vi "main4Ch_USBCam.vi"() -> ()   [LabVIEW 2024]
doc: "Main VI for FLS imaging system."
uses:
  SubVI/DigitizerConfiguration/FLImDAQ.ctl
  <instrlib>/niScope/Controls/niScope trigger source.ctl
  SubVI/LabJack/LJ Pin Setting.ctl
  ConfigFiles/AimingBeamVideoConfig.ctl
  LaguerreDeconLib/DeconEngineClass/LaguerreDeconEngineClass.lvclass/LaguerreDeconEngineClass.ctl
  <vilib>/Utility/error.llb/DialogType.ctl
  LaguerreDeconLib/DeconEngineClass/LaguerreDeconEngineClass.lvclass
  <vilib>/event_ctls.llb/usereventprio.ctl
  <vilib>/Utility/miscctls.llb/LVMinMaxIncTypeDef.ctl
  SubVI/APD/APDClass.lvclass
  <vilib>/vision/driver/IMAQdx.llb/IMAQdx Acquisition Mode.ctl
  <vilib>/userDefined/High Color/IMAQdx.ctl
  <vilib>/vision/driver/IMAQdx.llb/IMAQdx Camera Control Mode.ctl
  <vilib>/vision/driver/IMAQdx.llb/IMAQdx Buffer Number Mode.ctl
  <vilib>/Analysis/baseanly.llb/Mean (DBL).vi
  SubVI/GlobalVariables.vi
  <vilib>/addons/control/pid/pid.llb/PID (DBL).vi
  <vilib>/Utility/file.llb/Write Delimited Spreadsheet (DBL).vi
  <instrlib>/niScope/Acquire/Fetch/niScope Multi Fetch Binary 16.vi
  <vilib>/Instr/_visa.llb/VISA Configure Serial Port (Instr).vi
  <userlib>/_OpenG.lib/file/file.llb/openg_file.lvlib
  <userlib>/_OpenG.lib/time/time.llb/openg_time.lvlib
  <vilib>/Analysis/NI_AALBase.lvlib
  <vilib>/Utility/miscctls.llb/LVPointTypeDef.ctl
  <vilib>/addons/control/pid/NI_PID_pid.lvlib
  <vilib>/vision/driver/NI_Vision_Acquisition_Software.lvlib
  <resource>/objmgr/imaqdx.rc
panel:
  out "Image 2":T1(plugin-control)
  in  "Live?":bool
  out "Record Backlog 2":i32
  in  "Auto gain ch4":bool=TRUE caption="Auto gain ch3"
  in  "V 4":dbl caption="Gain 3" min=0.0 max=4.67 step=0.1
  out "Gain4":dbl
  out "Lifetime 4":dbl caption="Lifetime 3"
  out "IntR4":dbl format="%#_2g"
  out "SNR4":dbl format="%#_3g"
  out "Channel 4":dbl[][](graph) caption="Channel 3"
  out "RunStartTime":u32
  out "Dig1 Temp":dbl
  out "Dig2 Temp":dbl
  out "Visualization PC video source":T2
  in  "V target(1.0)":dbl=1.0 caption="V target(1.5)" min=0.3 max=1.5 step=0.1 format="%#_4g"
  out "SNR3":dbl format="%#_3g"
  out "SNR2":dbl format="%#_3g"
  out "SNR1":dbl format="%#_3g"
  in  "Show BG removed?":bool=TRUE
  out "IntR3":dbl format="%#_2g"
  out "IntR2":dbl format="%#_2g"
  out "IntR1":dbl format="%#_2g"
  in  "Video Display":bool
  out "Gain3":dbl
  out "Gain2":dbl
  out "Gain1":dbl
  in  "Skip Data Save?":bool
  out "Aq Loop?":bool
  out "ML?":bool
  out "aquisition loop Error Out":errorcluster
  out "Laser f (Hz)":dbl
  out "Record Backlog":i32
  out "Fetch Record #":i32
  out "Sync Success?":bool
  out "Disclamer":picture
  out "Calibration #":i8
  out "BG #":i8
  in  "TCP Connect":bool
  out "Help":string
  in  "355nm Laser toggle":bool caption="355nm 460Hz"
  in  "Cali&iRF alignment":bool
  in  "Background":bool
  in  "Aiming beam toggle":bool caption="445nm 0Hz 25mA"
  out "Lifetime 3":dbl
  out "Lifetime 2":dbl
  in  "Auto gain ch3":bool=TRUE
  in  "Auto gain ch2":bool=TRUE
  in  "Auto gain ch1":bool=TRUE
  out "Run #":i8
  in  "StopButton":bool caption="Stop"
  out "Aquisition Status:":bool
  in  "StartButton":bool caption="Start"
  in  "V 3":dbl caption="Gain 3" min=0.0 max=4.68 step=0.1
  in  "V 2":dbl caption="Gain 2" min=0.0 max=4.62 step=0.1
  out "Lifetime 1":dbl
  in  "V 1":dbl caption="Gain 1" min=0.0 max=4.66 step=0.1 format="%#_4g"
  in  "Video Source":enum32{"Camera", "FrameGrabber"}(radio)
  out "Case #":string
  out "System Hardware Connection Status":T3
  out "Channel 3":dbl[][](graph)
  out "Channel 2":dbl[][](graph)
  out "Channel 1":dbl[][](graph)
  in  "Tab Control":T4(tab)
  out "display loop timing(ms)":u32
  out "Aquisition loop timing(ms)":u32 format="%.2f"
  out "DisplayLoop":i32
  out "PID loop":i32 caption="processing loop"
  out "PID loop timing(ms)":u32 caption="processing loop timing(ms)"
  out "laser EM lamp V":dbl format="%0.6f"
  out "Decon Loop timing (ms)":dbl
  out "Auisition Loop idx":i32
  out "LJ process (ms)":u32
  out "LJ time(ms)":u32[](array[numeric])
  out "output variable":i32
  out "Lifetime (ns)":dbl(graph)
  out "Waveform Chart":dbl(graph)
  in  "Truncation":u32=600
  out "iRF Graph":dbl[][](graph)
  in  "Show BG":bool
  out "iRF length":i32
  out "BG length":i32
  out "data length":i32
  out "SysConfigCluster":T5
  out "LJ Pinout":T6={"Ch1 Bias"="DAC0", "Ch2 Bias"="DAC1", "Ch3 Bias"="DAC2", "Ch4 Bias"="DAC0", "355 PWM"="FIO0", "AimingBeam PWM"="FIO2", "Laser Ready"="FIO3", "Interlock"="FIO1", "Laser Start/Stop"="FIO1", "Red LED"="FIO1", "Green LED"="DIO3", "Foot Pedal"="DIO15"}
  out "FLImDAQ":T7={"Digitizer 1"="", "Digitizer 2"="", "Channel"=enum."Channel 0", "trigger source"="VAL_EXTERNAL", "trigger level"=0.5, "trigger delay"=1.35e-07, "min sample rate"=12500000000.0, "min record length"=2500, "vertical range"=1.0, "vertical offset"=-0.25, "Waveform to Avg"=2000} caption="FLIm DAQ Configuration" {"trigger delay" format="%^#.4e"; "trigger level" min=0.0 max=3.5 step=0.5 format="%.2f"; "vertical offset" format="%.4f"; "vertical range" format="%.2f"; "min sample rate" format="%#.2p"}
  in  "Sys Reconfig":bool
  out "PID loop error out":errorcluster caption="processing Error Out"
  out "decon error out":errorcluster
  out "Laser Rep Rate":dbl
  out "V4 Size":i32 caption="V3 Size"
  in  "Data Class":enum16{"Data", "BG", "Cali"}(ring)
  out "V1 Size":i32
  out "V2 Size":i32
  out "V3 Size":i32
  out "data Size":i32[](array[numeric])
  out "State log":string
  in  "Ch4 PID gains":T9={"proportional gain (Kc)"=30.0, "integral time (Ti, min)"=0.0003, "derivative time (Td, min)"=1e-05}
  in  "Ch3 PID gains":T9={"proportional gain (Kc)"=30.0, "integral time (Ti, min)"=0.0003, "derivative time (Td, min)"=1e-05}
  in  "Ch2 PID gains":T9={"proportional gain (Kc)"=30.0, "integral time (Ti, min)"=0.0003, "derivative time (Td, min)"=1e-05}
  in  "Ch1 PID gains":T9={"proportional gain (Kc)"=30.0, "integral time (Ti, min)"=0.0003, "derivative time (Td, min)"=1e-05}
  out "PNG write time (ms)":dbl(graph)
  in  "VideoMode":u32=12
  out "Acquired Frames/s":dbl
  out "FLIm 1st point time":dbl format="%_19f"
  out "Cam error out":errorcluster
  in  "Quit":bool
  in  "Radio Buttons":T10(radio)=enum."Ch2" caption="DeCon Chan"
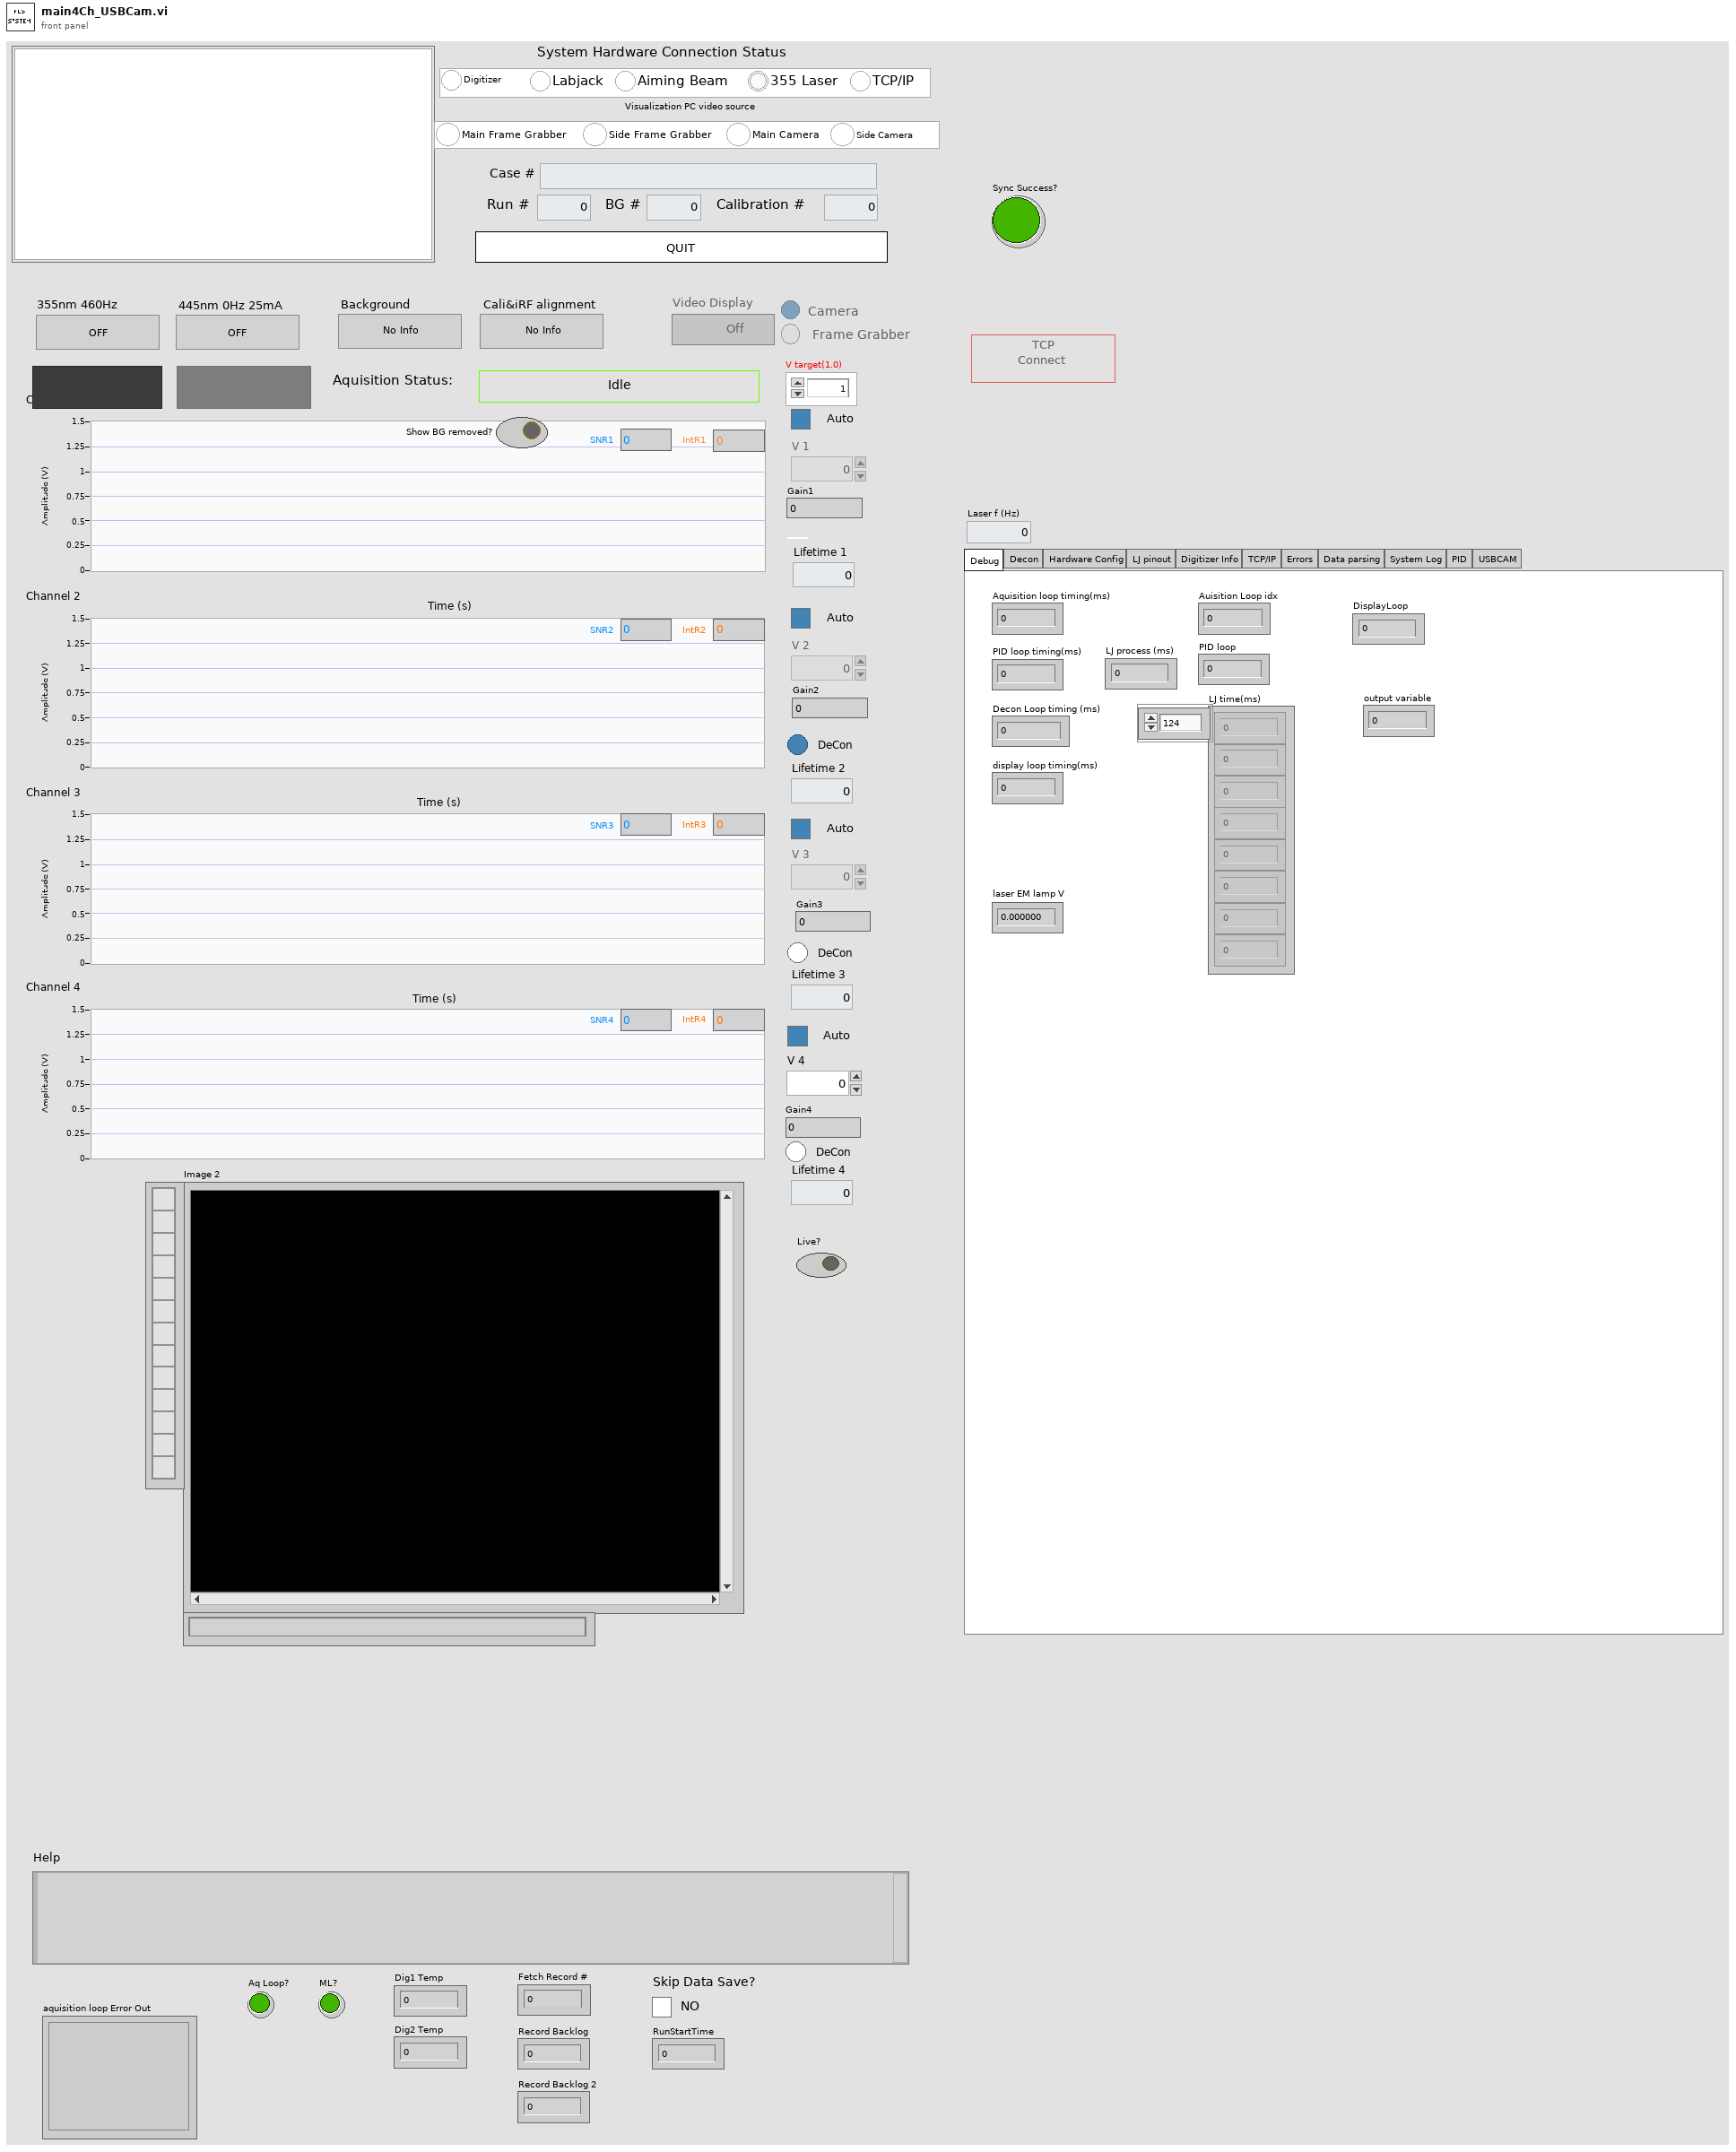
[diagram p1: front panel]
types:
  T1 = typedef "IMAQ Image.ctl" = refnum<image>
  T2 = cluster{"Main Frame Grabber":bool, "Side Frame Grabber":bool, "Main Camera":bool, "Side Camera":bool}
  T3 = cluster{"Digitizer":bool, "Labjack":bool, "Aiming Beam":bool, "355 Laser":bool, "TCP/IP":bool}
  T4 = enum32{"Debug", "Decon", "Hardware Config", "LJ pinout", "Digitizer Info", "TCP/IP", "Errors", "Data parsing", "System Log", "PID", "USBCAM"}
  T5 = cluster{"Ch1Enable?":bool, "Ch2Enable?":bool, "Ch3Enable?":bool, "Ch1AutoGain?":bool, "Ch2AutoGain?":bool, "Ch3AutoGain?":bool, "AimingBeamEnable?":bool}
  T6 = typedef "LJ Pin Setting.ctl" = cluster{"Ch1 Bias":string, "Ch2 Bias":string, "Ch3 Bias":string, "Ch4 Bias":string, "355 PWM":string, "AimingBeam PWM":string, "Laser Ready":string, "Interlock":string, "Laser Start/Stop":string, "Red LED":string, "Green LED":string, "Foot Pedal":string}
  T7 = typedef "FLImDAQ.ctl" = cluster{"Digitizer 1":refnum<k15>, "Digitizer 2":refnum<k15>, "Channel":enum16{"Channel 0", "Channel 1", "Channel 0&1"}, "trigger source":T8, "trigger level":dbl, "trigger delay":dbl, "min sample rate":dbl, "min record length":i32, "vertical range":dbl, "vertical offset":dbl, "Waveform to Avg":i16}
  T8 = typedef "niScope trigger source.ctl" = string
  T9 = cluster{"proportional gain (Kc)":dbl, "integral time (Ti, min)":dbl, "derivative time (Td, min)":dbl}
  T10 = enum32{"No Selection", "Ch1", "Ch2", "Ch3", "Ch4"}
  T11 = cluster{"remote start event":refnum<user-event>, "remote stop  event":refnum<user-event>}
  T12 = enum8{"Enabled", "Disabled", "Disabled and Grayed Out"}
  T13 = enum16{"open", "replace", "create", "open or create", "replace or create", "replace or create with confirmation"}
  T14 = cluster{"CH1":dbl[][], "CH2":dbl[][], "CH3":dbl[][], "CH4":dbl[][], "Gain cluster":cluster{"V1":dbl, "V2":dbl, "V3":dbl, "V4":dbl}}
  T15 = cluster{"idx":i32, "CH1&2":dbl[][], "CH3":dbl[][], "V cluster":cluster{"V1":dbl, "V2":dbl, "V3":dbl, "V4":dbl}}
  T16 = cluster{"Ch1 iRF":dbl[], "Ch2 iRF":dbl[], "Ch3 iRF":dbl[], "Ch4 iRF":dbl[]}
  T17 = enum16{"open", "open or create", "create or replace", "create", "open (read-only)"}
  T18 = enum32{"Invalid", "Standard", "Closed", "Hidden", "Minimized", "Maximized"}
  T19 = enum32{"invalid app kind", "Development System", "Run Time System", "Student Edition", "Embedded LabVIEW", "Evaluation", "Custom"}
  T20 = typedef "usereventprio.ctl" = enum32{"high priority", "normal priority"}
  T21 = enum32{"Bad", "Idle", "Run top level", "Running"}
  T22 = enum16{"Standard", "Buffered", "CRLF", "Immediate"}
  T23 = typedef "NI_Vision_Acquisition_Software.lvlib/IMAQdx Acquisition Mode.ctl" = enum32{"One Shot", "Continuous"}
  T24 = typedef "NI_Vision_Acquisition_Software.lvlib/IMAQdx Camera Control Mode.ctl" = enum32{"Controller", "Listener"}
  T25 = typedef "IMAQdx.ctl" = refnum<k21>
  T26 = typedef "AimingBeamVideoConfig.ctl" = cluster{"DeCon Channel":enum16{"1", "2", "3"}, "Scale Bar":bool, "Scale Low":dbl, "Scale High":dbl, "ANSI":dbl, "Radius":dbl, "3D?":bool, "Firefly?":bool, "Pentero?":bool}
  T27 = cluster{"Core":cluster{"Current VI Reference":refnum<vi>, "Close Panel on Exit?":bool}, "SysConfigCluster":cluster{"Ch1Enable?":bool, "Ch2Enable?":bool, "Ch3Enable?":bool, "Ch1AutoGain?":bool, "Ch2AutoGain?":bool, "Ch3AutoGain?":bool, "AimingBeamEnable?":bool}, "System Status":cluster{"Digitizer":bool, "Labjack":bool, "Aiming Beam":bool, "355 Laser":bool, "TCP/IP":bool}, "IDs":cluster{"RunID":i8, "BG ID":i8, "Cali ID":i8}, "CaseID":string, "DefaultPath":path, "Pathes":cluster{"DataPath":path, "BG Path":path, "iRFPath":path, "CaliPath":path}, "FLImDAQ":cluster{"resource name":refnum<k15>, "resource name 2":refnum<k15>, "Channel":enum16{"Channel 0", "Channel 1", "Channel 0&1"}, "trigger source":T8, "trigger level":dbl, "trigger delay":dbl, "min sample rate":dbl, "min record length":i32, "vertical range":dbl, "vertical offset":dbl, "Waveform to Avg":i32}, "SysRunning?":bool, "AB Cluster":cluster{"Aiming Beam COM Port":refnum<visa-resource-name>, "Min Current":dbl, "Max Current":dbl, "Default Current":dbl, "Freq":i32}, "LJ Pinout":T6, "355 PWM setting":cluster{"DIO_EF_CLOCK1_DIVISOR":i16, "DIO_EF_CLOCK1_ROLL_VALUE":i32, "DIO#_EF_INDEX":i16, "DIO#_EF_OPTIONS":i16, "DIO#_EF_CONFIG_A":i32}, "AB PWM setting":cluster{"DIO_EF_CLOCK1_DIVISOR":i16, "DIO_EF_CLOCK1_ROLL_VALUE":i32, "DIO#_EF_INDEX":i16, "DIO#_EF_OPTIONS":i16, "DIO#_EF_CONFIG_A":i32}, "Last Trigger":u32, "niTClk sessions":refnum<k20>[], "Laser start tic":u32, "TCP attempt count":i32, "Ch1Data":dbl[][], "Ch2Data":dbl[][], "Ch3Data":dbl[][], "Ch4Data":dbl[][], "V1":dbl[], "V2":dbl[], "V3":dbl[], "V4":dbl[], "SlowTimer":u32, "FastTimer":u32, "listener ID":refnum<k5>, "TempPath":path, "CaliPath":path, "LED vi reference":refnum<vi>, "Aquisition Timer":u32, "APDSerialNum":cluster{"Ch1APDSerial#":string, "Ch2APDSerial#":string, "Ch3APDSerial#":string, "Ch4APDSerial#":string}, "VideoConfig":T26, "LED vi ref open?":bool, "video source":cluster{"Main Frame Grabber":bool, "Side Frame Grabber":bool, "Main Camera":bool, "Side Camera":bool}, "bothVidSourceAvail":bool}
  T28 = typedef "LVCursorListTypeDef.ctl" = cluster{"Name":string, "Color":u32, "Style":u8, "Point Style":u8, "Name Visible":bool, "Allow Drag":bool, "Cursor Mode":u32, "Plot":i32, "Index":i32, "Position":cluster{"X":dbl, "Y":dbl}, "X Scale":u32, "Y Scale":u32, "Watch Plots":i32[], "Watch All Plots":bool, "Plot Area":i32, "Label Offset":cluster{"X":dbl, "Y":dbl}}[]
  T29 = cluster{"Name":string, "Color":u32, "Style":u8, "Point Style":u8, "Name Visible":bool, "Allow Drag":bool, "Cursor Mode":u32, "Plot":i32, "Index":i32, "Position":cluster{"X":dbl, "Y":dbl}, "X Scale":u32, "Y Scale":u32, "Watch Plots":i32[], "Watch All Plots":bool, "Plot Area":i32, "Label Offset":cluster{"X":dbl, "Y":dbl}}
  T30 = cluster{"Ch1APDSerial#":string, "Ch2APDSerial#":string, "Ch3APDSerial#":string, "Ch4APDSerial#":string}
  T31 = cluster{"DataPath":path, "BG Path":path, "iRFPath":path, "CaliPath":path}
  T32 = cluster{"DIO_EF_CLOCK1_DIVISOR":i16, "DIO_EF_CLOCK1_ROLL_VALUE":i32, "DIO#_EF_INDEX":i16, "DIO#_EF_OPTIONS":i16, "DIO#_EF_CONFIG_A":i32}
  T33 = cluster{"Aiming Beam COM Port":refnum<visa-resource-name>, "Min Current":dbl, "Max Current":dbl, "Default Current":dbl, "Freq":i32}
  T34 = cluster{"resource name":refnum<k15>, "resource name 2":refnum<k15>, "Channel":enum16{"Channel 0", "Channel 1", "Channel 0&1"}, "trigger source":T8, "trigger level":dbl, "trigger delay":dbl, "min sample rate":dbl, "min record length":i32, "vertical range":dbl, "vertical offset":dbl, "Waveform to Avg":i32}
  T35 = cluster{"Current VI Reference":refnum<vi>, "Close Panel on Exit?":bool}
  T36 = cluster{"Channel 1":dbl[], "Channel 2":dbl[], "Channel 3":dbl[], "Channel 4":dbl[]}
  T37 = cluster{"V 1":dbl[], "V 2":dbl[], "V 3":dbl[], "V 4":dbl[]}
  T38 = cluster{"Ch1 WF":dbl[], "Ch2 WF":dbl[], "Ch3 WF":dbl[], "Ch4 WF":dbl[], "V1":dbl, "V2":dbl, "V3":dbl, "V4":dbl}
  T39 = typedef "iRFData.ctl" = cluster{"dt":dbl, "NumOfWFs":i32, "WFLength":i32, "iRFCtrlV":dbl[], "iRFWFsAvg":dbl[][], "iRFRaw":dbl[][]}
  T40 = cluster{"mean":dbl, "mean":dbl, "mean":dbl, "mean":dbl}
  T41 = cluster{"V1":dbl, "V2":dbl, "V3":dbl, "V4":dbl}[]
  T42 = cluster{"DataPath":path, "CaseID":string, "RunID":i16, "Ch1Data":dbl[][], "Ch2Data":dbl[][], "Ch3Data":dbl[][], "Ch4Data":dbl[][], "V1":dbl[], "V2":dbl[], "V3":dbl[], "V4":dbl[], "LaserRepRate":u16, "WFAverage":i16, "RunStartTime":u64}
  T43 = typedef "DialogType.ctl" = u16
  T44 = typedef "LJ PWM Setting.ctl" = cluster{"DIO_EF_CLOCK1_DIVISOR":i16, "DIO_EF_CLOCK1_ROLL_VALUE":i32, "DIO#_EF_INDEX":i16, "DIO#_EF_OPTIONS":i16, "DIO#_EF_CONFIG_A":i32}
  T45 = typedef "AimingBeam.ctl" = cluster{"Aiming Beam COM Port":refnum<visa-resource-name>, "Min Current":dbl, "Max Current":dbl, "Default Current":dbl, "Frequency(Hz)":u32}
  T46 = cluster{"DC1":i32, "DC2":i32, "BG1":i32, "BG2":i32}
  T47 = typedef "LVMinMaxIncTypeDef.ctl" = cluster{"Minimum":dbl, "Maximum":dbl, "Increment":dbl}
  T48 = typedef "LVBoundsTypeDef.ctl" = cluster{"Width":u32, "Height":u32}
  T49 = typedef "imagedata.ctl" = cluster{"image type":i32, "image depth":i32, "image":u8[], "mask":u8[], "colors":u32[], "Rectangle":cluster{"left":i16, "top":i16, "right":i16, "bottom":i16}}
  T50 = cluster{"DC Idx1":i32, "DC Idx2":i32, "BG Idx1":i32, "BG Idx2":i32}
  T51 = typedef "LVPointTypeDef.ctl" = cluster{"Horizontal":i16, "Vertical":i16}
  T52 = cluster{"actualSamples":i32, "absoluteInitialX":dbl, "relativeInitialX":dbl, "xIncrement":dbl, "offset":dbl, "gain":dbl, "reserved1":dbl, "reserved2":dbl}[]
  T53 = cluster{"V1 out":dbl, "V2 out":dbl, "V3 out":dbl, "V3 out":dbl}
  T54 = cluster{i32, dbl[][], dbl[][], cluster{"V1 out":dbl, "V2 out":dbl, "V3 out":dbl, "V3 out":dbl}}
  T55 = cluster{dbl[][], dbl[][], dbl[][], dbl[][], "V cluster":cluster{"V1":dbl, "V2":dbl, "V3":dbl, "V4":dbl}}
  T56 = typedef "NI_Vision_Acquisition_Software.lvlib/IMAQdx Buffer Number Mode.ctl" = enum32{"Next", "Last", "Buffer Number", "Every", "Last New"}
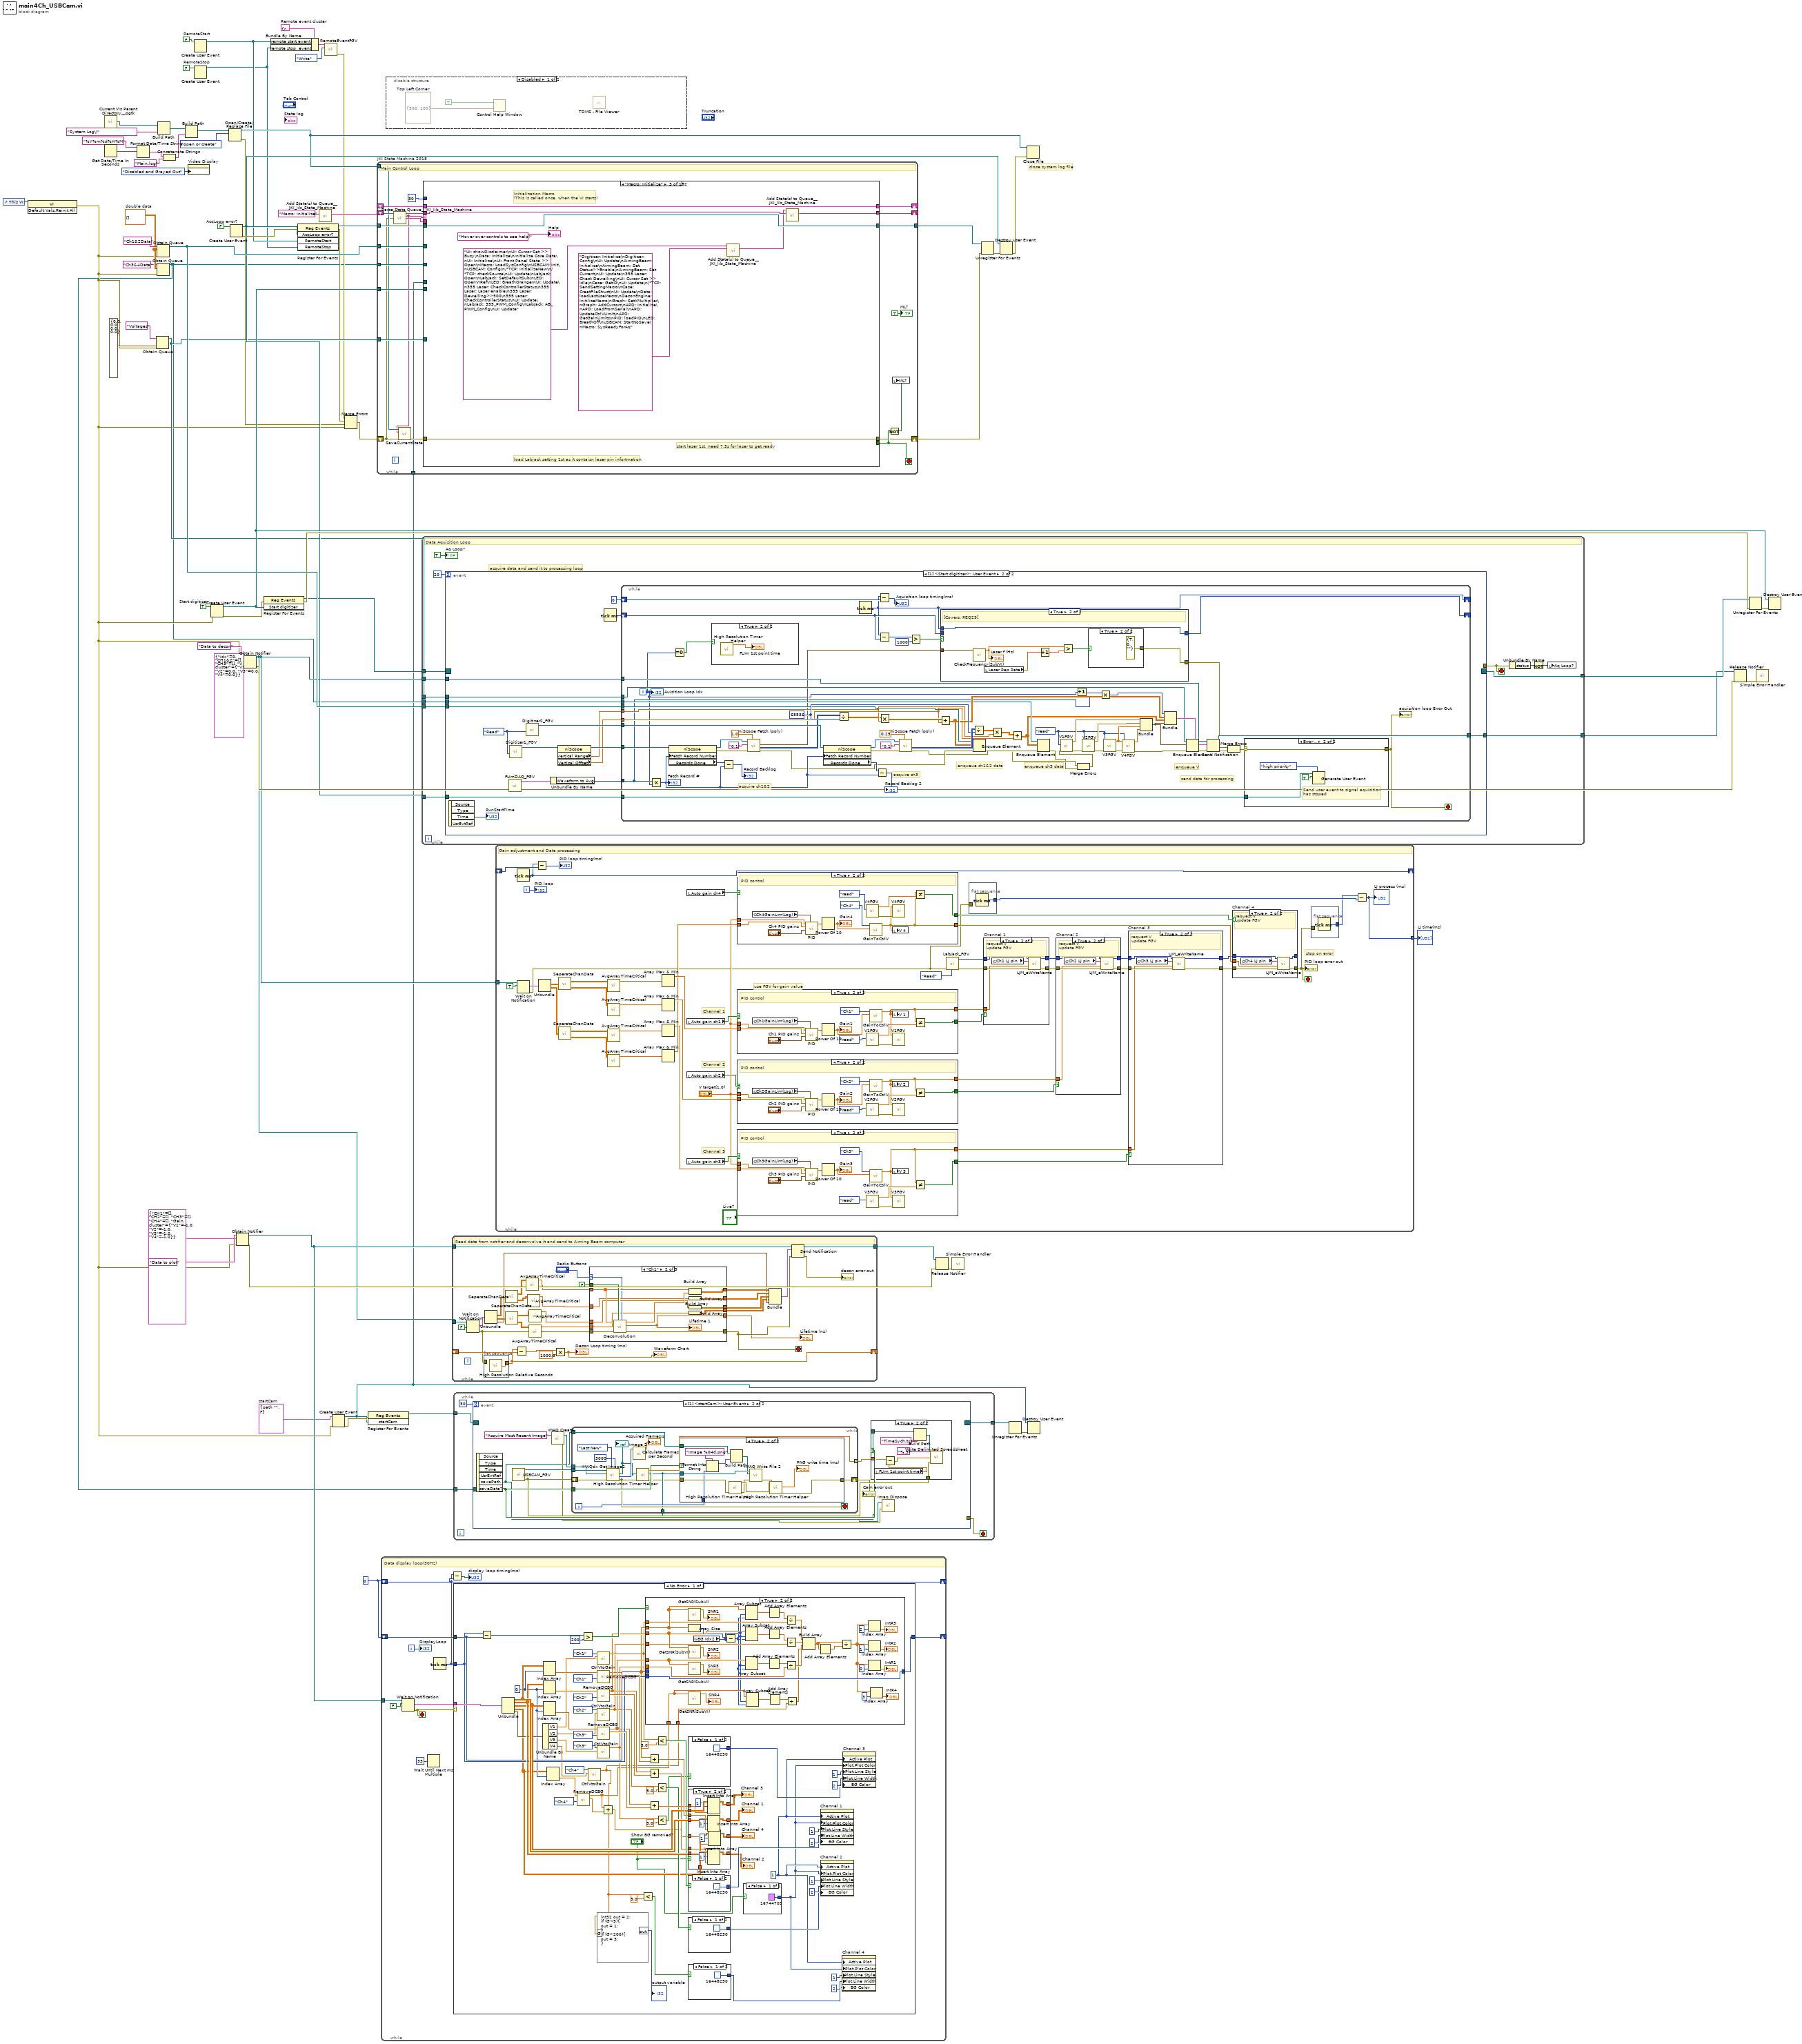
[diagram p0: block diagram]
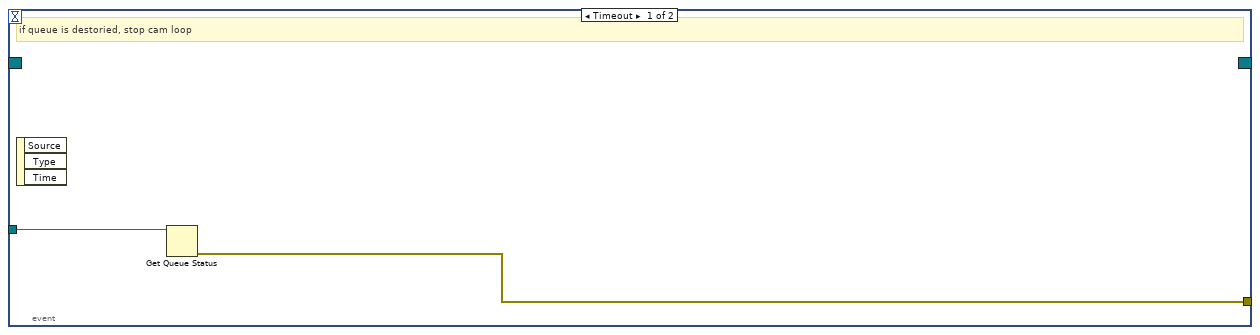
[diagram p2: hidden frame]
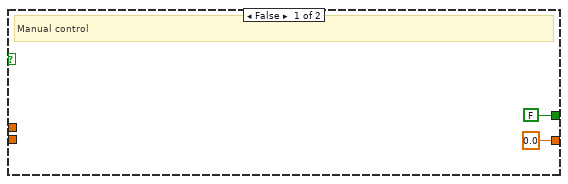
[diagram p9: hidden frame]
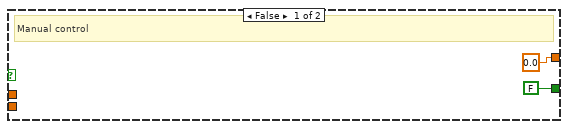
[diagram p10: hidden frame]
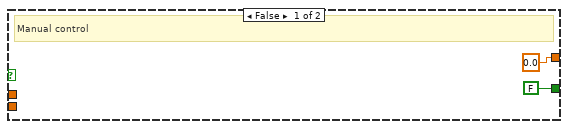
[diagram p11: hidden frame]
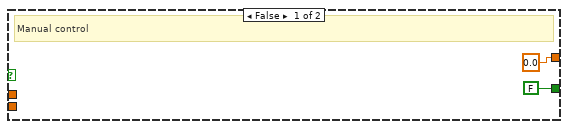
[diagram p12: hidden frame]
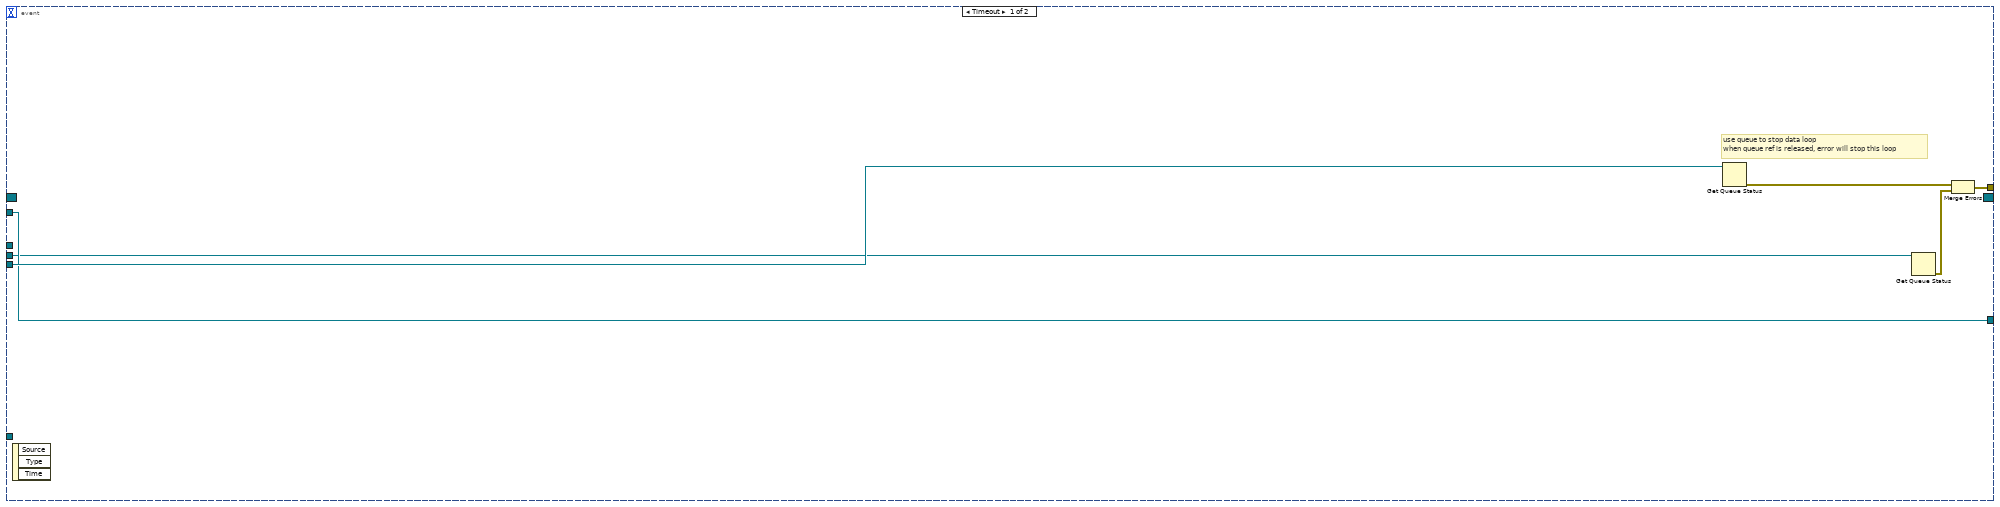
[diagram p13: hidden frame]
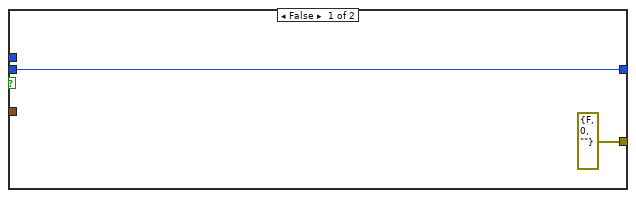
[diagram p15: hidden frame]
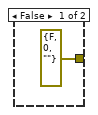
[diagram p16: hidden frame]
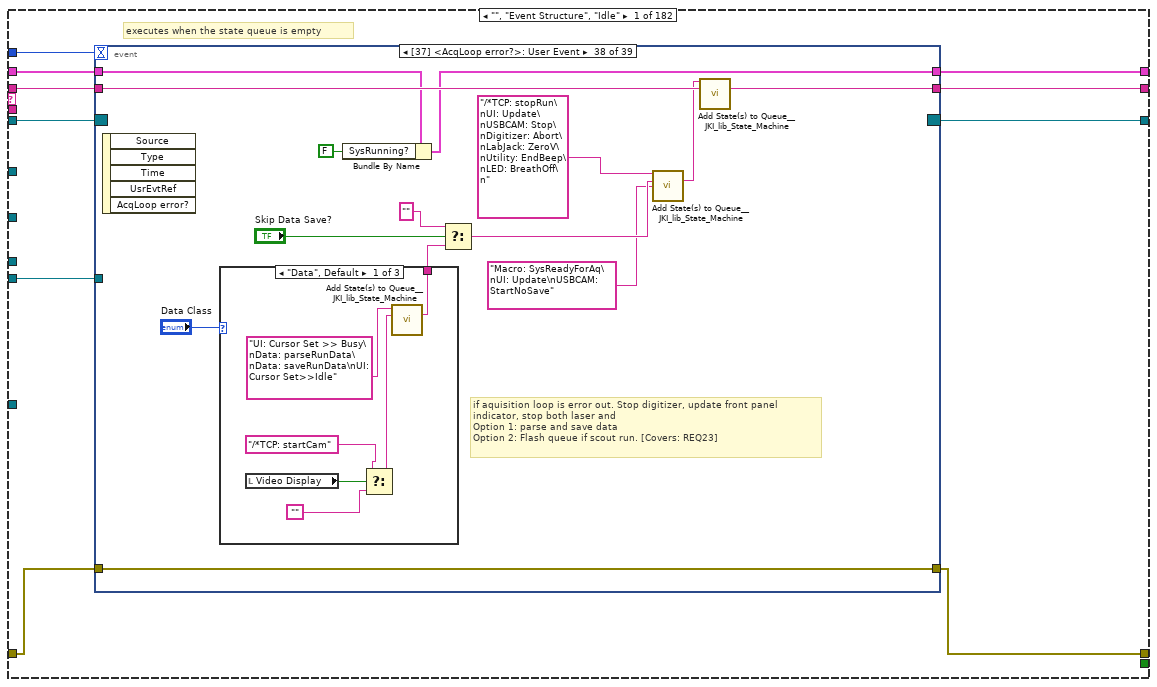
[diagram p18: hidden frame]
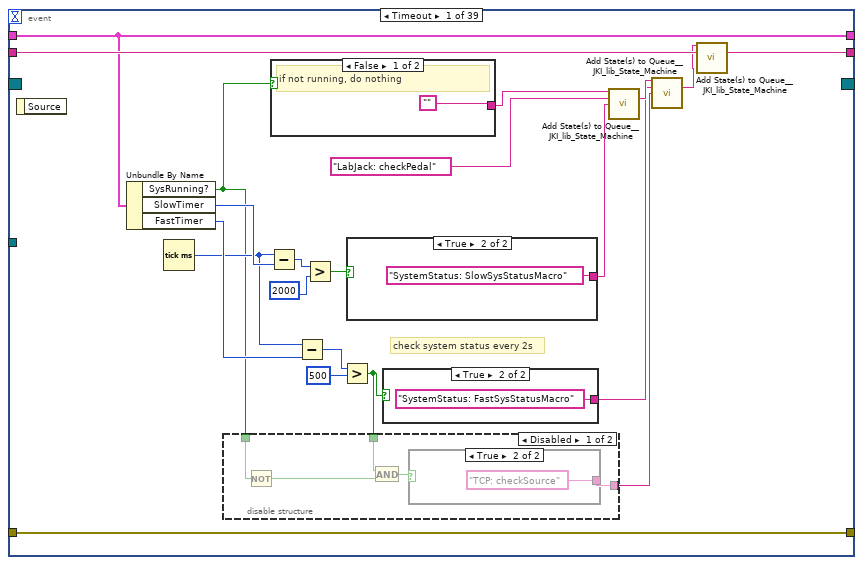
[diagram p19: hidden frame]
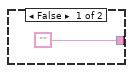
[diagram p20: hidden frame]
diagram:
  w8 = cluster{"savePath":path, "saveData?":bool} {"savePath"=path "", "saveData?"=FALSE}  # startCam
  w16 = T11 {"remote start event"=refnum, "remote stop  event"=refnum}  # Remote event cluster
  w19 = FALSE  # RemoteStop
  w20 = FALSE  # RemoteStart
  w23 = u32 0 ("millisecond timer value")
  w53 = FALSE  # AcqLoop error?
  w63 = TRUE  # Start digitizer
  w66 = dbl[][] []  # double data
  # "close system log file"
  n1 = control-ref of="This VI"() -> (w68:refnum<vi>)
  n2 = invoke on="Invoke Node" class="VI" method="Default Vals.Reinit All"(reference=w68) -> (error out=w7:errorcluster)  [unwired: 2 in, 2 out]
  n3 = call <userlib>:"Current VIs Parent Directory__ogtk.vi"() -> ("Parent Directory (+ Relative)"=w39:path)  [unwired: 5 in]
  n4 = Get Date/Time In Seconds() -> (seconds since 1Jan1904=w37:timestamp)
  n5 = Format Date/Time String(time format string (%c)="%Y%m%d%H%M", seconds (now)=w37) -> (date/time string=w34:string)  [unwired: 1 in]
  n6 = Obtain Queue(name (unnamed)="Voltages", element data type=cluster{"V1":dbl, "V2":dbl, "V3":dbl, "V4":dbl} {"V1"=0.0, "V2"=0.0, "V3"=0.0, "V4"=0.0}, error in (no error)=w7) -> (queue out=w40:refnum<queue>)  [unwired: 2 in, 2 out]
  n7 = Obtain Queue(name (unnamed)="Ch3&4Data", element data type=w66, error in (no error)=w7) -> (queue out=w4:refnum<queue>)  [unwired: 2 in, 2 out]
  n8 = Obtain Queue(name (unnamed)="Ch1&2Data", element data type=w66, error in (no error)=w7) -> (queue out=w64:refnum<queue>)  [unwired: 2 in, 2 out]
  n9 = Build Path(base path=w39, name or relative path="System Log\\") -> (appended path=w30:path)
  n10 = Concatenate Strings(w34, "Main.log" ("string")) -> (w32:string)
  n11 = Build Path(base path=w30, name or relative path=w32) -> (appended path=w35:path)
  n12 = property on="Video Display" class="Bool (strict)"("DisabledEnum"=T12."Disabled and Grayed Out" ("Disabled")) -> ()  [unwired: 2 in, 2 out]
  n13 = Create User Event(user event datatype=w20) -> (user event=w18:refnum<user-event>)  [unwired: 1 in, 1 out]
  n14 = Create User Event(user event datatype=w19) -> (user event=w17:refnum<user-event>)  [unwired: 1 in, 1 out]
  n15 = Create User Event(user event datatype=w63, error in=w7) -> (user event=w52:refnum<user-event>, error out=w44:errorcluster)
  n16 = Open/Create/Replace File(file path (use dialog)=w35, operation (0:open)=T13."open or create") -> (refnum out=w27:refnum<file>, error out=w28:errorcluster)  [unwired: 4 in, 1 out]
  n17 = Create User Event(user event datatype=w53) -> (user event=w43:refnum<user-event>, error out=w45:errorcluster)  [unwired: 1 in]
  n18 = Obtain Notifier(name (unnamed)="Data to plot", notification data type=T14 {"CH1"=[], "CH2"=[], "CH3"=[], "CH4"=[], "Gain cluster"={"V1"=-1.0, "V2"=-1.0, "V3"=-1.0, "V4"=-1.0}}, error in (no error)=w7) -> (notifier out=w21:refnum<notifier>, error out=w48:errorcluster)  [unwired: 1 in, 1 out]
  n19 = Obtain Notifier(name (unnamed)="Data to decon", notification data type=T15 {"idx"=0, "CH1&2"=[], "CH3"=[], "V cluster"={"V1"=0.0, "V2"=0.0, "V3"=0.0, "V4"=0.0}}, error in (no error)=w7) -> (notifier out=w25:refnum<notifier>, error out=w57:errorcluster)  [unwired: 1 in, 1 out]
  n20 = register-events(error in=w44, w52) -> (reference out=w54:refnum<event-registration>, error out=w60:errorcluster)  [unwired: 1 in]
  n21 = Bundle By Name(cluster=w16, "remote start event"=w18, "remote stop  event"=w17) -> (w14:T11)
  n22 = register-events(error in=w45, w43, w18, w17) -> (reference out=w47:refnum<event-registration>, error out=w13:errorcluster)  [unwired: 1 in]
  n23 = call <vilib>:"Add State(s) to Queue__JKI_lib_State_Machine.vi"("State(s) in (\"\")"="Macro: Initialize") -> ("States Out"=w70:string)  [unwired: 14 in]
  n24 = call "RemoteEventFGV.vi"("Operation (Read)"=enum16{"Read", "Write"}."Write", "Remote Event in"=w14) -> ("Error Out"=w10:errorcluster)  [unwired: 8 in, 1 out]
  n25 = Create User Event(user event datatype=w8, error in=w7) -> (user event=w1:refnum<user-event>, error out=w6:errorcluster)
  n26 = Merge Errors(w10, w13, w28, w7) -> (w29:errorcluster)
  n27 = register-events(error in=w6, w1) -> (reference out=w5:refnum<event-registration>)  [unwired: 1 in, 1 out]
  n28 = while "JKI State Machine 2018" {
    shift-right: [w88] -> _
    shift-left: _ -> [w87]
    shift-right: [w72] -> w12
    shift-left: w29 -> [w74]
    shift-right: [w89] -> _
    shift-left: w70 -> [w90]
    tunnel: w64 -> [w85]
    tunnel: w4 -> [w84]
    tunnel: w52 -> [w83]
    tunnel: w47 -> [w82]
    tunnel: [w81] -> w46
    tunnel: w40 -> [w77]
    tunnel: w27 -> [w76]
    tunnel: w1 -> [w71]
    stop <- w80 stop-if-true
    # "Main Control Loop"
    n29 = call <vilib>:"Parse State Queue__JKI_lib_State_Machine.vi"("State Queue"=w90, "Error In (no error)"=w74) -> ("Remaining States"=w92:string, "Current State"=w75:string, "Arguments"=w91:string)  [unwired: 11 in]
    n30 = call "SaveCurrentState.vi"("error in (no error)"=w74, "Current State"=w75, "Byte Stream File in"=w76) -> ("error out"=w73:errorcluster)  [unwired: 8 in]
    n31 = case shown="\"Macro: Initialize\"" w75 {
      selector: w75 -> [_ _ _ _ _ _ _ _ _ _ _ _ _ _ _ _ _ _ _ _ _ _ _ _ w1082 _ _ _ _ _ _ _ _ _ _ _ _ _ _ _ _ _ _ _ _ _ _ _ _ _ _ _ _ _ _ _ _ _ _ _ _ _ _ _ _ _ _ _ _ _ _ _ _ _ _ _ _ _ _ _ _ _ _ _ _ _ _ _ _ _ _ _ _ _ _ _ _ _ _ _ _ _ _ _ _ _ _ _ _ _ _ _ _ _ _ _ _ _ _ _ _ _ _ _ _ _ _ _ _ _ _ _ _ _ _ _ _ _ _ _ _ _ _ _ _ _ _ _ _ _ _ _ _ _ _ _ _ _ _ _ _ _ _ _ _ _ _ _ _ _ _ _ _ _ _ _ _ _ _ _ _ _]
      tunnel: w92 -> [w102 w518 w527 w533 w539 w561 w574 w616 w622 w649 w668 w739 w754 w785 w812 w844 w858 w887 w901 w986 w1023 w1062 w1075 w1080 w1086 w1114 w1122 w1145 w1150 w1163 w1182 w1210 w1238 w1276 w1281 w1287 w1311 w1335 w1359 w1383 w1388 w1405 w1452 w1474 w1490 w1505 w1525 w1530 w1542 w1571 w1597 w1609 w1647 w1660 w1666 w1677 w1689 w1720 w1733 w1747 w1762 w1781 w1816 w1821 w1835 w1845 w1861 w1873 w1885 w1913 w1928 w1933 w1945 w1957 w1962 w1970 w1978 w1987 w1996 w2001 w2009 w2018 w2036 w2053 w2073 w2084 w2106 w2121 w2138 w2143 w2151 w2159 w2164 w2172 w2179 w2187 w2194 w2204 w2232 w2240 w2247 w2255 w2260 w2268 w2275 w2281 w2290 w2306 w2311 w2318 w2330 w2400 w2412 w2421 w2438 w2447 w2470 w2487 w2498 w2511 w2536 w2559 w2565 w2581 w2603 w2611 w2617 w2622 w2629 w2639 w2651 w2660 w2665 w2677 w2682 w2692 w2698 w2704 w2709 w2714 w2719 w2729 w2753 w2774 w2779 w2790 w2815 w2842 w2865 w2870 w2885 w2936 w2982 w3027 w3038 w3056 w3076 w3090 w3103 w3111 w3128 w3150 w3174 w3193 w3211 w3229 w3247 w3261 w3275 w3294 w3308 w3323 w3338 w3347 w3352 w3373 w3387 w3395 w3407 w3418 w3429 w3434]
      tunnel: w91 -> [_ _ _ _ _ _ _ _ _ _ _ _ _ _ _ _ _ _ _ _ _ _ _ _ _ _ _ _ _ _ _ _ _ _ _ _ _ _ _ _ _ _ _ _ _ _ _ _ _ _ _ _ _ _ _ _ w1687 _ _ _ _ _ _ _ _ _ _ _ _ _ _ _ _ _ _ _ _ _ _ _ _ _ _ _ _ _ _ _ _ _ _ _ _ _ _ _ _ w2195 _ _ _ _ _ _ _ _ _ _ _ w2313 w2324 _ _ _ _ w2444 _ _ _ _ _ w2555 _ _ _ _ _ _ w2624 _ _ _ _ _ _ w2688 _ _ _ _ _ _ _ _ _ _ _ _ _ _ _ _ _ _ _ _ _ _ _ _ _ _ _ _ _ _ _ _ _ _ _ _ _ _ _ _ _ _ _ _ _ _]
      tunnel: w87 -> [w100 w515 w523 w530 w536 w558 w571 _ w618 w645 w664 w736 w745 w782 w804 w835 w855 w884 w898 w947 w1015 w1050 w1070 w1077 w1084 w1107 w1119 w1143 w1147 w1151 w1172 w1202 w1230 w1272 w1278 w1284 w1292 w1316 w1341 w1365 w1385 w1398 w1442 w1471 w1475 w1502 w1522 w1527 w1531 w1560 w1587 w1602 w1630 w1658 w1663 w1670 w1685 w1703 w1728 w1739 w1757 w1774 w1799 w1818 w1831 w1839 w1858 w1870 w1882 w1901 w1917 w1930 w1943 w1955 w1959 w1964 w1971 w1983 w1992 w1998 w2005 w2015 w2023 w2040 w2068 w2074 w2103 w2114 w2136 w2140 w2144 w2152 w2161 w2170 w2176 w2184 w2191 w2201 w2229 w2237 w2244 w2252 w2257 w2262 w2273 w2278 w2284 w2303 w2308 w2316 w2326 w2397 w2402 w2415 w2436 w2445 w2460 w2484 w2495 w2505 w2529 w2556 w2562 w2574 w2599 w2608 w2614 w2619 w2626 w2633 w2647 w2657 w2662 w2674 w2679 w2685 w2695 w2701 w2706 w2711 w2716 w2726 w2751 w2772 w2776 w2788 w2813 w2840 w2863 w2867 w2878 w2930 w2978 w3024 w3034 w3051 w3071 w3085 w3099 w3105 w3123 w3145 w3169 w3188 w3206 w3224 w3242 w3256 w3270 w3289 w3303 w3318 w3335 w3345 w3349 w3365 w3379 w3393 w3405 w3412 w3426 w3431]
      tunnel: [w93 w516 w525 w531 w537 w559 w572 w614 w620 w641 w660 w713 w741 w783 w792 w824 w848 w875 w899 w923 w1012 w1049 w1071 w1078 w1088 w1111 errorcluster {"status"=FALSE, "code"=0, "source"=""} ("error out") w1142 w1148 w1161 w1180 w1194 w1217 w1274 w1279 w1285 w1293 w1317 w1342 w1366 w1386 w1389 w1434 w1465 w1479 w1503 w1513 w1528 w1534 w1558 w1586 w1601 w1617 w1652 w1664 w1675 w1679 w1694 w1723 w1735 w1753 w1773 w1790 w1819 w1823 w1841 w1856 w1868 w1880 w1903 w1918 w1931 w1935 w1952 w1960 w1968 w1976 w1980 w1989 w1999 w2002 w2011 w2026 w2048 w2067 w2078 w2096 w2118 w2134 w2141 w2149 w2157 w2162 w2169 w2177 w2185 w2192 w2202 w2230 w2238 w2245 w2253 w2258 w2266 w2272 w2279 w2287 w2304 w2309 w2314 w2327 w2398 w2406 w2418 w2428 w2441 w2461 w2485 w2494 w2507 w2531 w2557 w2563 w2571 w2593 w2609 w2615 w2620 w2627 w2637 w2649 w2658 w2663 w2675 w2680 w2690 w2696 w2702 w2707 w2712 w2717 w2727 w2741 w2765 w2777 w2781 w2800 w2832 w2857 w2868 w2872 w2931 w2979 w3025 w3033 w3053 w3073 w3087 w3101 w3107 w3125 w3147 w3171 w3190 w3208 w3226 w3244 w3258 w3272 w3291 w3305 w3319 w3336 w3343 w3350 w3367 w3381 w3389 w3396 w3409 w3425 w3432] -> w72
      tunnel: w73 -> [w99 w516 w525 w531 w537 w559 w572 w614 w620 w642 w658 w713 w740 w783 w793 w831 w848 w865 w899 w923 w1013 w1052 w1072 w1078 w1087 w1111 w1115 w1142 w1148 w1161 w1180 w1193 w1229 w1274 w1279 w1285 w1297 w1321 w1346 w1370 w1386 w1396 w1437 w1464 w1478 w1503 w1515 w1528 w1533 w1559 w1577 w1607 w1628 w1651 w1664 w1672 w1682 w1693 w1722 w1738 w1752 w1772 w1789 w1819 w1829 w1842 w1855 w1867 w1879 w1902 w1919 w1931 w1934 w1947 w1960 w1968 w1976 w1979 w1988 w1999 w2003 w2012 w2031 w2047 w2066 w2077 w2102 w2117 w2133 w2141 w2149 w2157 w2162 w2169 w2177 w2185 w2192 w2202 w2230 w2238 w2245 w2253 w2258 w2266 w2272 w2279 w2287 w2304 w2309 w2315 w2328 w2398 w2407 w2417 w2424 w2440 w2462 w2485 w2494 w2502 w2534 w2557 w2563 w2576 w2592 w2609 w2615 w2620 w2627 w2637 w2649 w2658 w2663 w2675 w2680 w2690 w2696 w2702 w2707 w2712 w2717 w2727 w2740 w2764 w2777 w2780 w2799 w2822 w2848 w2868 _ w2932 w2979 w3025 w3032 w3052 w3072 w3086 w3101 w3106 w3124 w3146 w3170 w3189 w3207 w3225 w3243 w3257 w3271 w3290 w3304 w3317 w3336 w3342 w3350 w3366 w3380 w3388 w3403 w3413 w3424 w3432]
      tunnel: [w101 w517 w526 w532 w538 w560 w573 w615 w621 w648 w667 w738 w753 w784 w811 w843 w857 w886 w900 w985 w1022 w1061 w1074 w1079 w1085 w1113 w1121 w1144 w1149 w1162 w1181 w1209 w1237 w1275 w1280 w1286 w1310 w1334 w1358 w1382 w1387 w1404 w1451 w1473 w1489 w1504 w1524 w1529 w1541 w1570 w1596 w1608 w1646 w1659 w1665 w1676 w1688 w1719 w1732 w1746 w1761 w1780 w1815 w1820 w1834 w1844 w1860 w1872 w1884 w1912 w1927 w1932 w1944 w1956 w1961 w1969 w1977 w1986 w1995 w2000 w2008 w2017 w2035 w2052 w2072 w2083 w2105 w2120 w2137 w2142 w2150 w2158 w2163 w2171 w2178 w2186 w2193 w2203 w2231 w2239 w2246 w2254 w2259 w2267 w2274 w2280 w2289 w2305 w2310 w2317 w2329 w2399 w2411 w2420 w2437 w2446 w2469 w2486 w2497 w2510 w2535 w2558 w2564 w2580 w2602 w2610 w2616 w2621 w2628 w2638 w2650 w2659 w2664 w2676 w2681 w2691 w2697 w2703 w2708 w2713 w2718 w2728 w2752 w2773 w2778 w2789 w2814 w2841 w2864 w2869 w2884 w2935 w2981 w3026 w3037 w3055 w3075 w3089 w3102 w3110 w3127 w3149 w3173 w3192 w3210 w3228 w3246 w3260 w3274 w3293 w3307 w3322 w3337 w3346 w3351 w3372 w3386 w3394 w3406 w3417 w3428 w3433] -> w89
      tunnel: [_ _ _ _ _ _ _ _ _ _ _ _ _ _ _ _ _ _ _ _ _ _ _ _ _ _ _ TRUE _ _ _ _ _ _ _ _ _ _ _ _ _ _ _ _ _ _ _ _ _ _ _ _ _ _ _ _ _ _ _ _ _ _ _ _ _ _ _ _ _ _ _ _ _ _ _ _ _ _ _ _ _ _ _ _ _ _ _ _ _ _ _ _ _ _ _ _ _ _ _ _ _ _ _ _ _ _ _ _ _ _ _ _ _ _ _ _ _ _ _ _ _ _ _ _ _ _ _ _ _ _ _ _ _ _ _ _ _ _ _ _ _ _ _ _ _ _ _ _ _ _ _ _ _ _ _ _ _ _ _ _ _ _ _ _ _ _ _ _ _ _ _ _ _ _ _ _ _ _ _ _ _ _] -> w80
      tunnel: [w98 w515 w523 w530 w536 w558 w571 w589 w618 w645 w664 w736 w745 w782 w804 w835 w855 w884 w898 w947 w1016 w1051 w1070 w1077 w1084 w1112 w1119 w1143 w1147 w1152 w1173 w1203 w1231 w1273 w1278 w1284 w1292 w1316 w1341 w1365 w1385 w1398 w1443 w1471 w1476 w1502 w1523 w1527 w1532 w1560 w1587 w1606 w1630 w1658 w1663 w1673 w1685 w1703 w1728 w1739 w1757 w1774 w1799 w1818 w1832 w1839 w1858 w1870 w1882 w1901 w1917 w1930 w1943 w1955 w1959 w1965 w1972 w1984 w1993 w1998 w2006 w2016 w2024 w2046 w2055 w2079 w2104 w2115 w2136 w2140 w2145 w2153 w2161 w2170 w2176 w2184 w2191 w2201 w2229 w2237 w2244 w2252 w2257 w2262 w2273 w2278 w2284 w2303 w2308 w2316 w2326 w2397 w2403 w2416 w2436 w2445 w2460 w2484 w2495 w2506 w2530 w2556 w2562 w2575 w2599 w2608 w2614 w2619 w2626 w2634 w2647 w2657 w2662 w2674 w2679 w2685 w2695 w2701 w2706 w2711 w2716 w2726 w2751 w2772 w2776 w2788 w2813 w2840 w2863 w2867 w2883 w2929 w2978 w3024 w3034 w3051 w3071 w3085 w3099 w3105 w3123 w3145 w3169 w3188 w3206 w3224 w3242 w3256 w3270 w3289 w3303 w3320 w3335 w3345 w3349 w3365 w3379 w3393 w3405 w3412 w3426 w3431] -> w88
      tunnel: 30 ("Timeout") -> [w97 _ _ _ _ _ _ _ _ _ _ _ _ _ _ _ _ _ _ _ _ _ _ _ _ _ _ _ _ _ _ _ _ _ _ _ _ _ _ _ _ _ _ _ _ _ _ _ _ _ _ _ _ _ _ _ _ _ _ _ _ _ _ _ _ _ _ _ _ _ _ _ _ _ _ _ _ _ _ _ _ _ _ _ _ _ _ _ _ _ _ _ _ _ _ _ _ _ _ _ _ _ _ _ _ _ _ _ _ _ _ _ _ _ _ _ _ _ _ _ _ _ _ _ _ _ _ _ _ _ _ _ _ _ _ _ _ _ _ _ _ _ _ _ _ _ _ _ _ _ _ _ _ _ _ _ _ _ _ _ _ _ _ _ _ _ _ _ _ _ _ _ _ _ _ _ _ _ _ _ _ _]
      tunnel: w85 -> [_ _ _ _ _ _ _ _ _ _ _ _ _ _ _ _ _ _ _ _ w1020 _ _ _ _ _ _ _ _ _ _ _ _ _ _ _ _ _ _ _ _ _ _ _ _ _ _ _ _ _ _ _ _ _ _ _ _ _ _ _ _ _ _ _ _ _ _ _ _ _ _ _ w1940 w1951 _ _ _ _ _ _ _ _ _ _ _ _ _ _ _ _ _ _ _ _ _ _ _ _ _ _ _ _ _ _ _ _ _ _ _ _ _ _ _ _ _ _ _ _ _ _ _ _ _ _ _ _ _ _ _ _ _ _ _ _ _ _ _ _ _ _ _ _ _ _ _ _ _ _ _ _ _ _ _ _ _ _ _ _ _ _ _ _ _ _ _ _ _ _ _ _ _ _ _ _ _ _ _ _ _ _ _ _]
      tunnel: w84 -> [_ _ _ _ _ _ _ _ _ _ _ _ _ _ _ _ _ _ _ _ w1019 _ _ _ _ _ _ _ _ _ _ _ _ _ _ _ _ _ _ _ _ _ _ _ _ _ _ _ _ _ _ _ _ _ _ _ _ _ _ _ _ _ _ _ _ _ _ _ _ _ _ _ w1941 w1950 _ _ _ _ _ _ _ _ _ _ _ _ _ _ _ _ _ _ _ _ _ _ _ _ _ _ _ _ _ _ _ _ _ _ _ _ _ _ _ _ _ _ _ _ _ _ _ _ _ _ _ _ _ _ _ _ _ _ _ _ _ _ _ _ _ _ _ _ _ _ _ _ _ _ _ _ _ _ _ _ _ _ _ _ _ _ _ _ _ _ _ _ _ _ _ _ _ _ _ _ _ _ _ _ _ _ _ _]
      tunnel: w83 -> [w96 _ _ _ _ _ _ _ _ _ _ _ _ _ _ _ _ _ _ _ _ _ _ _ _ _ _ _ _ _ _ _ _ _ _ _ _ _ _ _ _ _ _ w1467 _ _ _ _ _ _ _ _ _ _ _ _ _ _ _ _ _ _ _ _ _ _ _ _ _ _ _ _ _ _ _ _ _ _ _ _ _ _ _ _ _ _ _ _ _ _ _ _ _ _ _ _ _ _ _ _ _ _ _ _ _ _ _ _ _ _ _ _ _ _ _ _ _ _ _ _ _ _ _ _ _ _ _ _ _ _ _ _ _ _ _ _ _ _ _ _ _ _ _ _ _ _ _ _ _ _ _ _ _ _ _ _ _ _ _ _ _ _ _ _ _ _ _ _ _ _ _ _ _ _ _ _ _ _ _ _ _ _]
      tunnel: w82 -> [w95 w514 w524 w529 w535 w550 w570 w599 w619 w647 w666 w737 w752 w781 w810 w842 w856 w885 w897 w984 w1021 w1060 w1069 w1076 w1081 w1099 w1118 w1141 w1146 w1160 w1179 w1208 w1228 w1271 w1277 w1283 w1291 w1315 w1340 w1364 w1384 w1393 w1417 w1472 w1488 w1501 w1510 w1526 w1540 w1569 w1595 w1600 w1645 w1650 w1662 w1669 w1678 w1690 w1721 w1737 w1751 w1771 w1786 w1817 w1833 w1843 w1859 w1871 w1883 w1911 w1914 w1929 w1942 w1949 w1958 w1967 w1975 w1982 w1991 w1997 w2007 w2010 w2022 w2041 w2056 w2075 w2101 w2119 w2135 w2139 w2147 w2155 w2160 w2168 w2175 w2183 w2190 w2200 w2228 w2236 w2243 w2248 w2256 w2265 w2271 w2277 w2286 w2298 w2307 w2312 w2323 w2396 w2401 w2413 w2423 w2439 w2468 w2483 w2496 w2508 w2532 w2552 w2560 w2573 w2601 w2606 w2612 w2618 w2625 w2636 w2648 w2656 w2661 w2673 w2678 w2689 w2694 w2700 w2705 w2710 w2715 w2725 w2750 w2771 w2775 w2787 w2812 w2839 w2862 w2866 w2882 w2934 w2980 w3021 w3036 w3054 w3074 w3088 w3100 w3109 w3126 w3148 w3172 w3191 w3209 w3227 w3245 w3259 w3273 w3292 w3306 w3321 w3334 w3344 w3348 w3371 w3385 w3392 w3404 w3416 w3427 w3430]
      tunnel: [w94 w514 w524 w529 w535 w550 w570 w599 w619 w647 w666 w737 w752 w781 w810 w842 w856 w885 w897 w984 w1021 w1060 w1069 w1076 w1081 w1099 w1118 w1141 w1146 w1160 w1179 w1208 w1228 w1271 w1277 w1283 w1291 w1315 w1340 w1364 w1384 w1393 w1417 w1472 w1488 w1501 w1510 w1526 w1540 w1569 w1595 w1600 w1645 w1650 w1662 w1669 w1678 w1690 w1721 w1737 w1751 w1771 w1786 w1817 w1833 w1843 w1859 w1871 w1883 w1911 w1914 w1929 w1942 w1949 w1958 w1967 w1975 w1982 w1991 w1997 w2007 w2010 w2022 w2041 w2056 w2075 w2101 w2119 w2135 w2139 w2147 w2155 w2160 w2168 w2175 w2183 w2190 w2200 w2228 w2236 w2243 w2248 w2256 w2265 w2271 w2277 w2286 w2298 w2307 w2312 w2323 w2396 w2401 w2413 w2423 w2439 w2468 w2483 w2496 w2508 w2532 w2552 w2560 w2573 w2601 w2606 w2612 w2618 w2625 w2636 w2648 w2656 w2661 w2673 w2678 w2689 w2694 w2700 w2705 w2710 w2715 w2725 w2750 w2771 w2775 w2787 w2812 w2839 w2862 w2866 w2882 w2934 w2980 w3021 w3036 w3054 w3074 w3088 w3100 w3109 w3126 w3148 w3172 w3191 w3209 w3227 w3245 w3259 w3273 w3292 w3306 w3321 w3334 w3344 w3348 w3371 w3385 w3392 w3404 w3416 w3427 w3430] -> w81
      tunnel: w77 -> [_ _ _ _ _ _ _ _ _ _ _ _ _ _ _ _ _ _ _ _ w1014 _ _ _ _ _ _ _ _ _ _ _ _ _ _ _ _ _ _ _ _ _ _ _ _ _ _ _ _ _ _ _ _ _ _ _ _ _ _ _ _ _ _ _ _ _ _ _ _ _ _ _ w1939 w1948 _ _ _ _ _ _ _ _ _ _ _ _ _ _ _ _ _ _ _ _ _ _ _ _ _ _ _ _ _ _ _ _ _ _ _ _ _ _ _ _ _ _ _ _ _ _ _ _ _ _ _ _ _ _ _ _ _ _ _ _ _ _ _ _ _ _ _ _ _ _ _ _ _ _ _ _ _ _ _ _ _ _ _ _ _ _ _ _ _ _ _ _ _ _ _ _ _ _ _ _ _ _ _ _ _ _ _ _]
      tunnel: w71 -> [_ _ _ _ _ _ _ _ _ _ _ _ _ _ _ _ _ _ _ _ _ _ _ _ _ _ _ _ _ _ _ _ _ _ _ _ _ _ _ _ _ _ _ _ _ _ _ _ _ _ _ _ _ _ _ _ _ _ _ _ _ _ _ _ _ _ _ _ _ _ _ _ _ _ _ _ _ _ _ _ _ _ _ _ _ _ _ _ _ _ _ _ _ _ _ _ _ _ _ _ _ _ _ _ _ _ _ _ _ _ _ _ _ _ _ _ _ _ _ _ _ _ _ _ _ _ _ _ _ _ _ _ _ _ _ _ _ _ _ _ _ _ _ _ _ _ _ _ _ _ _ _ _ _ _ _ _ _ _ _ _ _ _ _ _ _ _ _ _ _ _ _ _ _ _ w3368 w3382 _ _ _ _ _]
      frame "", "Event Structure", "Idle" {
        # "executes when the state queue is empty"
        n32 = event shown="[37] <AcqLoop error?>: User Event" {
          selector: w95 -> [_ _ _ _ _ _ _ _ _ _ _ _ _ _ _ _ _ _ _ _ _ _ _ _ _ _ _ _ _ _ _ _ _ _ _ _ _ _ _]
          dyn-events: [_ _ _ _ _ _ _ _ _ _ _ _ _ _ _ _ _ _ _ _ _ _ _ _ _ _ _ _ _ _ _ _ _ _ _ _ _ _ _] -> w94
          timeout: w97 -> [_ _ _ _ _ _ _ _ _ _ _ _ _ _ _ _ _ _ _ _ _ _ _ _ _ _ _ _ _ _ _ _ _ _ _ _ _ _ _]
          tunnel: w102 -> [w122 w140 w149 w157 w161 w165 w173 w179 w187 w195 w205 w212 w241 w261 w281 w301 w305 w312 w335 w349 w363 w377 w382 w385 w391 w398 w405 w411 w417 w423 w430 w443 w454 w466 w473 w477 w481 w497 w513]
          tunnel: [w123 w139 w149 w156 w161 w164 w173 w179 w187 w195 w205 w211 w241 w261 w281 w301 w305 w311 w335 w349 w363 w377 w381 w384 w391 w399 w406 w410 w416 w423 w431 w444 w454 w467 w473 w477 w480 w498 w512] -> w101
          tunnel: w100 -> [w106 w142 w147 w151 w159 w166 w172 w180 w188 w196 w203 w207 w239 w259 w279 w299 w303 w307 w334 w348 w362 w376 w378 w386 w389 w394 w401 w413 w418 w421 w425 w438 w452 w462 w471 w475 w482 w495 w510]
          tunnel: [w121 w143 w148 w152 w160 w167 w171 w178 w186 w194 w204 w213 w240 w260 w280 w300 w304 w313 w332 w336 w359 w374 w380 w387 w390 w395 w402 w414 w419 w422 w429 w442 w453 w463 w472 w476 w483 w499 w511] -> w93
          tunnel: w99 -> [w121 w143 w148 w152 w160 w167 w171 w178 w186 w194 w204 w213 w240 w260 w280 w300 w304 w313 w329 w338 w350 w366 w380 w387 w390 w395 w402 w414 w419 w422 w429 w442 w453 w465 w472 w476 w483 w499 w511]
          tunnel: [w106 w142 w147 w151 w159 w166 w172 w180 w188 w196 w203 w208 w239 w259 w279 w299 w303 w308 w334 w348 w362 w376 w378 w386 w389 w396 w403 w413 w418 w421 w426 w439 w452 w468 w471 w475 w482 w496 w510] -> w98
          tunnel: w96 -> [_ _ _ _ _ _ _ _ _ _ _ _ _ _ _ _ _ _ _ _ _ _ _ _ _ _ _ _ _ _ _ _ _ _ _ _ _ _ _]
          event Timeout {
            # "check system status every 2s"
            n33 = event-data() -> ()  [unwired: 1 in, 1 out]
            n34 = Unbundle By Name(w106) -> ("SysRunning?"=w104:bool, "SlowTimer"=w120:u32, "FastTimer"=w114:u32)
            n35 = Tick Count (ms)() -> (millisecond timer value=w107:u32)
            n36 = Subtract(x=w107, y=w120) -> (x-y=w117:u32)
            n37 = case shown="False" w104 {
              tunnel: ["" "Utility: AquiTimerCheck" ("State(s) in Front (\"\")")] -> w112
              frame False {
                # "if not running, do nothing"
              }
              frame True {
                # "if aquisition is running, check timer"
              }
            }
            n38 = Subtract(x=w107, y=w114) -> (x-y=w115:u32)
            n39 = Greater?(x=w117, y=u32 2000) -> (0:w118:bool)
            n40 = Greater?(x=w115, y=u32 500) -> (0:w105:bool)
            n41 = disable-structure shown="Disabled" {
              disable-tunnel: w105 -> [w128 _]
              disable-tunnel: w104 -> [w127 _]
              disable-tunnel: [w124 "" ("State(s) at Back (\"\")")] -> w103
              frame Disabled {
                n42 = Not(x=w127) -> (.not. x?=w126:bool)
                n43 = And(x=w128, y=w126) -> (x .and. y?=w125:bool)
                n44 = case shown="True" w125 {
                  tunnel: ["" ("Empty String Constant") "TCP: checkSource" ("State(s) in Front (\"\")")] -> w124
                  frame False {
                  }
                  frame True {
                  }
                }
              }
              frame Enabled {
              }
            }
            n45 = case shown="True" w118 {
              tunnel: ["" ("Empty String Constant") "SystemStatus: SlowSysStatusMacro" ("State(s) in Front (\"\")")] -> w110
              frame False {
              }
              frame True {
              }
            }
            n46 = case shown="True" w105 {
              tunnel: ["" ("Empty String Constant") "SystemStatus: FastSysStatusMacro" ("State(s) in Front (\"\")")] -> w108
              frame False {
              }
              frame True {
              }
            }
            n47 = call <vilib>:"Add State(s) to Queue__JKI_lib_State_Machine.vi"("State(s) in Front (\"\")"=w112, "State(s) in (\"\")"="LabJack: checkPedal" ("State(s) in Front (\"\")"), "State(s) at Back (\"\")"=w110) -> ("States Out"=w109:string)  [unwired: 12 in]
            n48 = call <vilib>:"Add State(s) to Queue__JKI_lib_State_Machine.vi"("State(s) in Front (\"\")"=w109, "State(s) in (\"\")"=w108, "State(s) at Back (\"\")"=w103) -> ("States Out"=w113:string)  [unwired: 12 in]
            n49 = call <vilib>:"Add State(s) to Queue__JKI_lib_State_Machine.vi"("State(s) in Front (\"\")"=w113, "State(s) in (\"\")"=w122) -> ("States Out"=w123:string)  [unwired: 13 in]
          }
          event "Live?": Value Change {
            n50 = event-data() -> ("NewVal"=w141:bool)  [unwired: 1 in, 5 out]
            n51 = case shown="True" w141 {
              tunnel: ["USBCAM: Stop" "USBCAM: StartNoSave"] -> w138
              frame False {
              }
              frame True {
              }
            }
            n52 = call <vilib>:"Add State(s) to Queue__JKI_lib_State_Machine.vi"("State(s) in Front (\"\")"=w138, "State(s) in (\"\")"=w140) -> ("States Out"=w139:string)  [unwired: 13 in]
          }
          event "355nm Laser toggle": Mouse Enter {
            n53 = event-data() -> ()  [unwired: 1 in, 4 out]
            n54 = local write "Help"("Toggle 355nm laser." ("Help")) -> ()
          }
          event "355nm Laser toggle": Value Change {
            # "[Covers: REQ34]"
            n55 = event-data() -> ()  [unwired: 1 in, 6 out]
            n56 = Select(t="LabJack: 355_PWM_Start\nLabJack: AB_Start", s="355nm Laser toggle", f="LabJack: 355_PWM_Stop\nLabJack: AB_Stop") -> (s? t:f=w154:string)
            n57 = call <vilib>:"Add State(s) to Queue__JKI_lib_State_Machine.vi"("State(s) in Front (\"\")"=w154, "State(s) in (\"\")"=w157) -> ("States Out"=w156:string)  [unwired: 13 in]
          }
          event "Aiming beam toggle": Mouse Enter {
            n58 = event-data() -> ()  [unwired: 1 in, 4 out]
            n59 = local write "Help"("Toggle aiming beam laser." ("Help")) -> ()
          }
          event "Aiming beam toggle": Value Change {
            # "[Covers: REQ33]"
            n60 = event-data() -> ()  [unwired: 1 in, 6 out]
            n61 = case shown="True" "Aiming beam toggle" {
              tunnel: ["LabJack: AB_Stop" ("State(s) in Front (\"\")") "LabJack: AB_Start" ("State(s) in Front (\"\")")] -> w163
              frame False {
              }
              frame True {
              }
            }
            n62 = call <vilib>:"Add State(s) to Queue__JKI_lib_State_Machine.vi"("State(s) in Front (\"\")"=w163, "State(s) in (\"\")"=w165) -> ("States Out"=w164:string)  [unwired: 13 in]
          }
          event "Auto gain ch1": Value Change {
            n63 = event-data() -> ("NewVal"=w170:bool)  [unwired: 1 in, 5 out]
            n64 = case shown="True" w170 {
              frame False {
                n65 = local read "V 1"() -> (w174:dbl)
                n66 = call "V1FGV.vi"("action (write)"=enum16{"write", "read"}."write" ("action"), "V1 in"=w174) -> ()  [unwired: 8 in, 2 out]
                n67 = property on="V 1" class="DigNum (strict)"("DisabledEnum"=T12."Enabled" ("Disabled")) -> ()  [unwired: 2 in, 2 out]
              }
              frame True {
                n68 = property on="V 1" class="DigNum (strict)"("DisabledEnum"=T12."Disabled and Grayed Out" ("Disabled")) -> ()  [unwired: 2 in, 2 out]
              }
            }
          }
          event "Auto gain ch2": Value Change {
            n69 = event-data() -> ("NewVal"=w181:bool)  [unwired: 1 in, 5 out]
            n70 = case shown="False" w181 {
              frame False {
                n71 = local read "V 2"() -> (w182:dbl)
                n72 = property on="V 2" class="DigNum (strict)"("DisabledEnum"=T12."Enabled" ("Disabled")) -> ()  [unwired: 2 in, 2 out]
                n73 = call "V2FGV.vi"("action(write)"=enum16{"write", "read"}."write" ("action"), "V2 in"=w182) -> ()  [unwired: 8 in, 2 out]
              }
              frame True {
                n74 = property on="V 2" class="DigNum (strict)"("DisabledEnum"=T12."Disabled and Grayed Out" ("Disabled")) -> ()  [unwired: 2 in, 2 out]
              }
            }
          }
          event "Auto gain ch3": Value Change {
            n75 = event-data() -> ("NewVal"=w189:bool)  [unwired: 1 in, 5 out]
            n76 = case shown="False" w189 {
              frame False {
                n77 = local read "V 3"() -> (w190:dbl)
                n78 = property on="V 3" class="DigNum (strict)"("DisabledEnum"=T12."Enabled" ("Disabled")) -> ()  [unwired: 2 in, 2 out]
                n79 = call "V3FGV.vi"("action(write)"=enum16{"write", "read"}."write" ("action"), "V3 in"=w190) -> ()  [unwired: 8 in, 2 out]
              }
              frame True {
                n80 = property on="V 3" class="DigNum (strict)"("DisabledEnum"=T12."Disabled and Grayed Out" ("Disabled")) -> ()  [unwired: 2 in, 2 out]
              }
            }
          }
          event "Auto gain ch4": Value Change {
            n81 = event-data() -> ("NewVal"=w197:bool)  [unwired: 1 in, 5 out]
            n82 = case shown="False" w197 {
              frame False {
                n83 = local read "V 4"() -> (w198:dbl)
                n84 = property on="V 4" class="DigNum (strict)"("DisabledEnum"=T12."Enabled" ("Disabled")) -> ()  [unwired: 2 in, 2 out]
                n85 = call "V4FGV.vi"("action(write)"=enum16{"write", "read"}."write" ("action"), "V3 in"=w198) -> ()  [unwired: 8 in, 2 out]
              }
              frame True {
                n86 = property on="V 4" class="DigNum (strict)"("DisabledEnum"=T12."Disabled and Grayed Out" ("Disabled")) -> ()  [unwired: 2 in, 2 out]
              }
            }
          }
          event "Background": Mouse Enter {
            n87 = event-data() -> ()  [unwired: 1 in, 4 out]
            n88 = local write "Help"("Click to record a background." ("Help")) -> ()
          }
          event "Background": Value Change {
            n89 = event-data() -> ("NewVal"=w209:bool)  [unwired: 1 in, 5 out]
            n90 = case shown="True" w209 {
              tunnel: ["Utility: SetAllChanManualGain\nQueue: Flash\nUtility: Dewelling >> 2500\nLabJack: 355_PWM_Stop\nLabJack: AB_Stop" "Utility: SetDataClass >> Bg\nUI: Update\nLabJack: 355_PWM_Start\nLabJack: AB_Start\nUtility: SaveDeconChan\nUtility: Dewelling >> 50\nLabJack: SetV\nDigitizer: Start\nUtility: AquiTimerReset\nLED: BreathGreen\nUI: duringBGAcquire"] -> w210
              tunnel: [FALSE TRUE] -> w206
              frame False {
                n91 = local read "Skip Data Save?"() -> (w214:bool)
                n92 = case shown="False" w214 {
                  frame False {
                    n93 = property on="Background" class="Bool (strict)"("BoolText.Text"="Done!" ("Boolean Text.Text")) -> ()  [unwired: 2 in, 2 out]
                  }
                  frame True {
                  }
                }
              }
              frame True {
                # "[Covers: REQ6]"
                n94 = property on="Background" class="Bool (strict)"("BoolText.Text"="Running" ("Boolean Text.Text"), "Colors [4]"=cluster{u32, u32}[] [{6618880, 6618880}, {16711680, 16711680}]) -> ()  [unwired: 2 in, 2 out]
              }
            }
            n95 = Bundle By Name(cluster=w207, "SysRunning?"=w206) -> (w208:T27)
            n96 = call <vilib>:"Add State(s) to Queue__JKI_lib_State_Machine.vi"("State(s) in Front (\"\")"=w210, "State(s) in (\"\")"=w212) -> ("States Out"=w211:string)  [unwired: 13 in]
          }
          event "Channel 1": Cursor Move {
            n97 = event-data() -> ("CursIdx"=w225:i32, "CursLoc"=w237:cluster{"X":dbl, "Y":dbl})  [unwired: 1 in, 7 out]
            n98 = property on="Channel 3" class="WFGraph (strict)"() -> ("CrsrList"=w232:T28)  [unwired: 2 in, 2 out]
            n99 = property on="Channel 4" class="WFGraph (strict)"() -> ("CrsrList"=w224:T28)  [unwired: 2 in, 2 out]
            n100 = property on="Channel 2" class="WFGraph (strict)"() -> ("CrsrList"=w235:T28)  [unwired: 2 in, 2 out]
            n101 = Index Array(array=w232, index=w225) -> (element=w236:T29)
            n102 = Index Array(array=w224, index=w225) -> (element=w227:T29)
            n103 = Unbundle By Name(w237) -> ("X"=w226:dbl)
            n104 = Index Array(array=w235, index=w225) -> (element=w238:T29)
            n105 = Bundle By Name(cluster=w236, "Position.X"=w226) -> (w231:T29)
            n106 = Bundle By Name(cluster=w227, "Position.X"=w226) -> (w223:T29)
            n107 = Bundle By Name(cluster=w238, "Position.X"=w226) -> (w234:T29)
            n108 = control-ref of="Channel 1"() -> (w228:refnum<vi>)
            n109 = Replace Array Subset(array=w232, new element=w231, index=w225) -> (w230:T28)
            n110 = Replace Array Subset(array=w224, new element=w223, index=w225) -> (w222:T28)
            n111 = Replace Array Subset(array=w235, new element=w234, index=w225) -> (w233:T28)
            n112 = property on="Channel 3" class="WFGraph (strict)"("CrsrList"=w230) -> (error out=w229:errorcluster)  [unwired: 2 in, 1 out]
            n113 = property on="Channel 4" class="WFGraph (strict)"("CrsrList"=w222) -> ()  [unwired: 2 in, 2 out]
            n114 = property on="Channel 2" class="WFGraph (strict)"("CrsrList"=w233) -> ()  [unwired: 2 in, 2 out]
            n115 = call "UpdateCurserIdx(SubVI).vi"("error in (no error)"=w229, "WaveformGraph in"=w228) -> ()  [unwired: 9 in, 1 out]
          }
          event "Channel 2": Cursor Move {
            n116 = event-data() -> ("CursIdx"=w244:i32, "CursLoc"=w258:cluster{"X":dbl, "Y":dbl})  [unwired: 1 in, 7 out]
            n117 = Unbundle By Name(w258) -> ("X"=w246:dbl)
            n118 = property on="Channel 1" class="WFGraph (strict)"() -> ("CrsrList"=w252:T28)  [unwired: 2 in, 2 out]
            n119 = property on="Channel 3" class="WFGraph (strict)"() -> ("CrsrList"=w254:T28)  [unwired: 2 in, 2 out]
            n120 = property on="Channel 4" class="WFGraph (strict)"() -> ("CrsrList"=w245:T28)  [unwired: 2 in, 2 out]
            n121 = Index Array(array=w252, index=w244) -> (element=w257:T29)
            n122 = Index Array(array=w254, index=w244) -> (element=w256:T29)
            n123 = Index Array(array=w245, index=w244) -> (element=w247:T29)
            n124 = Bundle By Name(cluster=w247, "Position.X"=w246) -> (w243:T29)
            n125 = Bundle By Name(cluster=w257, "Position.X"=w246) -> (w255:T29)
            n126 = Bundle By Name(cluster=w256, "Position.X"=w246) -> (w253:T29)
            n127 = Replace Array Subset(array=w252, new element=w255, index=w244) -> (w251:T28)
            n128 = Replace Array Subset(array=w254, new element=w253, index=w244) -> (w250:T28)
            n129 = Replace Array Subset(array=w245, new element=w243, index=w244) -> (w242:T28)
            n130 = control-ref of="Channel 1"() -> (w249:refnum<vi>)
            n131 = property on="Channel 1" class="WFGraph (strict)"("CrsrList"=w251) -> ()  [unwired: 2 in, 2 out]
            n132 = property on="Channel 3" class="WFGraph (strict)"("CrsrList"=w250) -> (error out=w248:errorcluster)  [unwired: 2 in, 1 out]
            n133 = property on="Channel 4" class="WFGraph (strict)"("CrsrList"=w242) -> ()  [unwired: 2 in, 2 out]
            n134 = call "UpdateCurserIdx(SubVI).vi"("error in (no error)"=w248, "WaveformGraph in"=w249) -> ()  [unwired: 9 in, 1 out]
          }
          event "Channel 3": Cursor Move {
            n135 = event-data() -> ("CursIdx"=w264:i32, "CursLoc"=w278:cluster{"X":dbl, "Y":dbl})  [unwired: 1 in, 7 out]
            n136 = Unbundle By Name(w278) -> ("X"=w266:dbl)
            n137 = property on="Channel 4" class="WFGraph (strict)"() -> ("CrsrList"=w265:T28)  [unwired: 2 in, 2 out]
            n138 = property on="Channel 1" class="WFGraph (strict)"() -> ("CrsrList"=w275:T28)  [unwired: 2 in, 2 out]
            n139 = property on="Channel 2" class="WFGraph (strict)"() -> ("CrsrList"=w273:T28)  [unwired: 2 in, 2 out]
            n140 = Index Array(array=w265, index=w264) -> (element=w267:T29)
            n141 = Index Array(array=w275, index=w264) -> (element=w277:T29)
            n142 = Index Array(array=w273, index=w264) -> (element=w276:T29)
            n143 = Bundle By Name(cluster=w267, "Position.X"=w266) -> (w263:T29)
            n144 = Bundle By Name(cluster=w277, "Position.X"=w266) -> (w274:T29)
            n145 = Bundle By Name(cluster=w276, "Position.X"=w266) -> (w272:T29)
            n146 = Replace Array Subset(array=w265, new element=w263, index=w264) -> (w262:T28)
            n147 = Replace Array Subset(array=w275, new element=w274, index=w264) -> (w271:T28)
            n148 = Replace Array Subset(array=w273, new element=w272, index=w264) -> (w270:T28)
            n149 = control-ref of="Channel 1"() -> (w268:refnum<vi>)
            n150 = property on="Channel 4" class="WFGraph (strict)"("CrsrList"=w262) -> ()  [unwired: 2 in, 2 out]
            n151 = property on="Channel 1" class="WFGraph (strict)"("CrsrList"=w271) -> ()  [unwired: 2 in, 2 out]
            n152 = property on="Channel 2" class="WFGraph (strict)"("CrsrList"=w270) -> (error out=w269:errorcluster)  [unwired: 2 in, 1 out]
            n153 = call "UpdateCurserIdx(SubVI).vi"("error in (no error)"=w269, "WaveformGraph in"=w268) -> ()  [unwired: 9 in, 1 out]
          }
          event "Channel 4": Cursor Move {
            n154 = event-data() -> ("CursIdx"=w286:i32, "CursLoc"=w298:cluster{"X":dbl, "Y":dbl})  [unwired: 1 in, 7 out]
            n155 = Unbundle By Name(w298) -> ("X"=w284:dbl)
            n156 = property on="Channel 1" class="WFGraph (strict)"() -> ("CrsrList"=w296:T28)  [unwired: 2 in, 2 out]
            n157 = property on="Channel 2" class="WFGraph (strict)"() -> ("CrsrList"=w292:T28)  [unwired: 2 in, 2 out]
            n158 = property on="Channel 3" class="WFGraph (strict)"() -> ("CrsrList"=w287:T28)  [unwired: 2 in, 2 out]
            n159 = Index Array(array=w296, index=w286) -> (element=w297:T29)
            n160 = Index Array(array=w292, index=w286) -> (element=w293:T29)
            n161 = Index Array(array=w287, index=w286) -> (element=w289:T29)
            n162 = Bundle By Name(cluster=w297, "Position.X"=w284) -> (w295:T29)
            n163 = Bundle By Name(cluster=w293, "Position.X"=w284) -> (w291:T29)
            n164 = Bundle By Name(cluster=w289, "Position.X"=w284) -> (w288:T29)
            n165 = Replace Array Subset(array=w296, new element=w295, index=w286) -> (w294:T28)
            n166 = Replace Array Subset(array=w292, new element=w291, index=w286) -> (w290:T28)
            n167 = Replace Array Subset(array=w287, new element=w288, index=w286) -> (w285:T28)
            n168 = control-ref of="Channel 1"() -> (w282:refnum<vi>)
            n169 = call "UpdateCurserIdx(SubVI).vi"() -> ()  [unwired: 11 in, 1 out]
            n170 = call "UpdateCurserIdx(SubVI).vi"() -> ()  [unwired: 11 in, 1 out]
            n171 = property on="Channel 1" class="WFGraph (strict)"("CrsrList"=w294) -> ()  [unwired: 2 in, 2 out]
            n172 = property on="Channel 2" class="WFGraph (strict)"("CrsrList"=w290) -> ()  [unwired: 2 in, 2 out]
            n173 = property on="Channel 3" class="WFGraph (strict)"("CrsrList"=w285) -> (error out=w283:errorcluster)  [unwired: 2 in, 1 out]
            n174 = call "UpdateCurserIdx(SubVI).vi"("error in (no error)"=w283, "WaveformGraph in"=w282) -> ()  [unwired: 9 in, 1 out]
          }
          event "Cali&iRF alignment": Mouse Enter {
            n175 = event-data() -> ()  [unwired: 1 in, 4 out]
            n176 = local write "Help"("Click to run system intensity calibration and irf alignment" ("Help")) -> ()
          }
          event "Cali&iRF alignment": Value Change {
            n177 = event-data() -> ("NewVal"=w309:bool)  [unwired: 1 in, 5 out]
            n178 = case shown="False" w309 {
              tunnel: ["Utility: SetAllChanManualGain\nQueue: Flash\nUtility: Dewelling >> 2500\nLabJack: 355_PWM_Stop\nLabJack: AB_Stop" "Utility: SetDataClass >> Cali\nUI: Update\nUtility: SaveDeconChan\nLabJack: 355_PWM_Start\nLabJack: AB_Start\nLabJack: SetV\nDigitizer: Start\nUtility: AquiTimerReset\nLED: BreathGreen\nUI: duringIRFAlign"] -> w310
              tunnel: [FALSE TRUE] -> w306
              frame False {
                n179 = local read "Skip Data Save?"() -> (w314:bool)
                n180 = case shown="False" w314 {
                  frame False {
                    n181 = property on="Cali&iRF alignment" class="Bool (strict)"("BoolText.Text"="Done!" ("Boolean Text.Text")) -> ()  [unwired: 2 in, 2 out]
                  }
                  frame True {
                  }
                }
              }
              frame True {
                n182 = property on="Cali&iRF alignment" class="Bool (strict)"("BoolText.Text"="Running" ("Boolean Text.Text"), "Colors [4]"=cluster{u32, u32}[] [{6618880, 6618880}, {16711680, 16711680}]) -> ()  [unwired: 2 in, 2 out]
              }
            }
            n183 = Bundle By Name(cluster=w307, "SysRunning?"=w306) -> (w308:T27)
            n184 = call <vilib>:"Add State(s) to Queue__JKI_lib_State_Machine.vi"("State(s) in Front (\"\")"=w310, "State(s) in (\"\")"=w312) -> ("States Out"=w311:string)  [unwired: 13 in]
          }
          event "V 1": Value Change {
            n185 = event-data() -> ()  [unwired: 1 in, 6 out]
            n186 = call "LabJack_FGV.vi"("Operation(Read)"=enum16{"Write", "Read"}."Read" ("Operation"), "error in (no error)"=w329) -> ("error out"=w326:errorcluster, "Read data"=w327:i32)  [unwired: 8 in]
            n187 = global read "GlobalVariables.vi" "Ch1 LJ pin"() -> (w325:string)
            n188 = call "LJM_eWriteName.vi"("Handle In"=w327, "Name"=w325, "Value"="V 1", "error in"=w326) -> ("error out"=w323:errorcluster)  [unwired: 10 in, 1 out]
            n189 = call "V1FGV.vi"("Error In"=w323, "action (write)"=enum16{"write", "read"}."write" ("action"), "V1 in"="V 1") -> ("Error Out"=w322:errorcluster)  [unwired: 7 in, 1 out]
            n190 = call "CtrlVtoGain.vi"("error in (no error)"=w322, "CtrlV(V)"="V 1", "Channel"=enum16{"Ch1", "Ch2", "Ch3"}."Ch1" ("Enum")) -> ("error out"=w332:errorcluster, "Gain"=w331:dbl)  [unwired: 7 in]
            n191 = local write "Gain1"(w331) -> ()
          }
          event "V 2": Value Change {
            n192 = event-data() -> ()  [unwired: 1 in, 6 out]
            n193 = call "LabJack_FGV.vi"("Operation(Read)"=enum16{"Write", "Read"}."Read" ("Operation"), "error in (no error)"=w338) -> ("error out"=w343:errorcluster, "Read data"=w344:i32)  [unwired: 8 in]
            n194 = global read "GlobalVariables.vi" "Ch2 LJ pin"() -> (w342:string)
            n195 = call "LJM_eWriteName.vi"("Handle In"=w344, "Name"=w342, "Value"="V 2", "error in"=w343) -> ("error out"=w341:errorcluster)  [unwired: 10 in, 1 out]
            n196 = call "V2FGV.vi"("Error In"=w341, "action(write)"=enum16{"write", "read"}."write" ("action"), "V2 in"="V 2") -> ("Error Out"=w340:errorcluster)  [unwired: 7 in, 1 out]
            n197 = call "CtrlVtoGain.vi"("error in (no error)"=w340, "CtrlV(V)"="V 2", "Channel"=enum16{"Ch1", "Ch2", "Ch3"}."Ch2" ("Enum")) -> ("error out"=w336:errorcluster, "Gain"=w337:dbl)  [unwired: 7 in]
            n198 = local write "Gain2"(w337) -> ()
          }
          event "V 3": Value Change {
            n199 = event-data() -> ()  [unwired: 1 in, 6 out]
            n200 = call "LabJack_FGV.vi"("Operation(Read)"=enum16{"Write", "Read"}."Read" ("Operation"), "error in (no error)"=w350) -> ("error out"=w355:errorcluster, "Read data"=w356:i32)  [unwired: 8 in]
            n201 = global read "GlobalVariables.vi" "Ch3 LJ pin"() -> (w354:string)
            n202 = call "LJM_eWriteName.vi"("Handle In"=w356, "Name"=w354, "Value"="V 3", "error in"=w355) -> ("error out"=w352:errorcluster)  [unwired: 10 in, 1 out]
            n203 = call "V3FGV.vi"("Error In"=w352, "action(write)"=enum16{"write", "read"}."write" ("action"), "V3 in"="V 3") -> ("Error Out"=w351:errorcluster)  [unwired: 7 in, 1 out]
            n204 = call "CtrlVtoGain.vi"("error in (no error)"=w351, "CtrlV(V)"="V 3", "Channel"=enum16{"Ch1", "Ch2", "Ch3"}."Ch3" ("Enum")) -> ("error out"=w359:errorcluster, "Gain"=w358:dbl)  [unwired: 7 in]
            n205 = local write "Gain3"(w358) -> ()
          }
          event "V 4": Value Change {
            n206 = event-data() -> ()  [unwired: 1 in, 6 out]
            n207 = call "LabJack_FGV.vi"("Operation(Read)"=enum16{"Write", "Read"}."Read" ("Operation"), "error in (no error)"=w366) -> ("error out"=w370:errorcluster, "Read data"=w371:i32)  [unwired: 8 in]
            n208 = global read "GlobalVariables.vi" "Ch4 LJ pin"() -> (w369:string)
            n209 = call "LJM_eWriteName.vi"("Handle In"=w371, "Name"=w369, "Value"="V 4", "error in"=w370) -> ("error out"=w368:errorcluster)  [unwired: 10 in, 1 out]
            n210 = call "V4FGV.vi"("Error In"=w368, "action(write)"=enum16{"write", "read"}."write" ("action"), "V3 in"="V 4") -> ("Error Out"=w367:errorcluster)  [unwired: 7 in, 1 out]
            n211 = call "CtrlVtoGain.vi"("error in (no error)"=w367, "CtrlV(V)"="V 4", "Channel"=enum16{"Ch1", "Ch2", "Ch3", "Ch4"}."Ch4") -> ("error out"=w374:errorcluster, "Gain"=w373:dbl)  [unwired: 7 in]
            n212 = local write "Gain4"(w373) -> ()
          }
          event "Quit": Value Change {
            # "Exit Button Value Change (pressed) Event\n(when pressed.  quite)"
            n213 = event-data() -> ()  [unwired: 1 in, 1 out]
            n214 = call <vilib>:"Add State(s) to Queue__JKI_lib_State_Machine.vi"("State(s) in Front (\"\")"="LED: Off\nMacro: Exit", "State(s) in (\"\")"=w382) -> ("States Out"=w381:string)  [unwired: 13 in]
          }
          event "Show BG": Value Change {
            n215 = event-data() -> ()  [unwired: 1 in, 6 out]
            n216 = call <vilib>:"Add State(s) to Queue__JKI_lib_State_Machine.vi"("State(s) in Front (\"\")"="Data: showBG" ("State(s) in Front (\"\")"), "State(s) in (\"\")"=w385) -> ("States Out"=w384:string)  [unwired: 13 in]
          }
          event "StartButton": Mouse Enter {
            n217 = event-data() -> ()  [unwired: 1 in, 4 out]
            n218 = local write "Help"("Press to start aquisition." ("Help")) -> ()
          }
          event "StartButton": Value Change {
            # "[Covers: REQ32]"
            # "start PWM before acquisition"
            # "Initialize both digitizer aquisition and\n send user event to trigger aquisition loop"
            n219 = event-data() -> ()  [unwired: 1 in, 6 out]
            n220 = local write "StartButton"(FALSE ("StartButton")) -> ()
            n221 = Bundle By Name(cluster=w394, "SysRunning?"=TRUE) -> (w396:T27)
            n222 = call <vilib>:"Add State(s) to Queue__JKI_lib_State_Machine.vi"("State(s) in Front (\"\")"="/*TCP: stopCam\nUSBCAM: Stop\nUtility: SetDataClass >> Data\nQueue: Flash\nUI: Update\nUSBCAM: StartAndSave\nUtility: StartBeep\nLabJack: 355_PWM_Start\nLabJack: AB_Start\nLabJack: SetV\nDigitizer: Start\nUtility: AquiTimerReset\nUI: DuringAquisition\nLED: BreathGreen\n/*TCP: sendRunNum\n/*TCP: sendVideoSource\n/*TCP: sendChannel\n/*TCP: startRun", "State(s) in (\"\")"=w398) -> ("States Out"=w399:string)  [unwired: 13 in]
          }
          event User Event {
            # "[Covers: REQ32]"
            # "start PWM before acquisition"
            # "Initialize both digitizer aquisition and\n send user event to trigger aquisition loop"
            n223 = event-data() -> ()  [unwired: 1 in, 5 out]
            n224 = Bundle By Name(cluster=w401, "SysRunning?"=TRUE) -> (w403:T27)
            n225 = call <vilib>:"Add State(s) to Queue__JKI_lib_State_Machine.vi"("State(s) in Front (\"\")"="/*TCP: stopCam\nUtility: SetDataClass >> Data\nQueue: Flash\nUI: Update\nUtility: StartBeep\nLabJack: 355_PWM_Start\nLabJack: AB_Start\nLabJack: SetV\nDigitizer: Start\nUtility: AquiTimerReset\nUI: DuringAquisition\nLED: BreathGreen\n/*TCP: sendRunNum\n/*TCP: sendVideoSource\n/*TCP: sendChannel\n/*TCP: startRun", "State(s) in (\"\")"=w405) -> ("States Out"=w406:string)  [unwired: 13 in]
          }
          event "Video Display": Value Change {
            n226 = event-data() -> ("NewVal"=w412:bool)  [unwired: 1 in, 5 out]
            n227 = Select(t="/*TCP: startCam", s=w412, f="/*TCP: stopCam") -> (s? t:f=w409:string)
            n228 = call <vilib>:"Add State(s) to Queue__JKI_lib_State_Machine.vi"("State(s) in (\"\")"=w411, "State(s) at Back (\"\")"=w409) -> ("States Out"=w410:string)  [unwired: 13 in]
          }
          event "Video Source": Value Change {
            n229 = event-data() -> ()  [unwired: 1 in, 6 out]
            n230 = call <vilib>:"Add State(s) to Queue__JKI_lib_State_Machine.vi"("State(s) in Front (\"\")"="TCP: sendVideoSource" ("State(s) in Front (\"\")"), "State(s) in (\"\")"=w417) -> ("States Out"=w416:string)  [unwired: 13 in]
          }
          event "StopButton": Mouse Enter {
            n231 = event-data() -> ()  [unwired: 1 in, 4 out]
            n232 = local write "Help"("Press to stop data aquisition." ("Help")) -> ()
          }
          event "StopButton": Value Change {
            # "if system is running, send stop command, if not do nothing."
            # "stop aquisition\nupdate UI"
            n233 = event-data() -> ()  [unwired: 1 in, 6 out]
            n234 = Unbundle By Name(w425) -> ("SysRunning?"=w427:bool)
            n235 = case shown="True" w427 {
              tunnel: ["" ("Empty String Constant") "LabJack: AB_Stop\nLabJack: 355_PWM_Stop\n/*Digitizer: Abort"] -> w428
              tunnel: w425 -> [w432 w436]
              tunnel: [w432 w435] -> w426
              frame False {
              }
              frame True {
                n236 = Bundle By Name(cluster=w436, "SysRunning?"=FALSE) -> (w435:T27)
              }
            }
            n237 = call <vilib>:"Add State(s) to Queue__JKI_lib_State_Machine.vi"("State(s) in Front (\"\")"=w428, "State(s) in (\"\")"=w430) -> ("States Out"=w431:string)  [unwired: 13 in]
            n238 = local write "StopButton"(FALSE ("StopButton")) -> ()
          }
          event User Event {
            # "if system is running, send stop command, if not do nothing."
            # "stop aquisition\nupdate UI"
            n239 = event-data() -> ()  [unwired: 1 in, 5 out]
            n240 = Unbundle By Name(w438) -> ("SysRunning?"=w440:bool)
            n241 = case shown="True" w440 {
              tunnel: ["" ("Empty String Constant") "LabJack: AB_Stop\nLabJack: 355_PWM_Stop\n/*Digitizer: Abort"] -> w441
              tunnel: w438 -> [w445 w449]
              tunnel: [w445 w448] -> w439
              frame False {
              }
              frame True {
                n242 = Bundle By Name(cluster=w449, "SysRunning?"=FALSE) -> (w448:T27)
              }
            }
            n243 = call <vilib>:"Add State(s) to Queue__JKI_lib_State_Machine.vi"("State(s) in Front (\"\")"=w441, "State(s) in (\"\")"=w443) -> ("States Out"=w444:string)  [unwired: 13 in]
          }
          event "Sys Reconfig": Mouse Enter {
            n244 = event-data() -> ()  [unwired: 1 in, 4 out]
            n245 = local write "Help"("Click to reconfig digitizer settings." ("Help")) -> ()
          }
          event "Sys Reconfig": Value Change {
            # "everytime the user change data aquisition setting, need to reinitilize decon engine and realign iRF.\ncheck whether data length has changed, if changed, reinitialize Decon engine\nreset BG ready, need a new BG"
            # "update DAQ FGV"
            n246 = event-data() -> ()  [unwired: 1 in, 6 out]
            n247 = call "SystemConfigEditorV6.vi"("error in"=w465) -> ("error out"=w464:errorcluster, "FLImDAQ out"=w459:T7)  [unwired: 1 in]
            n248 = Unbundle By Name(w462) -> ("FLImDAQ.min record length"=w461:i32)
            n249 = Unbundle By Name(w459) -> ("min record length"=w460:i32)
            n250 = call "FLImDAQ_FGV.vi"("error in (no error)"=w464, "Operation (Read)"=enum16{"Write", "Read"}."Write" ("Operation"), "Write data"=w459) -> ("error out"=w463:errorcluster, "Read data"=w458:T7)  [unwired: 7 in]
            n251 = Equal?(x=w461, y=w460) -> (x = y?=w457:bool)
            n252 = case shown="False" w457 {
              tunnel: ["UI: Cursor Set >> Busy\nDigitizer: Config\nDeconEngine: InitializeCh1\nDeconEngine: InitializeCh2\nDeconEngine: InitializeCh3\nUI: CaliAndiRFNotReady\n/*UI iRF not ready\nUI: Update\nUI: Cursor Set >> Idle" "UI: Cursor Set >> Busy\nDigitizer: Config\nUI: Update\nUI: Cursor Set >> Idle"] -> w456
              frame False {
              }
              frame True {
              }
            }
            n253 = Bundle By Name(cluster=w462, "FLImDAQ"=w458) -> (w468:T27)
            n254 = call <vilib>:"Add State(s) to Queue__JKI_lib_State_Machine.vi"("State(s) in Front (\"\")"=w456, "State(s) in (\"\")"=w466) -> ("States Out"=w467:string)  [unwired: 13 in]
          }
          event "System Hardware Connection Status", "StartButton", "StopButton", "355nm Laser toggle", "Aiming beam toggle", "Cali&iRF alignment", "Background", "Sys Reconfig": Mouse Leave {
            n255 = event-data() -> ()  [unwired: 1 in, 4 out]
            n256 = invoke on="Help" class="Str" method="Reinit To Default"() -> ()  [unwired: 3 in, 3 out]
          }
          event "System Hardware Connection Status.Digitizer": Mouse Enter {
            n257 = event-data() -> ()  [unwired: 1 in, 4 out]
            n258 = local write "Help"("Status of hardware connections. TCP/IP is optional." ("Help")) -> ()
          }
          event "TCP Connect": Value Change {
            n259 = event-data() -> ("NewVal"=w478:bool)  [unwired: 1 in, 5 out]
            n260 = case shown="False" w478 {
              tunnel: ["/*TCP: Close\nUI: Update" ("State(s) in Front (\"\")") "/*TCP: SendSettingMacro\nUI: Update" ("State(s) in Front (\"\")")] -> w479
              frame False {
              }
              frame True {
              }
            }
            n261 = call <vilib>:"Add State(s) to Queue__JKI_lib_State_Machine.vi"("State(s) in Front (\"\")"=w479, "State(s) in (\"\")"=w481) -> ("States Out"=w480:string)  [unwired: 13 in]
          }
          event User Event {
            # "if aquisition loop is error out. Stop digitizer, update front panel indicator, stop both laser and \nOption 1: parse and save data\nOption 2: Flash queue if scout run. [Covers: REQ23]"
            n262 = event-data() -> ()  [unwired: 1 in, 5 out]
            n263 = case shown="\"Data\", Default" "Data Class" {
              tunnel: [w503 "UI: Cursor Set >> Busy\nUtility: SetAllChanAutoGain\nUtility: RestoreDeConChan\nData: parseRunData\nData: irfAlignment\nUI: Cursor Set >> Idle" "UI: Cursor Set >> Busy\nUtility: SetAllChanAutoGain\nUtility: RestoreDeConChan\nData: parseRunData\nData: saveBGtoFGV\nData: saveBGtoFile\nUI: Cursor Set >> Idle\nData: showBG\nRun: BGIncrement"] -> w493
              frame "Data", Default {
                n264 = local read "Video Display"() -> (w505:bool)
                n265 = Select(t="/*TCP: startCam", s=w505, f="") -> (s? t:f=w501:string)
                n266 = call <vilib>:"Add State(s) to Queue__JKI_lib_State_Machine.vi"("State(s) in Front (\"\")"="UI: Cursor Set >> Busy\nData: parseRunData\nData: saveRunData\nUI: Cursor Set>>Idle" ("State(s) in Front (\"\")"), "State(s) in (\"\")"=w501) -> ("States Out"=w503:string)  [unwired: 13 in]
              }
              frame "Cali" {
              }
              frame "BG" {
              }
            }
            n267 = Bundle By Name(cluster=w495, "SysRunning?"=FALSE) -> (w496:T27)
            n268 = Select(t="" ("State(s) in Front (\"\")"), s="Skip Data Save?", f=w493) -> (s? t:f=w490:string)
            n269 = call <vilib>:"Add State(s) to Queue__JKI_lib_State_Machine.vi"("State(s) in Front (\"\")"="/*TCP: stopRun\nUI: Update\nUSBCAM: Stop\nDigitizer: Abort\nLabJack: ZeroV\nUtility: EndBeep\nLED: BreathOff\n" ("State(s) in Front (\"\")"), "State(s) in (\"\")"=w490, "State(s) at Back (\"\")"="Macro: SysReadyForAq\nUI: Update\nUSBCAM: StartNoSave" ("State(s) in Front (\"\")")) -> ("States Out"=w488:string)  [unwired: 12 in]
            n270 = call <vilib>:"Add State(s) to Queue__JKI_lib_State_Machine.vi"("State(s) in Front (\"\")"=w488, "State(s) in (\"\")"=w497) -> ("States Out"=w498:string)  [unwired: 13 in]
          }
          event Panel Close? {
            # "Discard the event because we'll close the front panel ourselves in Macro: Exit"
            # "Close Panel button (pressed) Event\n(this executes Macro: Exit to terminate the VI)"
            n271 = event-data() -> ()  [unwired: 1 in, 1 out]
            n272 = call <vilib>:"Add State(s) to Queue__JKI_lib_State_Machine.vi"("State(s) in Front (\"\")"="Macro: Exit", "State(s) in (\"\")"=w513) -> ("States Out"=w512:string)  [unwired: 13 in]
            n273 = event-data ("Event Filter Node")("Discard?"=TRUE) -> ()  [unwired: 1 in, 1 out]
          }
        }
      }
      frame "---------- Macro ----------" {
        # "Do not put any code in this frame.\n(It is a separator no-op. You can make a copy of this frame to create a new Macro frame)"
        n274 = call <vilib>:"Add State(s) to Queue__JKI_lib_State_Machine.vi"("State(s) in (\"\")"=w518) -> ("States Out"=w517:string)  [unwired: 14 in]
      }
      frame "Macro: Initialize" {
        # "load Labjack setting 1st as it contaisn laser pin infortmation"
        # "start laser 1st, need 7.5s for laser to get ready"
        # "Initialization Macro\n(This is called once, when the VI starts)"
        n275 = call <vilib>:"Add State(s) to Queue__JKI_lib_State_Machine.vi"("State(s) in Front (\"\")"="UI: showDisclaimer\nUI: Cursor Set >> Busy\nData: Initialize\nInitialize Core Data\nUI: Initialize\nUI: Front Panel State >> Open\nMacro: LoadSysConfig\nUSBCAM: Init\nUSBCAM: Config\n/*TCP: InitializeNew\n/*TCP: checkSource\nUI: Update\nLabJack: Open\nLabJack: SetDefaultSub\nLED: OpenVIRef\nLED: BreathOrange\nUI: Update\n355 Laser: CheckControllerStatus\n355 Laser: Laser enable\n355 Laser: Dewelling>>500\n355 Laser: CheckControllerStatus\nUI: Update\nLabJack: 355_PWM_Config\nLabJack: AB_PWM_Config\nUI: Update", "State(s) in (\"\")"="Digitizer: Initialize\nDigitizer: Config\nUI: Update\nAimingBeam: Initialize\nAimingBeam: Set Status>>Enable\nAimingBeam: Set Current\nUI: Update\n355 Laser: Check Dewelling\nUI: Cursor Set >> Idle\nCase: GetID\nUI: Update\n/*TCP: SendSettingMacro\nCase: CreatFileStruct\nUI: Update\nData: loadLastUseMacro\nDeconEngine: InitilizeMacro\nGraph: SetXMultiplier\nGraph: AddCursors\nAPD: Initialize\nAPD: LoadFromSerial\nAPD: UpdateCtrlVLimit\nAPD: GetGainLimits\nPID: loadPID\nLED: BreathOff\nUSBCAM: StartNoSave\nMacro: SysReadyForAq") -> ("States Out"=w519:string)  [unwired: 13 in]
        n276 = call <vilib>:"Add State(s) to Queue__JKI_lib_State_Machine.vi"("State(s) in Front (\"\")"=w519, "State(s) in (\"\")"=w527) -> ("States Out"=w526:string)  [unwired: 13 in]
        "Help" <- "Hover over controls to see help!" ("Help")
      }
      frame "Macro: LoadSysConfig" {
        # "System configuration Macro. [Covers: REQ15]\n(Load configurations for different component of the system)"
        n277 = call <vilib>:"Add State(s) to Queue__JKI_lib_State_Machine.vi"("State(s) in Front (\"\")"="SysConfig: Load Sys Config\nSysConfig: Load Digitizer Setting\nSysConfig: Load AB setting\nSysConfig: Load LJ Pinout\nSysConfig: Load 355 PWM\nSysConfig: LoadAPDSerialNumber\nSysConfig: LoadABVideoSetting\nSysConfig: LoadCursorLocation", "State(s) in (\"\")"=w533) -> ("States Out"=w532:string)  [unwired: 13 in]
      }
      frame "Macro: SysReadyForAq" {
        # "Macro for system ready\n(It is a separator no-op. You can make a copy of this frame to create a new Macro frame)"
        n278 = call <vilib>:"Add State(s) to Queue__JKI_lib_State_Machine.vi"("State(s) in Front (\"\")"="UI: ReadyForAquisition\nLED: Green" ("State(s) in Front (\"\")"), "State(s) in (\"\")"=w539) -> ("States Out"=w538:string)  [unwired: 13 in]
      }
      frame "Macro: Exit" {
        # "close LJ last"
        # "check whether hardware is initilized, if so close, if not do nothing"
        # "Exit Macro, close all hardware\n(This is called once, when the VI exits)"
        n279 = Unbundle By Name(w558) -> ("System Status.Digitizer"=w554:bool, "System Status.Aiming Beam"=w553:bool, "System Status.355 Laser"=w552:bool, "System Status.Labjack"=w543:bool, "Core.Close Panel on Exit?"=w547:bool)
        n280 = case shown="True" w554 {
          tunnel: ["" ("Empty String Constant") "Digitizer: Close"] -> w549
          frame False {
          }
          frame True {
          }
        }
        n281 = case shown="True" w543 {
          tunnel: ["" ("Empty String Constant") "LabJack: SetDefaultAndClose"] -> w540
          frame False {
          }
          frame True {
          }
        }
        n282 = case shown="True" w553 {
          tunnel: ["" ("Empty String Constant") w565] -> w542
          frame False {
          }
          frame True {
            w565 = "AimingBeam: Set Status >> Disable\nAimingBeam: Close"  # AimingBeam: Set Status >> Disable AimingBeam: Close
          }
        }
        n283 = case shown="True" w552 {
          tunnel: ["" ("Empty String Constant") "355 Laser: Close\n355 Laser: CheckControllerStatus"] -> w541
          frame False {
          }
          frame True {
          }
        }
        n284 = Select(t="UI: Front Panel State >> Close", s=w547, f="" ("Empty String Constant")) -> (s? t:f=w544:string)
        n285 = call <vilib>:"Add State(s) to Queue__JKI_lib_State_Machine.vi"("State(s) in Front (\"\")"="USBCAM: Close", "State(s) in (\"\")"=w549, "State(s) at Back (\"\")"=w542) -> ("States Out"=w551:string)  [unwired: 12 in]
        n286 = call <vilib>:"Add State(s) to Queue__JKI_lib_State_Machine.vi"("State(s) in Front (\"\")"=w551, "State(s) in (\"\")"=w541, "State(s) at Back (\"\")"=w540) -> ("States Out"=w546:string)  [unwired: 12 in]
        n287 = call <vilib>:"Add State(s) to Queue__JKI_lib_State_Machine.vi"("State(s) in Front (\"\")"=w546, "State(s) in (\"\")"="UI: Update\nUI: Reset\nGraph: SaveCursorLoc\nLED: CloseVIRef\nQueue: Destory\nData: Cleanup\nExit", "State(s) at Back (\"\")"=w544) -> ("States Out"=w555:string)  [unwired: 12 in]
        n288 = call <vilib>:"Add State(s) to Queue__JKI_lib_State_Machine.vi"("State(s) in Front (\"\")"=w555, "State(s) in (\"\")"=w561) -> ("States Out"=w560:string)  [unwired: 13 in]
      }
      frame "---------- Data ----------" {
        # "Do not put any code in this frame.\n(It is a separator no-op. You can make a copy of this frame to create a new Data frame)"
        n289 = call <vilib>:"Add State(s) to Queue__JKI_lib_State_Machine.vi"("State(s) in (\"\")"=w574) -> ("States Out"=w573:string)  [unwired: 14 in]
      }
      frame "Data: Initialize" {
        w575 = path ""  # CaliPath
        w576 = dbl[] []  # V4
        w577 = dbl[][] []  # Ch4Data
        w578 = FALSE  # bothVidSourceAvail
        w579 = T2 {"Main Frame Grabber"=FALSE, "Side Frame Grabber"=FALSE, "Main Camera"=FALSE, "Side Camera"=FALSE}  # video source
        w580 = FALSE  # LED vi ref open?
        w582 = T26 {"DeCon Channel"=enum."1", "Scale Bar"=FALSE, "Scale Low"=3.0, "Scale High"=8.0, "ANSI"=20.0, "Radius"=1.0, "3D?"=FALSE, "Firefly?"=FALSE, "Pentero?"=FALSE}  # VideoConfig
        w583 = T30 {"Ch1APDSerial#"="", "Ch2APDSerial#"="", "Ch3APDSerial#"="", "Ch4APDSerial#"=""}  # APDSerialNum
        w584 = u32 0  # Aquisition Timer
        w585 = cluster{"RunID":i8, "BG ID":i8, "Cali ID":i8} {"RunID"=1, "BG ID"=1, "Cali ID"=1}  # IDs
        w586 = refnum<vi> refnum  # LED vi reference
        w587 = path ""  # TempPath
        w588 = T31 {"DataPath"=path "", "BG Path"=path "", "iRFPath"=path "", "CaliPath"=path ""}  # Pathes
        w590 = dbl[] []  # V3
        w591 = dbl[] []  # V2
        w592 = dbl[] []  # V1
        w594 = u32 0  # FastTimer
        w595 = u32 0  # SlowTimer
        w596 = dbl[][] []  # Ch3Data
        w597 = dbl[][] []  # Ch2Data
        w581 = dbl[][] []  # Ch1Data
        w600 = T3 {"Digitizer"=FALSE, "Labjack"=FALSE, "Aiming Beam"=FALSE, "355 Laser"=FALSE, "TCP/IP"=FALSE}  # System Status
        w601 = T32 {"DIO_EF_CLOCK1_DIVISOR"=16, "DIO_EF_CLOCK1_ROLL_VALUE"=25000, "DIO#_EF_INDEX"=0, "DIO#_EF_OPTIONS"=1, "DIO#_EF_CONFIG_A"=6250}  # AB PWM setting
        w602 = T6 {"Ch1 Bias"="TDA11", "Ch2 Bias"="DAC10", "Ch3 Bias"="DAC0", "Ch4 Bias"="DAC0", "355 PWM"="FIO0", "AimingBeam PWM"="FIO2", "Laser Ready"="FIO3", "Interlock"="FIO1", "Laser Start/Stop"="FIO1", "Red LED"="FIO1", "Green LED"="FIO1", "Foot Pedal"="DIO15"}  # LJ Pinout
        w603 = 0  # TCP attempt count
        w604 = u32 0  # Laser start tic
        w605 = refnum<k20>[] []  # niTClk sessions
        w606 = u32 0  # Last Trigger
        w607 = T32 {"DIO_EF_CLOCK1_DIVISOR"=16, "DIO_EF_CLOCK1_ROLL_VALUE"=25000, "DIO#_EF_INDEX"=0, "DIO#_EF_OPTIONS"=1, "DIO#_EF_CONFIG_A"=6250}  # 355 PWM setting
        w608 = T33 {"Aiming Beam COM Port"="COM3", "Min Current"=0.0, "Max Current"=63.0, "Default Current"=20.0, "Freq"=0}  # AB Cluster
        w609 = T34 {"resource name"="", "resource name 2"="", "Channel"=enum."Channel 0", "trigger source"="VAL_EXTERNAL", "trigger level"=0.5, "trigger delay"=1.35e-07, "min sample rate"=12500000000.0, "min record length"=2500, "vertical range"=1.0, "vertical offset"=-0.25, "Waveform to Avg"=2000}  # FLImDAQ
        w610 = FALSE  # SysRunning?
        w598 = path ""  # DefaultPath
        w611 = ""  # CaseID
        w612 = T5 {"Ch1Enable?"=FALSE, "Ch2Enable?"=FALSE, "Ch3Enable?"=FALSE, "Ch1AutoGain?"=FALSE, "Ch2AutoGain?"=FALSE, "Ch3AutoGain?"=FALSE, "AimingBeamEnable?"=FALSE}  # SysConfigCluster
        w613 = T35 {"Current VI Reference"=refnum, "Close Panel on Exit?"=FALSE}  # Core
        # "Initialize the shift-register data, here.\n(data names are defined by what you wire into the bundle function)"
        n290 = Bundle("Core"=w613, "SysConfigCluster"=w612, "System Status"=w600, "IDs"=w585, "CaseID"=w611, "DefaultPath"=w598, "Pathes"=w588, "FLImDAQ"=w609, "SysRunning?"=w610, "AB Cluster"=w608, "LJ Pinout"=w602, "355 PWM setting"=w607, "AB PWM setting"=w601, "Last Trigger"=w606, "niTClk sessions"=w605, "Laser start tic"=w604, "TCP attempt count"=w603, "Ch1Data"=w581, "Ch2Data"=w597, "Ch3Data"=w596, "Ch4Data"=w577, "V1"=w592, "V2"=w591, "V3"=w590, "V4"=w576, "SlowTimer"=w595, "FastTimer"=w594, "listener ID"=refnum<k5> refnum, "TempPath"=w587, "CaliPath"=w575, "LED vi reference"=w586, "Aquisition Timer"=w584, "APDSerialNum"=w583, "VideoConfig"=w582, "LED vi ref open?"=w580, "video source"=w579, "bothVidSourceAvail"=w578) -> (w589:T27)  [unwired: 1 in]
        n291 = call <vilib>:"Add State(s) to Queue__JKI_lib_State_Machine.vi"("State(s) in (\"\")"=w616) -> ("States Out"=w615:string)  [unwired: 14 in]
      }
      frame "Data: loadLastUseMacro" {
        # "Load last use BG and Cali and iRF.\n(It is a separator no-op. You can make a copy of this frame to create a new Data frame)"
        n292 = call <vilib>:"Add State(s) to Queue__JKI_lib_State_Machine.vi"("State(s) in Front (\"\")"="Data: loadLastUseBG\nData: loadSystemCali\nData: loadLastUseiRF\n/*Data: LoadiRFFromAPDFile\nUI: CaliAndiRFLoaded\nData: ShowiRF" ("State(s) in Front (\"\")"), "State(s) in (\"\")"=w622) -> ("States Out"=w621:string)  [unwired: 13 in]
      }
      frame "Data: loadLastUseBG" {
        w626 = enum16{"write", "read"}."write" ("action")
        # "Load last use BG.\n()"
        n293 = Unbundle By Name(w645) -> ("TempPath"=w644:path)
        n294 = call "FLImDAQ_FGV.vi"() -> ("Read data"=w640:T7)  [unwired: 10 in, 1 out]
        n295 = Build Path(base path=w644, name or relative path="Background.tdms") -> (appended path=w643:path)
        n296 = call "ReadBGorCali (SubVI).vi"("DataType"=enum16{"BG", "Cali"}."BG", "error in (no error)"=w642, "file path in"=w643) -> ("error out"=w641:errorcluster, "AvgDataCluster"=w636:T36)  [unwired: 6 in, 1 out]
        n297 = Unbundle By Name(w636) -> ("Channel 1"=w623:dbl[], "Channel 2"=w635:dbl[], "Channel 3"=w628:dbl[], "Channel 4"=w625:dbl[])
        n298 = Unbundle By Name(w640) -> ("min record length"=w632:i32)
        n299 = Array Size(array=w623) -> (size(s)=w634:i32)
        "BG length" <- w634
        n300 = Equal?(x=w634, y=w632) -> (x = y?=w633:bool)
        n301 = Select(t="UI: BGLoaded" ("State(s) in Front (\"\")"), s=w633, f="UI: BGSizeError" ("State(s) in Front (\"\")")) -> (s? t:f=w637:string)
        n302 = case shown="True" w633 {
          tunnel: w623 -> [_ w656]
          tunnel: w635 -> [_ w655]
          tunnel: w628 -> [_ w654]
          tunnel: w632 -> [w651 _]
          tunnel: [w650 w656] -> w631
          tunnel: [w650 w655] -> w630
          tunnel: [w650 w654] -> w629
          tunnel: w625 -> [_ w653]
          tunnel: [w650 w653] -> w624
          frame False {
            # "If error set BG all 0, update UI"
            n303 = for {
              N: w651 -> [_]
              tunnel: [0.0] -> w650 mode=indexing
            }
          }
          frame True {
            # "If no error, check size match"
          }
        }
        n304 = call "BG4FGV.vi"("action"=w626, "BG4 in"=w624) -> ()  [unwired: 8 in, 2 out]
        n305 = call "BG3FGV.vi"("action"=w626, "BG3 in"=w629) -> ()  [unwired: 8 in, 2 out]
        n306 = call "BG1FGV.vi"("action"=w626, "BG1 in"=w631) -> ()  [unwired: 8 in, 2 out]
        n307 = call "BG2FGV.vi"("action"=w626, "BG2 in"=w630) -> ()  [unwired: 8 in, 2 out]
        n308 = call <vilib>:"Add State(s) to Queue__JKI_lib_State_Machine.vi"("State(s) in Front (\"\")"=w637, "State(s) in (\"\")"=w649) -> ("States Out"=w648:string)  [unwired: 13 in]
      }
      frame "Data: loadSystemCali" {
        # "Load last use calibration.\n()"
        n309 = Unbundle By Name(w664) -> ("CaliPath"=w663:path)
        n310 = Build Path(base path=w663, name or relative path="Calibration.tdms") -> (appended path=w659:path)
        n311 = call "ReadBGorCali (SubVI).vi"("DataType"=enum16{"BG", "Cali"}."Cali", "error in (no error)"=w658, "file path in"=w659) -> ("error out"=w660:errorcluster, "CtrlVCluster"=w662:T37, "AvgDataCluster"=w661:T36)  [unwired: 6 in]
        n312 = case shown="No Error" w660 {
          tunnel: w662 -> [w683 _]
          tunnel: w661 -> [w682 _]
          frame No Error {
            w673 = T38 {"Ch1 WF"=[], "Ch2 WF"=[], "Ch3 WF"=[], "Ch4 WF"=[], "V1"=0.0, "V2"=0.0, "V3"=0.0, "V4"=0.0}  # SysCaliData
            n313 = Unbundle By Name(w682) -> ("Channel 1"=w681:dbl[], "Channel 2"=w680:dbl[], "Channel 3"=w679:dbl[], "Channel 4"=w672:dbl[])
            n314 = Unbundle By Name(w683) -> ("V 1"=w678:dbl[], "V 2"=w677:dbl[], "V 3"=w671:dbl[], "V 4"=w669:dbl[])
            n315 = Index Array(array=w678) -> (element=w676:dbl)  [unwired: 1 in]
            n316 = Index Array(array=w677) -> (element=w675:dbl)  [unwired: 1 in]
            n317 = Index Array(array=w671) -> (element=w674:dbl)  [unwired: 1 in]
            n318 = Index Array(array=w669) -> (element=w670:dbl)  [unwired: 1 in]
            n319 = Bundle By Name(cluster=w673, "Ch1 WF"=w681, "Ch2 WF"=w680, "Ch3 WF"=w679, "Ch4 WF"=w672, "V1"=w676, "V2"=w675, "V3"=w674, "V4"=w670) -> (w684:T38)
            n320 = global write "GlobalVariables.vi" "SysCaliData"(w684) -> ()
          }
          frame Error {
          }
        }
        n321 = call <vilib>:"Add State(s) to Queue__JKI_lib_State_Machine.vi"("State(s) in (\"\")"=w668) -> ("States Out"=w667:string)  [unwired: 14 in]
      }
      frame "Data: LoadiRFFromAPDFile" {
        w714 = T16 {"Ch1 iRF"=[], "Ch2 iRF"=[], "Ch3 iRF"=[], "Ch4 iRF"=[]}  # LastUseiRF
        # "only load the last 5th  iRF for the moment"
        # "Load APD detector data\n(It is a separator no-op. You can make a copy of this frame to create a new Data frame)"
        n322 = Unbundle By Name(w736) -> ("APDSerialNum.Ch1APDSerial#"=w735:string, "APDSerialNum.Ch2APDSerial#"=w716:string, "APDSerialNum.Ch3APDSerial#"=w715:string, "APDSerialNum.Ch4APDSerial#"=w712:string)
        n323 = call "CreatFromSerialNumNoRaw.vi"("error in (no error)"=w713, "APD Serial #"=w735) -> ("error out"=w733:errorcluster, "APDClass out"=w734:refnum<class "APDClass.lvclass">)  [unwired: 8 in]
        n324 = call "CreatFromSerialNumNoRaw.vi"("error in (no error)"=w713, "APD Serial #"=w716) -> ("error out"=w724:errorcluster, "APDClass out"=w725:refnum<class "APDClass.lvclass">)  [unwired: 8 in]
        n325 = call "CreatFromSerialNumNoRaw.vi"("error in (no error)"=w713, "APD Serial #"=w715) -> ("error out"=w718:errorcluster, "APDClass out"=w719:refnum<class "APDClass.lvclass">)  [unwired: 8 in]
        n326 = call "CreatFromSerialNumNoRaw.vi"("error in (no error)"=w713, "APD Serial #"=w712) -> ("error out"=w710:errorcluster, "APDClass out"=w711:refnum<class "APDClass.lvclass">)  [unwired: 8 in]
        n327 = call-dynamic "Read iRFData.vi"("error in (no error)"=w733, "APDClass in"=w734) -> ("iRFData"=w732:T39)  [unwired: 7 in, 2 out]
        n328 = call-dynamic "Read iRFData.vi"("error in (no error)"=w724, "APDClass in"=w725) -> ("iRFData"=w728:T39)  [unwired: 7 in, 2 out]
        n329 = call-dynamic "Read iRFData.vi"("error in (no error)"=w718, "APDClass in"=w719) -> ("iRFData"=w722:T39)  [unwired: 7 in, 2 out]
        n330 = call-dynamic "Read iRFData.vi"("error in (no error)"=w710, "APDClass in"=w711) -> ("iRFData"=w709:T39)  [unwired: 7 in, 2 out]
        n331 = Unbundle By Name(w732) -> ("iRFWFsAvg"=w731:dbl[][])
        n332 = Unbundle By Name(w728) -> ("iRFWFsAvg"=w727:dbl[][])
        n333 = Unbundle By Name(w722) -> ("iRFWFsAvg"=w721:dbl[][])
        n334 = Unbundle By Name(w709) -> ("iRFWFsAvg"=w706:dbl[][])
        n335 = Array Size(array=w731) -> (size(s)=w730:i32[])
        n336 = Array Size(array=w727) -> (size(s)=w723:i32[])
        n337 = Array Size(array=w721) -> (size(s)=w717:i32[])
        n338 = Array Size(array=w706) -> (size(s)=w707:i32[])
        n339 = Index Array(array=w730, index=0) -> (element=w705:i32)
        n340 = Index Array(array=w723, index=0) -> (element=w701:i32)
        n341 = Index Array(array=w717, index=0) -> (element=w698:i32)
        n342 = Index Array(array=w707, index=0) -> (element=w695:i32)
        n343 = Subtract(x=w705, y=5) -> (x-y=w703:i32)
        n344 = Subtract(x=w701, y=5) -> (x-y=w700:i32)
        n345 = Subtract(x=w698, y=5) -> (x-y=w697:i32)
        n346 = Subtract(x=w695, y=5) -> (x-y=w694:i32)
        n347 = Index Array(array=w731, index (row)=w703) -> (element=w693:dbl[])  [unwired: 1 in]
        n348 = Index Array(array=w727, index (row)=w700) -> (element=w692:dbl[])  [unwired: 1 in]
        n349 = Index Array(array=w721, index (row)=w697) -> (element=w691:dbl[])  [unwired: 1 in]
        n350 = Index Array(array=w706, index (row)=w694) -> (element=w690:dbl[])  [unwired: 1 in]
        n351 = call "DownSampleAndShiftiRF (SubVI).vi"("ArrayIn"=w693) -> ("ArrayOut"=w689:dbl[])  [unwired: 10 in]
        n352 = call "DownSampleAndShiftiRF (SubVI).vi"("ArrayIn"=w692) -> ("ArrayOut"=w685:dbl[])  [unwired: 10 in]
        n353 = call "DownSampleAndShiftiRF (SubVI).vi"("ArrayIn"=w691) -> ("ArrayOut"=w686:dbl[])  [unwired: 10 in]
        n354 = call "DownSampleAndShiftiRF (SubVI).vi"("ArrayIn"=w690) -> ("ArrayOut"=w688:dbl[])  [unwired: 10 in]
        n355 = call <vilib>:"Add State(s) to Queue__JKI_lib_State_Machine.vi"("State(s) in (\"\")"=w739) -> ("States Out"=w738:string)  [unwired: 14 in]
        n356 = Bundle(cluster=w714, "Ch1 iRF"=w689, "Ch2 iRF"=w685, "Ch3 iRF"=w686, "Ch4 iRF"=w688) -> (w687:T16)
        n357 = global write "GlobalVariables.vi" "LastUseiRF"(w687) -> ()
      }
      frame "Data: loadLastUseiRF" {
        # "Load last use iRF.\n()"
        n358 = Unbundle By Name(w745) -> ("TempPath"=w744:path)
        n359 = Build Path(base path=w744, name or relative path="iRF.tdms") -> (appended path=w750:path)
        n360 = TDMS Open(8:w740, 11:w750) -> (0:w748:errorcluster, 3:w749:refnum<k34>)  [unwired: 5 in]
        n361 = TDMS Read(0:w749, 11:w748, 12:dbl[][] []) -> (4:w743:refnum<k34>, 10:w746:dbl[][], 15:w742:errorcluster)  [unwired: 5 in, 3 out]
        n362 = TDMS Close(8:w742, 11:w743) -> (0:w741:errorcluster)  [unwired: 1 out]
        n363 = case shown="No Error" w742 {
          tunnel: w746 -> [w756 _]
          frame No Error {
            w760 = T16 {"Ch1 iRF"=[], "Ch2 iRF"=[], "Ch3 iRF"=[], "Ch4 iRF"=[]}  # LastUseiRF
            n364 = Index Array(array=w756, index (row)=0) -> (element=w769:dbl[])  [unwired: 1 in]
            n365 = Index Array(array=w756, index (row)=1) -> (element=w766:dbl[])  [unwired: 1 in]
            n366 = Index Array(array=w756, index (row)=2) -> (element=w763:dbl[])  [unwired: 1 in]
            n367 = Index Array(array=w756, index (row)=3) -> (element=w758:dbl[])  [unwired: 1 in]
            n368 = Add Array Elements(numeric array=w769) -> (sum=w768:dbl)
            n369 = Add Array Elements(numeric array=w766) -> (sum=w765:dbl)
            n370 = Add Array Elements(numeric array=w763) -> (sum=w762:dbl)
            n371 = Add Array Elements(numeric array=w758) -> (sum=w757:dbl)
            n372 = Divide(x=w769, y=w768) -> (x/y=w767:dbl[])
            n373 = Divide(x=w766, y=w765) -> (x/y=w764:dbl[])
            n374 = Divide(x=w763, y=w762) -> (x/y=w761:dbl[])
            n375 = Divide(x=w758, y=w757) -> (x/y=w755:dbl[])
            n376 = Bundle(cluster=w760, "Ch1 iRF"=w767, "Ch2 iRF"=w764, "Ch3 iRF"=w761, "Ch4 iRF"=w755) -> (w771:T16)
            n377 = Array Size(array=w769) -> (size(s)=→"iRF length":i32)
            n378 = global write "GlobalVariables.vi" "LastUseiRF"(w771) -> ()
          }
          frame Error {
          }
        }
        n379 = call <vilib>:"Add State(s) to Queue__JKI_lib_State_Machine.vi"("State(s) in (\"\")"=w754) -> ("States Out"=w753:string)  [unwired: 14 in]
      }
      frame "Data: ShowiRF" {
        # "Show loaded iRF.\n(It is a separator no-op. You can make a copy of this frame to create a new Data frame)"
        n380 = global read "GlobalVariables.vi" "LastUseiRF"() -> (w780:T16)
        n381 = Unbundle By Name(w780) -> ("Ch1 iRF"=w779:dbl[], "Ch2 iRF"=w778:dbl[], "Ch3 iRF"=w777:dbl[], "Ch4 iRF"=w776:dbl[])
        n382 = Build Array(w779, w778, w777, w776) -> (→"iRF Graph":dbl[][])
        n383 = call <vilib>:"Add State(s) to Queue__JKI_lib_State_Machine.vi"("State(s) in (\"\")"=w785) -> ("States Out"=w784:string)  [unwired: 14 in]
      }
      frame "Data: saveCalibration" {
        # "Average data and save calibration file. [Covers: REQ11]\n(It is a separator no-op. You can make a copy of this frame to create a new Data frame)"
        n384 = Unbundle By Name(w804) -> ("Ch1Data"=w803:dbl[][], "V1"=w802:dbl[], "Ch2Data"=w801:dbl[][], "V2"=w800:dbl[], "Ch3Data"=w799:dbl[][], "V3"=w798:dbl[], "Ch4Data"=w789:dbl[][], "V4"=w788:dbl[], "Pathes.CaliPath"=w807:path, "IDs.Cali ID"=w806:i8)
        n385 = Increment(x=w806) -> (x+1=w790:i8)
        n386 = Bundle("Ch1Data"=w803, "V1"=w802) -> (w797:cluster{"Ch1Data":dbl[][], "V1":dbl[]})  [unwired: 1 in]
        n387 = Bundle("Ch4Data"=w789, "V4"=w788) -> (w787:cluster{"Ch4Data":dbl[][], "V4":dbl[]})  [unwired: 1 in]
        n388 = Bundle("Ch2Data"=w801, "V2"=w800) -> (w796:cluster{"Ch2Data":dbl[][], "V2":dbl[]})  [unwired: 1 in]
        n389 = Bundle("Ch3Data"=w799, "V3"=w798) -> (w795:cluster{"Ch3Data":dbl[][], "V3":dbl[]})  [unwired: 1 in]
        n390 = Format Value(string ("")="Calibration" ("default name"), format string="%02d", value (0)=w790) -> (output string=w809:string)
        n391 = Build Path(base path=w807, name or relative path=w809) -> (appended path=w794:path)
        n392 = call "SaveBGorCali(SubVI).vi"("Channel1"=w797, "BG path"=w794, "DataType"=enum16{"BG", "Cali"}."Cali", "Channel 2"=w796, "Channel 3"=w795, "Channel 4"=w787, "error in (no error)"=w793, "SytemID"="UCDVetMed") -> ("error out"=w792:errorcluster)  [unwired: 7 in]
        n393 = call <vilib>:"Add State(s) to Queue__JKI_lib_State_Machine.vi"("State(s) in (\"\")"=w812) -> ("States Out"=w811:string)  [unwired: 14 in]
      }
      frame "Data: saveiRF" {
        w818 = enum16{"write", "read"}."read" ("action")
        # "Get iRF from decon stracture and save it on disk.\n(It is a separator no-op. You can make a copy of this frame to create a new Data frame)"
        n394 = Unbundle By Name(w835) -> ("TempPath"=w834:path)
        n395 = call "Ch1DeconEngineFGV.vi"("action(read)"=w818) -> ("Error Out"=w840:errorcluster, "Ch1DeconEngine out"=w841:refnum<class "LaguerreDeconEngineClass.lvclass">)  [unwired: 9 in]
        n396 = call "Ch2DeconEngineFGV.vi"("action(read)"=w818) -> ("Error Out"=w838:errorcluster, "Ch2DeconEngine out"=w839:refnum<class "LaguerreDeconEngineClass.lvclass">)  [unwired: 9 in]
        n397 = call "Ch3DeconEngineFGV.vi"("action(read)"=w818) -> ("Error Out"=w836:errorcluster, "Ch3DeconEngine out"=w837:refnum<class "LaguerreDeconEngineClass.lvclass">)  [unwired: 9 in]
        n398 = call "Ch4DeconEngineFGV.vi"("action(read)"=w818) -> ("Error Out"=w817:errorcluster, "Ch3DeconEngine out"=w816:refnum<class "LaguerreDeconEngineClass.lvclass">)  [unwired: 9 in]
        n399 = Build Path(base path=w834, name or relative path="iRF" ("default name")) -> (appended path=w832:path)
        n400 = call "getIRF.vi"("error in (no error)"=w817, "LaguerreDeconEngineClass in"=w816) -> ("iRF"=w815:dbl[])  [unwired: 7 in, 2 out]
        n401 = call "getIRF.vi"("error in (no error)"=w840, "LaguerreDeconEngineClass in"=w841) -> ("iRF"=w823:dbl[])  [unwired: 7 in, 2 out]
        n402 = call "getIRF.vi"("error in (no error)"=w838, "LaguerreDeconEngineClass in"=w839) -> ("iRF"=w822:dbl[])  [unwired: 7 in, 2 out]
        n403 = call "getIRF.vi"("error in (no error)"=w836, "LaguerreDeconEngineClass in"=w837) -> ("iRF"=w821:dbl[])  [unwired: 7 in, 2 out]
        n404 = TDMS Open(8:w831, 10:T17."create or replace" ("operation (0:open)"), 11:w832) -> (0:w828:errorcluster, 3:w829:refnum<k34>)  [unwired: 4 in]
        n405 = Bundle(cluster=T16 {"Ch1 iRF"=[], "Ch2 iRF"=[], "Ch3 iRF"=[], "Ch4 iRF"=[]} ("LastUseiRF"), "Ch1 iRF"=w823, "Ch2 iRF"=w822, "Ch3 iRF"=w821, "Ch4 iRF"=w815) -> (w819:T16)
        n406 = Build Array(w823, w822, w821, w815) -> (w827:dbl[][])
        n407 = global write "GlobalVariables.vi" "LastUseiRF"(w819) -> ()
        n408 = TDMS Write(0:w829, 5:"iRF" ("group name in (Untitled)"), 7:string[] ["Ch1", "Ch2", "Ch3", "Ch4"] ("channel name(s) in (Untitled)"), 9:w827, 11:w828) -> (4:w826:refnum<k34>, 15:w825:errorcluster)  [unwired: 1 in, 2 out]
        n409 = TDMS Close(8:w825, 11:w826) -> (0:w824:errorcluster)  [unwired: 1 out]
        n410 = call <vilib>:"Add State(s) to Queue__JKI_lib_State_Machine.vi"("State(s) in (\"\")"=w844) -> ("States Out"=w843:string)  [unwired: 14 in]
      }
      frame "Data: saveBGtoFGV" {
        w845 = enum16{"write", "read"}."write" ("action")
        # "Save BG and pass it to FGV.\n(save BG to disk and set it to FGV)"
        n411 = Unbundle By Name(w855) -> ("Ch1Data"=w854:dbl[][], "Ch2Data"=w853:dbl[][], "Ch3Data"=w852:dbl[][], "Ch4Data"=w847:dbl[][])
        n412 = call "AvgArrayTimeCritical.vi"("2D array"=w854) -> ("1D Avg"=w851:dbl[])  [unwired: 10 in]
        n413 = call "AvgArrayTimeCritical.vi"("2D array"=w853) -> ("1D Avg"=w850:dbl[])  [unwired: 10 in]
        n414 = call "AvgArrayTimeCritical.vi"("2D array"=w852) -> ("1D Avg"=w849:dbl[])  [unwired: 10 in]
        n415 = call "AvgArrayTimeCritical.vi"("2D array"=w847) -> ("1D Avg"=w846:dbl[])  [unwired: 10 in]
        n416 = call "BG1FGV.vi"("action"=w845, "BG1 in"=w851) -> ()  [unwired: 8 in, 2 out]
        n417 = call "BG2FGV.vi"("action"=w845, "BG2 in"=w850) -> ()  [unwired: 8 in, 2 out]
        n418 = call "BG3FGV.vi"("action"=w845, "BG3 in"=w849) -> ()  [unwired: 8 in, 2 out]
        n419 = call "BG4FGV.vi"("action"=w845, "BG4 in"=w846) -> ()  [unwired: 8 in, 2 out]
        n420 = call <vilib>:"Add State(s) to Queue__JKI_lib_State_Machine.vi"("State(s) in (\"\")"=w858) -> ("States Out"=w857:string)  [unwired: 14 in]
      }
      frame "Data: saveBGtoFile" {
        w880 = "Background" ("name or relative path")
        # "Save BG to file.\n(save BG to disk both data folder and temp folder)"
        n421 = Unbundle By Name(w884) -> ("Pathes.BG Path"=w877:path, "IDs.BG ID"=w876:i8, "Ch1Data"=w874:dbl[][], "V1"=w873:dbl[], "Ch2Data"=w872:dbl[][], "V2"=w871:dbl[], "Ch3Data"=w870:dbl[][], "V3"=w869:dbl[], "Ch4Data"=w861:dbl[][], "V4"=w860:dbl[], "TempPath"=w882:path)
        n422 = Increment(x=w876) -> (x+1=w881:i8)
        n423 = Format Value(string ("")=w880, format string="%02d", value (0)=w881) -> (output string=w879:string)
        n424 = Build Path(base path=w882, name or relative path=w880) -> (appended path=w863:path)
        n425 = call "File Dialog2"("start path"=w877, "prompt"="Please select BG name, DO NOT CANCEL!", "default name"=w879) -> ("selected path"=w864:path)  [unwired: 9 in, 3 out]
        n426 = Bundle("Ch1Data"=w874, "V1"=w873) -> (w868:cluster{"Ch1Data":dbl[][], "V1":dbl[]})  [unwired: 1 in]
        n427 = Bundle("Ch4Data"=w861, "V4"=w860) -> (w859:cluster{"Ch4Data":dbl[][], "V4":dbl[]})  [unwired: 1 in]
        n428 = Bundle("Ch2Data"=w872, "V2"=w871) -> (w867:cluster{"Ch2Data":dbl[][], "V2":dbl[]})  [unwired: 1 in]
        n429 = Bundle("Ch3Data"=w870, "V3"=w869) -> (w866:cluster{"Ch3Data":dbl[][], "V3":dbl[]})  [unwired: 1 in]
        n430 = Build Array(w864, w863) -> (w862:path[])
        n431 = for {
          tunnel: w868 -> [w895]
          tunnel: w867 -> [w894]
          tunnel: w866 -> [w893]
          shift-right: [w896] -> w875
          shift-left: w865 -> [w892]
          tunnel: w862 -> [w891] mode=indexing
          tunnel: w859 -> [w889]
          n432 = call "SaveBGorCali(SubVI).vi"("Channel1"=w895, "BG path"=w891, "DataType"=enum16{"BG", "Cali"}."BG", "Channel 2"=w894, "Channel 3"=w893, "Channel 4"=w889, "error in (no error)"=w892, "SytemID"="UCDVetMed") -> ("error out"=w896:errorcluster)  [unwired: 7 in]
        }
        n433 = call <vilib>:"Add State(s) to Queue__JKI_lib_State_Machine.vi"("State(s) in (\"\")"=w887) -> ("States Out"=w886:string)  [unwired: 14 in]
      }
      frame "Data: showBG" {
        # "Show BG in seperate window.\n()"
        n434 = call "showBG.vi"() -> ()  [unwired: 12 in]
        n435 = call <vilib>:"Add State(s) to Queue__JKI_lib_State_Machine.vi"("State(s) in (\"\")"=w901) -> ("States Out"=w900:string)  [unwired: 14 in]
      }
      frame "Data: irfAlignment" {
        w902 = enum16{"write", "read"}."write" ("action")
        # "do iRF alignment in this state\n(It is a separator no-op. You can make a copy of this frame to create a new Data frame)"
        n436 = Unbundle By Name(w947) -> ("Ch1Data"=w983:dbl[][], "Ch2Data"=w982:dbl[][], "Ch3Data"=w981:dbl[][], "Ch4Data"=w924:dbl[][])
        n437 = call "Ch1DeconEngineFGV.vi"("Error In"=w923) -> ("Error Out"=w979:errorcluster, "Ch1DeconEngine out"=w980:refnum<class "LaguerreDeconEngineClass.lvclass">)  [unwired: 9 in]
        n438 = call "Ch2DeconEngineFGV.vi"("Error In"=w923) -> ("Error Out"=w977:errorcluster, "Ch2DeconEngine out"=w978:refnum<class "LaguerreDeconEngineClass.lvclass">)  [unwired: 9 in]
        n439 = call "Ch3DeconEngineFGV.vi"("Error In"=w923) -> ("Error Out"=w975:errorcluster, "Ch3DeconEngine out"=w976:refnum<class "LaguerreDeconEngineClass.lvclass">)  [unwired: 9 in]
        n440 = call "Ch4DeconEngineFGV.vi"("Error In"=w923) -> ("Error Out"=w914:errorcluster, "Ch3DeconEngine out"=w913:refnum<class "LaguerreDeconEngineClass.lvclass">)  [unwired: 9 in]
        n441 = call "AvgArray.vi"("2D array in"=w982) -> ("1D Avg out"=w929:dbl[])  [unwired: 10 in]
        n442 = call "AvgArray.vi"("2D array in"=w981) -> ("1D Avg out"=w928:dbl[])  [unwired: 10 in]
        n443 = call "AvgArray.vi"("2D array in"=w924) -> ("1D Avg out"=w903:dbl[])  [unwired: 10 in]
        n444 = call "AvgArray.vi"("2D array in"=w983) -> ("1D Avg out"=w930:dbl[])  [unwired: 10 in]
        n445 = call "RemoveDCBG.vi"("WF in"=w930) -> ("DC"=w937:dbl, "WF out"=w927:dbl[])  [unwired: 8 in, 1 out]
        n446 = call "RemoveDCBG.vi"("WF in"=w929) -> ("DC"=w934:dbl, "WF out"=w940:dbl[])  [unwired: 8 in, 1 out]
        n447 = call "RemoveDCBG.vi"("WF in"=w928) -> ("DC"=w932:dbl, "WF out"=w939:dbl[])  [unwired: 8 in, 1 out]
        n448 = call "RemoveDCBG.vi"("WF in"=w903) -> ("DC"=w907:dbl, "WF out"=w905:dbl[])  [unwired: 8 in, 1 out]
        n449 = call "computeIRFAlignment.vi"("error in (no error)"=w979, "fIRF temp"=w927, "LaguerreDeconEngineClass in"=w980) -> ("error out"=w971:errorcluster, "LaguerreDeconEngineClass out"=w972:refnum<class "LaguerreDeconEngineClass.lvclass">)  [unwired: 6 in, 1 out]
        n450 = call "computeIRFAlignment.vi"("error in (no error)"=w977, "fIRF temp"=w940, "LaguerreDeconEngineClass in"=w978) -> ("error out"=w969:errorcluster, "LaguerreDeconEngineClass out"=w970:refnum<class "LaguerreDeconEngineClass.lvclass">)  [unwired: 6 in, 1 out]
        n451 = call "computeIRFAlignment.vi"("error in (no error)"=w975, "fIRF temp"=w939, "LaguerreDeconEngineClass in"=w976) -> ("error out"=w973:errorcluster, "LaguerreDeconEngineClass out"=w974:refnum<class "LaguerreDeconEngineClass.lvclass">)  [unwired: 6 in, 1 out]
        n452 = call "computeIRFAlignment.vi"("error in (no error)"=w914, "fIRF temp"=w905, "LaguerreDeconEngineClass in"=w913) -> ("error out"=w921:errorcluster, "LaguerreDeconEngineClass out"=w922:refnum<class "LaguerreDeconEngineClass.lvclass">)  [unwired: 6 in, 1 out]
        n453 = call "Ch1DeconEngineFGV.vi"("Error In"=w971, "action(read)"=w902, "Ch1DeconEngine in"=w972) -> ("Error Out"=w967:errorcluster, "Ch1DeconEngine out"=w968:refnum<class "LaguerreDeconEngineClass.lvclass">)  [unwired: 7 in]
        n454 = call "Ch2DeconEngineFGV.vi"("Error In"=w969, "action(read)"=w902, "Ch2DeconEngine in"=w970) -> ("Error Out"=w957:errorcluster, "Ch2DeconEngine out"=w958:refnum<class "LaguerreDeconEngineClass.lvclass">)  [unwired: 7 in]
        n455 = call "Ch3DeconEngineFGV.vi"("Error In"=w973, "action(read)"=w902, "Ch3DeconEngine in"=w974) -> ("Error Out"=w951:errorcluster, "Ch3DeconEngine out"=w952:refnum<class "LaguerreDeconEngineClass.lvclass">)  [unwired: 7 in]
        n456 = call "Ch4DeconEngineFGV.vi"("Error In"=w921, "action(read)"=w902, "Ch3DeconEngine in"=w922) -> ("Error Out"=w915:errorcluster, "Ch3DeconEngine out"=w916:refnum<class "LaguerreDeconEngineClass.lvclass">)  [unwired: 7 in]
        n457 = call "setfIRF.vi"("error in (no error)"=w951, "fIRF"=w939, "LaguerreDeconEngineClass in"=w952) -> ("error out"=w955:errorcluster, "LaguerreDeconEngineClass out"=w956:refnum<class "LaguerreDeconEngineClass.lvclass">)  [unwired: 7 in]
        n458 = call "setfIRF.vi"("error in (no error)"=w915, "fIRF"=w905, "LaguerreDeconEngineClass in"=w916) -> ("error out"=w919:errorcluster, "LaguerreDeconEngineClass out"=w920:refnum<class "LaguerreDeconEngineClass.lvclass">)  [unwired: 7 in]
        n459 = call "setfIRF.vi"("error in (no error)"=w957, "fIRF"=w940, "LaguerreDeconEngineClass in"=w958) -> ("error out"=w961:errorcluster, "LaguerreDeconEngineClass out"=w962:refnum<class "LaguerreDeconEngineClass.lvclass">)  [unwired: 7 in]
        n460 = call "setfIRF.vi"("error in (no error)"=w967, "fIRF"=w927, "LaguerreDeconEngineClass in"=w968) -> ("error out"=w965:errorcluster, "LaguerreDeconEngineClass out"=w966:refnum<class "LaguerreDeconEngineClass.lvclass">)  [unwired: 7 in]
        n461 = Unbundle By Name(w947) -> ("V1"=w926:dbl[], "V2"=w946:dbl[], "V3"=w945:dbl[], "V4"=w912:dbl[])
        n462 = call "computeLCs.vi"("error in (no error)"=w965, "LaguerreDeconClass in"=w966) -> ("error out"=w963:errorcluster, "LaguerreDeconClass out"=w964:refnum<class "LaguerreDeconEngineClass.lvclass">)  [unwired: 8 in]
        n463 = call "computeLCs.vi"("error in (no error)"=w961, "LaguerreDeconClass in"=w962) -> ("error out"=w959:errorcluster, "LaguerreDeconClass out"=w960:refnum<class "LaguerreDeconEngineClass.lvclass">)  [unwired: 8 in]
        n464 = call "computeLCs.vi"("error in (no error)"=w955, "LaguerreDeconClass in"=w956) -> ("error out"=w953:errorcluster, "LaguerreDeconClass out"=w954:refnum<class "LaguerreDeconEngineClass.lvclass">)  [unwired: 8 in]
        n465 = call "computeLCs.vi"("error in (no error)"=w919, "LaguerreDeconClass in"=w920) -> ("error out"=w917:errorcluster, "LaguerreDeconClass out"=w918:refnum<class "LaguerreDeconEngineClass.lvclass">)  [unwired: 8 in]
        n466 = call-poly <vilib>:"Mean.vi"("X"=w926) -> ("mean"=w925:dbl)  [unwired: 1 out]
        n467 = call-poly <vilib>:"Mean.vi"("X"=w912) -> ("mean"=w911:dbl)  [unwired: 1 out]
        n468 = call-poly <vilib>:"Mean.vi"("X"=w946) -> ("mean"=w944:dbl)  [unwired: 1 out]
        n469 = call "getFitting.vi"("error in (no error)"=w963, "LaguerreDeconEngineClass in"=w964) -> ("Fitting"=w936:dbl[])  [unwired: 7 in, 2 out]
        n470 = call "getFitting.vi"("error in (no error)"=w959, "LaguerreDeconEngineClass in"=w960) -> ("Fitting"=w933:dbl[])  [unwired: 7 in, 2 out]
        n471 = call "getFitting.vi"("error in (no error)"=w953, "LaguerreDeconEngineClass in"=w954) -> ("Fitting"=w909:dbl[])  [unwired: 7 in, 2 out]
        n472 = call "getFitting.vi"("error in (no error)"=w917, "LaguerreDeconEngineClass in"=w918) -> ("Fitting"=w908:dbl[])  [unwired: 7 in, 2 out]
        n473 = Add(x=w937, y=w936) -> (x+y=w938:dbl[])
        n474 = Add(x=w934, y=w933) -> (x+y=w935:dbl[])
        n475 = call-poly <vilib>:"Mean.vi"("X"=w945) -> ("mean"=w943:dbl)  [unwired: 1 out]
        n476 = Add(x=w932, y=w909) -> (x+y=w931:dbl[])
        n477 = Build Array(w930, w938) -> (w950:dbl[][])
        n478 = Build Array(w929, w935) -> (w949:dbl[][])
        n479 = Build Array(w928, w931) -> (w948:dbl[][])
        n480 = Add(x=w907, y=w908) -> (x+y=w906:dbl[])
        n481 = Bundle("mean"=w925, "mean"=w944, "mean"=w943, "mean"=w911) -> (w910:T40)  [unwired: 1 in]
        n482 = Build Array(w903, w906) -> (w904:dbl[][])
        n483 = call "Calib_and_iRFAlign_confirm.vi"("Current V"=w910, "Ch4 Data"=w904, "Ch3 Data"=w948, "Ch2 Data"=w949, "Ch1 Data"=w950) -> ("Save?"=w942:bool)  [unwired: 6 in]
        n484 = case shown="True" w942 {
          tunnel: ["" ("Empty String Constant") "Data: saveCalibration\nData: saveiRF\nRun: CaliIncrement"] -> w941
          frame False {
          }
          frame True {
            # "[Covers: REQ2]"
          }
        }
        n485 = call <vilib>:"Add State(s) to Queue__JKI_lib_State_Machine.vi"("State(s) in Front (\"\")"=w941, "State(s) in (\"\")"=w986) -> ("States Out"=w985:string)  [unwired: 13 in]
      }
      frame "Data: parseRunData" {
        # "All APD bias"
        # "flash queue"
        # "Ch3&4"
        # "Ch1&2"
        # "Flash data from queue and save it in structure\n()"
        n486 = Flush Queue(queue=w1014, error in (no error)=w1013) -> (remaining elements=w1008:T41, error out=w1009:errorcluster)  [unwired: 1 out]
        n487 = Flush Queue(queue=w1019, error in (no error)=w1013) -> (remaining elements=w1017:cluster{"double data":dbl[][]}[], error out=w1010:errorcluster)  [unwired: 1 out]
        n488 = Flush Queue(queue=w1020, error in (no error)=w1013) -> (remaining elements=w1018:cluster{"double data":dbl[][]}[], error out=w1011:errorcluster)  [unwired: 1 out]
        n489 = for {
          tunnel: w1018 -> [w1036] mode=indexing
          tunnel: [w1034] -> w1003 mode=concatenating
          tunnel: [w1033] -> w1004 mode=concatenating
          n490 = Unbundle By Name(w1036) -> ("double data"=w1035:dbl[][])
          n491 = call "SeperateChanData.vi"("Input (Ch1&2)"=w1035) -> ("Ch1"=w1034:dbl[][], "Ch2"=w1033:dbl[][])
        }
        n492 = for {
          tunnel: w1017 -> [w1032] mode=indexing
          tunnel: [w1031] -> w993 mode=concatenating
          tunnel: [w1029] -> w994 mode=concatenating
          n493 = Unbundle By Name(w1032) -> ("double data"=w1030:dbl[][])
          n494 = call "SeperateChanData.vi"("Input (Ch1&2)"=w1030) -> ("Ch1"=w1031:dbl[][], "Ch2"=w1029:dbl[][])
        }
        n495 = call "FLImDAQ_FGV.vi"() -> ("Read data"=w1001:T7)  [unwired: 10 in, 1 out]
        n496 = Unbundle By Name(w1001) -> ("Waveform to Avg"=w991:i16)
        n497 = for {
          tunnel: w1008 -> [w1028] mode=indexing
          tunnel: [w1027] -> w1000 mode=indexing
          tunnel: [w1026] -> w998 mode=indexing
          tunnel: [w1025] -> w996 mode=indexing
          tunnel: [w1024] -> w992 mode=indexing
          n498 = Unbundle By Name(w1028) -> ("V1"=w1027:dbl, "V2"=w1026:dbl, "V3"=w1025:dbl, "V4"=w1024:dbl)
        }
        n499 = call "DuplicateV(SubVI).vi"("Averaging"=w991, "V in"=w1000) -> ("V out"=w999:dbl[])  [unwired: 9 in]
        n500 = Array Size(array=w993) -> (size(s)=→"data Size":i32[])
        n501 = call "DuplicateV(SubVI).vi"("Averaging"=w991, "V in"=w998) -> ("V out"=w997:dbl[])  [unwired: 9 in]
        n502 = call "DuplicateV(SubVI).vi"("Averaging"=w991, "V in"=w996) -> ("V out"=w995:dbl[])  [unwired: 9 in]
        n503 = call "DuplicateV(SubVI).vi"("Averaging"=w991, "V in"=w992) -> ("V out"=w989:dbl[])  [unwired: 9 in]
        n504 = Bundle By Name(cluster=w1015, "Ch1Data"=w1003, "Ch2Data"=w1004, "Ch3Data"=w993, "Ch4Data"=w994, "V1"=w999, "V2"=w997, "V3"=w995, "V4"=w989) -> (w1016:T27)
        n505 = Merge Errors(w1011, w1010, w1009) -> (w1012:errorcluster)
        n506 = Array Size(array=w999) -> (size(s)=→"V1 Size":i32)
        n507 = Array Size(array=w997) -> (size(s)=→"V2 Size":i32)
        n508 = Array Size(array=w995) -> (size(s)=→"V3 Size":i32)
        n509 = Array Size(array=w989) -> (size(s)=→"V4 Size":i32)
        n510 = call <vilib>:"Add State(s) to Queue__JKI_lib_State_Machine.vi"("State(s) in (\"\")"=w1023) -> ("States Out"=w1022:string)  [unwired: 14 in]
      }
      frame "Data: saveRunData" {
        w1039 = T42 {"DataPath"=path "", "CaseID"="", "RunID"=0, "Ch1Data"=[], "Ch2Data"=[], "Ch3Data"=[], "Ch4Data"=[], "V1"=[], "V2"=[], "V3"=[], "V4"=[], "LaserRepRate"=0, "WFAverage"=0, "RunStartTime"=0}  # Data cluster
        # "Save FLIm data to disk.\n(Save to LV tdms file format)"
        n511 = Unbundle By Name(w1050) -> ("Pathes.DataPath"=w1046:path, "CaseID"=w1058:string, "IDs.RunID"=w1048:i8, "Ch1Data"=w1057:dbl[][], "Ch2Data"=w1056:dbl[][], "Ch3Data"=w1045:dbl[][], "Ch4Data"=w1038:dbl[][], "V1"=w1040:dbl[], "V2"=w1055:dbl[], "V3"=w1054:dbl[], "V4"=w1037:dbl[])
        n512 = call "FLImDAQ_FGV.vi"() -> ("Read data"=w1043:T7)  [unwired: 10 in, 1 out]
        n513 = Unbundle By Name(w1043) -> ("Waveform to Avg"=w1042:i16)
        n514 = local read "RunStartTime"() -> (w1041:u32)
        n515 = local read "Laser Rep Rate"() -> (w1044:dbl)
        n516 = Increment(x=w1048) -> (x+1=w1047:i8)
        n517 = Bundle By Name(cluster=w1039, "DataPath"=w1046, "CaseID"=w1058, "RunID"=w1047, "Ch1Data"=w1057, "Ch2Data"=w1056, "Ch3Data"=w1045, "Ch4Data"=w1038, "V1"=w1040, "V2"=w1055, "V3"=w1054, "V4"=w1037, "LaserRepRate"=w1044, "WFAverage"=w1042, "RunStartTime"=w1041) -> (w1053:T42)
        n518 = call "SaveRunData(SubVI).vi"("Data cluster"=w1053, "error in (no error)"=w1052) -> ("error out"=w1049:errorcluster)  [unwired: 13 in]
        n519 = flat-sequence {
          tunnel: w1050 -> [w1066]
          tunnel: [w1065] -> w1051
          tunnel: w1049 -> [_]
          frame #0 {
            w1063 = dbl[][] [] ("Ch1Data")
            w1064 = dbl[] [] ("V1")
            # "reset local data"
            n520 = Bundle By Name(cluster=w1066, "Ch1Data"=w1063, "Ch2Data"=w1063, "Ch3Data"=w1063, "Ch4Data"=w1063, "V1"=w1064, "V2"=w1064, "V3"=w1064, "V4"=w1064) -> (w1065:T27)
          }
        }
        n521 = case shown="No Error" w1049 {
          tunnel: ["Run: Increment" "" ("Empty String Constant")] -> w1059
          frame No Error {
          }
          frame Error {
          }
        }
        n522 = call <vilib>:"Add State(s) to Queue__JKI_lib_State_Machine.vi"("State(s) in Front (\"\")"=w1059, "State(s) in (\"\")"=w1062) -> ("States Out"=w1061:string)  [unwired: 13 in]
      }
      frame "Data: Cleanup" {
        # "Cleanup any data and references, here.\n(this is called automatically, by the Macro: Exit)"
        n523 = Unbundle By Name(w1070) -> ("Core.Current VI Reference"=w1073:refnum<vi>)
        n524 = Close Reference(reference=w1073, error in (no error)=w1072) -> (error out=w1071:errorcluster)
        n525 = call <vilib>:"Add State(s) to Queue__JKI_lib_State_Machine.vi"("State(s) in (\"\")"=w1075) -> ("States Out"=w1074:string)  [unwired: 14 in]
      }
      frame "---------- Core ----------" {
        # "Do not put any code in this frame.\n(it is a separator no-op)"
        n526 = call <vilib>:"Add State(s) to Queue__JKI_lib_State_Machine.vi"("State(s) in (\"\")"=w1080) -> ("States Out"=w1079:string)  [unwired: 14 in]
      }
      frame Default {
        w1091 = 42 items=["No error", "Argument error", "Memory is full", "Out of zone", "End of file", "File already open", "Generic file I/O error", "File not found", "File permission error", "Disk is full", "Duplicate path", "Too many files open", "System feature not enabled", "Resource file not found", "Cannot add resource", "Resource not found", "Image not found", "Image memory error", "Pen does not exist", "Config type invalid", "Config token not found", "Config parse error", "Config memory error", "Bad external code format", "Bad external code offset", "External code not present", "Null window", "Destroy window error", "Null menu", "Print aborted", "Bad print record", "Print driver error", "Windows error during printing", "Memory error during printing", "Print dialog error", "Generic print error", "Invalid device refnum", "Device not found", "Device parameter error", "Device unit error", "Cannot open device", "Device call aborted", "Generic error", "Cancelled by user", "Object ID too low", "Object ID too high", "Object not in heap", "Unknown heap", "Unknown object (invalid DefProc)", "Unknown object (DefProc not in table)", "Message out of range", "Invalid (null) method", "Unknown message", "Manager call not supported", "Bad address", "Network operation in progress", "Network operation timed out", "Connection is busy", "Network attribute not supported", "Network error", "Address in use", "System out of memory", "Connection aborted", "Connection refused", "Not connected", "Already connected", "Connection closed", "Initialization error (interapplication manager)", "Bad occurrence", "Wait on unbound occurrence handler", "Occurrence queue overflow", "Datalog type conflict", "Unused", "Unrecognized type (interapplication manager)", "Memory corrupt", "Failed to make temporary DLL", "Old CIN version", "Drag socket not found", "Failed to load drop-object", "Failed to register OLE object", "Failed to release OLE object", "Format specifier type mismatch", "Unknown format specifier", "Too few format specifiers", "Too many format specifiers", "Scan failed", "Newer CIN version", "Error converting to variant", "Runtime menu error", "Password tampered", "Variant attribute not found", "Incompatible variant data type", "Event data is not available", "Event Store is not present", "Occurrence is not found", "Event Queue is not created", "Event info is not available", "Refnum passed is NULL", "Error retrieving Class GUID", "Error retrieving CoClass GUID", "Error retrieving TypeLib GUID.", "Bad built application magic bytes.", "Specific driver is different from the specific driver associated with the Logical Name.", "There is no session opened to the class driver.", "Max Error", "MAX - Error with config objects", "MAX - Error loading configuration", "MAX - Group not supported"]
        # "Current State"
        # "Do not delete, rename, or modify this frame.\n(this is used to capture unhandled states and typos)"
        # "Handle mistyped state name (developer tool)"
        n527 = Format Into String(format string="Software Exception: Unhandled State \"%s\"." ("message"), error in=w1087, w1082) -> (resulting string=w1090:string, error out=w1089:errorcluster)  [unwired: 1 in]
        n528 = call <vilib>:"Error Cluster From Error Code.vi"("show call chain? (False)"=TRUE, "error in (no error)"=w1089, "error message (\"\")"=w1090, "error code (0)"=w1091) -> ("error out"=w1088:errorcluster)  [unwired: 5 in]
        n529 = call <vilib>:"Add State(s) to Queue__JKI_lib_State_Machine.vi"("State(s) in (\"\")"=w1086) -> ("States Out"=w1085:string)  [unwired: 14 in]
      }
      frame "Initialize Core Data" {
        # "Build default path based on the location of project"
        # "Do not delete, rename, or modify this frame.\n(this is used to determine panel behavior on exit)"
        # "originally closed?"
        # "exe?"
        # "If panel starts closed or is an EXE, then close it when we exit"
        n530 = call <vilib>:"Application Directory.vi"() -> ("Application Directory"=w1094:path)
        n531 = property on="Property Node" class="App"() -> ("App.Kind"=w1110:T19)  [unwired: 2 in, 2 out]
        n532 = property on="Property Node" class="VI"() -> ("FP.State"=w1104:T18)  [unwired: 2 in, 2 out]
        n533 = control-ref of="Current VI Reference"() -> (w1105:refnum<vi>)
        n534 = Equal?(x=w1104, y=T18."Closed" ("Front Panel Window:State")) -> (x = y?=w1102:bool)
        n535 = Strip Path(path=w1094) -> (stripped path=w1093:path)  [unwired: 1 out]
        n536 = Equal?(x=w1110, y=T19."Run Time System" ("Application:Kind")) -> (x = y?=w1108:bool)
        n537 = Build Path(base path=w1093, name or relative path="Data") -> (appended path=w1100:path)
        n538 = Build Path(base path=w1094, name or relative path="SystemTemp") -> (appended path=w1097:path)
        n539 = Build Path(base path=w1094, name or relative path="SystemCalibrationFile") -> (appended path=w1095:path)
        n540 = Or(x=w1102, y=w1108) -> (x .or. y?=w1106:bool)
        n541 = Bundle By Name(cluster=w1107, "Core.Current VI Reference"=w1105, "Core.Close Panel on Exit?"=w1106, "DefaultPath"=w1100, "TempPath"=w1097, "CaliPath"=w1095) -> (w1112:T27)
        n542 = call <vilib>:"Add State(s) to Queue__JKI_lib_State_Machine.vi"("State(s) in (\"\")"=w1114) -> ("States Out"=w1113:string)  [unwired: 14 in]
      }
      frame "Error Handler" {
        # "Unhandled Error -- Display it"
        # "Handle any errors here.\nYou can also output any states to clean-up after errors occur"
        # "Clear error"
        n543 = Unbundle By Name(w1115) -> ("code"=w1117:i32)
        n544 = case shown="Default" w1117 {
          tunnel: ["Macro: Exit" w1127 w1133] -> w1116
          tunnel: w1115 -> [w1123 _ _]
          frame Default {
            w1125 = T43 1 items=["no dialog", "OK message", "continue or stop message", "OK message + warnings", "continue/stop + warnings"] ("type of dialog (OK msg:1)")
            n545 = call <vilib>:"General Error Handler.vi"("type of dialog (OK msg:1)"=w1125, "error in (no error)"=w1123) -> ()  [unwired: 9 in, 5 out]
          }
          frame 5002 {
            n546 = Two Button Dialog(message="Laser interlock open! Please close interlock and try again! ", 1:"Safely Shutdown" ("F button name (\"Cancel\")"), 2:"OK" ("T button name (\"OK\")")) -> (T button?=w1128:bool)
            n547 = case shown="True" w1128 {
              tunnel: ["Macro: Exit" "355 Laser: CheckControllerStatus"] -> w1127
              frame False {
              }
              frame True {
              }
            }
          }
          frame 5001 {
            n548 = Two Button Dialog(message="Unable to connect to imaging computer, do you want to run data aquisiton alone? ", 1:"No" ("F button name (\"Cancel\")"), 2:"Yes" ("T button name (\"OK\")")) -> (T button?=w1134:bool)
            n549 = case shown="False" w1134 {
              tunnel: ["Macro: Exit" "" ("Empty String Constant")] -> w1133
              frame False {
              }
              frame True {
              }
            }
          }
        }
        n550 = call <vilib>:"Add State(s) to Queue__JKI_lib_State_Machine.vi"("State(s) in Front (\"\")"=w1116, "State(s) in (\"\")"=w1122) -> ("States Out"=w1121:string)  [unwired: 13 in]
      }
      frame "Exit" {
        # "Do not put any code in this frame.\n(No errors that occur here will be handled.)"
        n551 = call <vilib>:"Add State(s) to Queue__JKI_lib_State_Machine.vi"("State(s) in (\"\")"=w1145) -> ("States Out"=w1144:string)  [unwired: 14 in]
      }
      frame "---------- Case ----------" {
        # "Template Separator\n(You can make a copy of, or modify, this frame)"
        n552 = call <vilib>:"Add State(s) to Queue__JKI_lib_State_Machine.vi"("State(s) in (\"\")"=w1150) -> ("States Out"=w1149:string)  [unwired: 14 in]
      }
      frame "Case: getCaliID" {
        # "Get Calibration file #\n(You can make a copy of, or modify, this frame)"
        n553 = Unbundle By Name(w1151) -> ("Pathes.CaliPath"=w1154:path)
        n554 = call <vilib>:"Recursive File List.vi"("pattern"="*.tdms", "Treat LLBs as Folders?"=FALSE, "Folder Path"=w1154) -> ("All Files in Dir"=w1159:path[])  [unwired: 4 in, 4 out]
        n555 = for {
          tunnel: w1159 -> [w1169] mode=indexing
          tunnel: [w1168] -> w1158 mode=indexing
          tunnel: "Calibration" -> [w1165]
          n556 = Strip Path(path=w1169) -> (name=w1166:string)  [unwired: 1 out]
          n557 = Search and Replace String(input string=w1166, search string=w1165) -> (result string=w1164:string)  [unwired: 6 in, 3 out]
          n558 = Scan From String(format string="%d" ("string"), input string=w1164) -> (output 1=w1168:i32)  [unwired: 3 in, 3 out]
        }
        n559 = Array Max & Min(array=w1158) -> (max value=w1157:i32)  [unwired: 3 out]
        n560 = Bundle By Name(cluster=w1151, "IDs.Cali ID"=w1157) -> (w1152:T27)
        n561 = call <vilib>:"Add State(s) to Queue__JKI_lib_State_Machine.vi"("State(s) in (\"\")"=w1163) -> ("States Out"=w1162:string)  [unwired: 14 in]
      }
      frame "Case: getBGID" {
        # "Get background #\n(You can make a copy of, or modify, this frame)"
        n562 = Unbundle By Name(w1172) -> ("Pathes.BG Path"=w1177:path)
        n563 = call <vilib>:"Recursive File List.vi"("pattern"="*.tdms", "Treat LLBs as Folders?"=FALSE, "Folder Path"=w1177) -> ("All Files in Dir"=w1175:path[])  [unwired: 4 in, 4 out]
        n564 = for {
          tunnel: w1175 -> [w1192] mode=indexing
          tunnel: "Background" ("name or relative path") -> [w1190]
          shift-right: [w1183] -> w1170
          shift-left: 0 -> [w1187]
          n565 = Strip Path(path=w1192) -> (name=w1191:string)  [unwired: 1 out]
          n566 = Search and Replace String(input string=w1191, search string=w1190) -> (number of replacements=w1189:i32)  [unwired: 6 in, 3 out]
          n567 = Greater Than 0?(x=w1189) -> (x > 0?=w1188:bool)
          n568 = Select(t=1, s=w1188, f=0) -> (s? t:f=w1186:i32)
          n569 = Add(x=w1186, y=w1187) -> (x+y=w1183:i32)
        }
        n570 = Bundle By Name(cluster=w1172, "IDs.BG ID"=w1170) -> (w1173:T27)
        n571 = call <vilib>:"Add State(s) to Queue__JKI_lib_State_Machine.vi"("State(s) in (\"\")"=w1182) -> ("States Out"=w1181:string)  [unwired: 14 in]
      }
      frame "Case: getRunID" {
        # "Check folder for run ID\n(You can make a copy of, or modify, this frame)"
        n572 = Unbundle By Name(w1202) -> ("Pathes.DataPath"=w1201:path, "CaseID"=w1197:string)
        n573 = Build Array("Background" ("name or relative path"), "Calibration", "3DScanData" ("element")) -> (w1207:string[])
        n574 = call <vilib>:"Recursive File List.vi"("Folders to Exclude"=w1207, "pattern"="*.tdms", "Treat LLBs as Folders?"=FALSE, "Folder Path"=w1201) -> ("All Files in Dir"=w1198:path[])  [unwired: 3 in, 4 out]
        n575 = for {
          tunnel: w1198 -> [w1216] mode=indexing
          tunnel: [w1215] -> w1204 mode=indexing
          tunnel: w1197 -> [w1212]
          n576 = Strip Path(path=w1216) -> (name=w1213:string)  [unwired: 1 out]
          n577 = Search and Replace String(input string=w1213, search string=w1212) -> (result string=w1211:string)  [unwired: 6 in, 3 out]
          n578 = Scan From String(format string="_%d" ("string"), input string=w1211) -> (output 1=w1215:i32)  [unwired: 3 in, 3 out]
        }
        n579 = Array Max & Min(array=w1204) -> (max value=w1195:i32)  [unwired: 3 out]
        n580 = Bundle By Name(cluster=w1202, "IDs.RunID"=w1195) -> (w1203:T27)
        n581 = call "RunIDFGV.vi"("Error In"=w1193, "RunID in"=w1195) -> ("Error Out"=w1194:errorcluster)  [unwired: 8 in, 1 out]
        n582 = call <vilib>:"Add State(s) to Queue__JKI_lib_State_Machine.vi"("State(s) in (\"\")"=w1210) -> ("States Out"=w1209:string)  [unwired: 14 in]
      }
      frame "Case: CreatFileStruct" {
        # "Creat case file structure"
        n583 = Unbundle By Name(w1230) -> ("DefaultPath"=w1236:path, "CaseID"=w1223:string)
        n584 = Build Path(base path=w1236, name or relative path=w1223) -> (appended path=w1235:path)
        n585 = call <vilib>:"Check if File or Folder Exists.vi"("error in (no error)"=w1229, "path"=w1235) -> ("error out"=w1232:errorcluster, "file or folder exists?"=w1234:bool, "dup path"=w1233:path)  [unwired: 7 in]
        n586 = case shown="False" w1234 {
          tunnel: w1233 -> [w1253 w1261]
          tunnel: w1232 -> [w1251 w1256]
          tunnel: [w1245 w1261] -> w1221
          tunnel: [w1249 w1263] -> w1220
          tunnel: [u32 0 u32 0] -> w1219
          tunnel: [w1247 w1266] -> w1227
          tunnel: "Background" ("name or relative path") -> [w1246 w1258]
          tunnel: "Calibration" -> [w1244 w1257]
          tunnel: [w1240 w1259] -> w1224
          tunnel: w1223 -> [_ _]
          tunnel: ["" ("Empty String Constant") "Case: getRunID\nCase: getBGID\nCase: getCaliID\nUI: Update"] -> w1222
          frame False {
            # "Folder not exist. Creat folders."
            n587 = Create Folder(path (use dialog)=w1253, error in=w1251) -> (created path=w1245:path, error out=w1242:errorcluster)  [unwired: 1 in, 1 out]
            n588 = Build Path(base path=w1245, name or relative path=w1244) -> (appended path=w1243:path)
            n589 = Build Path(base path=w1245, name or relative path=w1246) -> (appended path=w1252:path)
            n590 = Create Folder(path (use dialog)=w1252, error in=w1242) -> (created path=w1247:path, error out=w1248:errorcluster)  [unwired: 1 in, 1 out]
            n591 = Create Folder(path (use dialog)=w1243, error in=w1242) -> (created path=w1240:path, error out=w1241:errorcluster)  [unwired: 1 in, 1 out]
            n592 = Merge Errors(w1248, w1241) -> (w1249:errorcluster)
          }
          frame True {
            # "Folder exsit, check file #"
            n593 = Build Path(base path=w1261, name or relative path=w1257) -> (appended path=w1262:path)
            n594 = Build Path(base path=w1261, name or relative path=w1258) -> (appended path=w1267:path)
            n595 = call <vilib>:"Check if File or Folder Exists.vi"("path"=w1262) -> ("file or folder exists?"=w1260:bool, "dup path"=w1259:path)  [unwired: 8 in, 1 out]
            n596 = call <vilib>:"Check if File or Folder Exists.vi"("path"=w1267) -> ("file or folder exists?"=w1265:bool, "dup path"=w1266:path)  [unwired: 8 in, 1 out]
            n597 = And(x=w1265, y=w1260) -> (x .and. y?=w1264:bool)
            n598 = case shown="False" w1264 {
              tunnel: w1256 -> [_ w1269]
              tunnel: [errorcluster {"status"=TRUE, "code"=5003, "source"="File structure error."} ("error out") w1269] -> w1263
              frame False {
              }
              frame True {
              }
            }
          }
        }
        n599 = Bundle By Name(cluster=w1230, "Pathes.DataPath"=w1221, "Pathes.BG Path"=w1227, "Pathes.CaliPath"=w1224, "IDs.RunID"=w1219, "IDs.BG ID"=w1219, "IDs.Cali ID"=w1219) -> (w1231:T27)
        n600 = call "DataRootPathFGV.vi"("Error In"=w1220, "PathIn"=w1221) -> ("Error Out"=w1218:errorcluster)  [unwired: 8 in, 1 out]
        n601 = call "RunIDFGV.vi"("Error In"=w1218, "RunID in"=w1219) -> ("Error Out"=w1217:errorcluster)  [unwired: 8 in, 1 out]
        n602 = call <vilib>:"Add State(s) to Queue__JKI_lib_State_Machine.vi"("State(s) in Front (\"\")"=w1222, "State(s) in (\"\")"=w1238) -> ("States Out"=w1237:string)  [unwired: 13 in]
      }
      frame "Case: GetID" {
        # "Template Separator\n(You can make a copy of, or modify, this frame)"
        n603 = call "set_subjectID.vi"() -> ("subject_id"=w1270:string)  [unwired: 10 in]
        n604 = Bundle By Name(cluster=w1272, "CaseID"=w1270) -> (w1273:T27)
        n605 = call <vilib>:"Add State(s) to Queue__JKI_lib_State_Machine.vi"("State(s) in (\"\")"=w1276) -> ("States Out"=w1275:string)  [unwired: 14 in]
      }
      frame "---------- DeconEngine ----------" {
        # "start data aquisition and then set irfAligh to ture and decon channel to 1,2 and 3."
        # "Template Separator\n(You can make a copy of, or modify, this frame)"
        n606 = call <vilib>:"Add State(s) to Queue__JKI_lib_State_Machine.vi"("State(s) in (\"\")"=w1281) -> ("States Out"=w1280:string)  [unwired: 14 in]
      }
      frame "DeconEngine: InitilizeMacro" {
        # "start data aquisition and then set irfAligh to ture and decon channel to 1,2 and 3."
        # "Initilize Decon Engine for all channel\n(You can make a copy of, or modify, this frame)"
        n607 = call <vilib>:"Add State(s) to Queue__JKI_lib_State_Machine.vi"("State(s) in Front (\"\")"="DeconEngine: InitializeCh1\nDeconEngine: InitializeCh2\nDeconEngine: InitializeCh3\nDeconEngine: InitializeCh4" ("State(s) in Front (\"\")"), "State(s) in (\"\")"=w1287) -> ("States Out"=w1286:string)  [unwired: 13 in]
      }
      frame "DeconEngine: InitializeCh1" {
        w1309 = refnum<class "LaguerreDeconEngineClass.lvclass"> refnum  # Ch1DeconObj
        # "Initilize Laguerre Deconvolution engine Object\n(You can make a copy of, or modify, this frame)"
        n608 = global read "GlobalVariables.vi" "LastUseiRF"() -> (w1290:T16)
        n609 = local read "Truncation"() -> (w1288:u32)
        n610 = call "setLaguerreOrder.vi"("error in (no error)"=w1297, "LaguerreOrder"=u32 12, "LaguerreDeconClass in"=w1309) -> ("error out"=w1306:errorcluster, "LaguerreDeconClass out"=w1307:refnum<class "LaguerreDeconEngineClass.lvclass">)  [unwired: 7 in]
        n611 = Unbundle By Name(w1290) -> ("Ch1 iRF"=w1289:dbl[])
        n612 = call "setDataLength.vi"("error in (no error)"=w1306, "dataLength"=w1288, "LaguerreDeconClass in"=w1307) -> ("error out"=w1305:errorcluster, "LaguerreDeconClass out"=w1304:refnum<class "LaguerreDeconEngineClass.lvclass">)  [unwired: 7 in]
        n613 = call "setIRF.vi"("error in (no error)"=w1305, "iRF"=w1289, "LaguerreDeconClass in"=w1304) -> ("error out"=w1302:errorcluster, "LaguerreDeconClass out"=w1303:refnum<class "LaguerreDeconEngineClass.lvclass">)  [unwired: 7 in]
        n614 = call "computeAlpha.vi"("error in (no error)"=w1302, "LaguerreDeconClass in"=w1303) -> ("error out"=w1300:errorcluster, "LaguerreDeconClass out"=w1301:refnum<class "LaguerreDeconEngineClass.lvclass">)  [unwired: 8 in]
        n615 = call "dataInitilize.vi"("error in (no error)"=w1300, "LaguerreDeconClass in"=w1301) -> ("error out"=w1298:errorcluster, "LaguerreDeconClass out"=w1299:refnum<class "LaguerreDeconEngineClass.lvclass">)  [unwired: 8 in]
        n616 = call "computeDeconMatrix.vi"("error in (no error)"=w1298, "LaguerreDeconClass in"=w1299) -> ("error out"=w1294:errorcluster, "LaguerreDeconClass out"=w1296:refnum<class "LaguerreDeconEngineClass.lvclass">)  [unwired: 8 in]
        n617 = call "Ch1DeconEngineFGV.vi"("Error In"=w1294, "action(read)"=enum16{"write", "read"}."write" ("action"), "Ch1DeconEngine in"=w1296) -> ("Error Out"=w1293:errorcluster)  [unwired: 7 in, 1 out]
        n618 = call <vilib>:"Add State(s) to Queue__JKI_lib_State_Machine.vi"("State(s) in (\"\")"=w1311) -> ("States Out"=w1310:string)  [unwired: 14 in]
      }
      frame "DeconEngine: InitializeCh2" {
        w1333 = refnum<class "LaguerreDeconEngineClass.lvclass"> refnum  # Ch2DeconObj
        # "Initilize Laguerre Deconvolution engine Object\n(You can make a copy of, or modify, this frame)"
        n619 = global read "GlobalVariables.vi" "LastUseiRF"() -> (w1314:T16)
        n620 = call "setLaguerreOrder.vi"("error in (no error)"=w1321, "LaguerreOrder"=u32 12, "LaguerreDeconClass in"=w1333) -> ("error out"=w1330:errorcluster, "LaguerreDeconClass out"=w1331:refnum<class "LaguerreDeconEngineClass.lvclass">)  [unwired: 7 in]
        n621 = local read "Truncation"() -> (w1312:u32)
        n622 = Unbundle By Name(w1314) -> ("Ch2 iRF"=w1313:dbl[])
        n623 = call "setDataLength.vi"("error in (no error)"=w1330, "dataLength"=w1312, "LaguerreDeconClass in"=w1331) -> ("error out"=w1329:errorcluster, "LaguerreDeconClass out"=w1328:refnum<class "LaguerreDeconEngineClass.lvclass">)  [unwired: 7 in]
        n624 = call "setIRF.vi"("error in (no error)"=w1329, "iRF"=w1313, "LaguerreDeconClass in"=w1328) -> ("error out"=w1326:errorcluster, "LaguerreDeconClass out"=w1327:refnum<class "LaguerreDeconEngineClass.lvclass">)  [unwired: 7 in]
        n625 = call "computeAlpha.vi"("error in (no error)"=w1326, "LaguerreDeconClass in"=w1327) -> ("error out"=w1324:errorcluster, "LaguerreDeconClass out"=w1325:refnum<class "LaguerreDeconEngineClass.lvclass">)  [unwired: 8 in]
        n626 = call "dataInitilize.vi"("error in (no error)"=w1324, "LaguerreDeconClass in"=w1325) -> ("error out"=w1322:errorcluster, "LaguerreDeconClass out"=w1323:refnum<class "LaguerreDeconEngineClass.lvclass">)  [unwired: 8 in]
        n627 = call "computeDeconMatrix.vi"("error in (no error)"=w1322, "LaguerreDeconClass in"=w1323) -> ("error out"=w1318:errorcluster, "LaguerreDeconClass out"=w1320:refnum<class "LaguerreDeconEngineClass.lvclass">)  [unwired: 8 in]
        n628 = call "Ch2DeconEngineFGV.vi"("Error In"=w1318, "action(read)"=enum16{"write", "read"}."write" ("action"), "Ch2DeconEngine in"=w1320) -> ("Error Out"=w1317:errorcluster)  [unwired: 7 in, 1 out]
        n629 = call <vilib>:"Add State(s) to Queue__JKI_lib_State_Machine.vi"("State(s) in (\"\")"=w1335) -> ("States Out"=w1334:string)  [unwired: 14 in]
      }
      frame "DeconEngine: InitializeCh3" {
        w1337 = refnum<class "LaguerreDeconEngineClass.lvclass"> refnum  # Ch3DeconObj
        # "Initilize Laguerre Deconvolution engine Object\n(You can make a copy of, or modify, this frame)"
        n630 = global read "GlobalVariables.vi" "LastUseiRF"() -> (w1339:T16)
        n631 = local read "Truncation"() -> (w1336:u32)
        n632 = call "setLaguerreOrder.vi"("error in (no error)"=w1346, "LaguerreOrder"=u32 12, "LaguerreDeconClass in"=w1337) -> ("error out"=w1355:errorcluster, "LaguerreDeconClass out"=w1356:refnum<class "LaguerreDeconEngineClass.lvclass">)  [unwired: 7 in]
        n633 = Unbundle By Name(w1339) -> ("Ch3 iRF"=w1338:dbl[])
        n634 = call "setDataLength.vi"("error in (no error)"=w1355, "dataLength"=w1336, "LaguerreDeconClass in"=w1356) -> ("error out"=w1354:errorcluster, "LaguerreDeconClass out"=w1353:refnum<class "LaguerreDeconEngineClass.lvclass">)  [unwired: 7 in]
        n635 = call "setIRF.vi"("error in (no error)"=w1354, "iRF"=w1338, "LaguerreDeconClass in"=w1353) -> ("error out"=w1351:errorcluster, "LaguerreDeconClass out"=w1352:refnum<class "LaguerreDeconEngineClass.lvclass">)  [unwired: 7 in]
        n636 = call "computeAlpha.vi"("error in (no error)"=w1351, "LaguerreDeconClass in"=w1352) -> ("error out"=w1349:errorcluster, "LaguerreDeconClass out"=w1350:refnum<class "LaguerreDeconEngineClass.lvclass">)  [unwired: 8 in]
        n637 = call "dataInitilize.vi"("error in (no error)"=w1349, "LaguerreDeconClass in"=w1350) -> ("error out"=w1347:errorcluster, "LaguerreDeconClass out"=w1348:refnum<class "LaguerreDeconEngineClass.lvclass">)  [unwired: 8 in]
        n638 = call "computeDeconMatrix.vi"("error in (no error)"=w1347, "LaguerreDeconClass in"=w1348) -> ("error out"=w1343:errorcluster, "LaguerreDeconClass out"=w1345:refnum<class "LaguerreDeconEngineClass.lvclass">)  [unwired: 8 in]
        n639 = call "Ch3DeconEngineFGV.vi"("Error In"=w1343, "action(read)"=enum16{"write", "read"}."write" ("action"), "Ch3DeconEngine in"=w1345) -> ("Error Out"=w1342:errorcluster)  [unwired: 7 in, 1 out]
        n640 = call <vilib>:"Add State(s) to Queue__JKI_lib_State_Machine.vi"("State(s) in (\"\")"=w1359) -> ("States Out"=w1358:string)  [unwired: 14 in]
      }
      frame "DeconEngine: InitializeCh4" {
        w1361 = refnum<class "LaguerreDeconEngineClass.lvclass"> refnum  # Ch3DeconObj
        # "Initilize Laguerre Deconvolution engine Object\n(You can make a copy of, or modify, this frame)"
        n641 = global read "GlobalVariables.vi" "LastUseiRF"() -> (w1363:T16)
        n642 = local read "Truncation"() -> (w1360:u32)
        n643 = call "setLaguerreOrder.vi"("error in (no error)"=w1370, "LaguerreOrder"=u32 12, "LaguerreDeconClass in"=w1361) -> ("error out"=w1379:errorcluster, "LaguerreDeconClass out"=w1380:refnum<class "LaguerreDeconEngineClass.lvclass">)  [unwired: 7 in]
        n644 = Unbundle By Name(w1363) -> ("Ch4 iRF"=w1362:dbl[])
        n645 = call "setDataLength.vi"("error in (no error)"=w1379, "dataLength"=w1360, "LaguerreDeconClass in"=w1380) -> ("error out"=w1378:errorcluster, "LaguerreDeconClass out"=w1377:refnum<class "LaguerreDeconEngineClass.lvclass">)  [unwired: 7 in]
        n646 = call "setIRF.vi"("error in (no error)"=w1378, "iRF"=w1362, "LaguerreDeconClass in"=w1377) -> ("error out"=w1375:errorcluster, "LaguerreDeconClass out"=w1376:refnum<class "LaguerreDeconEngineClass.lvclass">)  [unwired: 7 in]
        n647 = call "computeAlpha.vi"("error in (no error)"=w1375, "LaguerreDeconClass in"=w1376) -> ("error out"=w1373:errorcluster, "LaguerreDeconClass out"=w1374:refnum<class "LaguerreDeconEngineClass.lvclass">)  [unwired: 8 in]
        n648 = call "dataInitilize.vi"("error in (no error)"=w1373, "LaguerreDeconClass in"=w1374) -> ("error out"=w1371:errorcluster, "LaguerreDeconClass out"=w1372:refnum<class "LaguerreDeconEngineClass.lvclass">)  [unwired: 8 in]
        n649 = call "computeDeconMatrix.vi"("error in (no error)"=w1371, "LaguerreDeconClass in"=w1372) -> ("error out"=w1367:errorcluster, "LaguerreDeconClass out"=w1369:refnum<class "LaguerreDeconEngineClass.lvclass">)  [unwired: 8 in]
        n650 = call "Ch4DeconEngineFGV.vi"("Error In"=w1367, "action(read)"=enum16{"write", "read"}."write" ("action"), "Ch3DeconEngine in"=w1369) -> ("Error Out"=w1366:errorcluster)  [unwired: 7 in, 1 out]
        n651 = call <vilib>:"Add State(s) to Queue__JKI_lib_State_Machine.vi"("State(s) in (\"\")"=w1383) -> ("States Out"=w1382:string)  [unwired: 14 in]
      }
      frame "---------- Digitizer ----------" {
        # "Template Separator\n(You can make a copy of, or modify, this frame)"
        n652 = call <vilib>:"Add State(s) to Queue__JKI_lib_State_Machine.vi"("State(s) in (\"\")"=w1388) -> ("States Out"=w1387:string)  [unwired: 14 in]
      }
      frame "Digitizer: Initialize" {
        # "reset digitizer to everytime the system runs"
        # "reset digitizer to everytime the system runs"
        # "Initialize digitizer.\nInitialize both digitizer and update status."
        n653 = call "FLImDAQ_FGV.vi"("error in (no error)"=w1396) -> ("error out"=w1390:errorcluster, "Read data"=w1395:T7)  [unwired: 9 in]
        n654 = Unbundle By Name(w1398) -> ("SysConfigCluster.Ch1Enable?"=w1403:bool, "SysConfigCluster.Ch2Enable?"=w1402:bool, "SysConfigCluster.Ch3Enable?"=w1400:bool)
        n655 = Unbundle By Name(w1395) -> ("Digitizer 1"=w1391:refnum<k15>, "Digitizer 2"=w1394:refnum<k15>)
        n656 = property on="Digitizer" class="Bool (strict)"("Blinking"=TRUE) -> ()  [unwired: 2 in, 2 out]
        n657 = Or(x=w1403, y=w1402) -> (x .or. y?=w1401:bool)
        n658 = case shown="True" w1401 {
          tunnel: w1390 -> [w1411 w1414]
          tunnel: [w1411 w1413] -> w1392
          tunnel: w1391 -> [_ w1415]
          frame False {
          }
          frame True {
            n659 = call <instrlib>:"niScope Initialize.vi"("resource name"=w1415, "reset device"=TRUE, "error in"=w1414) -> ("error out"=w1413:errorcluster)  [unwired: 11 in, 1 out]
          }
        }
        n660 = case shown="True" w1400 {
          tunnel: w1390 -> [w1406 w1408]
          tunnel: [w1406 w1410] -> w1397
          tunnel: w1394 -> [_ w1409]
          frame False {
          }
          frame True {
            n661 = call <instrlib>:"niScope Initialize.vi"("resource name"=w1409, "reset device"=TRUE, "error in"=w1408) -> ("error out"=w1410:errorcluster)  [unwired: 11 in, 1 out]
          }
        }
        n662 = Merge Errors(w1392, w1397) -> (w1389:errorcluster)
        n663 = call <vilib>:"Add State(s) to Queue__JKI_lib_State_Machine.vi"("State(s) in (\"\")"=w1405) -> ("States Out"=w1404:string)  [unwired: 14 in]
      }
      frame "Digitizer: Config" {
        # "Synchronize is taking time ~3s."
        # "Config  digitizer\nCall subVi to config digitizer"
        n664 = call "FLImDAQ_FGV.vi"() -> ("Read data"=w1433:T7)  [unwired: 10 in, 1 out]
        n665 = Unbundle By Name(w1442) -> ("SysConfigCluster.Ch1Enable?"=w1450:bool, "SysConfigCluster.Ch2Enable?"=w1449:bool, "SysConfigCluster.Ch3Enable?"=w1447:bool, "FLImDAQ"=w1444:T34)
        n666 = Unbundle By Name(w1433) -> ("Digitizer 1"=w1436:refnum<k15>, "Digitizer 2"=w1435:refnum<k15>)
        n667 = property on="Digitizer" class="Bool (strict)"(error in=w1437, "Blinking"=TRUE) -> (error out=w1438:errorcluster)  [unwired: 1 in, 1 out]
        n668 = Or(x=w1450, y=w1449) -> (x .or. y?=w1448:bool)
        n669 = case shown="True" w1448 {
          tunnel: w1444 -> [_ w1463]
          tunnel: w1438 -> [w1459 w1462]
          tunnel: [w1459 w1461] -> w1445
          tunnel: w1436 -> [_ w1460]
          frame False {
          }
          frame True {
            n670 = call "DigitizerConfig.vi"("error in (no error)"=w1462, "FLImDAQ"=w1463, "IVI Refnum in"=w1460) -> ("error out"=w1461:errorcluster)  [unwired: 7 in, 1 out]
          }
        }
        n671 = case shown="True" w1447 {
          tunnel: w1444 -> [_ w1458]
          tunnel: w1445 -> [w1453 w1457]
          tunnel: [w1453 w1456] -> w1421
          tunnel: w1435 -> [_ w1454]
          frame False {
          }
          frame True {
            n672 = call "DigitizerConfig.vi"("Config Trigger? (T)"=FALSE ("Config Trigge(T)r:"), "error in (no error)"=w1457, "FLImDAQ"=w1458, "IVI Refnum in"=w1454) -> ("error out"=w1456:errorcluster)  [unwired: 6 in, 1 out]
          }
        }
        n673 = call "Digitizer1_FGV.vi"("error in (no error)"=w1421) -> ("error out"=w1431:errorcluster, "Read data"=w1432:refnum<k15>)  [unwired: 9 in]
        n674 = call <instrlib>:"niScope Get Session Reference.vi"("instrument handle"=w1432, "error in"=w1431) -> ("session reference"=w1425:refnum<k20>, "error out"=w1423:errorcluster)  [unwired: 11 in, 1 out]
        n675 = call "Digitizer2_FGV.vi"("error in (no error)"=w1423) -> ("error out"=w1429:errorcluster, "Read data"=w1430:refnum<k15>)  [unwired: 9 in]
        n676 = call <instrlib>:"niScope Get Session Reference.vi"("instrument handle"=w1430, "error in"=w1429) -> ("session reference"=w1424:refnum<k20>, "error out"=w1422:errorcluster)  [unwired: 11 in, 1 out]
        n677 = Build Array(w1425, w1424) -> (w1428:refnum<k20>[])
        n678 = call <instrlib>:"niTClk Configure For Homogeneous Triggers.vi"("error in (no error)"=w1422, "sessions"=w1428) -> ("error out"=w1427:errorcluster, "sessions out"=w1426:refnum<k20>[])  [unwired: 8 in]
        n679 = call <instrlib>:"niTClk Synchronize.vi"("error in (no error)"=w1427, "sessions"=w1426) -> ("error out"=w1420:errorcluster, "sessions out"=w1418:refnum<k20>[])  [unwired: 8 in]
        n680 = call <userlib>:"Wait (ms)__ogtk.vi"("error in (no error)"=w1420, "milliseconds to wait"=u32 1500) -> ("error out"=w1416:errorcluster)  [unwired: 8 in, 1 out]
        n681 = Unbundle By Name(w1416) -> ("status"=w1441:bool)
        n682 = Not(x=w1441) -> (.not. x?=w1440:bool)
        n683 = Bundle By Name(cluster=w1442, "System Status.Digitizer"=w1440, "niTClk sessions"=w1418) -> (w1443:T27)
        n684 = property on="Digitizer" class="Bool (strict)"(error in=w1416, "Blinking"=FALSE) -> (error out=w1434:errorcluster)  [unwired: 1 in, 1 out]
        n685 = call <vilib>:"Add State(s) to Queue__JKI_lib_State_Machine.vi"("State(s) in (\"\")"=w1452) -> ("States Out"=w1451:string)  [unwired: 14 in]
      }
      frame "Digitizer: Start" {
        # "send trigger to start acquisition loop"
        # "initilize aquisition"
        # "Start Digitizer\n(TClk start)"
        n686 = Unbundle By Name(w1471) -> ("niTClk sessions"=w1470:refnum<k20>[])
        n687 = call <instrlib>:"niTClk Initiate.vi"("error in (no error)"=w1464, "sessions"=w1470) -> ("error out"=w1466:errorcluster)  [unwired: 8 in, 1 out]
        n688 = Generate User Event(priority (normal)=usereventprio."high priority", user event=w1467, event data cluster=TRUE ("event data"), error in=w1466) -> (error out=w1465:errorcluster)  [unwired: 1 out]
        n689 = call <vilib>:"Add State(s) to Queue__JKI_lib_State_Machine.vi"("State(s) in (\"\")"=w1474) -> ("States Out"=w1473:string)  [unwired: 14 in]
      }
      frame "Digitizer: Abort" {
        # "Template Separator\n(You can make a copy of, or modify, this frame)"
        n690 = call "Digitizer1_FGV.vi"("error in (no error)"=w1478, "Operation (Read)"=enum16{"Write", "Read"}."Read" ("Operation")) -> ("error out"=w1485:errorcluster, "Read data"=w1482:refnum<k15>)  [unwired: 8 in]
        n691 = call "Digitizer2_FGV.vi"("error in (no error)"=w1478, "Operation (Read)"=enum16{"Write", "Read"}."Read" ("Operation")) -> ("error out"=w1481:errorcluster, "Read data"=w1483:refnum<k15>)  [unwired: 8 in]
        n692 = Bundle By Name(cluster=w1475, "SysRunning?"=FALSE ("System Status")) -> (w1476:T27)
        n693 = call <instrlib>:"niScope Abort.vi"("instrument handle"=w1482, "error in"=w1485) -> ("error out"=w1487:errorcluster)  [unwired: 12 in, 1 out]
        n694 = call <instrlib>:"niScope Abort.vi"("instrument handle"=w1483, "error in"=w1481) -> ("error out"=w1486:errorcluster)  [unwired: 12 in, 1 out]
        n695 = Merge Errors(w1487, w1486) -> (w1479:errorcluster)
        n696 = call <vilib>:"Add State(s) to Queue__JKI_lib_State_Machine.vi"("State(s) in (\"\")"=w1490) -> ("States Out"=w1489:string)  [unwired: 14 in]
      }
      frame "Digitizer: checkTemp" {
        w1493 = 65.0 ("y")
        w1498 = enum16{"Write", "Read"}."Read" ("Operation")
        # "Template Separator\n(You can make a copy of, or modify, this frame)"
        n697 = call "Digitizer1_FGV.vi"("Operation (Read)"=w1498) -> ("error out"=w1499:errorcluster, "Read data"=w1500:refnum<k15>)  [unwired: 9 in]
        n698 = call "Digitizer2_FGV.vi"("Operation (Read)"=w1498) -> ("error out"=w1496:errorcluster, "Read data"=w1497:refnum<k15>)  [unwired: 9 in]
        n699 = property on="Property Node" class="niScope"(reference=w1497, error in=w1496) -> ("Device Temperature"=w1494:dbl)  [unwired: 2 out]
        "Dig2 Temp" <- w1494
        n700 = property on="Property Node" class="niScope"(reference=w1500, error in=w1499) -> ("Device Temperature"=w1495:dbl)  [unwired: 2 out]
        "Dig1 Temp" <- w1495
        n701 = Greater?(x=w1495, y=w1493) -> (0:w1492:bool)
        n702 = Greater?(x=w1494, y=w1493) -> (0:w1491:bool)
        n703 = case shown="True" w1492 {
          frame False {
          }
          frame True {
            n704 = One Button Dialog(message="Digitizer 1 over heating!", button name ("OK")="OK") -> ()  [unwired: 1 out]
          }
        }
        n705 = case shown="True" w1491 {
          frame False {
          }
          frame True {
            n706 = One Button Dialog(message="Digitizer 2 over heating!", button name ("OK")="OK") -> ()  [unwired: 1 out]
          }
        }
        n707 = call <vilib>:"Add State(s) to Queue__JKI_lib_State_Machine.vi"("State(s) in (\"\")"=w1505) -> ("States Out"=w1504:string)  [unwired: 14 in]
      }
      frame "Digitizer: Close" {
        # "Close Digitizer"
        n708 = call "Digitizer1_FGV.vi"("error in (no error)"=w1515, "Operation (Read)"=enum16{"Write", "Read"}."Read" ("Operation")) -> ("error out"=w1517:errorcluster, "Read data"=w1521:refnum<k15>)  [unwired: 8 in]
        n709 = call "Digitizer2_FGV.vi"("error in (no error)"=w1515, "Operation (Read)"=enum16{"Write", "Read"}."Read" ("Operation")) -> ("error out"=w1516:errorcluster, "Read data"=w1519:refnum<k15>)  [unwired: 8 in]
        n710 = call <instrlib>:"niScope Close.vi"("instrument handle"=w1521, "error in"=w1517) -> ("error out"=w1514:errorcluster)  [unwired: 13 in]
        n711 = call <instrlib>:"niScope Close.vi"("instrument handle"=w1519, "error in"=w1516) -> ("error out"=w1513:errorcluster)  [unwired: 13 in]
        n712 = Merge Errors(w1514, w1513) -> (w1512:errorcluster)
        n713 = Unbundle By Name(w1512) -> ("status"=w1511:bool)
        n714 = Bundle By Name(cluster=w1522, "System Status.Digitizer"=w1511) -> (w1523:T27)
        n715 = call <vilib>:"Add State(s) to Queue__JKI_lib_State_Machine.vi"("State(s) in (\"\")"=w1525) -> ("States Out"=w1524:string)  [unwired: 14 in]
      }
      frame "---------- LabJack ----------" {
        # "Template Separator\n(You can make a copy of, or modify, this frame)"
        n716 = call <vilib>:"Add State(s) to Queue__JKI_lib_State_Machine.vi"("State(s) in (\"\")"=w1530) -> ("States Out"=w1529:string)  [unwired: 14 in]
      }
      frame "LabJack: checkPedal" {
        # "Template Separator\n(You can make a copy of, or modify, this frame)"
        n717 = Unbundle By Name(w1531) -> ("LJ Pinout.Foot Pedal"=w1535:string)
        n718 = call "LabJack_FGV.vi"("Operation(Read)"=enum16{"Write", "Read"}."Read" ("Operation"), "error in (no error)"=w1533) -> ("error out"=w1537:errorcluster, "Read data"=w1538:i32)  [unwired: 8 in]
        n719 = call "LJM_eReadName.vi"("Handle In"=w1538, "Name"=w1535, "error in"=w1537) -> ("Value"=w1536:dbl, "error out"=w1534:errorcluster)  [unwired: 10 in, 1 out]
        n720 = case shown="1" w1536 {
          tunnel: w1531 -> [w1543 w1546]
          tunnel: [w1543 w1544] -> w1532
          frame 0, Default {
          }
          frame 1 {
            # "If Pedal pressed"
            n721 = Tick Count (ms)() -> (millisecond timer value=w1550:u32)
            n722 = Unbundle By Name(w1546) -> ("Last Trigger"=w1545:u32)
            n723 = Subtract(x=w1550, y=w1545) -> (x-y=w1549:u32)
            n724 = Greater Or Equal?(x=w1549, y=u32 2000) -> (x >= y?=w1547:bool)
            n725 = case shown="True" w1547 {
              tunnel: w1546 -> [w1551 w1552]
              tunnel: w1545 -> [_ _]
              tunnel: [w1551 w1553] -> w1544
              frame False {
              }
              frame True {
                n726 = Tick Count (ms)() -> (millisecond timer value=w1554:u32)
                n727 = Unbundle By Name(w1552) -> ("SysRunning?"=w1555:bool)
                n728 = case shown="False" w1555 {
                  frame False {
                    n729 = property on="StartButton" class="Bool (strict)"("Val(Sgnl)"=TRUE ("Value (Signaling)")) -> ()  [unwired: 2 in, 2 out]
                  }
                  frame True {
                    n730 = property on="StopButton" class="Bool (strict)"("Val(Sgnl)"=TRUE ("Value (Signaling)")) -> ()  [unwired: 2 in, 2 out]
                  }
                }
                n731 = Bundle By Name(cluster=w1552, "Last Trigger"=w1554) -> (w1553:T27)
              }
            }
          }
        }
        n732 = call <vilib>:"Add State(s) to Queue__JKI_lib_State_Machine.vi"("State(s) in (\"\")"=w1542) -> ("States Out"=w1541:string)  [unwired: 14 in]
      }
      frame "LabJack: ZeroV" {
        # "Just Zero V\nDO not update FGV and front panel\nWIll resume from last V"
        # "set bias to 0"
        # "Zero APD bias\n(You can make a copy of, or modify, this frame)"
        n733 = Unbundle By Name(w1560) -> ("LJ Pinout.Ch1 Bias"=w1565:string, "LJ Pinout.Ch2 Bias"=w1564:string, "LJ Pinout.Ch3 Bias"=w1563:string)
        n734 = Build Array(w1565, w1564, w1563) -> (w1562:string[])
        n735 = call "LabJack_FGV.vi"("Operation(Read)"=enum16{"Write", "Read"}."Read" ("Operation"), "error in (no error)"=w1559) -> ("error out"=w1566:errorcluster, "Read data"=w1567:i32)  [unwired: 8 in]
        n736 = call "LJM_eWriteNames.vi"("Handle In"=w1567, "aNames"=w1562, "aValuesIn"=dbl[] [0.0, 0.0, 0.0], "error in"=w1566) -> ("error out"=w1558:errorcluster)  [unwired: 9 in, 2 out]
        n737 = call <vilib>:"Add State(s) to Queue__JKI_lib_State_Machine.vi"("State(s) in (\"\")"=w1571) -> ("States Out"=w1570:string)  [unwired: 14 in]
      }
      frame "LabJack: SetV" {
        w1578 = enum16{"write", "read"}."read" ("action (write)")
        # "set bias to user specifid"
        # "Set APD bias\n(You can make a copy of, or modify, this frame)"
        n738 = Unbundle By Name(w1587) -> ("LJ Pinout.Ch1 Bias"=w1591:string, "LJ Pinout.Ch2 Bias"=w1590:string, "LJ Pinout.Ch3 Bias"=w1589:string, "LJ Pinout.Ch4 Bias"=w1581:string)
        n739 = call "V2FGV.vi"("Error In"=w1577, "action(write)"=w1578) -> ("Error Out"=w1575:errorcluster, "V2 out"=w1583:dbl)  [unwired: 8 in]
        n740 = call "V4FGV.vi"("Error In"=w1577, "action(write)"=w1578) -> ("Error Out"=w1573:errorcluster, "V3 out"=w1579:dbl)  [unwired: 8 in]
        n741 = call "V1FGV.vi"("Error In"=w1577, "action (write)"=w1578) -> ("Error Out"=w1576:errorcluster, "V1 out"=w1580:dbl)  [unwired: 8 in]
        n742 = call "V3FGV.vi"("Error In"=w1577, "action(write)"=w1578) -> ("Error Out"=w1574:errorcluster, "V3 out"=w1582:dbl)  [unwired: 8 in]
        n743 = local write "V 3"(w1582) -> ()
        n744 = local write "V 2"(w1583) -> ()
        n745 = local write "V 4"(w1579) -> ()
        n746 = local write "V 1"(w1580) -> ()
        n747 = Build Array(w1591, w1590, w1589, w1581) -> (w1588:string[])
        n748 = call "LabJack_FGV.vi"("Operation(Read)"=enum16{"Write", "Read"}."Read" ("Operation"), "error in (no error)"=w1577) -> ("error out"=w1592:errorcluster, "Read data"=w1593:i32)  [unwired: 8 in]
        n749 = Build Array(w1580, w1583, w1582, w1579) -> (w1584:dbl[])
        n750 = call "LJM_eWriteNames.vi"("Handle In"=w1593, "aNames"=w1588, "aValuesIn"=w1584, "error in"=w1592) -> ("error out"=w1585:errorcluster)  [unwired: 9 in, 2 out]
        n751 = Merge Errors(w1576, w1575, w1574, w1573) -> (w1572:errorcluster)
        n752 = call <vilib>:"Add State(s) to Queue__JKI_lib_State_Machine.vi"("State(s) in (\"\")"=w1597) -> ("States Out"=w1596:string)  [unwired: 14 in]
        n753 = Merge Errors(w1572, w1585) -> (w1586:errorcluster)
      }
      frame "LabJack: Open" {
        # "Initialize LabJack T7\nEstablish connection and initialize pins"
        n754 = call "LJ_Open.vi"("error in"=w1607, "DeviceType"="LJM_dtT7") -> ("error out"=w1604:errorcluster, "Success?"=w1605:bool, "Handle Out"=w1599:i32)  [unwired: 7 in]
        n755 = call "LabJack_FGV.vi"("Operation(Read)"=enum16{"Write", "Read"}."Write" ("Operation"), "error in (no error)"=w1604, "Write data"=w1599) -> ("error out"=w1601:errorcluster)  [unwired: 7 in, 1 out]
        n756 = Bundle By Name(cluster=w1602, "System Status.Labjack"=w1605) -> (w1606:T27)
        n757 = call <vilib>:"Add State(s) to Queue__JKI_lib_State_Machine.vi"("State(s) in (\"\")"=w1609) -> ("States Out"=w1608:string)  [unwired: 14 in]
      }
      frame "LabJack: SetDefaultSub" {
        w1619 = enum16{"write", "read"}."write" ("action")
        w1620 = 0.0 ("V1 in")
        w1633 = "_EF_ENABLE" ("string")
        # "1. Disable PWM\n2. Set all V to 0\n3. Set 355 relay to open\n4. Set LED to off"
        # "read once to set DIO to input"
        # "set all initila V to 0. Set footpedal to input. Set PWM to low. Set laser relay to open. Set LEDs to yellow."
        # "Set Labjack to correct input and output state and initial values"
        n758 = disable-structure shown="Disabled" {
          frame Disabled {
            (unwired) dbl[] [0.0, 0.0, 0.0, 0.0, 0.0, 0.0, 0.0, 0.0, 0.0] ("aValuesIn")
          }
          frame Enabled {
          }
        }
        n759 = Unbundle By Name(w1630) -> ("LJ Pinout.355 PWM"=w1635:string, "LJ Pinout.AimingBeam PWM"=w1634:string, "LJ Pinout.Ch1 Bias"=w1640:string, "LJ Pinout.Ch2 Bias"=w1610:string, "LJ Pinout.Ch3 Bias"=w1644:string, "LJ Pinout.Ch4 Bias"=w1624:string, "LJ Pinout.Laser Start/Stop"=w1643:string, "LJ Pinout.Red LED"=w1642:string, "LJ Pinout.Green LED"=w1641:string)
        n760 = call "V1FGV.vi"("Error In"=w1628, "action (write)"=w1619, "V1 in"=w1620) -> ("Error Out"=w1623:errorcluster, "V1 out"=w1627:dbl)  [unwired: 7 in]
        n761 = local write "V 1"(w1627) -> ()
        n762 = call "V2FGV.vi"("Error In"=w1623, "action(write)"=w1619, "V2 in"=w1620) -> ("Error Out"=w1622:errorcluster, "V2 out"=w1626:dbl)  [unwired: 7 in]
        n763 = call "LabJack_FGV.vi"("Operation(Read)"=enum16{"Write", "Read"}."Read" ("Operation"), "error in (no error)"=w1628) -> ("error out"=w1616:errorcluster, "Read data"=w1638:i32)  [unwired: 8 in]
        n764 = Concatenate Strings(w1635, w1633) -> (w1632:string)
        n765 = Concatenate Strings(w1634, w1633) -> (w1631:string)
        n766 = local write "V 2"(w1626) -> ()
        n767 = call "V3FGV.vi"("Error In"=w1622, "action(write)"=w1619, "V3 in"=w1620) -> ("Error Out"=w1621:errorcluster, "V3 out"=w1625:dbl)  [unwired: 7 in]
        n768 = Build Array(w1632, w1631, w1640, w1610, w1644, w1624, w1643, w1642, w1641) -> (w1614:string[])
        n769 = local write "V 3"(w1625) -> ()
        n770 = call "V4FGV.vi"("Error In"=w1621, "action(write)"=w1619, "V3 in"=w1620) -> ("Error Out"=w1617:errorcluster, "V3 out"=w1618:dbl)  [unwired: 7 in]
        n771 = Array Size(array=w1614) -> (size(s)=w1613:i32)
        n772 = local write "V 4"(w1618) -> ()
        n773 = Initialize Array(0.0 ("element"), w1613) -> (w1611:dbl[])
        n774 = Unbundle By Name(w1630) -> ("LJ Pinout.Foot Pedal"=w1629:string)
        n775 = call "LJM_eWriteNames.vi"("Handle In"=w1638, "aNames"=w1614, "aValuesIn"=w1611, "error in"=w1616) -> ("Handle Out"=w1637:i32, "error out"=w1636:errorcluster)  [unwired: 9 in, 1 out]
        n776 = call "LJM_eReadName.vi"("Handle In"=w1637, "Name"=w1629, "error in"=w1636) -> ("error out"=w1615:errorcluster)  [unwired: 10 in, 2 out]
        n777 = case shown="Error .." w1615 {
          frame No Error {
            # "no error"
          }
          frame Error {
            # "handle error"
            n778 = One Button Dialog(message="Labjack error! The pin assignment is likely wrong. Please check pin setting of Labjack. Program will terminate.", button name ("OK")="OK") -> ()  [unwired: 1 out]
          }
        }
        n779 = call <vilib>:"Add State(s) to Queue__JKI_lib_State_Machine.vi"("State(s) in (\"\")"=w1647) -> ("States Out"=w1646:string)  [unwired: 14 in]
      }
      frame "LabJack: FootPedalConfig" {
        # "Setup footPedal\n(You can make a copy of, or modify, this frame)"
        n780 = call "LabJack_FGV.vi"("Operation(Read)"=enum16{"Write", "Read"}."Read" ("Operation"), "error in (no error)"=w1651) -> ("error out"=w1655:errorcluster, "Read data"=w1656:i32)  [unwired: 8 in]
        n781 = call "LJM_eWriteName.vi"("Handle In"=w1656, "Name"="DIO15", "Value"=1.0, "error in"=w1655) -> ("error out"=w1652:errorcluster)  [unwired: 10 in, 1 out]
        n782 = call <vilib>:"Add State(s) to Queue__JKI_lib_State_Machine.vi"("State(s) in (\"\")"=w1660) -> ("States Out"=w1659:string)  [unwired: 14 in]
      }
      frame "LabJack: SetDefaultAndClose" {
        # "Template Separator\n(You can make a copy of, or modify, this frame)"
        n783 = call <vilib>:"Add State(s) to Queue__JKI_lib_State_Machine.vi"("State(s) in Front (\"\")"="LabJack: SetDefaultSub\nLabJack: Close" ("State(s) in Front (\"\")"), "State(s) in (\"\")"=w1666) -> ("States Out"=w1665:string)  [unwired: 13 in]
      }
      frame "LabJack: Close" {
        # "Close LabJack Refnum"
        n784 = call "LabJack_FGV.vi"("Operation(Read)"=enum16{"Write", "Read"}."Read" ("Operation"), "error in (no error)"=w1672) -> ("error out"=w1667:errorcluster, "Read data"=w1668:i32)  [unwired: 8 in]
        n785 = Bundle By Name(cluster=w1670, "System Status.Labjack"=FALSE ("System Status.Gain Control")) -> (w1673:T27)
        n786 = call "LJM_Close.vi"("error in"=w1667, "Handle"=w1668) -> ("error out"=w1675:errorcluster)  [unwired: 9 in]
        n787 = call <vilib>:"Add State(s) to Queue__JKI_lib_State_Machine.vi"("State(s) in (\"\")"=w1677) -> ("States Out"=w1676:string)  [unwired: 14 in]
      }
      frame "LabJack: Interlock enable/disable" {
        w1686 = i8 0  # int8
        # "[Covers: REQ8]"
        # "Interlock enable/disable\n(Usage: \"LabJack: Interlock enable/disable >> 1|0\")"
        n788 = Fract/Exp String To Number(string=w1687, default (0 dbl)=w1686) -> (number=w1683:i8)  [unwired: 2 in, 1 out]
        n789 = Unbundle By Name(w1685) -> ("LJ Pinout.Interlock"=w1684:string)
        n790 = call "LabJack_FGV.vi"("Operation(Read)"=enum16{"Write", "Read"}."Read" ("Operation")) -> ("Read data"=w1681:i32)  [unwired: 9 in, 1 out]
        n791 = call "LJM_eWriteName.vi"("Handle In"=w1681, "Name"=w1684, "Value"=w1683, "error in"=w1682) -> ("error out"=w1679:errorcluster)  [unwired: 10 in, 1 out]
        n792 = call <vilib>:"Add State(s) to Queue__JKI_lib_State_Machine.vi"("State(s) in (\"\")"=w1689) -> ("States Out"=w1688:string)  [unwired: 14 in]
      }
      frame "LabJack: 355_PWM_Config" {
        w1691 = 0.0 ("element")
        w1711 = "DIO_EF_CLOCK1_ENABLE"
        # "Config PWM frequency"
        n793 = Unbundle By Name(w1703) -> ("LJ Pinout.355 PWM"=w1710:string)
        n794 = Unbundle By Name(w1703) -> ("355 PWM setting.DIO_EF_CLOCK1_DIVISOR"=w1702:i16, "355 PWM setting.DIO_EF_CLOCK1_ROLL_VALUE"=w1701:i32, "355 PWM setting.DIO#_EF_INDEX"=w1698:i16, "355 PWM setting.DIO#_EF_OPTIONS"=w1697:i16, "355 PWM setting.DIO#_EF_CONFIG_A"=w1696:i32)
        n795 = Concatenate Strings(w1710, "_EF_ENABLE" ("string")) -> (w1706:string)
        n796 = Concatenate Strings(w1710, "_EF_INDEX") -> (w1709:string)
        n797 = Concatenate Strings(w1710, "_EF_OPTIONS") -> (w1708:string)
        n798 = Concatenate Strings(w1710, "_EF_CONFIG_A") -> (w1707:string)
        n799 = call "LabJack_FGV.vi"("Operation(Read)"=enum16{"Write", "Read"}."Read" ("Operation")) -> ("Read data"=w1704:i32)  [unwired: 9 in, 1 out]
        n800 = Build Array(w1691, w1691, w1702, w1701, 1.0 ("element"), 0.0 ("element"), w1698, w1697, w1696) -> (w1695:dbl[])
        n801 = Build Array("DIO_EF_CLOCK0_ENABLE", w1711, "DIO_EF_CLOCK1_DIVISOR", "DIO_EF_CLOCK1_ROLL_VALUE", w1711, w1706, w1709, w1708, w1707) -> (w1705:string[])
        n802 = call "LJM_eWriteNames.vi"("Handle In"=w1704, "aNames"=w1705, "aValuesIn"=w1695, "error in"=w1693) -> ("error out"=w1694:errorcluster)  [unwired: 9 in, 2 out]
        n803 = call <vilib>:"Add State(s) to Queue__JKI_lib_State_Machine.vi"("State(s) in (\"\")"=w1720) -> ("States Out"=w1719:string)  [unwired: 14 in]
      }
      frame "LabJack: 355_PWM_Start" {
        # "Template Separator\n(You can make a copy of, or modify, this frame)"
        n804 = Unbundle By Name(w1728) -> ("LJ Pinout.355 PWM"=w1727:string)
        n805 = call "LabJack_FGV.vi"("Operation(Read)"=enum16{"Write", "Read"}."Read" ("Operation"), "error in (no error)"=w1722) -> ("error out"=w1729:errorcluster, "Read data"=w1730:i32)  [unwired: 8 in]
        n806 = Concatenate Strings(w1727, "_EF_ENABLE" ("string")) -> (w1725:string)
        n807 = call "LJM_eWriteName.vi"("Handle In"=w1730, "Name"=w1725, "Value"=1.0, "error in"=w1729) -> ("error out"=w1723:errorcluster)  [unwired: 10 in, 1 out]
        n808 = call <vilib>:"Add State(s) to Queue__JKI_lib_State_Machine.vi"("State(s) in (\"\")"=w1733) -> ("States Out"=w1732:string)  [unwired: 14 in]
      }
      frame "LabJack: 355_PWM_Stop" {
        # "Template Separator\n(You can make a copy of, or modify, this frame)"
        n809 = Unbundle By Name(w1739) -> ("LJ Pinout.355 PWM"=w1743:string)
        n810 = call "LabJack_FGV.vi"("Operation(Read)"=enum16{"Write", "Read"}."Read" ("Operation"), "error in (no error)"=w1738) -> ("error out"=w1744:errorcluster, "Read data"=w1736:i32)  [unwired: 8 in]
        n811 = Concatenate Strings(w1743, "_EF_ENABLE" ("string")) -> (w1741:string)
        n812 = call "LJM_eWriteName.vi"("Handle In"=w1736, "Name"=w1741, "Value"=0.0, "error in"=w1744) -> ("error out"=w1735:errorcluster)  [unwired: 10 in, 1 out]
        n813 = local write "355nm Laser toggle"(FALSE ("355nm Laser toggle")) -> ()
        n814 = call <vilib>:"Add State(s) to Queue__JKI_lib_State_Machine.vi"("State(s) in (\"\")"=w1747) -> ("States Out"=w1746:string)  [unwired: 14 in]
      }
      frame "LabJack: AB_Start" {
        # "Aiming Beam Start\n(Based on aimging beam frequency, set LabJack pin)"
        n815 = Unbundle By Name(w1757) -> ("AB Cluster.Freq"=w1749:i32, "LJ Pinout.AimingBeam PWM"=w1756:string)
        n816 = Greater Than 0?(x=w1749) -> (x > 0?=w1748:bool)
        n817 = case shown="False" w1748 {
          tunnel: w1756 -> [w1763 w1766]
          tunnel: [w1763 w1764] -> w1755
          frame False {
            # "if 0 freq, set PWM pin"
          }
          frame True {
            # "if non zero freq, set PWM enable"
            n818 = Concatenate Strings(w1766, "_EF_ENABLE" ("string")) -> (w1764:string)
          }
        }
        n819 = call "LabJack_FGV.vi"("Operation(Read)"=enum16{"Write", "Read"}."Read" ("Operation"), "error in (no error)"=w1752) -> ("error out"=w1758:errorcluster, "Read data"=w1759:i32)  [unwired: 8 in]
        n820 = call "LJM_eWriteName.vi"("Handle In"=w1759, "Name"=w1755, "Value"=1.0, "error in"=w1758) -> ("error out"=w1753:errorcluster)  [unwired: 10 in, 1 out]
        n821 = local write "Aiming beam toggle"(TRUE ("Aiming beam toggle")) -> ()
        n822 = call <vilib>:"Add State(s) to Queue__JKI_lib_State_Machine.vi"("State(s) in (\"\")"=w1762) -> ("States Out"=w1761:string)  [unwired: 14 in]
      }
      frame "LabJack: AB_Stop" {
        # "Aiming Beam Stop\n(Based on aiming beam frequency, set LabJack pin low)"
        n823 = Unbundle By Name(w1774) -> ("AB Cluster.Freq"=w1769:i32, "LJ Pinout.AimingBeam PWM"=w1776:string)
        n824 = Greater Than 0?(x=w1769) -> (x > 0?=w1768:bool)
        n825 = case shown="False" w1768 {
          tunnel: w1776 -> [w1782 w1785]
          tunnel: [w1782 w1783] -> w1767
          frame False {
          }
          frame True {
            n826 = Concatenate Strings(w1785, "_EF_ENABLE" ("string")) -> (w1783:string)
          }
        }
        n827 = call "LabJack_FGV.vi"("Operation(Read)"=enum16{"Write", "Read"}."Read" ("Operation"), "error in (no error)"=w1772) -> ("error out"=w1777:errorcluster, "Read data"=w1778:i32)  [unwired: 8 in]
        n828 = call "LJM_eWriteName.vi"("Handle In"=w1778, "Name"=w1767, "Value"=0.0, "error in"=w1777) -> ("error out"=w1773:errorcluster)  [unwired: 10 in, 1 out]
        n829 = local write "Aiming beam toggle"(FALSE ("Aiming beam toggle")) -> ()
        n830 = call <vilib>:"Add State(s) to Queue__JKI_lib_State_Machine.vi"("State(s) in (\"\")"=w1781) -> ("States Out"=w1780:string)  [unwired: 14 in]
      }
      frame "LabJack: AB_PWM_Config" {
        w1787 = 0.0 ("element")
        w1807 = "DIO_EF_CLOCK2_ENABLE"
        # "Config PWM frequency"
        n831 = Unbundle By Name(w1799) -> ("LJ Pinout.AimingBeam PWM"=w1806:string)
        n832 = Unbundle By Name(w1799) -> ("AB PWM setting.DIO_EF_CLOCK1_DIVISOR"=w1798:i16, "AB PWM setting.DIO_EF_CLOCK1_ROLL_VALUE"=w1797:i32, "AB PWM setting.DIO#_EF_INDEX"=w1794:i16, "AB PWM setting.DIO#_EF_OPTIONS"=w1793:i16, "AB PWM setting.DIO#_EF_CONFIG_A"=w1792:i32)
        n833 = Concatenate Strings(w1806, "_EF_ENABLE" ("string")) -> (w1802:string)
        n834 = Concatenate Strings(w1806, "_EF_INDEX") -> (w1805:string)
        n835 = Concatenate Strings(w1806, "_EF_OPTIONS") -> (w1804:string)
        n836 = Concatenate Strings(w1806, "_EF_CONFIG_A") -> (w1803:string)
        n837 = call "LabJack_FGV.vi"("Operation(Read)"=enum16{"Write", "Read"}."Read" ("Operation")) -> ("Read data"=w1800:i32)  [unwired: 9 in, 1 out]
        n838 = Build Array(w1787, w1787, w1798, w1797, 1.0 ("element"), 0.0 ("element"), w1794, w1793, w1792) -> (w1791:dbl[])
        n839 = Build Array("DIO_EF_CLOCK0_ENABLE", w1807, "DIO_EF_CLOCK2_DIVISOR", "DIO_EF_CLOCK2_ROLL_VALUE", w1807, w1802, w1805, w1804, w1803) -> (w1801:string[])
        n840 = call "LJM_eWriteNames.vi"("Handle In"=w1800, "aNames"=w1801, "aValuesIn"=w1791, "error in"=w1789) -> ("error out"=w1790:errorcluster)  [unwired: 9 in, 2 out]
        n841 = call <vilib>:"Add State(s) to Queue__JKI_lib_State_Machine.vi"("State(s) in (\"\")"=w1816) -> ("States Out"=w1815:string)  [unwired: 14 in]
      }
      frame "---------- LED ----------" {
        # "Template Separator\n(You can make a copy of, or modify, this frame)"
        n842 = call <vilib>:"Add State(s) to Queue__JKI_lib_State_Machine.vi"("State(s) in (\"\")"=w1821) -> ("States Out"=w1820:string)  [unwired: 14 in]
      }
      frame "LED: OpenVIRef" {
        # "Template Separator\n(You can make a copy of, or modify, this frame)"
        n843 = call <vilib>:"Application Directory.vi"() -> ("Application Directory"=w1828:path)
        n844 = Build Path(base path=w1828, name or relative path="SubVI") -> (appended path=w1826:path)
        n845 = Build Path(base path=w1826, name or relative path="LEDBreath.vi") -> (appended path=w1824:path)
        n846 = Open VI Reference(vi path=w1824, error in (no error)=w1829) -> (vi reference=w1830:refnum<vi>, error out=w1823:errorcluster)  [unwired: 4 in]
        n847 = case shown="Error .." w1823 {
          tunnel: [TRUE FALSE] -> w1822
          frame No Error {
          }
          frame Error {
          }
        }
        n848 = Bundle By Name(cluster=w1831, "LED vi reference"=w1830, "LED vi ref open?"=w1822) -> (w1832:T27)
        n849 = call <vilib>:"Add State(s) to Queue__JKI_lib_State_Machine.vi"("State(s) in (\"\")"=w1835) -> ("States Out"=w1834:string)  [unwired: 14 in]
      }
      frame "LED: CloseVIRef" {
        # "Template Separator\n(You can make a copy of, or modify, this frame)"
        n850 = Unbundle By Name(w1839) -> ("LED vi reference"=w1840:refnum<vi>, "LED vi ref open?"=w1838:bool)
        n851 = case shown="True" w1838 {
          tunnel: w1842 -> [w1846 w1849]
          tunnel: [w1846 w1848] -> w1841
          tunnel: w1840 -> [_ w1847]
          frame False {
          }
          frame True {
            n852 = Close Reference(reference=w1847, error in (no error)=w1849) -> (error out=w1848:errorcluster)
          }
        }
        n853 = call <vilib>:"Add State(s) to Queue__JKI_lib_State_Machine.vi"("State(s) in (\"\")"=w1845) -> ("States Out"=w1844:string)  [unwired: 14 in]
      }
      frame "LED: BreathGreen" {
        w1850 = FALSE ("Wait Until Done")
        # "Breath system LED\n(LED: Breath >> True/False)"
        n854 = Unbundle By Name(w1858) -> ("LED vi reference"=w1857:refnum<vi>)
        n855 = invoke class="VI" method="Ctrl Val.Set"(reference=w1857, error in=w1855, "Control Name"="Color", "Value"=0) -> (reference out=w1854:refnum<vi>, error out=w1853:errorcluster)  [unwired: 1 in, 3 out]
        n856 = invoke on="Invoke Node" class="VI" method="Run VI"(reference=w1854, error in=w1853, "Wait until done"=w1850, "Auto Dispose Ref"=w1850) -> (error out=w1856:errorcluster)  [unwired: 1 in, 4 out]
        n857 = call <vilib>:"Add State(s) to Queue__JKI_lib_State_Machine.vi"("State(s) in (\"\")"=w1861) -> ("States Out"=w1860:string)  [unwired: 14 in]
      }
      frame "LED: BreathOrange" {
        w1862 = FALSE ("Wait Until Done")
        # "Breath system LED\n(LED: Breath >> True/False)"
        n858 = Unbundle By Name(w1870) -> ("LED vi reference"=w1869:refnum<vi>)
        n859 = invoke class="VI" method="Ctrl Val.Set"(reference=w1869, error in=w1867, "Control Name"="Color", "Value"=1) -> (reference out=w1866:refnum<vi>, error out=w1865:errorcluster)  [unwired: 1 in, 3 out]
        n860 = invoke on="Invoke Node" class="VI" method="Run VI"(reference=w1866, error in=w1865, "Wait until done"=w1862, "Auto Dispose Ref"=w1862) -> (error out=w1868:errorcluster)  [unwired: 1 in, 4 out]
        n861 = call <vilib>:"Add State(s) to Queue__JKI_lib_State_Machine.vi"("State(s) in (\"\")"=w1873) -> ("States Out"=w1872:string)  [unwired: 14 in]
      }
      frame "LED: BreathOff" {
        # "System LED Breath Off\n(Breath off, check VI status to make sure it is off)"
        n862 = Unbundle By Name(w1882) -> ("LED vi reference"=w1881:refnum<vi>)
        n863 = invoke on="Invoke Node" class="VI" method="Ctrl Val.Set"(reference=w1881, error in=w1879, "Control Name"="Stop", "Value"=TRUE) -> (reference out=w1874:refnum<vi>, error out=w1875:errorcluster)  [unwired: 1 in, 3 out]
        n864 = case shown="No Error" w1875 {
          selector: w1875 -> [w1887 _]
          tunnel: [w1886 errorcluster {"status"=FALSE, "code"=0, "source"=""} ("error IO")] -> w1880
          tunnel: ["" ("State(s) in Front (\"\")") "LED: BreathOff" ("State(s) in Front (\"\")")] -> w1878
          tunnel: w1874 -> [w1888 _]
          frame No Error {
            # "No error, wait for VI to stop"
            n865 = while {
              tunnel: w1888 -> [w1896]
              shift-right: [w1890] -> w1886
              shift-left: w1887 -> [w1895]
              stop <- w1892 stop-if-true
              # "continue check whether vi is running"
              n866 = property class="VI"(reference=w1896, error in=w1895) -> (error out=w1890:errorcluster, "Exec.State"=w1894:T21)  [unwired: 1 out]
              n867 = Wait (ms)(milliseconds to wait=u32 50) -> ()  [unwired: 1 out]
              n868 = Equal?(x=w1894, y=T21."Idle") -> (x = y?=w1892:bool)
            }
          }
          frame Error {
            # "try again when error"
          }
        }
        n869 = call <vilib>:"Add State(s) to Queue__JKI_lib_State_Machine.vi"("State(s) in Front (\"\")"=w1878, "State(s) in (\"\")"=w1885) -> ("States Out"=w1884:string)  [unwired: 13 in]
      }
      frame "LED: Off" {
        # "set LED to red"
        # "Template Separator\n(You can make a copy of, or modify, this frame)"
        n870 = Unbundle By Name(w1901) -> ("LJ Pinout.Red LED"=w1900:string, "LJ Pinout.Green LED"=w1899:string)
        n871 = call "LabJack_FGV.vi"("Operation(Read)"=enum16{"Write", "Read"}."Read" ("Operation"), "error in (no error)"=w1902) -> ("error out"=w1909:errorcluster, "Read data"=w1908:i32)  [unwired: 8 in]
        n872 = call "LJM_eWriteName.vi"("Handle In"=w1908, "Name"=w1900, "Value"=0.0, "error in"=w1909) -> ("Handle Out"=w1906:i32, "error out"=w1905:errorcluster)  [unwired: 10 in]
        n873 = call "LJM_eWriteName.vi"("Handle In"=w1906, "Name"=w1899, "Value"=0.0, "error in"=w1905) -> ("error out"=w1903:errorcluster)  [unwired: 10 in, 1 out]
        n874 = call <vilib>:"Add State(s) to Queue__JKI_lib_State_Machine.vi"("State(s) in (\"\")"=w1913) -> ("States Out"=w1912:string)  [unwired: 14 in]
      }
      frame "LED: Green" {
        # "set LED to green"
        # "Template Separator\n(You can make a copy of, or modify, this frame)"
        n875 = Unbundle By Name(w1917) -> ("LJ Pinout.Red LED"=w1915:string, "LJ Pinout.Green LED"=w1916:string)
        n876 = call "LabJack_FGV.vi"("Operation(Read)"=enum16{"Write", "Read"}."Read" ("Operation"), "error in (no error)"=w1919) -> ("error out"=w1925:errorcluster, "Read data"=w1924:i32)  [unwired: 8 in]
        n877 = call "LJM_eWriteName.vi"("Handle In"=w1924, "Name"=w1915, "Value"=0.0, "error in"=w1925) -> ("Handle Out"=w1922:i32, "error out"=w1921:errorcluster)  [unwired: 10 in]
        n878 = call "LJM_eWriteName.vi"("Handle In"=w1922, "Name"=w1916, "Value"=9.0, "error in"=w1921) -> ("error out"=w1918:errorcluster)  [unwired: 10 in, 1 out]
        n879 = call <vilib>:"Add State(s) to Queue__JKI_lib_State_Machine.vi"("State(s) in (\"\")"=w1928) -> ("States Out"=w1927:string)  [unwired: 14 in]
      }
      frame "---------- Queue ----------" {
        # "Template Separator\n(You can make a copy of, or modify, this frame)"
        n880 = call <vilib>:"Add State(s) to Queue__JKI_lib_State_Machine.vi"("State(s) in (\"\")"=w1933) -> ("States Out"=w1932:string)  [unwired: 14 in]
      }
      frame "Queue: Flash" {
        # "Clear queue contnet\n(clear queue content by flash it)"
        n881 = Flush Queue(queue=w1940, error in (no error)=w1934) -> (error out=w1938:errorcluster)  [unwired: 2 out]
        n882 = Flush Queue(queue=w1941, error in (no error)=w1934) -> (error out=w1937:errorcluster)  [unwired: 2 out]
        n883 = Flush Queue(queue=w1939, error in (no error)=w1934) -> (error out=w1936:errorcluster)  [unwired: 2 out]
        n884 = Merge Errors(w1938, w1937, w1936) -> (w1935:errorcluster)
        n885 = call <vilib>:"Add State(s) to Queue__JKI_lib_State_Machine.vi"("State(s) in (\"\")"=w1945) -> ("States Out"=w1944:string)  [unwired: 14 in]
      }
      frame "Queue: Destory" {
        # "Destory Data Queue\nDistory data queue ref so the aquisition loop stop"
        n886 = Release Queue(queue=w1951, error in (no error)=w1947) -> (error out=w1954:errorcluster)  [unwired: 1 in, 2 out]
        n887 = Release Queue(queue=w1950, error in (no error)=w1947) -> (error out=w1953:errorcluster)  [unwired: 1 in, 2 out]
        n888 = Release Queue(queue=w1948, error in (no error)=w1947) -> (error out=w1946:errorcluster)  [unwired: 1 in, 2 out]
        n889 = Merge Errors(w1954, w1953, w1946) -> (w1952:errorcluster)
        n890 = call <vilib>:"Simple Error Handler.vi"("error in (no error)"=w1952) -> ()  [unwired: 4 in, 5 out]
        n891 = call <vilib>:"Add State(s) to Queue__JKI_lib_State_Machine.vi"("State(s) in (\"\")"=w1957) -> ("States Out"=w1956:string)  [unwired: 14 in]
      }
      frame "---------- Run ----------" {
        # "Template Separator\n(You can make a copy of, or modify, this frame)"
        n892 = call <vilib>:"Add State(s) to Queue__JKI_lib_State_Machine.vi"("State(s) in (\"\")"=w1962) -> ("States Out"=w1961:string)  [unwired: 14 in]
      }
      frame "Run: CaliIncrement" {
        # "Increment Calibration #\n(You can make a copy of, or modify, this frame)"
        n893 = Unbundle By Name(w1964) -> ("IDs.Cali ID"=w1966:i8)
        n894 = Increment(x=w1966) -> (x+1=w1963:i8)
        n895 = Bundle By Name(cluster=w1964, "IDs.Cali ID"=w1963) -> (w1965:T27)
        n896 = call <vilib>:"Add State(s) to Queue__JKI_lib_State_Machine.vi"("State(s) in (\"\")"=w1970) -> ("States Out"=w1969:string)  [unwired: 14 in]
      }
      frame "Run: BGIncrement" {
        # "Increment BG #\n(You can make a copy of, or modify, this frame)"
        n897 = Unbundle By Name(w1971) -> ("IDs.BG ID"=w1974:i8)
        n898 = Increment(x=w1974) -> (x+1=w1973:i8)
        n899 = Bundle By Name(cluster=w1971, "IDs.BG ID"=w1973) -> (w1972:T27)
        n900 = call <vilib>:"Add State(s) to Queue__JKI_lib_State_Machine.vi"("State(s) in (\"\")"=w1978) -> ("States Out"=w1977:string)  [unwired: 14 in]
      }
      frame "Run: Increment" {
        # "Increase Run# by 1"
        n901 = Unbundle By Name(w1983) -> ("IDs.RunID"=w1985:i8)
        n902 = Increment(x=w1985) -> (x+1=w1981:i8)
        n903 = Bundle By Name(cluster=w1983, "IDs.RunID"=w1981) -> (w1984:T27)
        n904 = call "RunIDFGV.vi"("Error In"=w1979, "RunID in"=w1981) -> ("Error Out"=w1980:errorcluster)  [unwired: 8 in, 1 out]
        n905 = call <vilib>:"Add State(s) to Queue__JKI_lib_State_Machine.vi"("State(s) in (\"\")"=w1987) -> ("States Out"=w1986:string)  [unwired: 14 in]
      }
      frame "Run: Decrement" {
        # "Increase Run# by 1"
        n906 = Unbundle By Name(w1992) -> ("IDs.RunID"=w1994:i8)
        n907 = Decrement(x=w1994) -> (x-1=w1990:i8)
        n908 = Bundle By Name(cluster=w1992, "IDs.RunID"=w1990) -> (w1993:T27)
        n909 = call "RunIDFGV.vi"("Error In"=w1988, "RunID in"=w1990) -> ("Error Out"=w1989:errorcluster)  [unwired: 8 in, 1 out]
        n910 = call <vilib>:"Add State(s) to Queue__JKI_lib_State_Machine.vi"("State(s) in (\"\")"=w1996) -> ("States Out"=w1995:string)  [unwired: 14 in]
      }
      frame "---------- SysConfig ----------" {
        # "Template Separator\n(You can make a copy of, or modify, this frame)"
        n911 = call <vilib>:"Add State(s) to Queue__JKI_lib_State_Machine.vi"("State(s) in (\"\")"=w2001) -> ("States Out"=w2000:string)  [unwired: 14 in]
      }
      frame "SysConfig: LoadAPDSerialNumber" {
        # "Template Separator\n(You can make a copy of, or modify, this frame)"
        n912 = call "readAPDSerial.vi"("Error In"=w2003) -> ("Error Out"=w2002:errorcluster, "output cluster"=w2004:T30)  [unwired: 9 in]
        n913 = Bundle By Name(cluster=w2005, "APDSerialNum"=w2004) -> (w2006:T27)
        n914 = call <vilib>:"Add State(s) to Queue__JKI_lib_State_Machine.vi"("State(s) in (\"\")"=w2009) -> ("States Out"=w2008:string)  [unwired: 14 in]
      }
      frame "SysConfig: Load Sys Config" {
        # "[Covers: REQ5]"
        # "Load System config"
        # "Load system configuration\n(Load both hardware and DAQ config)"
        n915 = call "LoadSysConfig.vi"("Error In"=w2012, "Enum"=enum16{"LastUse", "Default"}."LastUse") -> ("Error Out"=w2011:errorcluster, "SysConfigCluster"=w2014:T5)  [unwired: 8 in]
        "SysConfigCluster" <- w2014
        n916 = Bundle By Name(cluster=w2015, "SysConfigCluster"=w2014) -> (w2016:T27)
        n917 = call <vilib>:"Add State(s) to Queue__JKI_lib_State_Machine.vi"("State(s) in (\"\")"=w2018) -> ("States Out"=w2017:string)  [unwired: 14 in]
      }
      frame "SysConfig: Load Digitizer Setting" {
        w2019 = enum16{"Write", "Read"}."Write" ("Operation")
        # "Load DAQ config\nSave to FGV"
        # "Template Separator\n(You can make a copy of, or modify, this frame)"
        n918 = call <userlib>:"Current VIs Parent Directory__ogtk.vi"() -> ("Parent Directory (+ Relative)"=w2033:path)  [unwired: 5 in]
        n919 = Build Path(base path=w2033, name or relative path="SubVI\\DigitizerConfiguration\\V6_Scope_last_use.config") -> (appended path=w2034:path)
        n920 = call "ReadDigitizerConfig(SubVI).vi"("error in (no error)"=w2031, "appended path"=w2034) -> ("error out"=w2027:errorcluster, "FLImDAQ"=w2025:T7)  [unwired: 8 in]
        n921 = call "FLImDAQ_FGV.vi"("error in (no error)"=w2027, "Operation (Read)"=w2019, "Write data"=w2025) -> ("error out"=w2029:errorcluster)  [unwired: 7 in, 1 out]
        n922 = Unbundle By Name(w2025) -> ("min record length"=→"data length":i32, "Digitizer 1"=w2021:refnum<k15>, "Digitizer 2"=w2028:refnum<k15>)
        n923 = Bundle By Name(cluster=w2023, "FLImDAQ"=w2025) -> (w2024:T27)
        n924 = call "Digitizer1_FGV.vi"("error in (no error)"=w2029, "Operation (Read)"=w2019, "Write data"=w2021) -> ("error out"=w2030:errorcluster)  [unwired: 7 in, 1 out]
        n925 = call "Digitizer2_FGV.vi"("error in (no error)"=w2030, "Operation (Read)"=w2019, "Write data"=w2028) -> ("error out"=w2026:errorcluster)  [unwired: 7 in, 1 out]
        n926 = call <vilib>:"Add State(s) to Queue__JKI_lib_State_Machine.vi"("State(s) in (\"\")"=w2036) -> ("States Out"=w2035:string)  [unwired: 14 in]
      }
      frame "SysConfig: Load LJ Pinout" {
        # "Template Separator\n(You can make a copy of, or modify, this frame)"
        n927 = call <userlib>:"Current VIs Parent Directory__ogtk.vi"() -> ("Parent Directory (+ Relative)"=w2051:path)  [unwired: 5 in]
        n928 = Build Path(base path=w2051, name or relative path="SubVI\\LabJack\\LJ_pin_setting.config") -> (appended path=w2049:path)
        n929 = call "ReadLabjackConfig(SubVI).vi"("error in (no error)"=w2047, "appended path"=w2049) -> ("error out"=w2048:errorcluster, "Utility"=w2045:T6)  [unwired: 8 in]
        n930 = Unbundle By Name(w2045) -> ("Ch1 Bias"=w2044:string, "Ch2 Bias"=w2043:string, "Ch3 Bias"=w2042:string, "Ch4 Bias"=w2037:string, "Red LED"=w2039:string, "Green LED"=w2038:string)
        n931 = global write "GlobalVariables.vi" "LED Green pin"(w2038) -> ()
        n932 = global write "GlobalVariables.vi" "Ch1 LJ pin"(w2044) -> ()
        n933 = global write "GlobalVariables.vi" "Ch2 LJ pin"(w2043) -> ()
        n934 = global write "GlobalVariables.vi" "Ch3 LJ pin"(w2042) -> ()
        n935 = global write "GlobalVariables.vi" "Ch4 LJ pin"(w2037) -> ()
        n936 = global write "GlobalVariables.vi" "LED Red pin"(w2039) -> ()
        n937 = Bundle By Name(cluster=w2040, "LJ Pinout"=w2045) -> (w2046:T27)
        n938 = call <vilib>:"Add State(s) to Queue__JKI_lib_State_Machine.vi"("State(s) in (\"\")"=w2053) -> ("States Out"=w2052:string)  [unwired: 14 in]
      }
      frame "SysConfig: Load 355 PWM" {
        # "Template Separator\n(You can make a copy of, or modify, this frame)"
        n939 = call <userlib>:"Current VIs Parent Directory__ogtk.vi"() -> ("Parent Directory (+ Relative)"=w2071:path)  [unwired: 5 in]
        n940 = Build Path(base path=w2071, name or relative path="SubVI\\LabJack\\PWM_setting_355.config") -> (appended path=w2069:path)
        n941 = call "ReadPWMConfig(SubVI).vi"("error in (no error)"=w2066, "appended path"=w2069) -> ("error out"=w2067:errorcluster, "PWM Setting"=w2065:T44)  [unwired: 8 in]
        n942 = Unbundle By Name(w2065) -> ("DIO_EF_CLOCK1_DIVISOR"=w2062:i16, "DIO_EF_CLOCK1_ROLL_VALUE"=w2061:i32)
        n943 = Multiply(x=w2062, y=w2061) -> (x*y=w2063:i32)
        n944 = Bundle By Name(cluster=w2068, "355 PWM setting"=w2065) -> (w2055:T27)
        n945 = Divide(x=80000000.0, y=w2063) -> (x/y=w2060:dbl)
        "Laser Rep Rate" <- w2060
        n946 = Number To Decimal String(number=w2060) -> (decimal integer string=w2059:string)  [unwired: 1 in]
        n947 = Concatenate Strings("355nm " ("string"), w2059, "Hz" ("string")) -> (w2057:string)
        n948 = property on="355nm Laser toggle" class="Bool (strict)"("Caption.Text"=w2057) -> ()  [unwired: 2 in, 2 out]
        n949 = call <vilib>:"Add State(s) to Queue__JKI_lib_State_Machine.vi"("State(s) in (\"\")"=w2073) -> ("States Out"=w2072:string)  [unwired: 14 in]
      }
      frame "SysConfig: Load AB PWM" {
        # "Template Separator\n(You can make a copy of, or modify, this frame)"
        n950 = call <userlib>:"Current VIs Parent Directory__ogtk.vi"() -> ("Parent Directory (+ Relative)"=w2082:path)  [unwired: 5 in]
        n951 = Build Path(base path=w2082, name or relative path="SubVI\\LabJack\\PWM_setting_AB.config") -> (appended path=w2080:path)
        n952 = call "ReadPWMConfig(SubVI).vi"("error in (no error)"=w2077, "appended path"=w2080) -> ("error out"=w2078:errorcluster, "PWM Setting"=w2076:T44)  [unwired: 8 in]
        n953 = Bundle By Name(cluster=w2074, "AB PWM setting"=w2076) -> (w2079:T27)
        n954 = call <vilib>:"Add State(s) to Queue__JKI_lib_State_Machine.vi"("State(s) in (\"\")"=w2084) -> ("States Out"=w2083:string)  [unwired: 14 in]
      }
      frame "SysConfig: Load AB setting" {
        # "load aming beam setting\n(check frequency, if 0 do nothing, if not zero, config PWM)"
        n955 = call "readAimingBeamSetting.vi"("error in (no error)"=w2102) -> ("error out"=w2097:errorcluster, "Aiming Beam Setting"=w2089:T45)  [unwired: 9 in]
        n956 = Unbundle By Name(w2089) -> ("Default Current"=w2088:dbl)
        n957 = Unbundle By Name(w2089) -> ("Frequency(Hz)"=w2085:u32)
        n958 = Equal To 0?(x=w2085) -> (x = 0?=w2095:bool)
        n959 = Select(t="", s=w2095, f="SysConfig: Load AB PWM" ("State(s) in Front (\"\")")) -> (s? t:f=w2098:string)
        n960 = Number To Decimal String(number=w2085) -> (decimal integer string=w2094:string)  [unwired: 1 in]
        n961 = Number To Decimal String(number=w2088, width (-)=i16 2) -> (decimal integer string=w2087:string)
        n962 = Concatenate Strings("445nm " ("string"), w2094, "Hz " ("string"), w2087, "mA" ("string")) -> (w2093:string)
        n963 = property on="Aiming beam toggle" class="Bool (strict)"("Caption.Text"=w2093) -> ()  [unwired: 2 in, 2 out]
        n964 = case shown="False" w2095 {
          tunnel: w2097 -> [w2110 w2113]
          tunnel: [w2109 w2113] -> w2096
          tunnel: w2085 -> [w2108 _]
          frame False {
            n965 = call "LJ_calculate_PWM_parameters.vi"("Duty Cycle (%)"=u32 10, "Error In"=w2110, "Show Confirmation"=FALSE, "Laser Rep Rate (Hz)"=w2108, "Laser"=enum16{"355nm", "AimingBeam"}."AimingBeam") -> ("Error Out"=w2109:errorcluster)  [unwired: 5 in, 1 out]
          }
          frame True {
          }
        }
        n966 = Bundle By Name(cluster=w2103, "AB Cluster"=w2089) -> (w2104:T27)
        n967 = call <vilib>:"Add State(s) to Queue__JKI_lib_State_Machine.vi"("State(s) in Front (\"\")"=w2098, "State(s) in (\"\")"=w2106) -> ("States Out"=w2105:string)  [unwired: 13 in]
      }
      frame "SysConfig: LoadABVideoSetting" {
        # "Load AB video setting form ini file\n()"
        n968 = call "readVideoConfig.vi"("error in (no error)"=w2117) -> ("error out"=w2118:errorcluster, "Aiming Beam Config"=w2116:T26)  [unwired: 8 in, 1 out]
        n969 = Bundle By Name(cluster=w2114, "VideoConfig"=w2116) -> (w2115:T27)
        n970 = call <vilib>:"Add State(s) to Queue__JKI_lib_State_Machine.vi"("State(s) in (\"\")"=w2121) -> ("States Out"=w2120:string)  [unwired: 14 in]
      }
      frame "SysConfig: LoadCursorLocation" {
        # "Load cursor location from ini file\n(load cursor from system setting ini file)"
        n971 = call "readCursorConfigMain.vi"("error in (no error)"=w2133) -> ("error out"=w2134:errorcluster, "Cursor Locations"=w2132:T46)  [unwired: 9 in]
        n972 = Unbundle By Name(w2132) -> ("DC1"=w2131:i32, "DC2"=w2130:i32, "BG1"=w2125:i32, "BG2"=w2124:i32)
        n973 = Build Array(w2131, w2130) -> (w2129:i32[])
        n974 = Build Array(w2125, w2124) -> (w2126:i32[])
        n975 = Array Max & Min(array=w2129) -> (max value=w2128:i32, min value=w2127:i32)  [unwired: 2 out]
        n976 = Array Max & Min(array=w2126) -> (max value=w2123:i32, min value=w2122:i32)  [unwired: 2 out]
        n977 = global write "GlobalVariables.vi" "DC Idx2"(w2128) -> ()
        n978 = global write "GlobalVariables.vi" "DC Idx1"(w2127) -> ()
        n979 = global write "GlobalVariables.vi" "BG Idx2"(w2123) -> ()
        n980 = global write "GlobalVariables.vi" "BG Idx1"(w2122) -> ()
        n981 = call <vilib>:"Add State(s) to Queue__JKI_lib_State_Machine.vi"("State(s) in (\"\")"=w2138) -> ("States Out"=w2137:string)  [unwired: 14 in]
      }
      frame "---------- SystemStatus ----------" {
        # "Template Separator\n(You can make a copy of, or modify, this frame)"
        n982 = call <vilib>:"Add State(s) to Queue__JKI_lib_State_Machine.vi"("State(s) in (\"\")"=w2143) -> ("States Out"=w2142:string)  [unwired: 14 in]
      }
      frame "SystemStatus: SlowSysStatusMacro" {
        # "store system check time"
        # "Template Separator\n(You can make a copy of, or modify, this frame)"
        n983 = Tick Count (ms)() -> (millisecond timer value=w2146:u32)
        n984 = Bundle By Name(cluster=w2144, "SlowTimer"=w2146) -> (w2145:T27)
        n985 = call <vilib>:"Add State(s) to Queue__JKI_lib_State_Machine.vi"("State(s) in Front (\"\")"="Digitizer: checkTemp\n/*TCP: CheckConnection" ("State(s) in Front (\"\")"), "State(s) in (\"\")"=w2151) -> ("States Out"=w2150:string)  [unwired: 13 in]
      }
      frame "SystemStatus: FastSysStatusMacro" {
        # "store system check time"
        # "Template Separator\n(You can make a copy of, or modify, this frame)"
        n986 = Tick Count (ms)() -> (millisecond timer value=w2154:u32)
        n987 = Bundle By Name(cluster=w2152, "FastTimer"=w2154) -> (w2153:T27)
        n988 = call <vilib>:"Add State(s) to Queue__JKI_lib_State_Machine.vi"("State(s) in Front (\"\")"="355 Laser: CheckPWMStatus\nAimingBeam: GetPWMStatus\n/*355 Laser: CheckControllerStatus" ("State(s) in Front (\"\")"), "State(s) in (\"\")"=w2159) -> ("States Out"=w2158:string)  [unwired: 13 in]
      }
      frame "---------- UI ----------" {
        # "Do not put any code in this frame.\n(It is a separator no-op. You can make a copy of this frame to create a new UI frame)"
        n989 = call <vilib>:"Add State(s) to Queue__JKI_lib_State_Machine.vi"("State(s) in (\"\")"=w2164) -> ("States Out"=w2163:string)  [unwired: 14 in]
      }
      frame "UI: Initialize" {
        w2166 = T47 {"Minimum"=0.0, "Maximum"=4.6, "Increment"=0.1} ("Data Entry Limits")
        w2165 = T12."Disabled and Grayed Out" ("Disabled")
        # "Disable all button on startup"
        # "Initialize the User Interface, here.\n(this is called automatically, by the Macro: Init)"
        n990 = property on="V 1" class="DigNum (strict)"("DisabledEnum"=w2165) -> ()  [unwired: 2 in, 2 out]
        n991 = property on="V 2" class="DigNum (strict)"("DisabledEnum"=w2165) -> ()  [unwired: 2 in, 2 out]
        n992 = property on="StopButton" class="Bool (strict)"("DisabledEnum"=w2165) -> ()  [unwired: 2 in, 2 out]
        n993 = property on="Sys Reconfig" class="Bool"("DisabledEnum"=w2165) -> ()  [unwired: 2 in, 2 out]
        n994 = property on="StartButton" class="Bool (strict)"("DisabledEnum"=w2165) -> ()  [unwired: 2 in, 2 out]
        n995 = property on="355nm Laser toggle" class="Bool (strict)"("DisabledEnum"=w2165) -> ()  [unwired: 2 in, 2 out]
        n996 = property on="Aiming beam toggle" class="Bool (strict)"("DisabledEnum"=w2165) -> ()  [unwired: 2 in, 2 out]
        n997 = property on="Background" class="Bool (strict)"("DisabledEnum"=w2165) -> ()  [unwired: 2 in, 2 out]
        n998 = property on="Cali&iRF alignment" class="Bool (strict)"("DisabledEnum"=w2165) -> ()  [unwired: 2 in, 2 out]
        n999 = property on="V 3" class="DigNum (strict)"("DisabledEnum"=w2165) -> ()  [unwired: 2 in, 2 out]
        n1000 = property on="Video Source" class="RadioBtnsControl (strict)"("DisabledEnum"=w2165) -> ()  [unwired: 2 in, 2 out]
        n1001 = property on="V 1" class="DigNum (strict)"("Data Range"=w2166) -> ()  [unwired: 2 in, 2 out]
        n1002 = property on="V 2" class="DigNum (strict)"("Data Range"=w2166) -> ()  [unwired: 2 in, 2 out]
        n1003 = property on="V 3" class="DigNum (strict)"("Data Range"=w2166) -> ()  [unwired: 2 in, 2 out]
        n1004 = call <vilib>:"Add State(s) to Queue__JKI_lib_State_Machine.vi"("State(s) in Front (\"\")"="UI: CaliAndiRFNotReady" ("State(s) in Front (\"\")"), "State(s) in (\"\")"=w2172) -> ("States Out"=w2171:string)  [unwired: 13 in]
      }
      frame "UI: BGLoaded" {
        # "[Covers: REQ24]"
        # "Do not put any code in this frame.\n(It is a separator no-op. You can make a copy of this frame to create a new UI frame)"
        n1005 = property on="Background" class="Bool (strict)"("BoolText.Text"="Loaded!" ("Boolean Text.Text"), "Colors [4]"=cluster{u32, u32}[] [{15764023, 15764023}, {16711680, 16711680}]) -> ()  [unwired: 2 in, 2 out]
        n1006 = call <vilib>:"Add State(s) to Queue__JKI_lib_State_Machine.vi"("State(s) in (\"\")"=w2179) -> ("States Out"=w2178:string)  [unwired: 14 in]
      }
      frame "UI: BGSizeError" {
        # "[Covers: REQ24]"
        # "Do not put any code in this frame.\n(It is a separator no-op. You can make a copy of this frame to create a new UI frame)"
        n1007 = property on="Background" class="Bool (strict)"("BoolText.Text"="Loaded!" ("Boolean Text.Text"), "Colors [4]"=cluster{u32, u32}[] [{7171459, 7171459}, {16711680, 16711680}]) -> ()  [unwired: 2 in, 2 out]
        n1008 = One Button Dialog(message="Background waveform length and current digitizer setting mismatch! Please take a new background before any aquisition!") -> ()  [unwired: 1 in, 1 out]
        n1009 = call <vilib>:"Add State(s) to Queue__JKI_lib_State_Machine.vi"("State(s) in (\"\")"=w2187) -> ("States Out"=w2186:string)  [unwired: 14 in]
      }
      frame "UI: CaliAndiRFLoaded" {
        # "[Covers: REQ24]"
        # "Do not put any code in this frame.\n(It is a separator no-op. You can make a copy of this frame to create a new UI frame)"
        n1010 = property on="Cali&iRF alignment" class="Bool (strict)"("BoolText.Text"="Loaded!" ("Boolean Text.Text"), "Colors [4]"=cluster{u32, u32}[] [{15764023, 15764023}, {16711680, 16711680}]) -> ()  [unwired: 2 in, 2 out]
        n1011 = call <vilib>:"Add State(s) to Queue__JKI_lib_State_Machine.vi"("State(s) in (\"\")"=w2194) -> ("States Out"=w2193:string)  [unwired: 14 in]
      }
      frame "UI: WFAutoScale" {
        # "Set graph auto scale.\n(UI: WFAutoScale >> T/F)"
        n1012 = Equal?(x=w2195, y="F") -> (x = y?=w2196:bool)
        n1013 = Equal?(x=w2195, y="T") -> (x = y?=w2198:bool)
        n1014 = case shown="True" w2198 {
          frame False {
          }
          frame True {
            w2214 = u8 2 ("Y Scale.Scale Fit")
            n1015 = property on="Channel 1" class="WFGraph (strict)"("YScale.ScaleFit"=w2214) -> ()  [unwired: 2 in, 2 out]
            n1016 = property on="Channel 2" class="WFGraph (strict)"("YScale.ScaleFit"=w2214) -> ()  [unwired: 2 in, 2 out]
            n1017 = property on="Channel 3" class="WFGraph (strict)"("YScale.ScaleFit"=w2214) -> ()  [unwired: 2 in, 2 out]
          }
        }
        n1018 = case shown="True" w2196 {
          frame False {
          }
          frame True {
            w2211 = 0.0 ("Y Scale.Range:Maximum")
            w2212 = 2.0 ("Y Scale.Range:Maximum")
            w2213 = u8 0 ("Y Scale.Scale Fit")
            n1019 = property on="Channel 1" class="WFGraph (strict)"("YScale.ScaleFit"=w2213) -> (error out=w2210:errorcluster)  [unwired: 2 in, 1 out]
            n1020 = property on="Channel 2" class="WFGraph (strict)"("YScale.ScaleFit"=w2213) -> (error out=w2209:errorcluster)  [unwired: 2 in, 1 out]
            n1021 = property on="Channel 3" class="WFGraph (strict)"("YScale.ScaleFit"=w2213) -> (error out=w2208:errorcluster)  [unwired: 2 in, 1 out]
            n1022 = property on="Channel 1" class="WFGraph (strict)"(error in=w2210, "YScale.Maximum"=w2212) -> (error out=w2207:errorcluster)  [unwired: 1 in, 1 out]
            n1023 = property on="Channel 2" class="WFGraph (strict)"(error in=w2209, "YScale.Maximum"=w2212) -> (error out=w2206:errorcluster)  [unwired: 1 in, 1 out]
            n1024 = property on="Channel 3" class="WFGraph (strict)"(error in=w2208, "YScale.Maximum"=w2212) -> (error out=w2205:errorcluster)  [unwired: 1 in, 1 out]
            n1025 = property on="Channel 1" class="WFGraph (strict)"(error in=w2207, "YScale.Minimum"=w2211) -> ()  [unwired: 1 in, 2 out]
            n1026 = property on="Channel 2" class="WFGraph (strict)"(error in=w2206, "YScale.Minimum"=w2211) -> ()  [unwired: 1 in, 2 out]
            n1027 = property on="Channel 3" class="WFGraph (strict)"(error in=w2205, "YScale.Minimum"=w2211) -> ()  [unwired: 1 in, 2 out]
          }
        }
        n1028 = call <vilib>:"Add State(s) to Queue__JKI_lib_State_Machine.vi"("State(s) in (\"\")"=w2204) -> ("States Out"=w2203:string)  [unwired: 14 in]
      }
      frame "UI: showDisclaimer" {
        # "Show disclamer window.\n(It is a separator no-op. You can make a copy of this frame to create a new UI frame)"
        n1029 = call <vilib>:"Application Directory.vi"() -> ("Application Directory"=w2227:path)
        n1030 = Build Path(base path=w2227, name or relative path="Disclamer.png") -> (appended path=w2225:path)
        n1031 = property on="Disclamer" class="Pict"() -> ("Draw Area Size"=w2223:T48)  [unwired: 2 in, 2 out]
        n1032 = disable-structure "Diagram Disable Structure" shown="Disabled" {
          frame Disabled {
            n1033 = flat-sequence {
              frame #0 {
                n1034 = call "disclaimer.vi"() -> ()  [unwired: 12 in]
              }
              frame #1 {
                n1035 = Wait (ms)(milliseconds to wait=u32 250) -> ()  [unwired: 1 out]
              }
              frame #2 {
                n1036 = call "SoftwareNote.vi"() -> ()  [unwired: 12 in]
              }
            }
          }
          frame Enabled {
          }
        }
        n1037 = call <vilib>:"Read PNG File.vi"("path to PNG file"=w2225) -> ("image data"=w2222:T49)  [unwired: 8 in, 2 out]
        n1038 = Unbundle By Name(w2222) -> ("Rectangle.right"=w2220:i16, "Rectangle.bottom"=w2218:i16)
        n1039 = Unbundle By Name(w2223) -> ("Width"=w2221:u32, "Height"=w2219:u32)
        n1040 = call <vilib>:"Draw Flattened Pixmap.vi"("image data"=w2222) -> ("new picture"=→"Disclamer":picture)  [unwired: 8 in]
        n1041 = Divide(x=w2221, y=w2220) -> (x/y=w2217:dbl)
        n1042 = Divide(x=w2219, y=w2218) -> (x/y=w2216:dbl)
        n1043 = Max & Min(x=w2217, y=w2216) -> (min(x,y)=w2215:dbl)  [unwired: 1 out]
        n1044 = property on="Disclamer" class="Pict"("ZoomFactor"=w2215) -> ()  [unwired: 2 in, 2 out]
        n1045 = call <vilib>:"Add State(s) to Queue__JKI_lib_State_Machine.vi"("State(s) in (\"\")"=w2232) -> ("States Out"=w2231:string)  [unwired: 14 in]
      }
      frame "UI: CaliAndiRFNotReady" {
        # "Do not put any code in this frame.\n(It is a separator no-op. You can make a copy of this frame to create a new UI frame)"
        n1046 = property on="Cali&iRF alignment" class="Bool (strict)"("BoolText.Text"="No Info" ("Boolean Text.Text"), "Colors [4]"=cluster{u32, u32}[] [{13816530, 13816530}, {16711680, 16711680}]) -> ()  [unwired: 2 in, 2 out]
        n1047 = call <vilib>:"Add State(s) to Queue__JKI_lib_State_Machine.vi"("State(s) in (\"\")"=w2240) -> ("States Out"=w2239:string)  [unwired: 14 in]
      }
      frame "UI: BGnotReady" {
        # "Do not put any code in this frame.\n(It is a separator no-op. You can make a copy of this frame to create a new UI frame)"
        n1048 = property on="Background" class="Bool (strict)"("BoolText.Text"="No Info" ("Boolean Text.Text"), "Colors [4]"=cluster{u32, u32}[] [{13816530, 13816530}, {16711680, 16711680}]) -> ()  [unwired: 2 in, 2 out]
        n1049 = call <vilib>:"Add State(s) to Queue__JKI_lib_State_Machine.vi"("State(s) in (\"\")"=w2247) -> ("States Out"=w2246:string)  [unwired: 14 in]
      }
      frame "UI: Reset" {
        w2249 = cluster{u32, u32}[] [{13816530, 13816530}, {13816530, 13816530}] ("Colors [4]")
        # "Do not put any code in this frame.\n(It is a separator no-op. You can make a copy of this frame to create a new UI frame)"
        n1050 = property on="Cali&iRF alignment" class="Bool (strict)"("BoolText.Text"="No Info" ("Boolean Text.Text"), "Colors [4]"=w2249) -> ()  [unwired: 2 in, 2 out]
        n1051 = property on="Background" class="Bool (strict)"("BoolText.Text"="No Info" ("Boolean Text.Text"), "Colors [4]"=w2249) -> ()  [unwired: 2 in, 2 out]
        n1052 = call <vilib>:"Add State(s) to Queue__JKI_lib_State_Machine.vi"("State(s) in (\"\")"=w2255) -> ("States Out"=w2254:string)  [unwired: 14 in]
      }
      frame "UI: SetButtonText" {
        # "Set button text of 355nm laser and aiming beam."
        n1053 = call <vilib>:"Add State(s) to Queue__JKI_lib_State_Machine.vi"("State(s) in (\"\")"=w2260) -> ("States Out"=w2259:string)  [unwired: 14 in]
      }
      frame "UI: DuringAquisition" {
        w2263 = T12."Disabled and Grayed Out" ("Disabled")
        # "Do not put any code in this frame.\n(It is a separator no-op. You can make a copy of this frame to create a new UI frame)"
        n1054 = Unbundle By Name(w2262) -> ("bothVidSourceAvail"=w2261:bool)
        n1055 = case shown="True" w2261 {
          tunnel: w2263 -> [_ w2269]
          frame False {
          }
          frame True {
            n1056 = property on="Video Source" class="RadioBtnsControl (strict)"("DisabledEnum"=w2269) -> ()  [unwired: 2 in, 2 out]
          }
        }
        n1057 = property on="StartButton" class="Bool (strict)"("DisabledEnum"=w2263) -> ()  [unwired: 2 in, 2 out]
        n1058 = property on="Sys Reconfig" class="Bool"("DisabledEnum"=w2263) -> ()  [unwired: 2 in, 2 out]
        n1059 = property on="355nm Laser toggle" class="Bool (strict)"("DisabledEnum"=w2263) -> ()  [unwired: 2 in, 2 out]
        n1060 = property on="Aiming beam toggle" class="Bool (strict)"("DisabledEnum"=w2263) -> ()  [unwired: 2 in, 2 out]
        n1061 = property on="Background" class="Bool (strict)"("DisabledEnum"=w2263) -> ()  [unwired: 2 in, 2 out]
        n1062 = property on="Radio Buttons" class="RadioBtnsControl (strict)"("DisabledEnum"=w2263) -> ()  [unwired: 2 in, 2 out]
        n1063 = property on="Cali&iRF alignment" class="Bool (strict)"("DisabledEnum"=w2263) -> ()  [unwired: 2 in, 2 out]
        n1064 = property on="Quit" class="Bool"("DisabledEnum"=w2263) -> ()  [unwired: 2 in, 2 out]
        n1065 = property on="Skip Data Save?" class="Bool (strict)"("DisabledEnum"=w2263) -> ()  [unwired: 2 in, 2 out]
        n1066 = property on="Video Display" class="Bool (strict)"("DisabledEnum"=w2263) -> ()  [unwired: 2 in, 2 out]
        n1067 = property on="StopButton" class="Bool (strict)"("DisabledEnum"=T12."Enabled" ("Disabled")) -> ()  [unwired: 2 in, 2 out]
        n1068 = call <vilib>:"Add State(s) to Queue__JKI_lib_State_Machine.vi"("State(s) in (\"\")"=w2268) -> ("States Out"=w2267:string)  [unwired: 14 in]
      }
      frame "UI: duringIRFAlign" {
        w2270 = T12."Disabled and Grayed Out" ("Disabled")
        # "Set UI to during iRF alignment\n(It is a separator no-op. You can make a copy of this frame to create a new UI frame)"
        n1069 = property on="StartButton" class="Bool (strict)"("DisabledEnum"=w2270) -> ()  [unwired: 2 in, 2 out]
        n1070 = property on="Sys Reconfig" class="Bool"("DisabledEnum"=w2270) -> ()  [unwired: 2 in, 2 out]
        n1071 = property on="355nm Laser toggle" class="Bool (strict)"("DisabledEnum"=w2270) -> ()  [unwired: 2 in, 2 out]
        n1072 = property on="Aiming beam toggle" class="Bool (strict)"("DisabledEnum"=w2270) -> ()  [unwired: 2 in, 2 out]
        n1073 = property on="Background" class="Bool (strict)"("DisabledEnum"=w2270) -> ()  [unwired: 2 in, 2 out]
        n1074 = property on="StopButton" class="Bool (strict)"("DisabledEnum"=w2270) -> ()  [unwired: 2 in, 2 out]
        n1075 = call <vilib>:"Add State(s) to Queue__JKI_lib_State_Machine.vi"("State(s) in (\"\")"=w2275) -> ("States Out"=w2274:string)  [unwired: 14 in]
      }
      frame "UI: duringBGAcquire" {
        w2276 = T12."Disabled and Grayed Out" ("Disabled")
        # "Do not put any code in this frame.\n(It is a separator no-op. You can make a copy of this frame to create a new UI frame)"
        n1076 = property on="StartButton" class="Bool (strict)"("DisabledEnum"=w2276) -> ()  [unwired: 2 in, 2 out]
        n1077 = property on="StopButton" class="Bool (strict)"("DisabledEnum"=w2276) -> ()  [unwired: 2 in, 2 out]
        n1078 = property on="Sys Reconfig" class="Bool"("DisabledEnum"=w2276) -> ()  [unwired: 2 in, 2 out]
        n1079 = property on="355nm Laser toggle" class="Bool (strict)"("DisabledEnum"=w2276) -> ()  [unwired: 2 in, 2 out]
        n1080 = property on="Aiming beam toggle" class="Bool (strict)"("DisabledEnum"=w2276) -> ()  [unwired: 2 in, 2 out]
        n1081 = property on="Cali&iRF alignment" class="Bool (strict)"("DisabledEnum"=w2276) -> ()  [unwired: 2 in, 2 out]
        n1082 = call <vilib>:"Add State(s) to Queue__JKI_lib_State_Machine.vi"("State(s) in (\"\")"=w2281) -> ("States Out"=w2280:string)  [unwired: 14 in]
      }
      frame "UI: ReadyForAquisition" {
        w2285 = T12."Enabled" ("Disabled")
        # "Do not put any code in this frame.\n(It is a separator no-op. You can make a copy of this frame to create a new UI frame)"
        n1083 = Unbundle By Name(w2284) -> ("System Status.TCP/IP"=w2283:bool, "bothVidSourceAvail"=w2282:bool)
        n1084 = property on="StartButton" class="Bool (strict)"("DisabledEnum"=w2285) -> ()  [unwired: 2 in, 2 out]
        n1085 = property on="Sys Reconfig" class="Bool"("DisabledEnum"=w2285) -> ()  [unwired: 2 in, 2 out]
        n1086 = property on="355nm Laser toggle" class="Bool (strict)"("DisabledEnum"=w2285) -> ()  [unwired: 2 in, 2 out]
        n1087 = property on="Aiming beam toggle" class="Bool (strict)"("DisabledEnum"=w2285) -> ()  [unwired: 2 in, 2 out]
        n1088 = property on="Cali&iRF alignment" class="Bool (strict)"("DisabledEnum"=w2285) -> ()  [unwired: 2 in, 2 out]
        n1089 = property on="Background" class="Bool (strict)"("DisabledEnum"=w2285) -> ()  [unwired: 2 in, 2 out]
        n1090 = property on="Quit" class="Bool"("DisabledEnum"=w2285) -> ()  [unwired: 2 in, 2 out]
        n1091 = property on="Radio Buttons" class="RadioBtnsControl (strict)"("DisabledEnum"=w2285) -> ()  [unwired: 2 in, 2 out]
        n1092 = case shown="True" w2282 {
          tunnel: w2285 -> [_ w2291]
          frame False {
          }
          frame True {
            n1093 = property on="Video Source" class="RadioBtnsControl (strict)"("DisabledEnum"=w2291) -> ()  [unwired: 2 in, 2 out]
          }
        }
        n1094 = property on="Skip Data Save?" class="Bool (strict)"("DisabledEnum"=w2285) -> ()  [unwired: 2 in, 2 out]
        n1095 = case shown="True" w2283 {
          tunnel: w2285 -> [_ w2292]
          frame False {
          }
          frame True {
            n1096 = property on="Video Display" class="Bool (strict)"("DisabledEnum"=w2292) -> ()  [unwired: 2 in, 2 out]
          }
        }
        n1097 = property on="StopButton" class="Bool (strict)"("DisabledEnum"=T12."Disabled and Grayed Out" ("Disabled")) -> ()  [unwired: 2 in, 2 out]
        n1098 = call <vilib>:"Add State(s) to Queue__JKI_lib_State_Machine.vi"("State(s) in (\"\")"=w2290) -> ("States Out"=w2289:string)  [unwired: 14 in]
      }
      frame "UI: Update" {
        # "Do not put any code in this frame.\n(It is a separator no-op. You can make a copy of this frame to create a new UI frame)"
        n1099 = Unbundle By Name(w2303) -> ("System Status"=→"System Hardware Connection Status":T3, "IDs.RunID"=→"Run #":i8, "CaseID"=→"Case #":string, "FLImDAQ"=→"FLImDAQ":T34, "SysRunning?"=→"Aquisition Status:":bool, "LJ Pinout"=→"LJ Pinout":T6, "IDs.BG ID"=→"BG #":i8, "IDs.Cali ID"=→"Calibration #":i8, "video source"=→"Visualization PC video source":T2)
        n1100 = call <vilib>:"Add State(s) to Queue__JKI_lib_State_Machine.vi"("State(s) in (\"\")"=w2306) -> ("States Out"=w2305:string)  [unwired: 14 in]
      }
      frame "UI: updateVideoToggle" {
        # "Set video toggle based on visualization PC video source.\n(take )"
        n1101 = call <vilib>:"Add State(s) to Queue__JKI_lib_State_Machine.vi"("State(s) in (\"\")"=w2311) -> ("States Out"=w2310:string)  [unwired: 14 in]
      }
      frame "UI: Cursor Set" {
        # "Argument"
        # "Set and Unset Cursor Busy.\n(Usage: \"UI: Cursor Set >> Busy|Idle\")"
        n1102 = case shown="\"Idle\", Default" w2313 {
          tunnel: w2315 -> [w2320 w2322]
          tunnel: [w2319 w2321] -> w2314
          frame "Idle", Default {
            n1103 = call <vilib>:"Unset Busy.vi"("error in (no error)"=w2320) -> ("error out"=w2319:errorcluster)  [unwired: 10 in]
          }
          frame "Busy" {
            n1104 = call <vilib>:"Set Busy.vi"("error in (no error)"=w2322) -> ("error out"=w2321:errorcluster)  [unwired: 9 in, 1 out]
          }
        }
        n1105 = call <vilib>:"Add State(s) to Queue__JKI_lib_State_Machine.vi"("State(s) in (\"\")"=w2318) -> ("States Out"=w2317:string)  [unwired: 14 in]
      }
      frame "UI: Front Panel State" {
        # "Argument"
        # "Set Front Panel Open or Closed\n(Usage: \"UI: Front Panel State >> Open|Close\")"
        n1106 = Unbundle By Name(w2326) -> ("Core.Current VI Reference"=w2325:refnum<vi>)
        n1107 = case shown="\"Open\", \"Standard\", Default" w2324 {
          tunnel: w2328 -> [w2336 w2351 w2362 w2375 w2388]
          tunnel: [w2338 w2352 w2364 w2377 w2390] -> w2327
          tunnel: w2325 -> [w2337 w2349 w2363 w2376 w2389]
          frame "Open", "Standard", Default {
            w2331 = T18."Standard" ("State")
            n1108 = property on="Property Node" class="VI"(reference=w2337, error in=w2336) -> (reference out=w2334:refnum<vi>, error out=w2335:errorcluster, "FP.State"=w2333:T18)
            n1109 = Not Equal?(x=w2333, y=w2331) -> (x != y?=w2332:bool)
            n1110 = case shown="True" w2332 {
              tunnel: [w2342 w2344] -> w2338
              tunnel: w2335 -> [w2341 w2344]
              tunnel: w2334 -> [w2340 _]
              tunnel: w2331 -> [w2339 _]
              frame True {
                n1111 = invoke on="Invoke Node" class="VI" method="FP.Open"(reference=w2340, error in=w2341, "Activate"=TRUE, "State"=w2339) -> (error out=w2342:errorcluster)  [unwired: 1 in, 4 out]
              }
              frame False {
              }
            }
          }
          frame "Close", "Closed" {
            n1112 = property on="Property Node" class="VI"(reference=w2349, error in=w2351) -> (reference out=w2348:refnum<vi>, error out=w2350:errorcluster, "FP.State"=w2346:T18)
            n1113 = Not Equal?(x=w2346, y=T18."Closed" ("Front Panel Window:State")) -> (x != y?=w2345:bool)
            n1114 = case shown="True" w2345 {
              tunnel: [w2353 w2356] -> w2352
              tunnel: w2350 -> [w2353 w2355]
              tunnel: w2348 -> [_ w2354]
              frame False {
              }
              frame True {
                n1115 = invoke on="Invoke Node" class="VI" method="FP.Close"(reference=w2354, error in=w2355) -> (error out=w2356:errorcluster)  [unwired: 1 in, 2 out]
              }
            }
          }
          frame "Hidden", "Hide" {
            w2357 = T18."Hidden" ("State")
            n1116 = property on="Property Node" class="VI"(reference=w2363, error in=w2362) -> (reference out=w2360:refnum<vi>, error out=w2361:errorcluster, "FP.State"=w2359:T18)
            n1117 = Not Equal?(x=w2359, y=w2357) -> (x != y?=w2358:bool)
            n1118 = case shown="True" w2358 {
              tunnel: [w2368 w2369] -> w2364
              tunnel: w2361 -> [w2367 w2369]
              tunnel: w2360 -> [w2366 _]
              tunnel: w2357 -> [w2365 _]
              frame True {
                n1119 = invoke on="Invoke Node" class="VI" method="FP.Open"(reference=w2366, error in=w2367, "State"=w2365) -> (error out=w2368:errorcluster)  [unwired: 2 in, 4 out]
              }
              frame False {
              }
            }
          }
          frame "Minimize", "Minimized" {
            w2370 = T18."Minimized" ("State")
            n1120 = property on="Property Node" class="VI"(reference=w2376, error in=w2375) -> (reference out=w2373:refnum<vi>, error out=w2374:errorcluster, "FP.State"=w2372:T18)
            n1121 = Not Equal?(x=w2372, y=w2370) -> (x != y?=w2371:bool)
            n1122 = case shown="True" w2371 {
              tunnel: [w2381 w2382] -> w2377
              tunnel: w2374 -> [w2380 w2382]
              tunnel: w2373 -> [w2379 _]
              tunnel: w2370 -> [w2378 _]
              frame True {
                n1123 = invoke on="Invoke Node" class="VI" method="FP.Open"(reference=w2379, error in=w2380, "State"=w2378) -> (error out=w2381:errorcluster)  [unwired: 2 in, 4 out]
              }
              frame False {
              }
            }
          }
          frame "Maximize", "Maximized" {
            w2383 = T18."Maximized" ("State")
            n1124 = property on="Property Node" class="VI"(reference=w2389, error in=w2388) -> (reference out=w2386:refnum<vi>, error out=w2387:errorcluster, "FP.State"=w2385:T18)
            n1125 = Not Equal?(x=w2385, y=w2383) -> (x != y?=w2384:bool)
            n1126 = case shown="True" w2384 {
              tunnel: [w2394 w2395] -> w2390
              tunnel: w2387 -> [w2393 w2395]
              tunnel: w2386 -> [w2392 _]
              tunnel: w2383 -> [w2391 _]
              frame True {
                n1127 = invoke on="Invoke Node" class="VI" method="FP.Open"(reference=w2392, error in=w2393, "State"=w2391) -> (error out=w2394:errorcluster)  [unwired: 2 in, 4 out]
              }
              frame False {
              }
            }
          }
        }
        n1128 = call <vilib>:"Add State(s) to Queue__JKI_lib_State_Machine.vi"("State(s) in (\"\")"=w2330) -> ("States Out"=w2329:string)  [unwired: 14 in]
      }
      frame "---------- AimingBeam ----------" {
        # "Template Separator\n(You can make a copy of, or modify, this frame)"
        n1129 = call <vilib>:"Add State(s) to Queue__JKI_lib_State_Machine.vi"("State(s) in (\"\")"=w2400) -> ("States Out"=w2399:string)  [unwired: 14 in]
      }
      frame "AimingBeam: Initialize" {
        # "set aiming beam button color"
        # "Open COM port for Aiming Beam\n(Require USB connection)"
        n1130 = Unbundle By Name(w2402) -> ("AB Cluster.Aiming Beam COM Port"=w2410:refnum<visa-resource-name>)
        n1131 = call-poly "VISA Configure Serial Port"("VISA resource name"=w2410, "Enable Termination\nChar (T)"=TRUE ("Enable Termination\nChar (T)"), "baud rate (9600)"=u32 9600, "error in (no error)"=w2407) -> ("error out"=w2406:errorcluster)  [unwired: 10 in, 1 out]
        n1132 = Unbundle By Name(w2406) -> ("status"=w2405:bool)
        n1133 = Not(x=w2405) -> (.not. x?=w2404:bool)
        n1134 = Bundle By Name(cluster=w2402, "System Status.Aiming Beam"=w2404) -> (w2403:T27)
        n1135 = call <vilib>:"Add State(s) to Queue__JKI_lib_State_Machine.vi"("State(s) in (\"\")"=w2412) -> ("States Out"=w2411:string)  [unwired: 14 in]
      }
      frame "AimingBeam: Close" {
        # "Close Aiming Beam COM port\n(Require USB connection to Aiming Beam Laser)"
        n1136 = Unbundle By Name(w2415) -> ("AB Cluster.Aiming Beam COM Port"=w2419:refnum<visa-resource-name>)
        n1137 = VISA Close(VISA resource name=w2419, error in (no error)=w2417) -> (error out=w2418:errorcluster)
        n1138 = Bundle By Name(cluster=w2415, "System Status.Aiming Beam"=FALSE) -> (w2416:T27)
        n1139 = call <vilib>:"Add State(s) to Queue__JKI_lib_State_Machine.vi"("State(s) in (\"\")"=w2421) -> ("States Out"=w2420:string)  [unwired: 14 in]
      }
      frame "AimingBeam: Set Current" {
        # "Set Aiming Beam Current\n(You can make a copy of, or modify, this frame)"
        n1140 = Unbundle By Name(w2436) -> ("AB Cluster.Aiming Beam COM Port"=w2429:refnum<visa-resource-name>, "AB Cluster.Max Current"=w2425:dbl, "AB Cluster.Default Current"=w2427:dbl, "AB Cluster.Min Current"=w2426:dbl)
        n1141 = In Range and Coerce(upper limit=w2425, x=w2427, lower limit=w2426) -> (coerced(x)=w2422:dbl)  [unwired: 1 out]
        n1142 = Number To Fractional String(number=w2422, precision (6)=i16 2) -> (F-format string=w2430:string)  [unwired: 2 in]
        n1143 = Concatenate Strings("slc:", w2430, "\r" ("Carriage Return Constant"), "\n" ("Line Feed Constant")) -> (w2433:string)
        n1144 = VISA Write(VISA resource name=w2429, write buffer=w2433, error in (no error)=w2424) -> (error out=w2428:errorcluster)  [unwired: 2 out]
        n1145 = call <vilib>:"Add State(s) to Queue__JKI_lib_State_Machine.vi"("State(s) in (\"\")"=w2438) -> ("States Out"=w2437:string)  [unwired: 14 in]
      }
      frame "AimingBeam: Set Status" {
        # "Enable Aiming Beam\n(Usage: \"AimingBeam: Set >> Enable|Disable\")"
        n1146 = Unbundle By Name(w2445) -> ("AB Cluster.Aiming Beam COM Port"=w2442:refnum<visa-resource-name>)
        n1147 = case shown="\"Enable\"" w2444 {
          tunnel: [w2448 w2452] -> w2443
          frame "Disable", Default {
            n1148 = Concatenate Strings("cof", "\r" ("Carriage Return Constant"), "\n" ("Line Feed Constant")) -> (w2448:string)
          }
          frame "Enable" {
            n1149 = Concatenate Strings("con", "\r" ("Carriage Return Constant"), "\n" ("Line Feed Constant")) -> (w2452:string)
          }
        }
        n1150 = VISA Write(VISA resource name=w2442, write buffer=w2443, error in (no error)=w2440) -> (error out=w2441:errorcluster)  [unwired: 2 out]
        n1151 = call <vilib>:"Add State(s) to Queue__JKI_lib_State_Machine.vi"("State(s) in (\"\")"=w2447) -> ("States Out"=w2446:string)  [unwired: 14 in]
      }
      frame "AimingBeam: GetPWMStatus" {
        # "Get aiming beam PWM status\n()"
        n1152 = Unbundle By Name(w2460) -> ("AB Cluster.Freq"=w2459:i32, "LJ Pinout.AimingBeam PWM"=w2466:string)
        n1153 = Equal To 0?(x=w2459) -> (x = 0?=w2458:bool)
        n1154 = call "LabJack_FGV.vi"("Operation(Read)"=enum16{"Write", "Read"}."Read" ("Operation"), "error in (no error)"=w2462) -> ("error out"=w2464:errorcluster, "Read data"=w2465:i32)  [unwired: 8 in]
        n1155 = case shown="True" w2458 {
          tunnel: w2466 -> [w2479 _]
          tunnel: [w2477 "DIO_STATE"] -> w2463
          frame False {
            n1156 = Concatenate Strings(w2479, "_EF_ENABLE" ("string")) -> (w2477:string)
          }
          frame True {
          }
        }
        n1157 = call "LJM_eReadName.vi"("Handle In"=w2465, "Name"=w2463, "error in"=w2464) -> ("Value"=w2457:dbl, "error out"=w2461:errorcluster)  [unwired: 10 in, 1 out]
        n1158 = case shown="True" w2458 {
          tunnel: w2457 -> [w2472 w2476]
          tunnel: [w2471 w2473] -> w2456
          frame False {
            n1159 = Greater Than 0?(x=w2472) -> (x > 0?=w2471:bool)
          }
          frame True {
            n1160 = Number To Boolean Array(number=w2476) -> (Boolean array=w2475:bool[])
            n1161 = Index Array(array=w2475, index=3) -> (element=w2473:bool)
          }
        }
        n1162 = case shown="False" w2456 {
          frame False {
            # "PWM is off\nset color to dark green"
            n1163 = local write "Aiming beam toggle"(FALSE ("Aimging beam")) -> ()
          }
          frame True {
            # "PWM is on\nset color to light green"
            n1164 = local write "Aiming beam toggle"(TRUE ("Aimging beam")) -> ()
          }
        }
        n1165 = call <vilib>:"Add State(s) to Queue__JKI_lib_State_Machine.vi"("State(s) in (\"\")"=w2470) -> ("States Out"=w2469:string)  [unwired: 14 in]
      }
      frame "---------- 355 Laser ----------" {
        # "Template Separator\n(You can make a copy of, or modify, this frame)"
        n1166 = call <vilib>:"Add State(s) to Queue__JKI_lib_State_Machine.vi"("State(s) in (\"\")"=w2487) -> ("States Out"=w2486:string)  [unwired: 14 in]
      }
      frame "355 Laser: Check Dewelling" {
        # "if time laser start time is less than 7.5s before, wait 250ms then check again."
        # "Template Separator\n(You can make a copy of, or modify, this frame)"
        n1167 = Unbundle By Name(w2495) -> ("Laser start tic"=w2492:u32)
        n1168 = Tick Count (ms)() -> (millisecond timer value=w2493:u32)
        n1169 = Subtract(x=w2493, y=w2492) -> (x-y=w2491:u32)
        n1170 = Greater?(x=w2491, y=u32 5000) -> (0:w2489:bool)
        n1171 = case shown="False" w2489 {
          tunnel: ["355 Laser: Check Dewelling" ""] -> w2488
          frame False {
            n1172 = Wait (ms)(milliseconds to wait=u32 250) -> ()  [unwired: 1 out]
          }
          frame True {
          }
        }
        n1173 = call <vilib>:"Add State(s) to Queue__JKI_lib_State_Machine.vi"("State(s) in Front (\"\")"=w2488, "State(s) in (\"\")"=w2498) -> ("States Out"=w2497:string)  [unwired: 13 in]
      }
      frame "355 Laser: Laser enable" {
        # "Laser enable/disable\n(Usage: \"LabJack: Laser enable/disable >> 1|0\")"
        n1174 = Unbundle By Name(w2505) -> ("LJ Pinout.Laser Start/Stop"=w2509:string, "System Status.355 Laser"=w2503:bool)
        n1175 = case shown="False" w2503 {
          tunnel: w2502 -> [w2524 w2525]
          tunnel: w2509 -> [w2518 _]
          tunnel: [w2513 w2525] -> w2507
          tunnel: [w2512 u32 0 ("millisecond timer value")] -> w2504
          frame False {
            n1176 = call "LabJack_FGV.vi"("Operation(Read)"=enum16{"Write", "Read"}."Read" ("Operation")) -> ("Read data"=w2520:i32)  [unwired: 9 in, 1 out]
            n1177 = call "LJM_eWriteName.vi"("Handle In"=w2520, "Name"=w2518, "Value"=1.0, "error in"=w2524) -> ("Handle Out"=w2519:i32, "error out"=w2517:errorcluster)  [unwired: 10 in]
            n1178 = call <userlib>:"Wait (ms)__ogtk.vi"("error in (no error)"=w2517, "milliseconds to wait"=u32 250) -> ("error out"=w2516:errorcluster)  [unwired: 8 in, 1 out]
            n1179 = call "LJM_eWriteName.vi"("Handle In"=w2519, "Name"=w2518, "Value"=0.0, "error in"=w2516) -> ("error out"=w2514:errorcluster)  [unwired: 10 in, 1 out]
            n1180 = call <userlib>:"Tick Count (ms)__ogtk.vi"("error in (no error)"=w2514) -> ("error out"=w2513:errorcluster, "millisecond timer value"=w2512:u32)  [unwired: 9 in]
          }
          frame True {
          }
        }
        n1181 = Bundle By Name(cluster=w2505, "Laser start tic"=w2504) -> (w2506:T27)
        n1182 = call <vilib>:"Add State(s) to Queue__JKI_lib_State_Machine.vi"("State(s) in (\"\")"=w2511) -> ("States Out"=w2510:string)  [unwired: 14 in]
      }
      frame "355 Laser: Laser disable" {
        # "Laser enable/disable\n(Usage: \"LabJack: Laser enable/disable >> 1|0\")"
        n1183 = Unbundle By Name(w2529) -> ("LJ Pinout.Laser Start/Stop"=w2533:string, "System Status.355 Laser"=w2527:bool)
        n1184 = case shown="True" w2527 {
          tunnel: w2534 -> [w2537 w2551]
          tunnel: w2533 -> [_ w2545]
          tunnel: [w2537 w2540] -> w2531
          tunnel: [u32 0 ("millisecond timer value") w2539] -> w2528
          frame False {
          }
          frame True {
            n1185 = call "LabJack_FGV.vi"("Operation(Read)"=enum16{"Write", "Read"}."Read" ("Operation")) -> ("Read data"=w2547:i32)  [unwired: 9 in, 1 out]
            n1186 = call "LJM_eWriteName.vi"("Handle In"=w2547, "Name"=w2545, "Value"=1.0, "error in"=w2551) -> ("Handle Out"=w2546:i32, "error out"=w2544:errorcluster)  [unwired: 10 in]
            n1187 = call <userlib>:"Wait (ms)__ogtk.vi"("error in (no error)"=w2544, "milliseconds to wait"=u32 250) -> ("error out"=w2543:errorcluster)  [unwired: 8 in, 1 out]
            n1188 = call "LJM_eWriteName.vi"("Handle In"=w2546, "Name"=w2545, "Value"=0.0, "error in"=w2543) -> ("error out"=w2541:errorcluster)  [unwired: 10 in, 1 out]
            n1189 = call <userlib>:"Tick Count (ms)__ogtk.vi"("error in (no error)"=w2541) -> ("error out"=w2540:errorcluster, "millisecond timer value"=w2539:u32)  [unwired: 9 in]
          }
        }
        n1190 = Bundle By Name(cluster=w2529, "Laser start tic"=w2528) -> (w2530:T27)
        n1191 = call <vilib>:"Add State(s) to Queue__JKI_lib_State_Machine.vi"("State(s) in (\"\")"=w2536) -> ("States Out"=w2535:string)  [unwired: 14 in]
      }
      frame "355 Laser: Dewelling" {
        # "Wait some time (ms)\n(355 Laser: Dewelling >> #)"
        n1192 = Fract/Exp String To Number(string=w2555, default (0 dbl)=0) -> (number=w2553:i32)  [unwired: 2 in, 1 out]
        n1193 = Wait (ms)(milliseconds to wait=w2553) -> ()  [unwired: 1 out]
        n1194 = call <vilib>:"Add State(s) to Queue__JKI_lib_State_Machine.vi"("State(s) in (\"\")"=w2559) -> ("States Out"=w2558:string)  [unwired: 14 in]
      }
      frame "355 Laser: Close" {
        # "Template Separator\n(You can make a copy of, or modify, this frame)"
        n1195 = call <vilib>:"Add State(s) to Queue__JKI_lib_State_Machine.vi"("State(s) in Front (\"\")"="355 Laser: CheckControllerStatus\n355 Laser: Laser disable\n355 Laser: Dewelling >>1000", "State(s) in (\"\")"=w2565) -> ("States Out"=w2564:string)  [unwired: 13 in]
      }
      frame "355 Laser: CheckControllerStatus" {
        # "if average < 2, laser no power\nif average 2 < average < 9.3, laser on\nif 9.3<average<10, interlock open, blink indicator\nif average > 10, laser off\n[Covers: REQ30]"
        # "take 10 measuremt and look at average"
        # "Check 355 laser controller status\nBy probing Emisison Lamp negative terminal voltage"
        n1196 = Unbundle By Name(w2574) -> ("LJ Pinout.Laser Ready"=w2577:string)
        n1197 = call "LabJack_FGV.vi"("Operation(Read)"=enum16{"Write", "Read"}."Read" ("Operation")) -> ("Read data"=w2578:i32)  [unwired: 9 in, 1 out]
        n1198 = for {
          N: 20 -> [_]
          tunnel: w2578 -> [w2589]
          tunnel: w2577 -> [w2588]
          shift-right: [w2587] -> w2570
          shift-left: w2576 -> [w2586]
          tunnel: [w2584] -> w2569 mode=indexing
          n1199 = call "LJM_eReadName.vi"("Handle In"=w2589, "Name"=w2588, "error in"=w2586) -> ("Value"=w2584:dbl, "error out"=w2587:errorcluster)  [unwired: 10 in, 1 out]
          n1200 = Wait (ms)(milliseconds to wait=u32 25) -> ()  [unwired: 1 out]
        }
        n1201 = call "checkLaserStatus.vi"("error in (no error)"=w2570, "Laser LED voltage"=w2569) -> ("error out"=w2571:errorcluster, "Interlock open?"=w2566:bool, "Laser on?"=w2568:bool, "Mean voltage"=→"laser EM lamp V":dbl)  [unwired: 6 in]
        n1202 = Bundle By Name(cluster=w2574, "System Status.355 Laser"=w2568) -> (w2575:T27)
        n1203 = case shown="True" w2566 {
          frame False {
            n1204 = property on="355 Laser" class="Bool (strict)"("Blinking"=FALSE) -> ()  [unwired: 2 in, 2 out]
          }
          frame True {
            n1205 = property on="355 Laser" class="Bool (strict)"("Blinking"=TRUE) -> ()  [unwired: 2 in, 2 out]
          }
        }
        n1206 = call <vilib>:"Add State(s) to Queue__JKI_lib_State_Machine.vi"("State(s) in (\"\")"=w2581) -> ("States Out"=w2580:string)  [unwired: 14 in]
      }
      frame "355 Laser: CheckPWMStatus" {
        # "Check 355 laser PWM status\n(Read LJ DIO#EF_ENABLE register to determine PWM status)"
        n1207 = Unbundle By Name(w2599) -> ("LJ Pinout.355 PWM"=w2598:string)
        n1208 = call "LabJack_FGV.vi"("Operation(Read)"=enum16{"Write", "Read"}."Read" ("Operation"), "error in (no error)"=w2592) -> ("error out"=w2595:errorcluster, "Read data"=w2596:i32)  [unwired: 8 in]
        n1209 = Concatenate Strings(w2598, "_EF_ENABLE" ("string")) -> (w2594:string)
        n1210 = call "LJM_eReadName.vi"("Handle In"=w2596, "Name"=w2594, "error in"=w2595) -> ("Value"=w2591:dbl, "error out"=w2593:errorcluster)  [unwired: 10 in, 1 out]
        n1211 = Greater Than 0?(x=w2591) -> (x > 0?=w2590:bool)
        n1212 = case shown="False" w2590 {
          frame False {
            # "PWM is off\nset color to gray"
            n1213 = local write "355nm Laser toggle"(FALSE ("355nm Laser")) -> ()
          }
          frame True {
            # "PWM is on\nset color to light green"
            n1214 = local write "355nm Laser toggle"(TRUE ("355nm Laser")) -> ()
          }
        }
        n1215 = call <vilib>:"Add State(s) to Queue__JKI_lib_State_Machine.vi"("State(s) in (\"\")"=w2603) -> ("States Out"=w2602:string)  [unwired: 14 in]
      }
      frame "355 Laser: Start" {
        # "Template Separator\n(You can make a copy of, or modify, this frame)"
        n1216 = call <vilib>:"Add State(s) to Queue__JKI_lib_State_Machine.vi"("State(s) in Front (\"\")"="LabJack: 355_PWM_Start", "State(s) in (\"\")"=w2611) -> ("States Out"=w2610:string)  [unwired: 13 in]
      }
      frame "355 Laser: Stop" {
        # "Template Separator\n(You can make a copy of, or modify, this frame)"
        n1217 = call <vilib>:"Add State(s) to Queue__JKI_lib_State_Machine.vi"("State(s) in Front (\"\")"="LabJack: 355_PWM_Stop", "State(s) in (\"\")"=w2617) -> ("States Out"=w2616:string)  [unwired: 13 in]
      }
      frame "---------- Utility ----------" {
        # "Template Separator\n(You can make a copy of, or modify, this frame)"
        n1218 = call <vilib>:"Add State(s) to Queue__JKI_lib_State_Machine.vi"("State(s) in (\"\")"=w2622) -> ("States Out"=w2621:string)  [unwired: 14 in]
      }
      frame "Utility: SetDataClass" {
        # "Set Data Class in Queues\n(Set data class to either Data, Bg or Cali)"
        n1219 = case shown="\"Cali\"" w2624 {
          tunnel: [enum16{"Data", "BG", "Cali"}."Data" ("Data Class") enum16{"Data", "BG", "Cali"}."BG" ("Data Class") enum16{"Data", "BG", "Cali"}."Cali" ("Data Class")] -> w2623
          frame "Data", Default {
          }
          frame "Bg" {
          }
          frame "Cali" {
          }
        }
        n1220 = local write "Data Class"(w2623) -> ()
        n1221 = call <vilib>:"Add State(s) to Queue__JKI_lib_State_Machine.vi"("State(s) in (\"\")"=w2629) -> ("States Out"=w2628:string)  [unwired: 14 in]
      }
      frame "Utility: AquiTimerReset" {
        # "Set Aquisition Timer\n(You can make a copy of, or modify, this frame)"
        n1222 = Tick Count (ms)() -> (millisecond timer value=w2635:u32)
        n1223 = Bundle By Name(cluster=w2633, "Aquisition Timer"=w2635) -> (w2634:T27)
        n1224 = call <vilib>:"Add State(s) to Queue__JKI_lib_State_Machine.vi"("State(s) in (\"\")"=w2639) -> ("States Out"=w2638:string)  [unwired: 14 in]
      }
      frame "Utility: AquiTimerCheck" {
        # "5min to ms"
        # "Set Aquisition Timer\n([Covers: REQ35])"
        n1225 = Unbundle By Name(w2647) -> ("Aquisition Timer"=w2645:u32)
        n1226 = Tick Count (ms)() -> (millisecond timer value=w2646:u32)
        n1227 = Subtract(x=w2646, y=w2645) -> (x-y=w2644:u32)
        n1228 = Multiply(x=1000, y=300) -> (x*y=w2641:i32)
        n1229 = Greater Or Equal?(x=w2644, y=w2641) -> (x >= y?=w2640:bool)
        n1230 = case shown="True" w2640 {
          frame False {
            # "do nothing"
          }
          frame True {
            # "if timed out, stop aquisition"
            n1231 = property on="StopButton" class="Bool (strict)"("Val(Sgnl)"=TRUE ("Value (Signaling)")) -> ()  [unwired: 2 in, 2 out]
          }
        }
        n1232 = call <vilib>:"Add State(s) to Queue__JKI_lib_State_Machine.vi"("State(s) in (\"\")"=w2651) -> ("States Out"=w2650:string)  [unwired: 14 in]
      }
      frame "Utility: StartBeep" {
        # "Beep\n([Covers: REQ18])"
        n1233 = call <vilib>:"Beep.vi"("use system alert? (T)"=FALSE, "duration (msec)"=u32 1000, "frequency (Hz)"=u32 2000) -> ()  [unwired: 9 in]
        n1234 = call <vilib>:"Add State(s) to Queue__JKI_lib_State_Machine.vi"("State(s) in (\"\")"=w2660) -> ("States Out"=w2659:string)  [unwired: 14 in]
      }
      frame "Utility: EndBeep" {
        # "Beep\n([Covers: REQ18])"
        n1235 = flat-sequence {
          frame #0 {
            n1236 = call <vilib>:"Beep.vi"("use system alert? (T)"=FALSE, "duration (msec)"=u32 500, "frequency (Hz)"=u32 2000) -> ()  [unwired: 9 in]
          }
          frame #1 {
            n1237 = call <vilib>:"Beep.vi"("use system alert? (T)"=FALSE, "duration (msec)"=u32 500, "frequency (Hz)"=u32 2000) -> ()  [unwired: 9 in]
          }
        }
        n1238 = call <vilib>:"Add State(s) to Queue__JKI_lib_State_Machine.vi"("State(s) in (\"\")"=w2665) -> ("States Out"=w2664:string)  [unwired: 14 in]
      }
      frame "Utility: RestoreDeConChan" {
        # "Template Separator\n(You can make a copy of, or modify, this frame)"
        n1239 = global read "GlobalVariables.vi" "DeconChan Temp"() -> (w2672:T10)
        n1240 = local write "Radio Buttons"(w2672) -> ()
        n1241 = call <vilib>:"Add State(s) to Queue__JKI_lib_State_Machine.vi"("State(s) in (\"\")"=w2677) -> ("States Out"=w2676:string)  [unwired: 14 in]
      }
      frame "Utility: SaveDeconChan" {
        # "Save Decon Channel to global temp\n(You can make a copy of, or modify, this frame)"
        n1242 = flat-sequence {
          frame #0 {
            n1243 = local read "Radio Buttons"() -> (w2683:T10)
            n1244 = global write "GlobalVariables.vi" "DeconChan Temp"(w2683) -> ()
          }
          frame #1 {
            n1245 = local write "Radio Buttons"(T10."No Selection" ("Radio Buttons")) -> ()
          }
        }
        n1246 = flat-sequence {
          frame #0 {
          }
          frame #1 {
            (unwired) enum32{"No Selection", "Ch1", "Ch2", "Ch3"}."No Selection" ("Radio Buttons")
          }
        }
        n1247 = call <vilib>:"Add State(s) to Queue__JKI_lib_State_Machine.vi"("State(s) in (\"\")"=w2682) -> ("States Out"=w2681:string)  [unwired: 14 in]
      }
      frame "Utility: Dewelling" {
        # "Main loop dewell\n(Dewelling >> #)"
        n1248 = Fract/Exp String To Number(string=w2688, default (0 dbl)=0) -> (number=w2686:i32)  [unwired: 2 in, 1 out]
        n1249 = Wait (ms)(milliseconds to wait=w2686) -> ()  [unwired: 1 out]
        n1250 = call <vilib>:"Add State(s) to Queue__JKI_lib_State_Machine.vi"("State(s) in (\"\")"=w2692) -> ("States Out"=w2691:string)  [unwired: 14 in]
      }
      frame "Utility: SetAllChanManualGain" {
        w2693 = FALSE ("Value (Signaling)")
        # "Set all channel to manual gain\n(You can make a copy of, or modify, this frame)"
        n1251 = property on="Auto gain ch1" class="Bool (strict)"("Val(Sgnl)"=w2693) -> ()  [unwired: 2 in, 2 out]
        n1252 = property on="Auto gain ch2" class="Bool (strict)"("Val(Sgnl)"=w2693) -> ()  [unwired: 2 in, 2 out]
        n1253 = property on="Auto gain ch3" class="Bool (strict)"("Val(Sgnl)"=w2693) -> ()  [unwired: 2 in, 2 out]
        n1254 = property on="Auto gain ch4" class="Bool (strict)"("Val(Sgnl)"=w2693) -> ()  [unwired: 2 in, 2 out]
        n1255 = call <vilib>:"Add State(s) to Queue__JKI_lib_State_Machine.vi"("State(s) in (\"\")"=w2698) -> ("States Out"=w2697:string)  [unwired: 14 in]
      }
      frame "Utility: SetAllChanAutoGain" {
        w2699 = TRUE ("Value (Signaling)")
        # "Set all channels to auto gain\n(You can make a copy of, or modify, this frame)"
        n1256 = property on="Auto gain ch1" class="Bool (strict)"("Val(Sgnl)"=w2699) -> ()  [unwired: 2 in, 2 out]
        n1257 = property on="Auto gain ch2" class="Bool (strict)"("Val(Sgnl)"=w2699) -> ()  [unwired: 2 in, 2 out]
        n1258 = property on="Auto gain ch3" class="Bool (strict)"("Val(Sgnl)"=w2699) -> ()  [unwired: 2 in, 2 out]
        n1259 = property on="Auto gain ch4" class="Bool (strict)"("Val(Sgnl)"=w2699) -> ()  [unwired: 2 in, 2 out]
        n1260 = call <vilib>:"Add State(s) to Queue__JKI_lib_State_Machine.vi"("State(s) in (\"\")"=w2704) -> ("States Out"=w2703:string)  [unwired: 14 in]
      }
      frame "---------- SysLog ----------" {
        # "Template Separator\n(You can make a copy of, or modify, this frame)"
        n1261 = call <vilib>:"Add State(s) to Queue__JKI_lib_State_Machine.vi"("State(s) in (\"\")"=w2709) -> ("States Out"=w2708:string)  [unwired: 14 in]
      }
      frame "SysLog: OpenLogFile" {
        # "Template Separator\n(You can make a copy of, or modify, this frame)"
        n1262 = call <vilib>:"Add State(s) to Queue__JKI_lib_State_Machine.vi"("State(s) in (\"\")"=w2714) -> ("States Out"=w2713:string)  [unwired: 14 in]
      }
      frame "---------- Graph ----------" {
        # "Template Separator\n(You can make a copy of, or modify, this frame)"
        n1263 = call <vilib>:"Add State(s) to Queue__JKI_lib_State_Machine.vi"("State(s) in (\"\")"=w2719) -> ("States Out"=w2718:string)  [unwired: 14 in]
      }
      frame "Graph: SetXMultiplier" {
        # "Set X multiplier of WF graphs\n(You can make a copy of, or modify, this frame)"
        n1264 = call "Digitizer1_FGV.vi"() -> ("error out"=w2723:errorcluster, "Read data"=w2724:refnum<k15>)  [unwired: 10 in]
        n1265 = property class="niScope"(reference=w2724, error in=w2723) -> ("Min Sample Rate"=w2722:dbl)  [unwired: 2 out]
        n1266 = Divide(x=1.0, y=w2722) -> (x/y=w2720:dbl)
        n1267 = property on="Channel 1" class="WFGraph (strict)"("XScale.Multiplier"=w2720) -> ()  [unwired: 2 in, 2 out]
        n1268 = property on="Channel 2" class="WFGraph (strict)"("XScale.Multiplier"=w2720) -> ()  [unwired: 2 in, 2 out]
        n1269 = property on="Channel 3" class="WFGraph (strict)"("XScale.Multiplier"=w2720) -> ()  [unwired: 2 in, 2 out]
        n1270 = property on="Channel 4" class="WFGraph (strict)"("XScale.Multiplier"=w2720) -> ()  [unwired: 2 in, 2 out]
        n1271 = call <vilib>:"Add State(s) to Queue__JKI_lib_State_Machine.vi"("State(s) in (\"\")"=w2729) -> ("States Out"=w2728:string)  [unwired: 14 in]
      }
      frame "Graph: AddCursors" {
        # "Add BG and DC cursor to all graphs\n(You can make a copy of, or modify, this frame)"
        n1272 = property on="Channel 1" class="WFGraph (strict)"() -> ("XScale.Multiplier"=w2738:dbl)  [unwired: 2 in, 2 out]
        n1273 = global read "GlobalVariables.vi" "DC Idx1"() -> (w2737:i32)
        n1274 = global read "GlobalVariables.vi" "DC Idx2"() -> (w2736:i32)
        n1275 = global read "GlobalVariables.vi" "BG Idx1"() -> (w2735:i32)
        n1276 = global read "GlobalVariables.vi" "BG Idx2"() -> (w2734:i32)
        n1277 = property on="Channel 1" class="WFGraph (strict)"(error in=w2740) -> ("CrsrList"=w2749:T28)  [unwired: 1 in, 2 out]
        n1278 = property on="Channel 2" class="WFGraph (strict)"() -> ("CrsrList"=w2746:T28)  [unwired: 2 in, 2 out]
        n1279 = property on="Channel 3" class="WFGraph (strict)"() -> ("CrsrList"=w2745:T28)  [unwired: 2 in, 2 out]
        n1280 = property on="Channel 4" class="WFGraph (strict)"() -> ("CrsrList"=w2731:T28)  [unwired: 2 in, 2 out]
        n1281 = Build Array(w2737, w2736, w2735, w2734) -> (w2733:i32[])
        n1282 = Multiply(x=w2733, y=w2738) -> (x*y=w2732:dbl[])
        n1283 = for {
          tunnel: w2749 -> [w2763] mode=indexing
          tunnel: w2732 -> [w2756] mode=indexing
          tunnel: [w2762] -> w2748 mode=indexing
          tunnel: u32[] [6618880, 6618880, 16711680, 16711680] -> [w2755] mode=indexing
          tunnel: w2746 -> [w2761] mode=indexing
          tunnel: w2745 -> [w2760] mode=indexing
          tunnel: [w2759] -> w2744 mode=indexing
          tunnel: [w2758] -> w2743 mode=indexing
          tunnel: w2731 -> [w2757] mode=indexing
          tunnel: [w2754] -> w2730 mode=indexing
          n1284 = Bundle By Name(cluster=w2763, "Position.X"=w2756, "Color"=w2755) -> (w2762:T29)
          n1285 = Bundle By Name(cluster=w2761, "Position.X"=w2756, "Color"=w2755) -> (w2759:T29)
          n1286 = Bundle By Name(cluster=w2760, "Position.X"=w2756, "Color"=w2755) -> (w2758:T29)
          n1287 = Bundle By Name(cluster=w2757, "Position.X"=w2756, "Color"=w2755) -> (w2754:T29)
        }
        n1288 = property on="Channel 1" class="WFGraph (strict)"("CrsrList"=w2748) -> (error out=w2739:errorcluster)  [unwired: 2 in, 1 out]
        n1289 = property on="Channel 2" class="WFGraph (strict)"("CrsrList"=w2744) -> ()  [unwired: 2 in, 2 out]
        n1290 = property on="Channel 3" class="WFGraph (strict)"("CrsrList"=w2743) -> ()  [unwired: 2 in, 2 out]
        n1291 = property on="Channel 4" class="WFGraph (strict)"("CrsrList"=w2730) -> ()  [unwired: 2 in, 2 out]
        n1292 = control-ref of="Channel 1"() -> (w2742:refnum<vi>)
        n1293 = call <vilib>:"Add State(s) to Queue__JKI_lib_State_Machine.vi"("State(s) in (\"\")"=w2753) -> ("States Out"=w2752:string)  [unwired: 14 in]
        n1294 = call "UpdateCurserIdx(SubVI).vi"("error in (no error)"=w2739, "WaveformGraph in"=w2742) -> ("error out"=w2741:errorcluster)  [unwired: 9 in]
      }
      frame "Graph: SaveCursorLoc" {
        # "Save cursor location to ini file\n(Save cursor location to system setting ini file)"
        n1295 = global read "GlobalVariables.vi" "DC Idx1"() -> (w2770:i32)
        n1296 = global read "GlobalVariables.vi" "DC Idx2"() -> (w2769:i32)
        n1297 = global read "GlobalVariables.vi" "BG Idx1"() -> (w2768:i32)
        n1298 = global read "GlobalVariables.vi" "BG Idx2"() -> (w2767:i32)
        n1299 = Bundle("DC Idx1"=w2770, "DC Idx2"=w2769, "BG Idx1"=w2768, "BG Idx2"=w2767) -> (w2766:T50)  [unwired: 1 in]
        n1300 = call "writeCursorConfigMain.vi"("error in (no error)"=w2764, "Cursor Locations"=w2766) -> ("error out"=w2765:errorcluster)  [unwired: 9 in]
        n1301 = call <vilib>:"Add State(s) to Queue__JKI_lib_State_Machine.vi"("State(s) in (\"\")"=w2774) -> ("States Out"=w2773:string)  [unwired: 14 in]
      }
      frame "---------- APD ----------" {
        # "Template Separator\n(You can make a copy of, or modify, this frame)"
        n1302 = call <vilib>:"Add State(s) to Queue__JKI_lib_State_Machine.vi"("State(s) in (\"\")"=w2779) -> ("States Out"=w2778:string)  [unwired: 14 in]
      }
      frame "APD: Initialize" {
        w2786 = enum16{"Read", "Write"}."Write" ("Operation (Read)")
        w2785 = refnum<class "APDClass.lvclass"> refnum  # APDClass.lvclass
        # "Initialize APD FGV\n(Initialized APD FGV for holding data)"
        n1303 = call "APD1FGV.vi"("Error In"=w2780, "Operation (Read)"=w2786, "APDClass in"=w2785) -> ("Error Out"=w2784:errorcluster)  [unwired: 7 in, 1 out]
        n1304 = call "APD2FGV.vi"("Error In"=w2780, "Operation (Read)"=w2786, "APDClass in"=w2785) -> ("Error Out"=w2783:errorcluster)  [unwired: 7 in, 1 out]
        n1305 = call "APD3FGV.vi"("Error In"=w2780, "Operation (Read)"=w2786, "APDClass in"=w2785) -> ("Error Out"=w2782:errorcluster)  [unwired: 7 in, 1 out]
        n1306 = Merge Errors(w2784, w2783, w2782) -> (w2781:errorcluster)
        n1307 = call <vilib>:"Add State(s) to Queue__JKI_lib_State_Machine.vi"("State(s) in (\"\")"=w2790) -> ("States Out"=w2789:string)  [unwired: 14 in]
      }
      frame "APD: LoadFromSerial" {
        w2792 = enum16{"Read", "Write"}."Write" ("Operation (Read)")
        # "Load APD data from tdms file\n(load and update FGV)"
        n1308 = call "readAPDSerial.vi"("Error In"=w2799) -> ("Error Out"=w2795:errorcluster, "output cluster"=w2798:T30)  [unwired: 9 in]
        n1309 = Unbundle By Name(w2798) -> ("Ch1APDSerial#"=w2811:string, "Ch2APDSerial#"=w2797:string, "Ch3APDSerial#"=w2810:string, "Ch4APDSerial#"=w2796:string)
        n1310 = call "CreatFromSerialNumNoRaw.vi"("error in (no error)"=w2795, "APD Serial #"=w2811) -> ("error out"=w2808:errorcluster, "APDClass out"=w2809:refnum<class "APDClass.lvclass">)  [unwired: 8 in]
        n1311 = call "CreatFromSerialNumNoRaw.vi"("error in (no error)"=w2795, "APD Serial #"=w2797) -> ("error out"=w2806:errorcluster, "APDClass out"=w2807:refnum<class "APDClass.lvclass">)  [unwired: 8 in]
        n1312 = call "CreatFromSerialNumNoRaw.vi"("error in (no error)"=w2795, "APD Serial #"=w2810) -> ("error out"=w2804:errorcluster, "APDClass out"=w2805:refnum<class "APDClass.lvclass">)  [unwired: 8 in]
        n1313 = call "CreatFromSerialNumNoRaw.vi"("error in (no error)"=w2795, "APD Serial #"=w2796) -> ("error out"=w2793:errorcluster, "APDClass out"=w2794:refnum<class "APDClass.lvclass">)  [unwired: 8 in]
        n1314 = call "APD1FGV.vi"("Error In"=w2808, "Operation (Read)"=w2792, "APDClass in"=w2809) -> ("Error Out"=w2803:errorcluster)  [unwired: 7 in, 1 out]
        n1315 = call "APD2FGV.vi"("Error In"=w2806, "Operation (Read)"=w2792, "APDClass in"=w2807) -> ("Error Out"=w2801:errorcluster)  [unwired: 7 in, 1 out]
        n1316 = call "APD3FGV.vi"("Error In"=w2804, "Operation (Read)"=w2792, "APDClass in"=w2805) -> ("Error Out"=w2802:errorcluster)  [unwired: 7 in, 1 out]
        n1317 = call "APD4FGV.vi"("Error In"=w2793, "Operation (Read)"=w2792, "APDClass in"=w2794) -> ("Error Out"=w2791:errorcluster)  [unwired: 7 in, 1 out]
        n1318 = Merge Errors(w2803, w2801, w2802, w2791) -> (w2800:errorcluster)
        n1319 = call <vilib>:"Add State(s) to Queue__JKI_lib_State_Machine.vi"("State(s) in (\"\")"=w2815) -> ("States Out"=w2814:string)  [unwired: 14 in]
      }
      frame "APD: UpdateCtrlVLimit" {
        w2821 = enum16{"Read", "Write"}."Read" ("Operation (Read)")
        # "Set V limit\n(You can make a copy of, or modify, this frame)"
        n1320 = call "APD1FGV.vi"("Error In"=w2822, "Operation (Read)"=w2821) -> ("Error Out"=w2837:errorcluster, "APDClass out"=w2838:refnum<class "APDClass.lvclass">)  [unwired: 8 in]
        n1321 = call "APD2FGV.vi"("Error In"=w2822, "Operation (Read)"=w2821) -> ("Error Out"=w2835:errorcluster, "APDClass out"=w2836:refnum<class "APDClass.lvclass">)  [unwired: 8 in]
        n1322 = call "APD3FGV.vi"("Error In"=w2822, "Operation (Read)"=w2821) -> ("Error Out"=w2833:errorcluster, "APDClass out"=w2834:refnum<class "APDClass.lvclass">)  [unwired: 8 in]
        n1323 = call "APD4FGV.vi"("Error In"=w2822, "Operation (Read)"=w2821) -> ("Error Out"=w2819:errorcluster, "APDClass out"=w2820:refnum<class "APDClass.lvclass">)  [unwired: 8 in]
        n1324 = call-dynamic "ReadMaxCtrlV.vi"("error in (no error)"=w2837, "APDClass in"=w2838) -> ("error out"=w2828:errorcluster, "Numeric"=w2831:dbl)  [unwired: 7 in, 1 out]
        n1325 = call-dynamic "ReadMaxCtrlV.vi"("error in (no error)"=w2835, "APDClass in"=w2836) -> ("error out"=w2826:errorcluster, "Numeric"=w2830:dbl)  [unwired: 7 in, 1 out]
        n1326 = call-dynamic "ReadMaxCtrlV.vi"("error in (no error)"=w2833, "APDClass in"=w2834) -> ("error out"=w2824:errorcluster, "Numeric"=w2829:dbl)  [unwired: 7 in, 1 out]
        n1327 = call-dynamic "ReadMaxCtrlV.vi"("error in (no error)"=w2819, "APDClass in"=w2820) -> ("error out"=w2817:errorcluster, "Numeric"=w2818:dbl)  [unwired: 7 in, 1 out]
        n1328 = property on="V 1" class="DigNum (strict)"(error in=w2828, "Maximum"=w2831) -> (error out=w2827:errorcluster)  [unwired: 1 in, 1 out]
        n1329 = property on="V 2" class="DigNum (strict)"(error in=w2826, "Maximum"=w2830) -> (error out=w2825:errorcluster)  [unwired: 1 in, 1 out]
        n1330 = property on="V 4" class="DigNum (strict)"(error in=w2817, "Maximum"=w2818) -> (error out=w2816:errorcluster)  [unwired: 1 in, 1 out]
        n1331 = property on="V 3" class="DigNum (strict)"(error in=w2824, "Maximum"=w2829) -> (error out=w2823:errorcluster)  [unwired: 1 in, 1 out]
        n1332 = Merge Errors(w2827, w2825, w2823, w2816) -> (w2832:errorcluster)
        n1333 = call <vilib>:"Add State(s) to Queue__JKI_lib_State_Machine.vi"("State(s) in (\"\")"=w2842) -> ("States Out"=w2841:string)  [unwired: 14 in]
      }
      frame "APD: GetGainLimits" {
        w2847 = enum16{"Read", "Write"}."Read" ("Operation (Read)")
        # "Template Separator\n(You can make a copy of, or modify, this frame)"
        n1334 = call "APD1FGV.vi"("Error In"=w2848, "Operation (Read)"=w2847) -> ("Error Out"=w2853:errorcluster, "APDClass out"=w2854:refnum<class "APDClass.lvclass">)  [unwired: 8 in]
        n1335 = call "APD2FGV.vi"("Error In"=w2848, "Operation (Read)"=w2847) -> ("Error Out"=w2860:errorcluster, "APDClass out"=w2861:refnum<class "APDClass.lvclass">)  [unwired: 8 in]
        n1336 = call "APD3FGV.vi"("Error In"=w2848, "Operation (Read)"=w2847) -> ("Error Out"=w2858:errorcluster, "APDClass out"=w2859:refnum<class "APDClass.lvclass">)  [unwired: 8 in]
        n1337 = call "APD4FGV.vi"("Error In"=w2848, "Operation (Read)"=w2847) -> ("Error Out"=w2845:errorcluster, "APDClass out"=w2846:refnum<class "APDClass.lvclass">)  [unwired: 8 in]
        n1338 = call-dynamic "Read Gain Limits(Log).vi"("error in (no error)"=w2853, "APDClass in"=w2854) -> ("error out"=w2852:errorcluster, "GainLimits(Log)"=w2849:cluster{"GainMax":dbl, "GainMin":dbl})  [unwired: 7 in, 1 out]
        n1339 = call-dynamic "Read Gain Limits(Log).vi"("error in (no error)"=w2860, "APDClass in"=w2861) -> ("error out"=w2856:errorcluster, "GainLimits(Log)"=w2851:cluster{"GainMax":dbl, "GainMin":dbl})  [unwired: 7 in, 1 out]
        n1340 = call-dynamic "Read Gain Limits(Log).vi"("error in (no error)"=w2858, "APDClass in"=w2859) -> ("error out"=w2855:errorcluster, "GainLimits(Log)"=w2850:cluster{"GainMax":dbl, "GainMin":dbl})  [unwired: 7 in, 1 out]
        n1341 = call-dynamic "Read Gain Limits(Log).vi"("error in (no error)"=w2845, "APDClass in"=w2846) -> ("error out"=w2843:errorcluster, "GainLimits(Log)"=w2844:cluster{"GainMax":dbl, "GainMin":dbl})  [unwired: 7 in, 1 out]
        n1342 = Merge Errors(w2852, w2856, w2855, w2843) -> (w2857:errorcluster)
        n1343 = global write "GlobalVariables.vi" "Ch1GainLim(Log)"(w2849) -> ()
        n1344 = global write "GlobalVariables.vi" "Ch2GainLim(Log)"(w2851) -> ()
        n1345 = global write "GlobalVariables.vi" "Ch3GainLim(Log)"(w2850) -> ()
        n1346 = global write "GlobalVariables.vi" "Ch4GainLim(Log)"(w2844) -> ()
        n1347 = call <vilib>:"Add State(s) to Queue__JKI_lib_State_Machine.vi"("State(s) in (\"\")"=w2865) -> ("States Out"=w2864:string)  [unwired: 14 in]
      }
      frame "---------- TCP ----------" {
        # "Template Separator\n(You can make a copy of, or modify, this frame)"
        n1348 = call <vilib>:"Add State(s) to Queue__JKI_lib_State_Machine.vi"("State(s) in (\"\")"=w2870) -> ("States Out"=w2869:string)  [unwired: 14 in]
      }
      frame "TCP: InitializeNew" {
        # "if unsuccessful and count <10, increament count \nand try again"
        # "Initialize TCP connection to aimging beam computer\n(You can make a copy of, or modify, this frame)"
        n1349 = TCP Create Listener(10:u16 2100 ("port"), 11:"RTLT" ("service name")) -> (0:w2879:errorcluster, 3:w2871:refnum<k5>)  [unwired: 3 in, 1 out]
        n1350 = while {
          tunnel: w2871 -> [w2899]
          tunnel: w2879 -> [w2898]
          tunnel: [w2889] -> w2877
          tunnel: [w2886] -> w2873
          i -> [w2895]
          stop <- w2886 stop-if-true
          n1351 = TCP Wait On Listener(8:w2898, 9:200 ("timeout ms (wait forever: -1)"), 11:w2899) -> (0:w2896:errorcluster, 4:w2893:refnum<k5>)  [unwired: 1 in, 3 out]
          n1352 = Less Or Equal?(x=50, y=w2895) -> (x <= y?=w2892:bool)
          n1353 = case shown="No Error" w2896 {
            selector: w2896 -> [w2909 w2919]
            tunnel: w2893 -> [w2910 _]
            tunnel: [errorcluster {"status"=TRUE, "code"=0, "source"=""} ("No error") w2920] -> w2888
            tunnel: [w2901 FALSE ("TCP connected?")] -> w2889
            frame No Error {
              # "connection is ready, read data"
              n1354 = TCP Read(connection ID=w2910, bytes to read=512, error in (no error)=w2909, 7:T22."CRLF" ("mode (standard)"), 9:5000 ("timeout ms (25000)")) -> (connection ID out=w2903:refnum<k5>, data out=w2905:string, error out=w2902:errorcluster)
              n1355 = Concatenate Strings("alive" ("string"), "\r\n" ("End of Line Constant")) -> (w2906:string)
              n1356 = Equal?(x=w2906, y=w2905) -> (x = y?=w2904:bool)
              n1357 = case shown="False" w2904 {
                tunnel: w2903 -> [_ w2915]
                tunnel: w2902 -> [_ _]
                tunnel: [FALSE ("TCP connected?") TRUE ("TCP connected?")] -> w2901
                frame False {
                }
                frame True {
                  n1358 = call "TcpIDFGV.vi"("action"=enum16{"write", "read"}."write", "connection ID in"=w2915) -> ()  [unwired: 8 in, 2 out]
                }
              }
            }
            frame Error {
              # "connection not ready, keep waiting"
              n1359 = Unbundle By Name(w2919) -> ("code"=w2921:i32)
              n1360 = case shown="56" w2921 {
                tunnel: w2919 -> [w2922 _]
                tunnel: [w2922 w2923] -> w2920
                frame Default {
                }
                frame 56 {
                  w2923 = errorcluster {"status"=FALSE, "code"=0, "source"=""}  # No error
                }
              }
            }
          }
          n1361 = Select(t=errorcluster {"status"=TRUE, "code"=5001, "source"=""} ("error in (no error)"), s=w2892, f=errorcluster {"status"=FALSE, "code"=0, "source"=""} ("error in (no error)")) -> (s? t:f=w2887:errorcluster)
          n1362 = Merge Errors(w2888, w2887) -> (w2886:errorcluster)
        }
        n1363 = Unbundle By Name(w2873) -> ("code"=w2876:i32)
        n1364 = Bundle By Name(cluster=w2878, "System Status.TCP/IP"=w2877, "listener ID"=w2871) -> (w2883:T27)
        n1365 = global write "GlobalVariables.vi" "TCP connected?"(w2877) -> ()
        n1366 = Equal To 0?(x=w2876) -> (x = 0?=w2875:bool)
        n1367 = Select(t=errorcluster {"status"=FALSE, "code"=0, "source"=""} ("error in (no error)"), s=w2875, f=w2873) -> (s? t:f=w2872:errorcluster)
        n1368 = call <vilib>:"Add State(s) to Queue__JKI_lib_State_Machine.vi"("State(s) in (\"\")"=w2885) -> ("States Out"=w2884:string)  [unwired: 14 in]
      }
      frame "TCP: checkSource" {
        # "Check visualization PC video source\n(send !video_source message, listen for response, then parse it to binary mask)"
        n1369 = Unbundle By Name(w2930) -> ("System Status.TCP/IP"=w2933:bool)
        n1370 = case shown="True" w2933 {
          tunnel: w2932 -> [w2938 w2961]
          tunnel: [w2938 w2945] -> w2931
          tunnel: [w2937 w2950] -> w2928
          tunnel: [w2937 w2948] -> w2927
          tunnel: [w2937 w2949] -> w2926
          tunnel: [w2937 w2947] -> w2925
          tunnel: [w2937 w2939] -> w2924
          frame False {
            w2937 = FALSE
          }
          frame True {
            n1371 = call "TcpIDFGV.vi"("Error In"=w2961, "action"=enum16{"write", "read"}."read") -> ("Error Out"=w2958:errorcluster, "connection ID out"=w2960:refnum<k5>)  [unwired: 8 in]
            n1372 = call "TCP_WriteRead.vi"("error in (no error)"=w2958, "data in"="!video_source", "connectin ID in"=w2960) -> ("error out"=w2955:errorcluster, "data out"=w2957:string)  [unwired: 4 in, 1 out]
            n1373 = Scan From String(format string="!video_source:%d", input string=w2957, error in=w2955) -> (error out=w2946:errorcluster, output 1=w2944:i32)  [unwired: 2 in, 2 out]
            n1374 = case shown="5..7, 9..11, 13..15" w2944 {
              tunnel: w2946 -> [_ _ _ _]
              tunnel: [errorcluster {"status"=TRUE, "code"=5007, "source"="Visualization PC"} ("error out") errorcluster {"status"=FALSE, "code"=0, "source"=""} ("error out") errorcluster {"status"=FALSE, "code"=0, "source"=""} ("error out") errorcluster {"status"=FALSE, "code"=0, "source"=""} ("error out")] -> w2945
              tunnel: [FALSE FALSE FALSE TRUE] -> w2939
              frame 0, Default {
                # "No video source available or default"
                n1375 = property on="Video Source" class="RadioBtnsControl (strict)"("DisabledEnum"=T12."Disabled and Grayed Out" ("Disabled")) -> ()  [unwired: 2 in, 2 out]
              }
              frame 1..3 {
                # "one or both camera available"
                n1376 = local write "Video Source"(enum32{"Camera", "FrameGrabber"}."Camera" ("Video Source")) -> ()
                n1377 = property on="Video Source" class="RadioBtnsControl (strict)"("DisabledEnum"=T12."Disabled and Grayed Out" ("Disabled")) -> ()  [unwired: 2 in, 2 out]
              }
              frame 4, 8, 12 {
                # "one or both frame grabber available"
                n1378 = local write "Video Source"(enum32{"Camera", "FrameGrabber"}."FrameGrabber" ("Video Source")) -> ()
                n1379 = property on="Video Source" class="RadioBtnsControl (strict)"("DisabledEnum"=T12."Disabled and Grayed Out" ("Disabled")) -> ()  [unwired: 2 in, 2 out]
              }
              frame 5..7, 9..11, 13..15 {
                n1380 = property on="Video Source" class="RadioBtnsControl (strict)"("DisabledEnum"=T12."Enabled" ("Disabled")) -> ()  [unwired: 2 in, 2 out]
              }
            }
            n1381 = Integer to Fixed-Point Cast(fixed-point type=fxp<+,4,4> 0.0, integer=w2944) -> (fixed-point=w2943:fxp<+,4,4>)
            n1382 = Number To Boolean Array(number=w2943) -> (Boolean array=w2941:bool[])
            n1383 = Reverse 1D Array(array=w2941) -> (reversed array=w2940:bool[])
            n1384 = Index Array(array=w2940, index=0) -> (element=w2950:bool)
            n1385 = Index Array(array=w2940, index=1) -> (element=w2948:bool)
            n1386 = Index Array(array=w2940, index=2) -> (element=w2949:bool)
            n1387 = Index Array(array=w2940, index=3) -> (element=w2947:bool)
          }
        }
        n1388 = Bundle By Name(cluster=w2930, "video source.Main Frame Grabber"=w2928, "video source.Side Frame Grabber"=w2927, "video source.Main Camera"=w2926, "video source.Side Camera"=w2925, "bothVidSourceAvail"=w2924) -> (w2929:T27)
        n1389 = call <vilib>:"Add State(s) to Queue__JKI_lib_State_Machine.vi"("State(s) in (\"\")"=w2936) -> ("States Out"=w2935:string)  [unwired: 14 in]
      }
      frame "TCP: SyncTime" {
        # "Template Separator\n(You can make a copy of, or modify, this frame)"
        n1390 = Unbundle By Name(w2978) -> ("System Status.TCP/IP"=w2977:bool)
        n1391 = case shown="True" w2977 {
          tunnel: w2979 -> [_ w2987]
          frame False {
          }
          frame True {
            n1392 = call "TcpIDFGV.vi"("Error In"=w2987, "action"=enum16{"write", "read"}."read") -> ("Error Out"=w2986:errorcluster, "connection ID out"=w2983:refnum<k5>)  [unwired: 8 in]
            n1393 = call <userlib>:"Tick Count (ms)__ogtk.vi"("error in (no error)"=w2986) -> ("error out"=w2985:errorcluster, "millisecond timer value"=w2984:u32)  [unwired: 9 in]
            n1394 = while {
              tunnel: w2985 -> [w3007]
              tunnel: w2983 -> [w3006]
              tunnel: w2984 -> [w2995]
              stop <- w2990 stop-if-true
              n1395 = Concatenate Strings("latencycheck" ("string"), "\r\n" ("End of Line Constant")) -> (w3002:string)
              n1396 = TCP Read(connection ID=w3006, bytes to read=512, error in (no error)=w3007, 7:T22."CRLF" ("mode (standard)"), 9:2000 ("timeout ms (25000)")) -> (connection ID out=w2999:refnum<k5>, data out=w2997:string, error out=w2989:errorcluster)
              n1397 = Tick Count (ms)() -> (millisecond timer value=w2996:u32)
              n1398 = Subtract(x=w2996, y=w2995) -> (x-y=w2994:u32)
              n1399 = Equal?(x=w2997, y=w3002) -> (x = y?=w2998:bool)
              n1400 = case shown="True" w2998 {
                tunnel: w2999 -> [_ w3020]
                tunnel: w2997 -> [w3012 _]
                tunnel: [w3008 FALSE] -> w2992
                tunnel: w2989 -> [_ w3014]
                frame False {
                  n1401 = Concatenate Strings("synctimer" ("string"), "\r\n" ("End of Line Constant")) -> (w3009:string)
                  n1402 = Equal?(x=w3012, y=w3009) -> (x = y?=w3008:bool)
                  "Sync Success?" <- w3008
                }
                frame True {
                  n1403 = Concatenate Strings("latencycheck:" ("string"), "\r\n" ("End of Line Constant")) -> (w3019:string)
                  n1404 = TCP Write(connection ID=w3020, data in=w3019, error in (no error)=w3014, 9:1000 ("timeout ms (25000)")) -> (error out=w3013:errorcluster)  [unwired: 2 out]
                  n1405 = call <vilib>:"Clear Errors.vi"("error in (no error)"=w3013) -> ()  [unwired: 5 in, 2 out]
                }
              }
              n1406 = Greater?(x=w2994, y=u32 10000 ("x-y")) -> (0:w2991:bool)
              n1407 = Or(x=w2992, y=w2991) -> (x .or. y?=w2990:bool)
            }
          }
        }
        n1408 = call <vilib>:"Add State(s) to Queue__JKI_lib_State_Machine.vi"("State(s) in (\"\")"=w2982) -> ("States Out"=w2981:string)  [unwired: 14 in]
      }
      frame "TCP: SendSettingMacro" {
        # "Template Separator\n(You can make a copy of, or modify, this frame)"
        n1409 = Unbundle By Name(w3024) -> ("System Status.TCP/IP"=w3023:bool)
        n1410 = case shown="True" w3023 {
          tunnel: ["" ("Empty String Constant") "TCP: sendSubjectID\nTCP: sendScaleBarSetting\nTCP: sendScaleMaxMin\nTCP: sendDeconChannel\nTCP: sendANSI\nTCP: sendRadius\nTCP: send3Dsetting\nTCP: sendFirefly\nTCP: sendPentero"] -> w3022
          frame False {
          }
          frame True {
          }
        }
        n1411 = call <vilib>:"Add State(s) to Queue__JKI_lib_State_Machine.vi"("State(s) in Front (\"\")"=w3022, "State(s) in (\"\")"=w3027) -> ("States Out"=w3026:string)  [unwired: 13 in]
      }
      frame "TCP: sendRunNum" {
        # "Send run number to AB PC\n(You can make a copy of, or modify, this frame)"
        n1412 = Unbundle By Name(w3034) -> ("System Status.TCP/IP"=w3031:bool, "IDs.RunID"=w3035:i8)
        n1413 = Increment(x=w3035) -> (x+1=w3030:i8)
        n1414 = case shown="True" w3031 {
          tunnel: w3030 -> [_ w3049]
          tunnel: [w3039 w3041] -> w3033
          tunnel: w3032 -> [w3039 w3040]
          frame False {
          }
          frame True {
            n1415 = Number To Decimal String(number=w3049, width (-)=i16 3) -> (decimal integer string=w3044:string)
            n1416 = call "TcpIDFGV.vi"("Error In"=w3040, "action"=enum16{"write", "read"}."read") -> ("Error Out"=w3042:errorcluster, "connection ID out"=w3046:refnum<k5>)  [unwired: 8 in]
            n1417 = Concatenate Strings("!run:", w3044) -> (w3043:string)
            n1418 = call "TCP_WriteRead.vi"("error in (no error)"=w3042, "data in"=w3043, "connectin ID in"=w3046) -> ("error out"=w3041:errorcluster)  [unwired: 4 in, 2 out]
          }
        }
        n1419 = call <vilib>:"Add State(s) to Queue__JKI_lib_State_Machine.vi"("State(s) in (\"\")"=w3038) -> ("States Out"=w3037:string)  [unwired: 14 in]
      }
      frame "TCP: sendVideoSource" {
        # "Send video source \n(You can make a copy of, or modify, this frame)"
        n1420 = Unbundle By Name(w3051) -> ("System Status.TCP/IP"=w3050:bool)
        n1421 = case shown="True" w3050 {
          tunnel: [w3057 w3059] -> w3053
          tunnel: w3052 -> [w3057 w3058]
          frame False {
          }
          frame True {
            n1422 = case shown="\"Camera\", Default" "Video Source" {
              tunnel: [0 1] -> w3064
              frame "Camera", Default {
              }
              frame "FrameGrabber" {
              }
            }
            n1423 = call "TcpIDFGV.vi"("Error In"=w3058, "action"=enum16{"write", "read"}."read") -> ("Error Out"=w3060:errorcluster, "connection ID out"=w3066:refnum<k5>)  [unwired: 8 in]
            n1424 = Number To Decimal String(number=w3064) -> (decimal integer string=w3062:string)  [unwired: 1 in]
            n1425 = Concatenate Strings("!invivo:" ("data in"), w3062) -> (w3061:string)
            n1426 = call "TCP_WriteRead.vi"("error in (no error)"=w3060, "data in"=w3061, "connectin ID in"=w3066) -> ("error out"=w3059:errorcluster)  [unwired: 4 in, 2 out]
          }
        }
        n1427 = call <vilib>:"Add State(s) to Queue__JKI_lib_State_Machine.vi"("State(s) in (\"\")"=w3056) -> ("States Out"=w3055:string)  [unwired: 14 in]
      }
      frame "TCP: startRun" {
        # "Template Separator\n(You can make a copy of, or modify, this frame)"
        n1428 = Unbundle By Name(w3071) -> ("System Status.TCP/IP"=w3070:bool)
        n1429 = case shown="True" w3070 {
          tunnel: [w3077 w3079] -> w3073
          tunnel: w3072 -> [w3077 w3078]
          frame False {
          }
          frame True {
            n1430 = call "TcpIDFGV.vi"("Error In"=w3078, "action"=enum16{"write", "read"}."read") -> ("Error Out"=w3080:errorcluster, "connection ID out"=w3081:refnum<k5>)  [unwired: 8 in]
            n1431 = call "TCP_WriteRead.vi"("error in (no error)"=w3080, "data in"="!acquire:1", "connectin ID in"=w3081) -> ("error out"=w3079:errorcluster)  [unwired: 4 in, 2 out]
          }
        }
        n1432 = call <vilib>:"Add State(s) to Queue__JKI_lib_State_Machine.vi"("State(s) in (\"\")"=w3076) -> ("States Out"=w3075:string)  [unwired: 14 in]
      }
      frame "TCP: stopRun" {
        # "Send stop run to AB PC\n(You can make a copy of, or modify, this frame)"
        n1433 = Unbundle By Name(w3085) -> ("System Status.TCP/IP"=w3084:bool)
        n1434 = case shown="True" w3084 {
          tunnel: [w3091 w3093] -> w3087
          tunnel: w3086 -> [w3091 w3092]
          frame False {
            # "if not connected, do nothing"
          }
          frame True {
            # "If TCP connected, send stop run"
            n1435 = call "TcpIDFGV.vi"("Error In"=w3092, "action"=enum16{"write", "read"}."read") -> ("Error Out"=w3094:errorcluster, "connection ID out"=w3096:refnum<k5>)  [unwired: 8 in]
            n1436 = call "TCP_WriteRead.vi"("error in (no error)"=w3094, "data in"="!acquire:0", "connectin ID in"=w3096) -> ("error out"=w3093:errorcluster)  [unwired: 4 in, 2 out]
          }
        }
        n1437 = call <vilib>:"Add State(s) to Queue__JKI_lib_State_Machine.vi"("State(s) in (\"\")"=w3090) -> ("States Out"=w3089:string)  [unwired: 14 in]
      }
      frame "TCP: CheckConnection" {
        # "Check TCP/IP connection statuse\n(If connection is lost, throw error)"
        n1438 = Unbundle By Name(w3099) -> ("System Status.TCP/IP"=w3098:bool)
        n1439 = case shown="True" w3098 {
          frame False {
          }
          frame True {
            # "If TCP/IP is true check, otherwise skip"
          }
        }
        n1440 = call <vilib>:"Add State(s) to Queue__JKI_lib_State_Machine.vi"("State(s) in (\"\")"=w3103) -> ("States Out"=w3102:string)  [unwired: 14 in]
      }
      frame "TCP: sendSubjectID" {
        # "Send subject ID"
        n1441 = Unbundle By Name(w3105) -> ("System Status.TCP/IP"=w3104:bool, "CaseID"=w3108:string)
        n1442 = case shown="True" w3104 {
          tunnel: w3108 -> [_ w3119]
          tunnel: [w3112 w3114] -> w3107
          tunnel: w3106 -> [w3112 w3113]
          frame False {
          }
          frame True {
            n1443 = call "TcpIDFGV.vi"("Error In"=w3113, "action"=enum16{"write", "read"}."read") -> ("Error Out"=w3115:errorcluster, "connection ID out"=w3117:refnum<k5>)  [unwired: 8 in]
            n1444 = Concatenate Strings("!subject:", w3119) -> (w3116:string)
            n1445 = call "TCP_WriteRead.vi"("error in (no error)"=w3115, "data in"=w3116, "connectin ID in"=w3117) -> ("error out"=w3114:errorcluster)  [unwired: 4 in, 2 out]
          }
        }
        n1446 = call <vilib>:"Add State(s) to Queue__JKI_lib_State_Machine.vi"("State(s) in (\"\")"=w3111) -> ("States Out"=w3110:string)  [unwired: 14 in]
      }
      frame "TCP: sendScaleBarSetting" {
        # "Template Separator\n(You can make a copy of, or modify, this frame)"
        n1447 = Unbundle By Name(w3123) -> ("System Status.TCP/IP"=w3121:bool, "VideoConfig.Scale Bar"=w3122:bool)
        n1448 = case shown="True" w3121 {
          tunnel: [w3129 w3138] -> w3125
          tunnel: w3124 -> [w3129 w3137]
          tunnel: w3122 -> [_ w3136]
          frame False {
          }
          frame True {
            n1449 = Boolean To (0,1)(Boolean=w3136) -> (0, 1=w3135:i16)
            n1450 = call "TcpIDFGV.vi"("Error In"=w3137, "action"=enum16{"write", "read"}."read") -> ("Error Out"=w3139:errorcluster, "connection ID out"=w3140:refnum<k5>)  [unwired: 8 in]
            n1451 = Number To Fractional String(number=w3135, width (-)=i16 1, precision (6)=i16 0) -> (F-format string=w3133:string)  [unwired: 1 in]
            n1452 = Concatenate Strings("!autocolor:" ("data in"), w3133) -> (w3131:string)
            n1453 = call "TCP_WriteRead.vi"("error in (no error)"=w3139, "data in"=w3131, "connectin ID in"=w3140) -> ("error out"=w3138:errorcluster)  [unwired: 4 in, 2 out]
          }
        }
        n1454 = call <vilib>:"Add State(s) to Queue__JKI_lib_State_Machine.vi"("State(s) in (\"\")"=w3128) -> ("States Out"=w3127:string)  [unwired: 14 in]
      }
      frame "TCP: sendScaleMaxMin" {
        # "Send scale bar max and min to AB PC\n(You can make a copy of, or modify, this frame)"
        n1455 = Unbundle By Name(w3145) -> ("System Status.TCP/IP"=w3142:bool, "VideoConfig.Scale Low"=w3144:dbl, "VideoConfig.Scale High"=w3143:dbl)
        n1456 = case shown="True" w3142 {
          tunnel: [w3151 w3164] -> w3147
          tunnel: w3146 -> [w3151 w3163]
          tunnel: w3144 -> [_ w3162]
          tunnel: w3143 -> [_ w3153]
          frame False {
          }
          frame True {
            n1457 = call "TcpIDFGV.vi"("Error In"=w3163, "action"=enum16{"write", "read"}."read") -> ("Error Out"=w3165:errorcluster, "connection ID out"=w3166:refnum<k5>)  [unwired: 8 in]
            n1458 = Number To Fractional String(number=w3162, width (-)=i16 4, precision (6)=i16 2) -> (F-format string=w3158:string)  [unwired: 1 in]
            n1459 = Number To Fractional String(number=w3153, width (-)=i16 4, precision (6)=i16 2) -> (F-format string=w3154:string)  [unwired: 1 in]
            n1460 = Concatenate Strings("!color:" ("string"), w3158, ";" ("string"), w3154) -> (w3152:string)
            n1461 = call "TCP_WriteRead.vi"("error in (no error)"=w3165, "data in"=w3152, "connectin ID in"=w3166) -> ("error out"=w3164:errorcluster)  [unwired: 4 in, 2 out]
          }
        }
        n1462 = call <vilib>:"Add State(s) to Queue__JKI_lib_State_Machine.vi"("State(s) in (\"\")"=w3150) -> ("States Out"=w3149:string)  [unwired: 14 in]
      }
      frame "TCP: sendDeconChannel" {
        # "Send Decon channel\n(You can make a copy of, or modify, this frame)"
        n1463 = Unbundle By Name(w3169) -> ("System Status.TCP/IP"=w3168:bool)
        n1464 = case shown="True" w3168 {
          tunnel: [w3175 w3180] -> w3171
          tunnel: w3170 -> [w3175 w3179]
          frame False {
          }
          frame True {
            n1465 = local read "Radio Buttons"() -> (w3178:T10)
            n1466 = Increment(x=w3178) -> (x+1=w3177:T10)
            n1467 = Number To Decimal String(number=w3177) -> (decimal integer string=w3176:string)  [unwired: 1 in]
            n1468 = call "TcpIDFGV.vi"("Error In"=w3179, "action"=enum16{"write", "read"}."read") -> ("Error Out"=w3181:errorcluster, "connection ID out"=w3184:refnum<k5>)  [unwired: 8 in]
            n1469 = Concatenate Strings("!channel:", w3176) -> (w3182:string)
            n1470 = call "TCP_WriteRead.vi"("error in (no error)"=w3181, "data in"=w3182, "connectin ID in"=w3184) -> ("error out"=w3180:errorcluster)  [unwired: 4 in, 2 out]
          }
        }
        n1471 = call <vilib>:"Add State(s) to Queue__JKI_lib_State_Machine.vi"("State(s) in (\"\")"=w3174) -> ("States Out"=w3173:string)  [unwired: 14 in]
      }
      frame "TCP: sendANSI" {
        # "Template Separator\n(You can make a copy of, or modify, this frame)"
        n1472 = Unbundle By Name(w3188) -> ("System Status.TCP/IP"=w3186:bool, "VideoConfig.ANSI"=w3187:dbl)
        n1473 = case shown="True" w3186 {
          tunnel: [w3194 w3200] -> w3190
          tunnel: w3189 -> [w3194 w3199]
          tunnel: w3187 -> [_ w3198]
          frame False {
          }
          frame True {
            n1474 = Number To Fractional String(number=w3198) -> (F-format string=w3196:string)  [unwired: 3 in]
            n1475 = call "TcpIDFGV.vi"("Error In"=w3199, "action"=enum16{"write", "read"}."read") -> ("Error Out"=w3201:errorcluster, "connection ID out"=w3202:refnum<k5>)  [unwired: 8 in]
            n1476 = Concatenate Strings("!ansi:" ("data in"), w3196) -> (w3195:string)
            n1477 = call "TCP_WriteRead.vi"("error in (no error)"=w3201, "data in"=w3195, "connectin ID in"=w3202) -> ("error out"=w3200:errorcluster)  [unwired: 4 in, 2 out]
          }
        }
        n1478 = call <vilib>:"Add State(s) to Queue__JKI_lib_State_Machine.vi"("State(s) in (\"\")"=w3193) -> ("States Out"=w3192:string)  [unwired: 14 in]
      }
      frame "TCP: sendRadius" {
        # "Send drawing radius to AB PC\n(You can make a copy of, or modify, this frame)"
        n1479 = Unbundle By Name(w3206) -> ("System Status.TCP/IP"=w3204:bool, "VideoConfig.Radius"=w3205:dbl)
        n1480 = case shown="True" w3204 {
          tunnel: [w3212 w3218] -> w3208
          tunnel: w3207 -> [w3212 w3217]
          tunnel: w3205 -> [_ w3216]
          frame False {
          }
          frame True {
            n1481 = Number To Fractional String(number=w3216) -> (F-format string=w3215:string)  [unwired: 3 in]
            n1482 = Concatenate Strings("!radius:" ("data in"), w3215) -> (w3213:string)
            n1483 = call "TcpIDFGV.vi"("Error In"=w3217, "action"=enum16{"write", "read"}."read") -> ("Error Out"=w3219:errorcluster, "connection ID out"=w3220:refnum<k5>)  [unwired: 8 in]
            n1484 = call "TCP_WriteRead.vi"("error in (no error)"=w3219, "data in"=w3213, "connectin ID in"=w3220) -> ("error out"=w3218:errorcluster)  [unwired: 4 in, 2 out]
          }
        }
        n1485 = call <vilib>:"Add State(s) to Queue__JKI_lib_State_Machine.vi"("State(s) in (\"\")"=w3211) -> ("States Out"=w3210:string)  [unwired: 14 in]
      }
      frame "TCP: send3Dsetting" {
        # "Send 3D setting to AB computer\n(You can make a copy of, or modify, this frame)"
        n1486 = Unbundle By Name(w3224) -> ("System Status.TCP/IP"=w3222:bool, "VideoConfig.3D?"=w3223:bool)
        n1487 = case shown="True" w3222 {
          tunnel: [w3230 w3237] -> w3226
          tunnel: w3225 -> [w3230 w3236]
          tunnel: w3223 -> [_ w3235]
          frame False {
          }
          frame True {
            n1488 = Boolean To (0,1)(Boolean=w3235) -> (0, 1=w3234:i16)
            n1489 = Number To Fractional String(number=w3234) -> (F-format string=w3233:string)  [unwired: 3 in]
            n1490 = call "TcpIDFGV.vi"("Error In"=w3236, "action"=enum16{"write", "read"}."read") -> ("Error Out"=w3238:errorcluster, "connection ID out"=w3239:refnum<k5>)  [unwired: 8 in]
            n1491 = Concatenate Strings("!3dset:" ("data in"), w3233) -> (w3231:string)
            n1492 = call "TCP_WriteRead.vi"("error in (no error)"=w3238, "data in"=w3231, "connectin ID in"=w3239) -> ("error out"=w3237:errorcluster)  [unwired: 4 in, 2 out]
          }
        }
        n1493 = call <vilib>:"Add State(s) to Queue__JKI_lib_State_Machine.vi"("State(s) in (\"\")"=w3229) -> ("States Out"=w3228:string)  [unwired: 14 in]
      }
      frame "TCP: sendFirefly" {
        # "Template Separator\n(You can make a copy of, or modify, this frame)"
        n1494 = Unbundle By Name(w3242) -> ("System Status.TCP/IP"=w3241:bool)
        n1495 = case shown="False" w3241 {
          tunnel: [w3248 w3250] -> w3244
          tunnel: w3243 -> [w3248 w3249]
          frame False {
          }
          frame True {
            n1496 = call "TcpIDFGV.vi"("Error In"=w3249, "action"=enum16{"write", "read"}."read") -> ("Error Out"=w3251:errorcluster, "connection ID out"=w3253:refnum<k5>)  [unwired: 8 in]
            n1497 = call "TCP_WriteRead.vi"("error in (no error)"=w3251, "data in"="!firefly:0", "connectin ID in"=w3253) -> ("error out"=w3250:errorcluster)  [unwired: 4 in, 2 out]
          }
        }
        n1498 = call <vilib>:"Add State(s) to Queue__JKI_lib_State_Machine.vi"("State(s) in (\"\")"=w3247) -> ("States Out"=w3246:string)  [unwired: 14 in]
      }
      frame "TCP: sendPentero" {
        # "Send Pentero setting to AB computer\n(You can make a copy of, or modify, this frame)"
        n1499 = Unbundle By Name(w3256) -> ("System Status.TCP/IP"=w3255:bool)
        n1500 = case shown="True" w3255 {
          tunnel: [w3262 w3264] -> w3258
          tunnel: w3257 -> [w3262 w3263]
          frame False {
          }
          frame True {
            n1501 = call "TcpIDFGV.vi"("Error In"=w3263, "action"=enum16{"write", "read"}."read") -> ("Error Out"=w3265:errorcluster, "connection ID out"=w3267:refnum<k5>)  [unwired: 8 in]
            n1502 = call "TCP_WriteRead.vi"("error in (no error)"=w3265, "data in"="!pentero:0", "connectin ID in"=w3267) -> ("error out"=w3264:errorcluster)  [unwired: 4 in, 2 out]
          }
        }
        n1503 = call <vilib>:"Add State(s) to Queue__JKI_lib_State_Machine.vi"("State(s) in (\"\")"=w3261) -> ("States Out"=w3260:string)  [unwired: 14 in]
      }
      frame "TCP: sendChannel" {
        # "Send DeCon Channel to AB computer\n()"
        n1504 = Unbundle By Name(w3270) -> ("System Status.TCP/IP"=w3269:bool)
        n1505 = case shown="True" w3269 {
          tunnel: [w3276 w3280] -> w3272
          tunnel: w3271 -> [w3276 w3279]
          frame False {
          }
          frame True {
            n1506 = local read "Radio Buttons"() -> (w3278:T10)
            n1507 = case shown="\"No Selection\", Default" w3278 {
              tunnel: ["" ("data in") "!channel:1" ("data in") "!channel:2" ("data in") "!channel:3" ("data in")] -> w3277
              frame "No Selection", Default {
              }
              frame "Ch1" {
              }
              frame "Ch2" {
              }
              frame "Ch3" {
              }
            }
            n1508 = call "TcpIDFGV.vi"("Error In"=w3279, "action"=enum16{"write", "read"}."read") -> ("Error Out"=w3281:errorcluster, "connection ID out"=w3282:refnum<k5>)  [unwired: 8 in]
            n1509 = call "TCP_WriteRead.vi"("error in (no error)"=w3281, "data in"=w3277, "connectin ID in"=w3282) -> ("error out"=w3280:errorcluster)  [unwired: 4 in, 2 out]
          }
        }
        n1510 = call <vilib>:"Add State(s) to Queue__JKI_lib_State_Machine.vi"("State(s) in (\"\")"=w3275) -> ("States Out"=w3274:string)  [unwired: 14 in]
      }
      frame "TCP: startCam" {
        # "Send Pentero setting to AB computer\n(You can make a copy of, or modify, this frame)"
        n1511 = Unbundle By Name(w3289) -> ("System Status.TCP/IP"=w3288:bool)
        n1512 = case shown="True" w3288 {
          tunnel: [w3295 w3297] -> w3291
          tunnel: w3290 -> [w3295 w3296]
          frame False {
          }
          frame True {
            n1513 = call "TcpIDFGV.vi"("Error In"=w3296, "action"=enum16{"write", "read"}."read") -> ("Error Out"=w3298:errorcluster, "connection ID out"=w3300:refnum<k5>)  [unwired: 8 in]
            n1514 = call "TCP_WriteRead.vi"("error in (no error)"=w3298, "data in"="!focus:1", "connectin ID in"=w3300) -> ("error out"=w3297:errorcluster)  [unwired: 4 in, 2 out]
          }
        }
        n1515 = call <vilib>:"Add State(s) to Queue__JKI_lib_State_Machine.vi"("State(s) in (\"\")"=w3294) -> ("States Out"=w3293:string)  [unwired: 14 in]
      }
      frame "TCP: stopCam" {
        # "Send Pentero setting to AB computer\n(You can make a copy of, or modify, this frame)"
        n1516 = Unbundle By Name(w3303) -> ("System Status.TCP/IP"=w3302:bool)
        n1517 = case shown="True" w3302 {
          tunnel: [w3309 w3311] -> w3305
          tunnel: w3304 -> [w3309 w3310]
          frame False {
          }
          frame True {
            n1518 = call "TcpIDFGV.vi"("Error In"=w3310, "action"=enum16{"write", "read"}."read") -> ("Error Out"=w3312:errorcluster, "connection ID out"=w3314:refnum<k5>)  [unwired: 8 in]
            n1519 = call "TCP_WriteRead.vi"("error in (no error)"=w3312, "data in"="!focus:0", "connectin ID in"=w3314) -> ("error out"=w3311:errorcluster)  [unwired: 4 in, 2 out]
          }
        }
        n1520 = call <vilib>:"Add State(s) to Queue__JKI_lib_State_Machine.vi"("State(s) in (\"\")"=w3308) -> ("States Out"=w3307:string)  [unwired: 14 in]
      }
      frame "TCP: Close" {
        # "Close TCP connection\n()"
        n1521 = Unbundle By Name(w3318) -> ("System Status.TCP/IP"=w3316:bool)
        n1522 = case shown="True" w3316 {
          tunnel: [w3324 w3326] -> w3319
          tunnel: w3317 -> [w3324 w3325]
          frame False {
          }
          frame True {
            n1523 = call "TcpIDFGV.vi"("Error In"=w3325, "action"=enum16{"write", "read"}."read") -> ("Error Out"=w3328:errorcluster, "connection ID out"=w3329:refnum<k5>)  [unwired: 8 in]
            n1524 = TCP Close Connection(connection ID=w3329, error in (no error)=w3328) -> (error out=w3326:errorcluster)  [unwired: 1 in, 1 out]
          }
        }
        n1525 = case shown="Error .." w3319 {
          tunnel: [w3332 w3333] -> w3320
          tunnel: w3318 -> [w3331 w3333]
          frame No Error {
            w3330 = FALSE ("System Status.TCP/IP")
            n1526 = Bundle By Name(cluster=w3331, "System Status.TCP/IP"=w3330) -> (w3332:T27)
            n1527 = global write "GlobalVariables.vi" "TCP connected?"(w3330) -> ()
          }
          frame Error {
          }
        }
        n1528 = call <vilib>:"Add State(s) to Queue__JKI_lib_State_Machine.vi"("State(s) in (\"\")"=w3323) -> ("States Out"=w3322:string)  [unwired: 14 in]
      }
      frame "---------- PID ----------" {
        # "Template Separator\n(You can make a copy of, or modify, this frame)"
        n1529 = call <vilib>:"Add State(s) to Queue__JKI_lib_State_Machine.vi"("State(s) in (\"\")"=w3338) -> ("States Out"=w3337:string)  [unwired: 14 in]
      }
      frame "PID: loadPID" {
        # "Template Separator\n(You can make a copy of, or modify, this frame)"
        n1530 = call "readPIDSetting.vi"("Error In"=w3342) -> ("Error Out"=w3343:errorcluster, "Ch3 PID out"=w3339:T9, "Ch2 PID out"=w3340:T9, "Ch1 PID out"=w3341:T9)  [unwired: 7 in]
        n1531 = local write "Ch1 PID gains"(w3341) -> ()
        n1532 = local write "Ch2 PID gains"(w3340) -> ()
        n1533 = local write "Ch3 PID gains"(w3339) -> ()
        n1534 = local write "Ch4 PID gains"(w3339) -> ()
        n1535 = call <vilib>:"Add State(s) to Queue__JKI_lib_State_Machine.vi"("State(s) in (\"\")"=w3347) -> ("States Out"=w3346:string)  [unwired: 14 in]
      }
      frame "---------- USBCAM ----------" {
        # "Template Separator\n(You can make a copy of, or modify, this frame)"
        n1536 = call <vilib>:"Add State(s) to Queue__JKI_lib_State_Machine.vi"("State(s) in (\"\")"=w3352) -> ("States Out"=w3351:string)  [unwired: 14 in]
      }
      frame "USBCAM: StartAndSave" {
        # "Start Camera send user event\n(You can make a copy of, or modify, this frame)"
        n1537 = Unbundle By Name(w3365) -> ("Pathes.DataPath"=w3364:path, "IDs.RunID"=w3362:i8)
        n1538 = Increment(x=w3362) -> (x+1=w3361:i8)
        n1539 = call "USBCAM_FGV.vi"("error in (no error)"=w3366) -> ("error out"=w3370:errorcluster, "Session Out"=w3369:T25)  [unwired: 9 in]
        n1540 = Format Value(format string="Run_%02d", value (0)=w3361) -> (output string=w3360:string)  [unwired: 1 in]
        n1541 = call <vilib>:"IMAQdx Start Acquisition.vi"("error in"=w3370, "Session In"=w3369) -> ("error out"=w3355:errorcluster)  [unwired: 8 in, 1 out]
        n1542 = Build Path(base path=w3364, name or relative path=w3360) -> (appended path=w3356:path)
        n1543 = Create Folder(path (use dialog)=w3356, error in=w3355) -> (created path=w3354:path, error out=w3353:errorcluster)  [unwired: 1 in, 1 out]
        n1544 = Bundle("created path"=w3354, TRUE) -> (w3358:cluster{"created path":path, bool})  [unwired: 1 in]
        n1545 = Generate User Event(priority (normal)=usereventprio."high priority", user event=w3368, event data cluster=w3358, error in=w3353) -> (error out=w3367:errorcluster)  [unwired: 1 out]
        n1546 = call <vilib>:"Add State(s) to Queue__JKI_lib_State_Machine.vi"("State(s) in (\"\")"=w3373) -> ("States Out"=w3372:string)  [unwired: 14 in]
      }
      frame "USBCAM: StartNoSave" {
        # "Start Camera send user event\n(You can make a copy of, or modify, this frame)"
        n1547 = call "USBCAM_FGV.vi"("error in (no error)"=w3380) -> ("error out"=w3384:errorcluster, "Session Out"=w3383:T25)  [unwired: 9 in]
        n1548 = call <vilib>:"IMAQdx Start Acquisition.vi"("error in"=w3384, "Session In"=w3383) -> ("error out"=w3375:errorcluster)  [unwired: 8 in, 1 out]
        n1549 = Bundle(path "", FALSE) -> (w3377:cluster{path, bool})  [unwired: 1 in]
        n1550 = Generate User Event(priority (normal)=usereventprio."high priority", user event=w3382, event data cluster=w3377, error in=w3375) -> (error out=w3381:errorcluster)  [unwired: 1 out]
        n1551 = call <vilib>:"Add State(s) to Queue__JKI_lib_State_Machine.vi"("State(s) in (\"\")"=w3387) -> ("States Out"=w3386:string)  [unwired: 14 in]
      }
      frame "USBCAM: Stop" {
        # "Stop USB Cam\n(You can make a copy of, or modify, this frame)"
        n1552 = call "USBCAM_FGV.vi"("error in (no error)"=w3388) -> ("error out"=w3391:errorcluster, "Session Out"=w3390:T25)  [unwired: 9 in]
        n1553 = call <vilib>:"IMAQdx Stop Acquisition.vi"("error in"=w3391, "Session In"=w3390) -> ("error out"=w3389:errorcluster)  [unwired: 8 in, 1 out]
        n1554 = call <vilib>:"Add State(s) to Queue__JKI_lib_State_Machine.vi"("State(s) in (\"\")"=w3395) -> ("States Out"=w3394:string)  [unwired: 14 in]
      }
      frame "USBCAM: Config" {
        # "Config Camera\n(You can make a copy of, or modify, this frame)"
        n1555 = call "USBCAM_FGV.vi"("error in (no error)"=w3403) -> ("error out"=w3399:errorcluster, "Session Out"=w3400:T25)  [unwired: 9 in]
        n1556 = property class="IMAQdx"(reference=w3400, error in=w3399, "VideoMode"="VideoMode") -> (error out=w3398:errorcluster)  [unwired: 1 out]
        n1557 = call <vilib>:"IMAQdx Configure Acquisition.vi"("error in"=w3398, "Number of Buffers"=u32 5, "Continuous?"=IMAQdx_Acquisition_Mode."Continuous", "Session In"=w3400) -> ("error out"=w3396:errorcluster)  [unwired: 6 in, 1 out]
        n1558 = call <vilib>:"Add State(s) to Queue__JKI_lib_State_Machine.vi"("State(s) in (\"\")"=w3407) -> ("States Out"=w3406:string)  [unwired: 14 in]
      }
      frame "USBCAM: Init" {
        # "Initilize USB camera\n(You can make a copy of, or modify, this frame)"
        n1559 = call <vilib>:"IMAQdx Open Camera.vi"("Camera Control Mode"=IMAQdx_Camera_Control_Mode."Controller", "error in"=w3413, "Session In"=T25 "cam1") -> ("error out"=w3410:errorcluster, "Session Out"=w3411:T25)  [unwired: 7 in]
        n1560 = call "USBCAM_FGV.vi"("error in (no error)"=w3410, "Operation (Read)"=enum16{"Write", "Read"}."Write", "Session In"=w3411) -> ("error out"=w3409:errorcluster)  [unwired: 7 in, 1 out]
        n1561 = call <vilib>:"Add State(s) to Queue__JKI_lib_State_Machine.vi"("State(s) in (\"\")"=w3418) -> ("States Out"=w3417:string)  [unwired: 14 in]
      }
      frame "USBCAM: Close" {
        # "Close Camera\n(You can make a copy of, or modify, this frame)"
        n1562 = call "USBCAM_FGV.vi"("error in (no error)"=w3424, "Operation (Read)"=enum16{"Write", "Read"}."Read") -> ("error out"=w3420:errorcluster, "Session Out"=w3422:T25)  [unwired: 8 in]
        n1563 = call <vilib>:"IMAQdx Unconfigure Acquisition.vi"("error in"=w3420, "Session In"=w3422) -> ("error out"=w3419:errorcluster, "Session Out"=w3421:T25)  [unwired: 8 in]
        n1564 = call <vilib>:"IMAQdx Close Camera.vi"("error in"=w3419, "Session In"=w3421) -> ("error out"=w3425:errorcluster)  [unwired: 9 in]
        n1565 = call <vilib>:"Add State(s) to Queue__JKI_lib_State_Machine.vi"("State(s) in (\"\")"=w3429) -> ("States Out"=w3428:string)  [unwired: 14 in]
      }
      frame "---------- Temp (copy) ----------" {
        # "Template Separator\n(You can make a copy of, or modify, this frame)"
        n1566 = call <vilib>:"Add State(s) to Queue__JKI_lib_State_Machine.vi"("State(s) in (\"\")"=w3434) -> ("States Out"=w3433:string)  [unwired: 14 in]
      }
    }
    n1567 = Not(x=w80) -> (.not. x?=w79:bool)
    n1568 = local write "ML?"(w79) -> ()
    "ML?" <- TRUE ("main loop running?")
  }
  n1569 = while {
    tunnel: w21 -> [w3445]
    shift-right: [w3436] -> _
    shift-left: w23 -> [w3443]
    shift-right: [w3438] -> _
    shift-left: w23 -> [w3437]
    i -> [w3439]
    stop <- w3440 stop-if-true
    # "Data display loop(30Hz)"
    n1570 = Wait on Notification(notifier=w3445, ignore previous (F)=FALSE) -> (notification=w3441:T14, error out=w3440:errorcluster)  [unwired: 2 in, 2 out]
    n1571 = Wait Until Next ms Multiple(millisecond multiple=u32 33) -> ()  [unwired: 1 out]
    n1572 = Tick Count (ms)() -> (millisecond timer value=w3436:u32)
    n1573 = Subtract(x=w3436, y=w3443) -> (x-y=→"display loop timing(ms)":u32)
    n1574 = case shown="No Error" w3440 {
      tunnel: w3441 -> [w3518 _]
      tunnel: w3437 -> [w3490 w3590]
      tunnel: [w3492 w3590] -> w3438
      tunnel: w3436 -> [w3489 _]
      frame No Error {
        w3447 = u32 1 ("Active Plot")
        w3466 = 0 ("index (row)")
        n1575 = Subtract(x=w3489, y=w3490) -> (x-y=w3491:u32)
        n1576 = Unbundle(w3518) -> ("CH1"=w3513:dbl[][], "CH2"=w3511:dbl[][], "CH3"=w3508:dbl[][], "CH4"=w3461:dbl[][], "Gain cluster"=w3467:cluster{"V1":dbl, "V2":dbl, "V3":dbl, "V4":dbl})
        n1577 = Unbundle By Name(w3467) -> ("V1"=w3485:dbl, "V2"=w3483:dbl, "V3"=w3481:dbl, "V4"=w3459:dbl)
        n1578 = Index Array(array=w3513, index (row)=w3466) -> (element=w3497:dbl[])  [unwired: 1 in]
        n1579 = Index Array(array=w3511, index (row)=w3466) -> (element=w3495:dbl[])  [unwired: 1 in]
        n1580 = Index Array(array=w3508, index (row)=w3466) -> (element=w3496:dbl[])  [unwired: 1 in]
        n1581 = Index Array(array=w3461, index (row)=w3466) -> (element=w3465:dbl[])  [unwired: 1 in]
        n1582 = call "RemoveDCBG.vi"("Channel"=enum16{"DC Only", "Ch1", "Ch2", "Ch3", "Ch4"}."Ch4", "WF in"=w3465) -> ("DC"=w3463:dbl, "WF out"=w3452:dbl[])  [unwired: 7 in, 1 out]
        n1583 = Greater?(x=w3491, y=u32 200) -> (0:w3493:bool)
        n1584 = call "CtrlVtoGain.vi"("CtrlV(V)"=w3459, "Channel"=enum16{"Ch1", "Ch2", "Ch3", "Ch4"}."Ch4") -> ("Gain"=w3451:dbl)  [unwired: 8 in, 1 out]
        n1585 = call "CtrlVtoGain.vi"("CtrlV(V)"=w3485, "Channel"=enum16{"Ch1", "Ch2", "Ch3"}."Ch1") -> ("Gain"=w3479:dbl)  [unwired: 8 in, 1 out]
        n1586 = call "RemoveDCBG.vi"("Channel"=enum16{"DC Only", "Ch1", "Ch2", "Ch3"}."Ch1", "WF in"=w3497) -> ("DC"=w3514:dbl, "WF out"=w3486:dbl[])  [unwired: 7 in, 1 out]
        n1587 = call "RemoveDCBG.vi"("Channel"=enum16{"DC Only", "Ch1", "Ch2", "Ch3"}."Ch2", "WF in"=w3495) -> ("DC"=w3510:dbl, "WF out"=w3487:dbl[])  [unwired: 7 in, 1 out]
        n1588 = call "CtrlVtoGain.vi"("CtrlV(V)"=w3483, "Channel"=enum16{"Ch1", "Ch2", "Ch3"}."Ch2") -> ("Gain"=w3474:dbl)  [unwired: 8 in, 1 out]
        n1589 = call "RemoveDCBG.vi"("Channel"=enum16{"DC Only", "Ch1", "Ch2", "Ch3"}."Ch3", "WF in"=w3496) -> ("DC"=w3507:dbl, "WF out"=w3488:dbl[])  [unwired: 7 in, 1 out]
        n1590 = call "CtrlVtoGain.vi"("CtrlV(V)"=w3481, "Channel"=enum16{"Ch1", "Ch2", "Ch3"}."Ch3") -> ("Gain"=w3470:dbl)  [unwired: 8 in, 1 out]
        n1591 = formula code="int32 out = 2;\nif (G<5){\nout = 1;\n}\nif (G>200){\nout = 3;\n}"("G"=w3451) -> ("out"=→"output variable":i32)
        n1592 = Add(x=w3452, y=w3463) -> (x+y=w3462:dbl[])
        n1593 = Less?(x=w3451, y=5.0) -> (x < y?=w3457:bool)
        n1594 = case shown="True" w3493 {
          tunnel: w3486 -> [_ w3547]
          tunnel: w3487 -> [_ w3550]
          tunnel: w3488 -> [_ w3549]
          tunnel: w3489 -> [_ w3565]
          tunnel: [w3529 w3565] -> w3492
          tunnel: w3490 -> [w3529 _]
          tunnel: w3479 -> [_ w3543]
          tunnel: w3474 -> [_ w3542]
          tunnel: w3470 -> [_ w3541]
          tunnel: w3452 -> [_ w3537]
          tunnel: w3451 -> [_ w3534]
          frame False {
          }
          frame True {
            n1595 = call "GetSNR(SubVI).vi"("Waveform"=w3547) -> ("SNR"=→"SNR1":dbl)  [unwired: 10 in]
            n1596 = Array Size(array=w3547) -> (size(s)=w3548:i32)
            n1597 = call "GetSNR(SubVI).vi"("Waveform"=w3550) -> ("SNR"=→"SNR2":dbl)  [unwired: 10 in]
            n1598 = call "GetSNR(SubVI).vi"("Waveform"=w3549) -> ("SNR"=→"SNR3":dbl)  [unwired: 10 in]
            n1599 = call "GetSNR(SubVI).vi"("Waveform"=w3537) -> ("SNR"=→"SNR4":dbl)  [unwired: 10 in]
            n1600 = global read "GlobalVariables.vi" "BG Idx2"() -> (w3536:i32)
            n1601 = Subtract(x=w3548, y=w3536) -> (x-y=w3535:i32)
            n1602 = Array Subset(array=w3547, index=w3536, length=w3535) -> (w3554:dbl[])
            n1603 = Array Subset(array=w3550, index=w3536, length=w3535) -> (w3556:dbl[])
            n1604 = Array Subset(array=w3549, index=w3536, length=w3535) -> (w3558:dbl[])
            n1605 = Array Subset(array=w3537, index=w3536, length=w3535) -> (w3538:dbl[])
            n1606 = Add Array Elements(numeric array=w3554) -> (sum=w3555:dbl)
            n1607 = Add Array Elements(numeric array=w3556) -> (sum=w3557:dbl)
            n1608 = Add Array Elements(numeric array=w3558) -> (sum=w3559:dbl)
            n1609 = Add Array Elements(numeric array=w3538) -> (sum=w3539:dbl)
            n1610 = Divide(x=w3555, y=w3543) -> (x/y=w3560:dbl)
            n1611 = Divide(x=w3557, y=w3542) -> (x/y=w3561:dbl)
            n1612 = Divide(x=w3559, y=w3541) -> (x/y=w3562:dbl)
            n1613 = Divide(x=w3539, y=w3534) -> (x/y=w3533:dbl)
            n1614 = Build Array(w3560, w3561, w3562, w3533) -> (w3563:dbl[])
            n1615 = Add Array Elements(numeric array=w3563) -> (sum=w3564:dbl)
            n1616 = Divide(x=w3563, y=w3564) -> (x/y=w3532:dbl[])
            n1617 = Index Array(array=w3532, index=2) -> (element=→"IntR3":dbl)
            n1618 = Index Array(array=w3532, index=1) -> (element=→"IntR2":dbl)
            n1619 = Index Array(array=w3532, index=0) -> (element=→"IntR1":dbl)
            n1620 = Index Array(array=w3532, index=3) -> (element=→"IntR4":dbl)
          }
        }
        n1621 = Add(x=w3486, y=w3514) -> (x+y=w3512:dbl[])
        n1622 = Add(x=w3487, y=w3510) -> (x+y=w3509:dbl[])
        n1623 = Add(x=w3488, y=w3507) -> (x+y=w3506:dbl[])
        n1624 = Less?(x=w3479, y=5.0 ("x")) -> (x < y?=w3477:bool)
        n1625 = Less?(x=w3474, y=5.0 ("x")) -> (x < y?=w3473:bool)
        n1626 = Less?(x=w3470, y=5.0 ("x")) -> (x < y?=w3469:bool)
        n1627 = case shown="False" w3469 {
          tunnel: [u32 16448250 ("Plot.Plot Color") u32 16711680 ("Plot.Plot Color")] -> w3468
          frame False {
          }
          frame True {
          }
        }
        n1628 = case shown="True" "Show BG removed?" {
          tunnel: w3513 -> [w3572 w3588]
          tunnel: w3512 -> [_ w3578]
          tunnel: [w3572 w3587] -> w3505
          tunnel: w3511 -> [w3571 w3586]
          tunnel: [w3571 w3585] -> w3449
          tunnel: w3509 -> [_ w3574]
          tunnel: w3508 -> [w3570 w3584]
          tunnel: [w3570 w3583] -> w3500
          tunnel: w3506 -> [_ w3579]
          tunnel: [w3569 w3582] -> w3456
          tunnel: w3462 -> [_ w3576]
          tunnel: w3461 -> [w3569 w3581]
          frame False {
          }
          frame True {
            n1629 = Insert Into Array(array=w3584, index (row)=1, new element=w3579) -> (w3583:dbl[][])  [unwired: 1 in]
            n1630 = Insert Into Array(array=w3588, index (row)=1, new element=w3578) -> (w3587:dbl[][])  [unwired: 1 in]
            n1631 = Insert Into Array(array=w3586, index (row)=1, new element=w3574) -> (w3585:dbl[][])  [unwired: 1 in]
            n1632 = Insert Into Array(array=w3581, index (row)=1, new element=w3576) -> (w3582:dbl[][])  [unwired: 1 in]
          }
        }
        "Channel 1" <- w3505
        "Channel 2" <- w3449
        "Channel 3" <- w3500
        "Channel 4" <- w3456
        n1633 = case shown="False" w3477 {
          tunnel: [u32 16448250 ("Plot.Plot Color") u32 16711680 ("Plot.Plot Color")] -> w3476
          frame False {
          }
          frame True {
          }
        }
        n1634 = case shown="False" w3473 {
          tunnel: [u32 16448250 ("Plot.Plot Color") u32 16711680 ("Plot.Plot Color")] -> w3472
          frame False {
          }
          frame True {
          }
        }
        n1635 = case shown="False" w3457 {
          tunnel: [u32 16448250 ("Plot.Plot Color") u32 16711680 ("Plot.Plot Color")] -> w3453
          frame False {
          }
          frame True {
          }
        }
        n1636 = case shown="False" "Show BG removed?" {
          tunnel: [u32 16744703 ("Plot.Plot Color") u32 16741120 ("Plot.Plot Color")] -> w3446
          frame False {
          }
          frame True {
          }
        }
        n1637 = property on="Channel 1" class="WFGraph (strict)"("Active Plot"=w3447, "Plot.Plot Color"=w3446, "Plot.Line Style"=u8 1, "Plot.Line Width"=u8 2, "BG Color"=w3476) -> ()  [unwired: 2 in, 2 out]
        n1638 = property on="Channel 2" class="WFGraph (strict)"("Active Plot"=w3447, "Plot.Plot Color"=w3446, "Plot.Line Style"=u8 1, "Plot.Line Width"=u8 2, "BG Color"=w3472) -> ()  [unwired: 2 in, 2 out]
        n1639 = property on="Channel 4" class="WFGraph (strict)"("Active Plot"=w3447, "Plot.Plot Color"=w3446, "Plot.Line Style"=u8 1, "Plot.Line Width"=u8 2, "BG Color"=w3453) -> ()  [unwired: 2 in, 2 out]
        n1640 = property on="Channel 3" class="WFGraph (strict)"("Active Plot"=w3447, "Plot.Plot Color"=w3446, "Plot.Line Style"=u8 1, "Plot.Line Width"=u8 2, "BG Color"=w3468) -> ()  [unwired: 2 in, 2 out]
      }
      frame Error {
        w3589 = u32 16448250 ("Plot Area:Colors:BG Color")
        n1641 = property on="Channel 1" class="WFGraph (strict)"("BG Color"=w3589) -> ()  [unwired: 2 in, 2 out]
        n1642 = property on="Channel 2" class="WFGraph (strict)"("BG Color"=w3589) -> ()  [unwired: 2 in, 2 out]
        n1643 = property on="Channel 3" class="WFGraph (strict)"("BG Color"=w3589) -> ()  [unwired: 2 in, 2 out]
      }
    }
    "DisplayLoop" <- w3439
  }
  n1644 = disable-structure "Diagram Disable Structure" shown="Disabled" {
    frame Disabled {
      w3591 = T51 {"Horizontal"=500, "Vertical"=100}  # Top Left Corner
      n1645 = Control Help Window(0:w3591, 1:TRUE ("Show")) -> ()
      n1646 = call <vilib>:"TDMS - File Viewer.vi"() -> ()  [unwired: 6 in, 2 out]
    }
    frame Enabled {
    }
  }
  n1647 = while {
    tunnel: w64 -> [w3605]
    tunnel: w54 -> [w3604]
    tunnel: [w3603] -> w62
    tunnel: w25 -> [w3602]
    tunnel: [w3601] -> w58
    tunnel: w43 -> [w3599]
    tunnel: w4 -> [w3598]
    tunnel: w40 -> [w3593]
    stop <- w3596 stop-if-true
    # "acquire data and send it to processing loop"
    # "Data Aquisition Loop"
    n1648 = event shown="[1] <Start digitizer>: User Event" {
      selector: w3604 -> [_ _]
      dyn-events: [_ _] -> w3603
      timeout: 20 -> [_ _]
      tunnel: w3605 -> [w3611 w3621]
      tunnel: [w3606 _] -> w3596
      tunnel: w3602 -> [w3610 w3628]
      tunnel: [w3610 w3627] -> w3601
      tunnel: w3599 -> [_ w3625]
      tunnel: w3598 -> [w3609 w3620]
      tunnel: w3593 -> [_ w3618]
      event Timeout {
        # "use queue to stop data loop\nwhen queue ref is released, error will stop this loop"
        n1649 = event-data() -> ()  [unwired: 1 in, 3 out]
        n1650 = Get Queue Status(queue=w3611) -> (error out=w3608:errorcluster)  [unwired: 2 in, 7 out]
        n1651 = Get Queue Status(queue=w3609) -> (error out=w3607:errorcluster)  [unwired: 2 in, 7 out]
        n1652 = Merge Errors(w3608, w3607) -> (w3606:errorcluster)
      }
      event User Event {
        w3626 = enum16{"Write", "Read"}."Read" ("Operation")
        n1653 = event-data() -> ("Time"=→"RunStartTime":u32)  [unwired: 1 in, 3 out]
        n1654 = call "FLImDAQ_FGV.vi"() -> ("Read data"=w3623:T7)  [unwired: 10 in, 1 out]
        n1655 = call "Digitizer1_FGV.vi"("Operation (Read)"=w3626) -> ("Read data"=w3617:refnum<k15>)  [unwired: 9 in, 1 out]
        n1656 = call "Digitizer2_FGV.vi"("Operation (Read)"=w3626) -> ("Read data"=w3624:refnum<k15>)  [unwired: 9 in, 1 out]
        n1657 = Unbundle By Name(w3623) -> ("Waveform to Avg"=w3622:i16)
        n1658 = property on="Property Node" class="niScope"(reference=w3617) -> (reference out=w3616:refnum<k15>, "Vertical Range"=w3615:dbl, "Vertical Offset"=w3614:dbl)  [unwired: 1 in, 1 out]
        n1659 = Tick Count (ms)() -> (millisecond timer value=w3613:u32)
        n1660 = while {
          tunnel: w3628 -> [w3691]
          tunnel: [w3690] -> w3627
          tunnel: w3624 -> [w3684]
          tunnel: w3616 -> [w3683]
          tunnel: w3625 -> [w3682]
          shift-right: [w3651] -> _
          shift-left: u32 0 ("millisecond timer value") -> [w3676]
          tunnel: w3622 -> [w3631]
          tunnel: w3621 -> [w3673]
          tunnel: w3620 -> [w3671]
          tunnel: w3618 -> [w3664]
          tunnel: w3615 -> [w3661]
          tunnel: w3614 -> [w3662]
          shift-right: [w3656] -> _
          shift-left: w3613 -> [w3655]
          i -> [w3630]
          stop <- w3654 stop-if-true
          w3644 = enum16{"write", "read"}."read" ("action")
          w3677 = 65536
          # "enqueue V"
          # "enqueue ch3 data"
          # "enqueue ch1&2 data"
          # "acquire ch3"
          # "acquire ch1&2"
          # "send data for processing"
          n1661 = Multiply(x=w3631, y=w3630) -> (x*y=w3641:i32)
          "Fetch Record #" <- w3641
          n1662 = property on="Property Node" class="niScope"(reference=w3683, "Fetch Record Number"=w3641) -> (reference out=w3695:refnum<k15>, error out=w3694:errorcluster, "Records Done"=w3663:i32)  [unwired: 1 in]
          n1663 = Equal To 0?(x=w3630) -> (x = 0?=w3629:bool)
          n1664 = case shown="True" w3629 {
            frame False {
            }
            frame True {
              n1665 = call "High Resolution Timer Helper.vi"() -> ("Current Time"=→"FLIm 1st point time":dbl)  [unwired: 9 in, 2 out]
            }
          }
          n1666 = Subtract(x=w3663, y=w3641) -> (x-y=→"Record Backlog":i32)
          n1667 = call-poly <instrlib>:"niScope Fetch (poly).vi"("timeout"=1.0, "error in"=w3694, "channels"="0,1", "instrument handle"=w3695) -> ("error out"=w3638:errorcluster, "wfm"=w3639:i16[][], "wfm info"=w3660:T52)  [unwired: 4 in, 1 out]
          n1668 = property on="Property Node" class="niScope"(reference=w3684, "Fetch Record Number"=w3641) -> (reference out=w3688:refnum<k15>, error out=w3685:errorcluster, "Records Done"=w3642:i32)  [unwired: 1 in]
          n1669 = Divide(x=w3639, y=w3677) -> (x/y=w3650:dbl[][])
          n1670 = Tick Count (ms)() -> (millisecond timer value=w3651:u32)
          n1671 = Subtract(x=w3642, y=w3641) -> (x-y=→"Record Backlog 2":i32)
          n1672 = Subtract(x=w3651, y=w3676) -> (x-y=→"Aquisition loop timing(ms)":u32)
          n1673 = Subtract(x=w3651, y=w3655) -> (x-y=w3659:u32)
          n1674 = Multiply(x=w3650, y=w3661) -> (x*y=w3681:dbl[][])
          n1675 = call-poly <instrlib>:"niScope Fetch (poly).vi"("timeout"=0.25, "error in"=w3685, "channels"="0,1", "instrument handle"=w3688) -> ("error out"=w3637:errorcluster, "wfm"=w3678:i16[][])  [unwired: 4 in, 2 out]
          n1676 = Greater?(x=w3659, y=u32 1000) -> (0:w3657:bool)
          n1677 = Add(x=w3681, y=w3662) -> (x+y=w3672:dbl[][])
          n1678 = case shown="True" w3657 {
            tunnel: w3660 -> [_ w3705]
            tunnel: w3651 -> [_ w3704]
            tunnel: [w3698 w3704] -> w3656
            tunnel: w3655 -> [w3698 _]
            tunnel: [errorcluster {"status"=FALSE, "code"=0, "source"=""} ("error constant") w3701] -> w3652
            frame False {
            }
            frame True {
              # "[Covers: REQ29]"
              n1679 = call "CheckFrequency(SubVI).vi"("wfm info"=w3705) -> ("f (Hz)"=w3703:dbl)  [unwired: 10 in]
              "Laser f (Hz)" <- w3703
              n1680 = local read "Laser Rep Rate"() -> (w3700:dbl)
              n1681 = Increment(x=w3700) -> (x+1=w3699:dbl)
              n1682 = Greater?(x=w3703, y=w3699) -> (0:w3702:bool)
              n1683 = case shown="True" w3702 {
                tunnel: [errorcluster {"status"=FALSE, "code"=0, "source"=""} ("error constant") errorcluster {"status"=TRUE, "code"=0, "source"=""} ("error constant")] -> w3701
                frame False {
                }
                frame True {
                }
              }
            }
          }
          n1684 = Divide(x=w3678, y=w3677) -> (x/y=w3680:dbl[][])
          n1685 = Enqueue Element(queue=w3673, element=w3672, error in (no error)=w3638) -> (error out=w3636:errorcluster)  [unwired: 1 in, 2 out]
          n1686 = Multiply(x=w3680, y=w3661) -> (x*y=w3679:dbl[][])
          n1687 = Add(x=w3679, y=w3662) -> (x+y=w3670:dbl[][])
          n1688 = Enqueue Element(queue=w3671, element=w3670, error in (no error)=w3637) -> (error out=w3635:errorcluster)  [unwired: 1 in, 2 out]
          n1689 = Increment(x=w3630) -> (x+1=w3633:i32)
          n1690 = Merge Errors(w3636, w3635) -> (w3634:errorcluster)
          n1691 = call "V1FGV.vi"("Error In"=w3634, "action (write)"=w3644) -> ("Error Out"=w3668:errorcluster, "V1 out"=w3666:dbl)  [unwired: 8 in]
          n1692 = call "V2FGV.vi"("Error In"=w3668, "action(write)"=w3644) -> ("Error Out"=w3667:errorcluster, "V2 out"=w3665:dbl)  [unwired: 8 in]
          n1693 = Multiply(x=w3633, y=w3631) -> (x*y=w3632:i32)
          n1694 = call "V3FGV.vi"("Error In"=w3667, "action(write)"=w3644) -> ("Error Out"=w3647:errorcluster, "V3 out"=w3646:dbl)  [unwired: 8 in]
          n1695 = call "V4FGV.vi"("Error In"=w3647, "action(write)"=w3644, "V3 in"=w3646) -> ("Error Out"=w3645:errorcluster, "V3 out"=w3643:dbl)  [unwired: 7 in]
          n1696 = Bundle("V1 out"=w3666, "V2 out"=w3665, "V3 out"=w3646, "V3 out"=w3643) -> (w3649:T53)  [unwired: 1 in]
          n1697 = Bundle(w3632, w3672, w3670, w3649) -> (w3674:T54)  [unwired: 1 in]
          n1698 = Enqueue Element(queue=w3664, element=w3649, error in (no error)=w3645) -> (error out=w3648:errorcluster)  [unwired: 1 in, 2 out]
          n1699 = Send Notification(notification=w3674, notifier=w3691, error in (no error)=w3648) -> (notifier out=w3690:refnum<notifier>, error out=w3653:errorcluster)
          n1700 = Merge Errors(w3652, w3653) -> (w3669:errorcluster)
          n1701 = case shown="Error .." w3669 {
            selector: w3669 -> [w3708 w3709]
            tunnel: w3682 -> [_ w3712]
            tunnel: [w3708 w3709] -> w3654
            frame No Error {
            }
            frame Error {
              # "Send user event to signal aquisition has stoped"
              n1702 = Generate User Event(priority (normal)=usereventprio."high priority", user event=w3712, event data cluster=TRUE ("event data")) -> ()  [unwired: 1 in, 2 out]
            }
          }
          "aquisition loop Error Out" <- w3654
          "Auisition Loop idx" <- w3630
        }
      }
    }
    n1703 = Unbundle By Name(w3596) -> ("status"=w3595:bool)
    n1704 = Not(x=w3595) -> (.not. x?=w3594:bool)
    n1705 = local write "Aq Loop?"(w3594) -> ()
    "Aq Loop?" <- TRUE ("Aq L?")
  }
  n1706 = while {
    tunnel: w25 -> [w3744]
    tunnel: w21 -> [w3737]
    tunnel: [w3736] -> w24
    shift-right: [w3728] -> _
    shift-left: _ -> [w3729]
    stop <- w3726 stop-if-true
    # "Read data from notifier and deconvolve it and send to Aiming Beam computer"
    n1707 = Wait on Notification(notifier=w3744, ignore previous (F)=FALSE) -> (notification=w3743:T15, error out=w3714:errorcluster)  [unwired: 2 in, 2 out]
    n1708 = flat-sequence {
      tunnel: [w3745] -> w3728
      tunnel: w3714 -> [_]
      frame #0 {
        n1709 = call <vilib>:"High Resolution Relative Seconds.vi"() -> ("relative seconds"=w3745:dbl)
      }
    }
    n1710 = Unbundle(w3743) -> ("CH1&2"=w3742:dbl[][], "CH3"=w3741:dbl[][], "V cluster"=w3732:cluster{"V1":dbl, "V2":dbl, "V3":dbl, "V4":dbl})  [unwired: 1 out]
    n1711 = call "SeperateChanData.vi"("Input (Ch1&2)"=w3742) -> ("Ch1"=w3724:dbl[][], "Ch2"=w3722:dbl[][])
    n1712 = call "SeperateChanData.vi"("Input (Ch1&2)"=w3741) -> ("Ch1"=w3720:dbl[][], "Ch2"=w3718:dbl[][])
    n1713 = Subtract(x=w3728, y=w3729) -> (x-y=w3731:dbl)
    n1714 = call "AvgArrayTimeCritical.vi"("2D array"=w3724) -> ("1D Avg"=w3723:dbl[])  [unwired: 10 in]
    n1715 = call "AvgArrayTimeCritical.vi"("2D array"=w3722) -> ("1D Avg"=w3721:dbl[])  [unwired: 10 in]
    n1716 = call "AvgArrayTimeCritical.vi"("2D array"=w3720) -> ("1D Avg"=w3719:dbl[])  [unwired: 10 in]
    n1717 = call "AvgArrayTimeCritical.vi"("2D array"=w3718) -> ("1D Avg"=w3717:dbl[])  [unwired: 10 in]
    n1718 = Multiply(x=w3731, y=1000.0) -> (x*y=→"Decon Loop timing (ms)" →"Waveform Chart":dbl)
    n1719 = case shown="\"Ch1\"" "Radio Buttons" {
      selector: "Radio Buttons" -> [_ w3758 w3772 w3787 w3804]
      tunnel: w3723 -> [w3755 w3766 w3778 w3792 w3808]
      tunnel: w3721 -> [w3753 w3763 w3780 w3790 w3806]
      tunnel: w3719 -> [w3751 w3761 w3775 w3795 w3798]
      tunnel: FALSE -> [_ w3769 w3783 w3797 w3811]
      tunnel: w3714 -> [w3749 w3768 w3782 w3786 w3803]
      tunnel: [w3749 w3767 w3781 w3796 w3810] -> w3726
      tunnel: [w3754 w3764 w3776 w3791 w3807] -> w3735
      tunnel: [w3752 w3762 w3777 w3789 w3805] -> w3734
      tunnel: [w3750 w3760 w3774 w3793 w3799] -> w3733
      tunnel: [0.0 ("lifetime (ns)") w3759 w3773 w3788 w3802] -> w3713
      tunnel: w3717 -> [w3747 w3757 w3771 w3785 w3801]
      tunnel: [w3746 w3756 w3770 w3784 w3800] -> w3716
      frame "No Selection", Default {
        n1720 = Build Array(w3755) -> (w3754:dbl[][])
        n1721 = Build Array(w3753) -> (w3752:dbl[][])
        n1722 = Build Array(w3751) -> (w3750:dbl[][])
        n1723 = Build Array(w3747) -> (w3746:dbl[][])
      }
      frame "Ch1" {
        n1724 = call "Deconvolution.vi"("DeconChannel"=w3758, "iRF align"=w3769, "error in (no error)"=w3768, "Waveform"=w3766) -> ("error out"=w3767:errorcluster, "lifetime (ns)"=w3759:dbl, "Fitting"=w3765:dbl[])  [unwired: 5 in]
        "Lifetime 1" <- w3759
        n1725 = Build Array(w3766, w3765) -> (w3764:dbl[][])
        n1726 = Build Array(w3763) -> (w3762:dbl[][])
        n1727 = Build Array(w3761) -> (w3760:dbl[][])
        n1728 = Build Array(w3757) -> (w3756:dbl[][])
      }
      frame "Ch2" {
        n1729 = call "Deconvolution.vi"("DeconChannel"=w3772, "iRF align"=w3783, "error in (no error)"=w3782, "Waveform"=w3780) -> ("error out"=w3781:errorcluster, "lifetime (ns)"=w3773:dbl, "Fitting"=w3779:dbl[])  [unwired: 5 in]
        "Lifetime 2" <- w3773
        n1730 = Build Array(w3778) -> (w3776:dbl[][])
        n1731 = Build Array(w3780, w3779) -> (w3777:dbl[][])
        n1732 = Build Array(w3775) -> (w3774:dbl[][])
        n1733 = Build Array(w3771) -> (w3770:dbl[][])
      }
      frame "Ch3" {
        n1734 = call "Deconvolution.vi"("DeconChannel"=w3787, "iRF align"=w3797, "error in (no error)"=w3786, "Waveform"=w3795) -> ("error out"=w3796:errorcluster, "lifetime (ns)"=w3788:dbl, "Fitting"=w3794:dbl[])  [unwired: 5 in]
        "Lifetime 3" <- w3788
        n1735 = Build Array(w3792) -> (w3791:dbl[][])
        n1736 = Build Array(w3790) -> (w3789:dbl[][])
        n1737 = Build Array(w3795, w3794) -> (w3793:dbl[][])
        n1738 = Build Array(w3785) -> (w3784:dbl[][])
      }
      frame "Ch4" {
        n1739 = call "Deconvolution.vi"("DeconChannel"=w3804, "iRF align"=w3811, "error in (no error)"=w3803, "Waveform"=w3801) -> ("error out"=w3810:errorcluster, "lifetime (ns)"=w3802:dbl, "Fitting"=w3809:dbl[])  [unwired: 5 in]
        "Lifetime 4" <- w3802
        n1740 = Build Array(w3808) -> (w3807:dbl[][])
        n1741 = Build Array(w3806) -> (w3805:dbl[][])
        n1742 = Build Array(w3801, w3809) -> (w3800:dbl[][])
        n1743 = Build Array(w3798) -> (w3799:dbl[][])
      }
    }
    "Lifetime (ns)" <- w3713
    n1744 = Bundle(w3735, w3734, w3733, w3716, "V cluster"=w3732) -> (w3738:T55)  [unwired: 1 in]
    n1745 = Send Notification(notification=w3738, notifier=w3737, error in (no error)=w3726) -> (notifier out=w3736:refnum<notifier>, error out=→"decon error out":errorcluster)
  }
  n1746 = while {
    tunnel: w5 -> [w3814]
    tunnel: w4 -> [w3813]
    tunnel: [w3812] -> w2
    stop <- w3815 stop-if-true
    n1747 = event shown="[1] <startCam>: User Event" {
      selector: w3814 -> [_ _]
      dyn-events: [_ _] -> w3812
      timeout: 30 -> [_ _]
      tunnel: [w3818 _] -> w3815
      tunnel: w3813 -> [w3817 _]
      event Timeout {
        # "if queue is destoried, stop cam loop"
        n1748 = event-data() -> ()  [unwired: 1 in, 3 out]
        n1749 = Get Queue Status(queue=w3817) -> (error out=w3818:errorcluster)  [unwired: 2 in, 7 out]
      }
      event User Event {
        n1750 = event-data() -> ("savePath"=w3823:path, "saveData?"=w3824:bool)  [unwired: 1 in, 4 out]
        n1751 = call "USBCAM_FGV.vi"() -> ("error out"=w3827:errorcluster, "Session Out"=w3828:T25)  [unwired: 10 in]
        n1752 = call "IMAQ Create"("Image Name"="Acquire Most Recent Image") -> ("New Image"=w3825:T1, "error out"=w3822:errorcluster)  [unwired: 3 in, 1 out]
        n1753 = while {
          tunnel: w3828 -> [w3850]
          shift-right: [w3840] -> w3820
          shift-left: w3827 -> [w3849]
          tunnel: w3825 -> [w3847]
          tunnel: [w3844] -> w3819 mode=indexing
          tunnel: w3824 -> [w3843]
          tunnel: w3823 -> [w3842]
          tunnel: [w3838] -> w3821
          i -> [w3839]
          stop <- w3841 stop-if-true
          n1754 = call <vilib>:"IMAQdx Get Image2.vi"("Timeout (ms)"=5000, "Buffer Number Mode (Next)"=IMAQdx_Buffer_Number_Mode."Last New", "error in"=w3849, "Image In"=w3847, "Session In"=w3850) -> ("error out"=w3841:errorcluster, "Buffer Number Out"=w3846:u32, "Image Out"=w3838:T1)  [unwired: 3 in, 1 out]
          "Image 2" <- w3838
          n1755 = call <vilib>:"Calculate Frames per Second.vi"("Buffer Number"=w3846) -> ("Acquired Frames/s"=→"Acquired Frames/s":dbl)  [unwired: 8 in, 2 out]
          n1756 = call "High Resolution Timer Helper.vi"("error in (no error)"=w3841) -> ("error out"=w3837:errorcluster, "Current Time"=w3844:dbl)  [unwired: 8 in, 1 out]
          n1757 = case shown="True" w3843 {
            tunnel: w3838 -> [_ w3864]
            tunnel: w3842 -> [_ w3862]
            tunnel: w3837 -> [w3852 w3858]
            tunnel: [w3852 w3853] -> w3840
            tunnel: w3839 -> [_ w3861]
            frame False {
            }
            frame True {
              n1758 = Format Into String(format string="Image %04d.png", w3861) -> (resulting string=w3863:string)  [unwired: 2 in, 1 out]
              n1759 = call "High Resolution Timer Helper.vi"("error in (no error)"=w3858) -> ("error out"=w3854:errorcluster, "Current Time"=w3856:dbl)  [unwired: 8 in, 1 out]
              n1760 = Build Path(base path=w3862, name or relative path=w3863) -> (appended path=w3859:path)
              n1761 = call-poly "IMAQ Write File 2"("error in (no error)"=w3854, "File Path"=w3859, "Image"=w3864) -> ("error out"=w3857:errorcluster)  [unwired: 7 in, 1 out]
              n1762 = call "High Resolution Timer Helper.vi"("error in (no error)"=w3857, "Previous Time"=w3856) -> ("error out"=w3853:errorcluster, "Time Difference (ms)"=→"PNG write time (ms)":dbl)  [unwired: 7 in, 1 out]
            }
          }
        }
        "Cam error out" <- w3820
        n1763 = case shown="True" w3824 {
          tunnel: w3823 -> [_ w3835]
          tunnel: w3827 -> [_ w3832]
          tunnel: w3819 -> [_ w3831]
          frame False {
          }
          frame True {
            n1764 = local read "FLIm 1st point time"() -> (w3829:dbl)
            n1765 = Subtract(x=w3831, y=w3829) -> (x-y=w3830:dbl[])
            n1766 = Build Path(base path=w3835, name or relative path="TimeSych.txt") -> (appended path=w3833:path)
            n1767 = call-poly <vilib>:"Write Delimited Spreadsheet.vi"("file path (dialog if empty)"=w3833, "format (%.3f)"="%.5f", "1D data"=w3830, "error in (no error)"=w3832) -> ()  [unwired: 10 in, 2 out]
          }
        }
        n1768 = call "Imaq Dispose"("Image"=w3821, "error in (no error)"=w3822) -> ()  [unwired: 4 in, 1 out]
      }
    }
  }
  n1769 = while {
    tunnel: w25 -> [w3912]
    shift-right: [w3875] -> _
    shift-left: _ -> [w3908]
    tunnel: [w3866] -> w9 mode=indexing
    i -> [w3892]
    stop <- w3872 stop-if-true
    # "Channel 3"
    # "Channel 2"
    # "Channel 1"
    # "use FGV for gain value"
    # "stop on error"
    # "Gain adjustment and Data processing"
    n1770 = Tick Count (ms)() -> (millisecond timer value=w3875:u32)
    n1771 = Wait on Notification(notifier=w3912, ignore previous (F)=TRUE) -> (notification=w3886:T15, error out=w3865:errorcluster)  [unwired: 2 in, 2 out]
    n1772 = Subtract(x=w3875, y=w3908) -> (x-y=→"PID loop timing(ms)":u32)
    n1773 = Unbundle(w3886) -> ("CH1&2"=w3902:dbl[][], "CH3"=w3901:dbl[][])  [unwired: 2 out]
    n1774 = call "SeperateChanData.vi"("Input (Ch1&2)"=w3902) -> ("Ch1"=w3897:dbl[][], "Ch2"=w3895:dbl[][])
    n1775 = call "SeperateChanData.vi"("Input (Ch1&2)"=w3901) -> ("Ch1"=w3891:dbl[][], "Ch2"=w3884:dbl[][])
    n1776 = call "AvgArrayTimeCritical.vi"("2D array"=w3897) -> ("1D Avg"=w3896:dbl[])  [unwired: 10 in]
    n1777 = call "AvgArrayTimeCritical.vi"("2D array"=w3895) -> ("1D Avg"=w3906:dbl[])  [unwired: 10 in]
    n1778 = call "AvgArrayTimeCritical.vi"("2D array"=w3891) -> ("1D Avg"=w3903:dbl[])  [unwired: 10 in]
    n1779 = call "AvgArrayTimeCritical.vi"("2D array"=w3884) -> ("1D Avg"=w3883:dbl[])  [unwired: 10 in]
    n1780 = Array Max & Min(array=w3896) -> (max value=w3894:dbl)  [unwired: 3 out]
    n1781 = Array Max & Min(array=w3906) -> (max value=w3893:dbl)  [unwired: 3 out]
    n1782 = Array Max & Min(array=w3903) -> (max value=w3876:dbl)  [unwired: 3 out]
    n1783 = Array Max & Min(array=w3883) -> (max value=w3881:dbl)  [unwired: 3 out]
    n1784 = local read "Auto gain ch4"() -> (w3882:bool)
    n1785 = local read "Auto gain ch1"() -> (w3900:bool)
    n1786 = local read "Auto gain ch2"() -> (w3899:bool)
    n1787 = local read "Auto gain ch3"() -> (w3898:bool)
    n1788 = case shown="True" w3882 {
      tunnel: w3881 -> [_ w3959]
      tunnel: "V target(1.0)" -> [_ w3957]
      tunnel: [FALSE w3954] -> w3879
      tunnel: [0.0 ("CtrlV") w3949] -> w3880
      frame False {
        # "Manual control"
      }
      frame True {
        # "PID control"
        n1789 = global read "GlobalVariables.vi" "Ch4GainLim(Log)"() -> (w3960:cluster{"GainMax":dbl, "GainMin":dbl})
        n1790 = call-poly <vilib>:"PID.vi"("output range"=w3960, "PID gains"="Ch4 PID gains", "process variable"=w3959, "setpoint"=w3957) -> ("output"=w3958:dbl)  [unwired: 6 in, 1 out]
        n1791 = Power Of 10(x=w3958) -> (10^x=w3950:dbl)
        "Gain4" <- w3950
        n1792 = call "V4FGV.vi"("action(write)"=enum16{"write", "read"}."read") -> ("Error Out"=w3953:errorcluster, "V3 out"=w3955:dbl)  [unwired: 9 in]
        n1793 = call "GainToCtrlV.vi"("Gain"=w3950, "Channel"=enum16{"Ch1", "Ch2", "Ch3", "Ch4"}."Ch4") -> ("CtrlV"=w3949:dbl)  [unwired: 8 in, 1 out]
        n1794 = call "V4FGV.vi"("Error In"=w3953, "V3 in"=w3949) -> ()  [unwired: 8 in, 2 out]
        n1795 = local write "V 4"(w3949) -> ()
        n1796 = Not Equal?(x=w3949, y=w3955) -> (x != y?=w3954:bool)
      }
    }
    n1797 = case shown="True" w3900 {
      tunnel: "V target(1.0)" -> [_ w3974]
      tunnel: w3894 -> [_ w3971]
      tunnel: [0.0 ("CtrlV") w3963] -> w3873
      tunnel: [FALSE w3965] -> w3890
      frame False {
        # "Manual control"
      }
      frame True {
        # "PID control"
        n1798 = global read "GlobalVariables.vi" "Ch1GainLim(Log)"() -> (w3970:cluster{"GainMax":dbl, "GainMin":dbl})
        n1799 = call-poly <vilib>:"PID.vi"("output range"=w3970, "PID gains"="Ch1 PID gains", "process variable"=w3971, "setpoint"=w3974) -> ("output"=w3969:dbl)  [unwired: 6 in, 1 out]
        n1800 = Power Of 10(x=w3969) -> (10^x=w3968:dbl)
        "Gain1" <- w3968
        n1801 = call "V1FGV.vi"("action (write)"=enum16{"write", "read"}."read") -> ("Error Out"=w3964:errorcluster, "V1 out"=w3966:dbl)  [unwired: 9 in]
        n1802 = call "GainToCtrlV.vi"("Gain"=w3968, "Channel"=enum16{"Ch1", "Ch2", "Ch3"}."Ch1") -> ("CtrlV"=w3963:dbl)  [unwired: 8 in, 1 out]
        n1803 = local write "V 1"(w3963) -> ()
        n1804 = call "V1FGV.vi"("Error In"=w3964, "V1 in"=w3963) -> ()  [unwired: 8 in, 2 out]
        n1805 = Not Equal?(x=w3963, y=w3966) -> (x != y?=w3965:bool)
      }
    }
    n1806 = case shown="True" w3899 {
      tunnel: w3893 -> [_ w4001]
      tunnel: "V target(1.0)" -> [_ w4002]
      tunnel: [FALSE w3995] -> w3889
      tunnel: [0.0 ("CtrlV") w3991] -> w3885
      frame False {
        # "Manual control"
      }
      frame True {
        # "PID control"
        n1807 = global read "GlobalVariables.vi" "Ch2GainLim(Log)"() -> (w3999:cluster{"GainMax":dbl, "GainMin":dbl})
        n1808 = call-poly <vilib>:"PID.vi"("output range"=w3999, "PID gains"="Ch2 PID gains", "process variable"=w4001, "setpoint"=w4002) -> ("output"=w3998:dbl)  [unwired: 6 in, 1 out]
        n1809 = Power Of 10(x=w3998) -> (10^x=w3996:dbl)
        "Gain2" <- w3996
        n1810 = call "V2FGV.vi"("action(write)"=enum16{"write", "read"}."read") -> ("Error Out"=w3992:errorcluster, "V2 out"=w3993:dbl)  [unwired: 9 in]
        n1811 = call "GainToCtrlV.vi"("Gain"=w3996, "Channel"=enum16{"Ch1", "Ch2", "Ch3"}."Ch2") -> ("CtrlV"=w3991:dbl)  [unwired: 8 in, 1 out]
        n1812 = local write "V 2"(w3991) -> ()
        n1813 = call "V2FGV.vi"("Error In"=w3992, "V2 in"=w3991) -> ()  [unwired: 8 in, 2 out]
        n1814 = Not Equal?(x=w3991, y=w3993) -> (x != y?=w3995:bool)
      }
    }
    n1815 = case shown="True" w3898 {
      tunnel: w3876 -> [_ w3986]
      tunnel: "V target(1.0)" -> [_ w3983]
      tunnel: [FALSE w3979] -> w3888
      tunnel: [0.0 ("CtrlV") w3977] -> w3887
      frame False {
        # "Manual control"
      }
      frame True {
        # "PID control"
        n1816 = global read "GlobalVariables.vi" "Ch3GainLim(Log)"() -> (w3987:cluster{"GainMax":dbl, "GainMin":dbl})
        n1817 = call-poly <vilib>:"PID.vi"("output range"=w3987, "PID gains"="Ch3 PID gains", "process variable"=w3986, "setpoint"=w3983) -> ("output"=w3985:dbl)  [unwired: 6 in, 1 out]
        n1818 = Power Of 10(x=w3985) -> (10^x=w3982:dbl)
        "Gain3" <- w3982
        n1819 = call "V3FGV.vi"("action(write)"=enum16{"write", "read"}."read") -> ("Error Out"=w3978:errorcluster, "V3 out"=w3980:dbl)  [unwired: 9 in]
        n1820 = call "GainToCtrlV.vi"("Gain"=w3982, "Channel"=enum16{"Ch1", "Ch2", "Ch3"}."Ch3") -> ("CtrlV"=w3977:dbl)  [unwired: 8 in, 1 out]
        n1821 = local write "V 3"(w3977) -> ()
        n1822 = call "V3FGV.vi"("Error In"=w3978, "V3 in"=w3977) -> ()  [unwired: 8 in, 2 out]
        n1823 = Not Equal?(x=w3977, y=w3980) -> (x != y?=w3979:bool)
      }
    }
    n1824 = call "LabJack_FGV.vi"("Operation(Read)"=enum16{"Write", "Read"}."Read" ("Operation"), "error in (no error)"=w3865) -> ("error out"=w3874:errorcluster, "Read data"=w3910:i32)  [unwired: 8 in]
    n1825 = flat-sequence {
      tunnel: [w3914] -> w3871
      tunnel: w3865 -> [_]
      frame #0 {
        n1826 = Tick Count (ms)() -> (millisecond timer value=w3914:u32)
      }
    }
    n1827 = case "Channel 1" shown="True" w3890 {
      tunnel: w3874 -> [w3940 w3946]
      tunnel: w3910 -> [w3939 w3945]
      tunnel: [w3940 w3941] -> w3869
      tunnel: [w3939 w3944] -> w3905
      tunnel: w3873 -> [_ w3942]
      frame False {
        # "Do nothing"
      }
      frame True {
        # "request V\nupdate FGV"
        n1828 = global read "GlobalVariables.vi" "Ch1 LJ pin"() -> (w3943:string)
        n1829 = call "LJM_eWriteName.vi"("Handle In"=w3945, "Name"=w3943, "Value"=w3942, "error in"=w3946) -> ("Handle Out"=w3944:i32, "error out"=w3941:errorcluster)  [unwired: 10 in]
      }
    }
    n1830 = case "Channel 2" shown="True" w3889 {
      tunnel: w3869 -> [w3931 w3938]
      tunnel: [w3931 w3933] -> w3868
      tunnel: w3905 -> [w3932 w3937]
      tunnel: [w3932 w3936] -> w3904
      tunnel: w3885 -> [_ w3934]
      frame False {
        # "Do nothing"
      }
      frame True {
        # "request V\nupdate FGV"
        n1831 = global read "GlobalVariables.vi" "Ch2 LJ pin"() -> (w3935:string)
        n1832 = call "LJM_eWriteName.vi"("Handle In"=w3937, "Name"=w3935, "Value"=w3934, "error in"=w3938) -> ("Handle Out"=w3936:i32, "error out"=w3933:errorcluster)  [unwired: 10 in]
      }
    }
    n1833 = case "Channel 3" shown="True" w3888 {
      tunnel: w3868 -> [w3924 w3930]
      tunnel: [w3924 w3926] -> w3867
      tunnel: w3904 -> [w3923 w3929]
      tunnel: w3887 -> [_ w3927]
      tunnel: [w3923 w3925] -> w3878
      frame False {
        # "Do nothing"
      }
      frame True {
        # "request V\nupdate FGV"
        n1834 = global read "GlobalVariables.vi" "Ch3 LJ pin"() -> (w3928:string)
        n1835 = call "LJM_eWriteName.vi"("Handle In"=w3929, "Name"=w3928, "Value"=w3927, "error in"=w3930) -> ("Handle Out"=w3925:i32, "error out"=w3926:errorcluster)  [unwired: 10 in]
      }
    }
    n1836 = case "Channel 4" shown="True" w3879 {
      tunnel: w3867 -> [w3916 w3922]
      tunnel: w3878 -> [w3915 w3921]
      tunnel: [w3916 w3917] -> w3872
      tunnel: [w3915 w3920] -> _
      tunnel: w3880 -> [_ w3918]
      frame False {
        # "Do nothing"
      }
      frame True {
        # "request V\nupdate FGV"
        n1837 = global read "GlobalVariables.vi" "Ch4 LJ pin"() -> (w3919:string)
        n1838 = call "LJM_eWriteName.vi"("Handle In"=w3921, "Name"=w3919, "Value"=w3918, "error in"=w3922) -> ("Handle Out"=w3920:i32, "error out"=w3917:errorcluster)  [unwired: 10 in]
      }
    }
    "PID loop error out" <- w3872
    n1839 = flat-sequence {
      tunnel: [w3913] -> w3870
      tunnel: w3872 -> [_]
      frame #0 {
        n1840 = Tick Count (ms)() -> (millisecond timer value=w3913:u32)
      }
    }
    n1841 = Subtract(x=w3870, y=w3871) -> (x-y=w3866:u32)
    "LJ process (ms)" <- w3866
    "PID loop" <- w3892
  }
  "LJ time(ms)" <- w9
  n1842 = Release Notifier(notifier=w24, error in (no error)=w48) -> (error out=w49:errorcluster)  [unwired: 1 in, 2 out]
  n1843 = call <vilib>:"Simple Error Handler.vi"("error in (no error)"=w49) -> ()  [unwired: 4 in, 5 out]
  n1844 = Unregister For Events(event registration refnum=w46, error in=w12) -> (error out=w51:errorcluster)
  n1845 = Destroy User Event(user event=w43, error in=w51) -> (error out=w11:errorcluster)
  n1846 = Unregister For Events(event registration refnum=w2) -> (error out=w3:errorcluster)  [unwired: 1 in]
  n1847 = Close File(refnum=w27, error in=w11) -> ()  [unwired: 2 out]
  n1848 = Destroy User Event(user event=w1, error in=w3) -> ()  [unwired: 1 out]
  n1849 = Release Notifier(notifier=w58, error in (no error)=w57) -> (error out=w56:errorcluster)  [unwired: 1 in, 2 out]
  n1850 = Unregister For Events(event registration refnum=w62, error in=w60) -> (error out=w61:errorcluster)
  n1851 = call <vilib>:"Simple Error Handler.vi"("error in (no error)"=w56) -> ()  [unwired: 4 in, 5 out]
  n1852 = Destroy User Event(user event=w52, error in=w61) -> ()  [unwired: 1 out]
